vi "UNITEST MAIN v2.0.vi"() -> ()   [LabVIEW 2025]
uses:
  controls/LAB-IQ UI Data.ctl
  <vilib>/Platform/TimedLoop/XDataNode/timing_clust.ctl
  <vilib>/Platform/TimedLoop/XDataNode/nitl_modes.ctl
  <vilib>/Platform/TimedLoop/XDataNode/wakeup.ctl
  HEAVE vi's/Heave Write enum.ctl
  SWAY vi's/Sway Write enum.ctl
  d081153b-36ca-4bc4-8478-749476f82ba4.vi
  1202965f-721d-4349-8d61-5de826f379ef.vi
  785ec975-e53d-4ed4-be48-2cc128d7a91f.vi
  02c5850b-52e8-4ed5-91f8-6f0ad62f4994.vi
  1223eb78-e4c4-4b69-bf80-185c82055158.vi
  e5651a45-6a49-4a3f-b503-ff1eaf449b4a.vi
  <vilib>/Utility/error.llb/Trim Whitespace One-Sided.vi
  support/Message Queue/Enqueue Message (Single).vi
  <vilib>/Utility/error.llb/Error Cluster From Error Code.vi
  <vilib>/Utility/file.llb/Read Delimited Spreadsheet (string).vi
  <vilib>/Utility/file.llb/Write Delimited Spreadsheet (string).vi
  <vilib>/platform/TimedLoop/XDataNode/XDataNode.xnode
  <vilib>/ErrorRing/Error Ring.xnode
  support/Message Queue/LAB-IQ Message Queue.lvlib
  support/User Event - Stop/LAB-IQ User Event - Stop.lvlib
  <vilib>/Platform/TimedLoop/XDataNode/XDNodeRunTimeDep.lvlib
panel:
  in  "DEPTH TRIP   ENABLE":bool
  in  "DEPTH TRIP VALUE":dbl
  in  "LOAD TRIP  ENABLE":bool
  in  "LOAD TRIP VALUE":dbl
  in  "CYCLIC COF TRIP  ENABLE":bool
  in  "CYCLIC FF TRIP  ENABLE":bool
  in  "FF TRIP  ENABLE":bool
  in  "COF TRIP  ENABLE":bool
  in  "CYCLIC CoF TRIP VALUE":dbl
  in  "CYCLIC FF TRIP VALUE":dbl
  in  "FF TRIP VALUE":dbl
  in  "COF TRIP VALUE":dbl
  in  "Dummy Run":bool
  in  "AutoTune":bool
  in  "reinit 3":bool=TRUE
  in  "output range delay":cluster{"output high":dbl, "output low":dbl}={"output high"=100.0, "output low"=-100.0} {"output low" format="%.2f"; "output high" format="%.2f"}
  in  "PID gains out delay":T1={"proportional gain (Kc)"=30.0, "integral time (Ti, min)"=0.00101, "derivative time (Td, min)"=0.0} {"derivative time (Td, min)" format="%.3f"; "integral time (Ti, min)" min=1e-05 max=100.0 step=0.0001 format="%.4f"; "proportional gain (Kc)" format="%.3f"}
  in  "PID gains out delay (microForce)":T1={"proportional gain (Kc)"=300.0, "integral time (Ti, min)"=0.00011, "derivative time (Td, min)"=0.0} {"derivative time (Td, min)" format="%.3f"; "integral time (Ti, min)" min=1e-05 max=100.0 step=1e-06 format="%.6f"; "proportional gain (Kc)" format="%.3f"}
  in  "Gain 2":dbl=0.016
  in  "Offset  3":dbl=1.5
  in  "Ramp MulFac":dbl=2.0
  out "actpid":dbl
  in  "pulses LoadDiffRamp(2..10)":dbl=9.0
  in  "PulseControlRamp(diff<=3N)":dbl=5.0 min=1.0 max=1000.0 step=1.0 format="%#.1f"
  in  "SetLoadDeadband(%) Load(0-10N)":dbl=0.1 min=0.0001 max=100.0 step=0.0001 format="%#.6f"
  in  "pulses LoadDiff(2..10)":dbl=10.0
  in  "pulses LoadDiff(11..50)":dbl=40.0
  in  "PulseControl(diff<=3N)":dbl=1.0 min=1.0 max=1000.0 step=1.0 format="%#.1f"
  out "SetLoadDeadband(%)  2":dbl=1.0 min=0.001 max=100.0 step=0.001 format="%#.6f"
  in  "pulsesSent":dbl=200.0
  out "pulses":dbl
  in  "pulses LoadDiff(21..1000)":dbl=40.0
  in  "Delay":dbl=1.5 min=0.001 max=5.0 step=0.001 format="%#.6f"
  in  "deadband":dbl=0.2
  in  "Checkbox 2":bool
  in  "Checkbox":bool=TRUE
  out "Scratch Start Recording":bool
  in  "SwaySpeed Set":bool
  in  "Update":bool
  in  "Analysis Home":bool
  in  "Installation/Replacement completed":bool
  in  "Loahead":bool
  in  "Heave and Surge COM Port:":refnum<visa-resource-name>="COM9"
  in  "Sway COM Port:":refnum<visa-resource-name>="COM10"
  out "Test Trip":bool
  out "Hymidity":bool
  in  "Humidity Disable trip":bool=TRUE
  in  "CoF Trip  2":dbl=540.0 min=100.0 max=540.0 step=1.0
  in  "File Path :  2":path
  out "Wear Track Diameter":dbl
  in  "Stribeck table":bool
  in  "seq":bool=TRUE
  out "Drive Error":string
  out "mm/s  Surge":dbl=7.0 caption="Jog" min=0.001 max=50.0 step=0.0001 format="%.2f"
  in  "Update Surge Speed":bool
  out "mm/s  Sway":dbl=7.0 caption="Jog" min=0.001 max=50.0 step=0.0001 format="%.2f"
  in  "Update Sway Speed":bool
  in  "Update Heave Speed":bool
  out "mm/s Heave":dbl=7.0 caption="Jog" min=0.001 max=30.0 step=0.0001 format="%.2f"
  in  "mm/sec":dbl=1.0 caption="Jog" min=0.001 max=50.0 step=0.001 format="%.2f"
  out "Scratch Start Test":bool
  in  "HomeScratch":bool
  in  "TEST SELECTION":enum32{"Time", "Cycle"}(radio)
  out "HEAVE ENABLE":bool
  in  "SPARE  5":u8
  in  "Manual Write SWAY":bool
  out "SWAY WRITE":string
  in  "SPARE  4":u8
  in  "SPARE  3":u8
  in  "SPARE 2":u8
  in  "SPARE 1":u8
  out "Spare 15":u8
  out "Spare 14":u8
  out "Spare 13":u8
  out "Spare 12":u8
  out "Spare 11":u8
  out "Spare 10":u8
  out "Spare 9":u8
  out "Spare 8":u8
  out "Spare 7":u8
  out "Spare 6":u8
  out "Spare 5":u8
  out "Spare 4":u8
  out "Spare 3":u8
  out "Spare 2":u8
  out "Spare 1":u8
  out "Node Id":u8
  out "Read SWAY Temp":bool
  out "fwMinor":u8
  out "fwMajor":u8
  out "faultCode":u16
  out "Rotary POSE":sgl format="%#.6f"
  out "SWAY POSE":sgl format="%#.6f"
  out "Homed":u8
  out "State":u8
  out "Ack ID":u16
  in  "SPEED":sgl=10000.0
  in  "Distance":sgl=10000.0
  in  "Mode Command":u8=2
  out "Sequence ID":u16
  out "error out Read SWAY":errorcluster
  out "error out Write  SWAY":errorcluster
  out "SWAY READ":string
  out "Start Test Temp":bool
  in  "AppLoadSeq scratch":bool
  in  "PID Delay (sec)":dbl=1.0 format="%#_6p"
  in  "Manual Write Heave & Surge":bool
  out "Heave and Surge Write":string
  in  "SPARE 4":u8
  in  "SPARE 3":u8
  in  "SPARE 2":u8
  in  "SPARE 1":u8
  out "Spare 15":u8
  out "Spare 14":u8
  out "Spare 13":u8
  out "Spare 12":u8
  out "Spare 11":u8
  out "Spare 10":u8
  out "Spare 9":u8
  out "Spare 8":u8
  out "Spare 7":u8
  out "Spare 6":u8
  out "Spare 5":u8
  out "Spare 4":u8
  out "Spare 3":u8
  out "Spare 2":u8
  out "Spare 1":u8
  out "Node Id":u8
  out "Read Heave Temp":bool
  out "fwMinor":u8
  out "fwMajor":u8
  out "faultCode":u16
  out "SURGE POSE":sgl format="%#.6f"
  out "HEAVE POSE":sgl format="%#.6f"
  out "Homed":u8
  out "State":u8
  out "Ack ID":u16
  in  "SPEED":sgl=10000.0
  in  "Distance":sgl=10000.0
  in  "Mode Command":u8=2
  out "Sequence ID":u16
  out "error out Read":errorcluster
  out "error out Write":errorcluster
  out "Heave and Surge Read":string
  out "Load Cell Temp":bool
  in  "Stop Scratch":bool
  in  "Enter Fixed SRR 2":dbl min=0.0 max=0.0 format="%.3f"
  in  "E.Velocity 2":bool=TRUE caption="SRR"
  in  "Tab Control 3":T2(tab)
  in  "Tab Control 5":enum32{""}(tab)
  in  "Tab Control 14":T3(tab)=enum."Motor Load"
  in  "Ramp":bool
  in  "apply load":bool
  in  "Enter ByPass Load":dbl
  in  "Bypass Load":bool
  out "gFF Rot 7":cluster{dbl, dbl, dbl}(graph)
  in  "Current Load":dbl
  in  "Set Load":dbl
  out "Current Position":dbl
  in  "Kp":dbl=1.0
  in  "Ki":dbl
  in  "Kd":dbl
  in  "Deadband":dbl=0.1
  in  "pct_scale":dbl=100.0
  in  "Init Step":dbl=10.0
  in  "Max Step Linit":dbl=10.0
  in  "i_limit":dbl=10.0
  in  "Min_pos_limit":dbl
  in  "Max_pos_limit":dbl=50000000.0
  in  "Fine Tune Zone":dbl=10.0
  in  "fine_tune_pct":dbl=100.0
  in  "min_deadband_floor":dbl=0.05
  in  "min_finetune_floor":dbl=0.15
  out "Pulse delta":dbl
  out "Vertical load (N)":dbl format="%#.3f"
  in  "Tab Control 26":enum32{"Page 1", "Page 2"}(tab)
  in  "ClearAll":bool
  out "Mz(Nm)":dbl[](array[numeric])
  out "My(Nm)":dbl[](array[numeric])
  out "Mx(Nm)":dbl[](array[numeric])
  in  "Save Dwell":dbl=0.015 caption="Save Dwell (sec)" min=0.0 max=5.0 step=0.001 format="%.3f"
  out "Mx":dbl[](graph)
  out "My":dbl[](graph)
  out "Mz":dbl[](graph)
  out "Fy(N)":dbl[](graph)
  out "Fz(N)":dbl[](graph)
  in  "ZeroAll":bool
  in  "Acq Delay (ms)":dbl=10.0
  in  "Burst Delay (ms)":dbl=10.0
  out "model":string
  out "SN":i32
  out "FFx(N)":dbl[](array[numeric])
  in  "Sensor IP":string="192.168.1.100"
  in  "Port":i32=8080
  out "FFy(N)":dbl[](array[numeric])
  out "Load(N)":dbl[](array[numeric])
  out "Fx(N)":dbl[](graph)
  out "AE":bool
  in  "delete Handle":bool
  in  "Create Handle":bool=TRUE
  out "ft_data":dbl[](array[numeric])=[1.0, 1.0, 1.0, 1.0, 1.0, 1.0]
  out "ft_range":dbl[](array[numeric])=[1.0, 1.0, 1.0, 1.0, 1.0, 1.0]
  in  "stop 6":bool
  out "running_flag":bool
  out "ft_udp_handle":i32
  out "get-data-return":i32
  out "get-range-return":i32
  out "zero-return":i32
  out "filter-return":i32
  out "initial-return":i32
  out "deleteHandle-result":i32
  in  "Tab Control 19":enum32{"Platform COM", "Config ", "DevInfo"}(tab)=enum."Config "
  in  "SAMPLES":dbl=100.0
  in  "Re-initilaize":bool
  in  "Filter ON/OFF":bool=TRUE
  in  "TracHomeSurgeOffsetCounts 10MM":dbl=505100.0
  in  "TracHomeSwayOffsetCounts 10MM":dbl=1432.0
  in  "Acoustic Emission:":dbl=1.0 min=0.0001 max=200.0 step=0.0001 format="%.4f"
  in  "Apply Filter (FF)":bool
  in  "Filter% 2":dbl=50.0 min=50.0 max=100.0 step=0.1 format="%.1f"
  in  "Apply Filter (Load)":bool=TRUE
  in  "Filter%":dbl=80.0 min=50.0 max=100.0 step=0.1 format="%.1f"
  in  "Sway distance (mm)":dbl=245.0
  in  "Surge distance (mm)":dbl=370.0
  in  "DataSavingLoopDelay(ms)":dbl=15.0
  in  "SAVE  2":bool
  in  "Enter Distance":bool caption="Enter Counts"
  in  "Sway Counts:":dbl=100.0 min=0.0 max=100000000.0 step=1.0 format="%.2f"
  in  "Distance (mm): 3":dbl=100.0 caption="Distance (mm):" min=0.0 max=1500.0 step=0.001 format="%.5f"
  in  "Surge Counts:":dbl=100.0 min=0.0 max=100000000.0 step=1.0 format="%.1f"
  in  "Distance (mm): 2":dbl=100.0 caption="Distance (mm):" min=0.0 max=1500.0 step=0.0001 format="%.3f"
  in  "Distance (mm):":dbl=100.0 min=0.0 max=1500.0 step=0.001 format="%.5f"
  in  "Heave Counts:":dbl=100.0 min=0.0 max=100000000.0 step=1.0
  in  "LRMHomeSurgeOffsetCounts":dbl=307197.0
  in  "LRMHomeSwayOffsetCounts":dbl=26880.0
  in  "TracHomeSurgeOffsetCounts 20MM":dbl=505100.0
  in  "TracHomeSwayOffsetCounts 20MM":dbl=1432.0
  in  "RotHomeSwayOffsetCounts":dbl=14656.0
  in  "RotHomeSurgeOffsetCounts":dbl=311465.0
  in  "Heave distance":dbl=340.0
  out "Zmm":dbl=1600.0
  out "Heave Pulses/mm":dbl=1600.0
  out "Surge Pulses/mm":dbl=1600.0
  out "Sway Pulses/mm":dbl=320.0
  in  "Heave Pitch":dbl=4.0
  in  "Surge Pitch":dbl=3.0
  in  "Sway Pitch":dbl=2.0
  in  "Heave PPR":dbl=6400.0
  in  "Surge PPR":dbl=6400.0
  in  "Sway PPR":dbl=6400.0
  in  "Heave Jog Speed":dbl=15.0
  in  "Surge Jog Speed":dbl=1.0 format="%.4f"
  in  "Heave PID Speed":dbl=15.0
  in  "Heave Loop Delay":dbl
  in  "Sway Jog Speed":dbl=1.0 format="%.4f"
  in  "Sway PID Speed":dbl=1.0 format="%.4f"
  in  "Sway Loop Delay":dbl
  in  "GUI":T4(tab)
  in  "Platform Settings":bool caption="Password"
  in  "Configure":bool caption="Password"
  in  "Home":bool caption="Password"
  in  "EXIT":bool
  in  "Analysis":bool caption="Password"
  in  "service 2":bool caption="Password"
  in  "MainPage":T5(tab)=enum."HOME"
  in  "Select Load Head":bool
  in  "Notes :":string
  in  "FILE":string
  in  "Sample ID :":string
  in  "Operator ID :":string
  in  "Operator Name :":string
  in  "Auto":bool caption="Power Status"
  in  "Disable Axis Jog Soft Limits m":bool
  out "Sway and Surge COM Status":bool=TRUE caption="Load COM Status"
  out "Heave COM Status":bool=TRUE caption="Load COM Status"
  in  "Enable Platform":bool
  in  "Surge Forward Main":bool
  in  "Surge Backward Main":bool
  in  "Sway Right Main":bool
  in  "Sway Left Main":bool
  in  "Heave Down Main":bool
  in  "Heave Up main":bool
  in  "mm":dbl=0.001 caption="Jog" min=1.0 max=100.0 step=0.01 format="%#.3f"
  in  "Surface Analysis":bool
  in  "Imaging":bool
  in  "Image Analysis":bool
  in  "Post Analysis":bool
  in  "SSP 0.75":bool
  in  "SSP 0.5":bool
  in  "SSP 0.3":bool
  in  "Warning":enum32{"Page 2"}(tab)
  in  "gui GIF":enum32{"Check", "Deca", "kilo", "Micro"}(tab)
  out "Communication is established":bool=TRUE caption="Load COM Status"
  in  "Reference Sample":u16(ring) items=["None", "Brass", "Aluminium", "Mild Steel"]
  out "Load Cell Communication Slide":u8(slide)=1 min=1 max=10 step=1 scale=0.0..10.0
  in  "com 3":bool
  out "com":bool
  out "DecaForce COM Status":bool caption="Load COM Status"
  in  "Loading Mode":u16(ring) items=["Constant", "Ramp", "Steps", "Indentation"]
  in  "Enter the CoF Trip":dbl=1.0
  in  "Enter the Friction Force Trip":dbl=520.0 min=500.0 max=500.0 step=1.0 format="%#.1f"
  in  "Enter the Normal load Trip":dbl=520.0 min=500.0 max=500.0 step=0.001 format="%.3f"
  in  "KiloForce":bool
  in  "DecaForce":bool
  in  "MicroForce":bool
  in  "LHBack":bool
  in  "LHNext":bool
  in  "Load Selection":T6(tab)
  in  "Enter the Load  (N)":dbl=2.0 caption="Enter the Load (N)" min=2.0 max=200.0 step=0.1 format="%#.4f"
  in  "Enter the Final Load (N)":dbl=1.0 min=0.0 max=500.0 step=1.0 format="%#.0f"
  in  "Enter the Loading Rate (N/min)":dbl=60.0 min=1.0 max=1200.0 step=0.1 format="%.2f"
  out "Warning 2":bool
  in  "Stribeck Table  For loading":string[][](table)
  in  "Clear 3":bool
  out "Message":string="Load Entered is out of range!!!"
  in  "Indentation":string[][](table)=[["Detection", "5", "2"], ["Unload", "0", "5"], ["Load", "10", "2"], ["Unload", "0", "5"], ["Detection", "5", "2"], ["Unload", "0", "5"]]
  in  "Multipoint":bool caption="Singlepoint"
  in  "AppLoad 4":bool
  in  "zNL":bool
  out "NL disp":dbl caption="Normal Load ( N )" min=-2000.0 max=2000.0 step=0.0001 format="%.1f"
  in  "Traction":bool
  in  "Surge Forward MM":bool
  in  "Surge Backward MM":bool
  in  "M3 Image":enum32{"Page 1", "Page 2"}(tab)
  in  "String 39":string="Jog heave to bring the upper sample closer to the lower sample within 1mm."
  in  "Sway Left MM":bool
  in  "Sway Right MM":bool
  in  "Disable Axis Jog Soft Limits":bool
  in  "mm":dbl=0.001 caption="Jog" min=0.001 max=5.0 step=0.0001 format="%#.3f"
  in  "Heave Down MM":bool
  in  "Heave Up MM":bool
  in  "Wear Track Diameter (mm)":dbl=30.0 caption="Wear Track Diameter (mm):" min=1.0 max=30.0 step=1.0 format="%.2f"
  in  "Set WTD":bool
  in  "HomeScratch":bool
  in  "HomeRot":bool
  in  "PlaceModule":bool
  in  "Motion Mode:":u16(ring) items=["Uniform Rotation", "Angular Oscillation", "Stribeck ", "Steps"]
  in  "LR Sway":bool
  in  "Rot Hor":bool
  in  "Rot Ver":bool
  in  "Scratch":bool
  in  "LR Cam":bool
  in  "MMBack":bool
  in  "MMNext":bool
  in  "Rotary Module Selection":T7(tab)
  in  "SPEED SELECTION :":enum32{"Speed in RPM", "Speed in m/sec"}(radio)=enum."Speed in m/sec"
  in  "Enter the Speed(mm/sec)":dbl=0.1 min=0.1 max=10.0 step=0.1 format="%.3f"
  in  "Enter the Speed (RPM)":dbl=45.0 min=1.0 max=3000.0 step=1.0
  in  "Enter the Frequency (Hz)":dbl=1.0 min=0.1 max=10.0 step=0.1 format="%.1f"
  in  "Enter the Angle (Deg)":dbl=45.0 min=5.0 max=300.0 step=1.0
  in  "Angular Oscillation Set":bool
  in  "Rotary Tab":enum32{"Page 1", "Page 2"}(tab)
  out "e.v/ssr 2":enum32{"E.V", "SSR"}(tab)
  in  "Enter the Final E.Velocity (m/s) 2":dbl=1.0 min=0.001 max=4.0 step=0.001 format="%.3f"
  in  "Enter initial E.Velocity (m/s) 2":dbl=2.0 min=0.001 max=4.0 step=0.001 format="%.3f"
  in  "Enter Fixed E.Velocity 2":dbl=1.0 min=0.001 max=2.0 step=0.001 format="%.3f"
  in  "Enter Final SRR 2":dbl=1.0 min=0.001 max=1.0 step=0.001 format="%.2f"
  in  "Enter initial SRR 2":dbl=1.0 min=0.001 max=1.0 step=0.001 format="%.2f"
  out "Final Speed (RPM) 3":dbl=1.0 min=0.1 max=3000.0 step=0.1 format="%.1f"
  out "Initial Speed (RPM) 2":dbl=100.0 min=0.1 max=3000.0 step=0.1 format="%.1f"
  in  "Enter the Final Velocity (m/s) 3":dbl=1.0 min=0.001 max=2.0 step=0.001 format="%.3f"
  in  "Enter initial Velocity (m/s)  3":dbl=2.0 min=0.001 max=2.0 step=0.001 format="%.3f"
  out "Ramp Up 2":bool caption="Ramp Down"
  in  "Import 2":bool
  in  "Save 2":bool
  in  "SPEED SELECTION : rotary":enum32{"Speed in Rpm", "Speed in m/sec"}(radio)=enum."Speed in m/sec"
  in  "calculate rotary":bool
  in  "String 45":string="File Path Location : C:-->LAB-IQ 150 --> User Defined\n                                       Protocol-->File.txt"
  in  "Step Speed":enum32{"Step Speed", "Step (load-Speed)"}(tab)
  in  "StepTable For Speed":string[][](table)
  in  "StepTable For Load-Speed":string[][](table)=[["", "", ""], ["", "", ""], ["", "", ""], ["", "", ""]]
  in  "StepTable For Speed 3":string[][](table)=[["", "", ""], ["", "", ""], ["", "", ""], ["", "", ""]]
  in  "Motion Direction:  3":u16(ring) items=["Clockwise", "Counter Clockwise"]
  in  "Enter Scratch length (mm):":dbl=1.0 min=1.0 max=50.0 step=0.0001 format="%.4f"
  in  "Enter Scratch Speed (mm/s):":dbl=1.0 min=0.003 max=10.0 step=0.0031 format="%.5f"
  in  "Scartch Offset":dbl=1.0 caption="Scratch Offset: (mm)" min=0.1 max=5.0 step=0.1 format="%.1f"
  in  "Motion type:":u16(ring) items=["Unidirection", "Bidirection"]
  in  "Scratch Mode":u16(ring) items=["Scratch", "Pre-Post Scan", "Multi Scratch"]
  in  "Rotary Speed Exced":string="Motor Speed Out of Range"
  in  "No of Scratch":dbl=1.0 min=1.0 max=50.0 step=0.0001
  out "Humidity  Status  3":bool caption="Communication Status"
  out "Low Temp  Status  2":bool=TRUE caption="Communication Status"
  out "TK4 status 2":bool=TRUE caption="Communication Status"
  in  "String 40":string="Before selecting Acoustic make sure the sensor output pin is connected to A4."
  in  "Stage Temperature":dbl[](array[numeric])=[150.0, 230.0, 300.0, 350.0, 400.0, 450.0, 500.0]
  in  "Sample Temperature":dbl[](array[numeric])=[100.0, 150.0, 200.0, 250.0, 300.0, 350.0, 400.0]
  in  "Humidity (Amb)":bool
  in  "Clear List":bool
  out "Sensors Picked":string
  in  "Add to list":bool
  in  "Wear":bool
  in  "Vibration":bool
  in  "Humidity (Chamber)":bool
  in  "Temperature (Chamber)":bool
  in  "ECR":bool
  in  "Temperature (Amb)":bool
  in  "Microphone":bool
  in  "Acoustic Emission 3":bool
  in  "SNext":bool
  in  "APBack":bool
  in  "Enter the Temperature (°C):":dbl
  in  "Enter the Stage \nTemperature (°C):":dbl=20.0 min=20.0 max=150.0 step=1.0 format="%#.0f"
  in  "Enter the Humidity (%Rh):":dbl=30.0 min=30.0 max=85.0 step=1.0
  in  "Low Temp":bool
  in  "High Temp":bool
  in  "Humidity":bool
  in  "Main Screen Tab":T8(tab)
  in  "ClrLog":bool
  out "Trip Log":string
  in  "Start Test":bool
  out "Test status":bool caption="Test Status"
  out "AR Led":bool caption="AR"
  out "Data":bool=TRUE
  out "Health":bool=TRUE
  out "Sway COM Status":bool=TRUE caption="Load COM Status"
  out "Heave COM Status":bool=TRUE caption="Load COM Status"
  in  "BACK":bool
  out "Ambient \nTemperature":dbl min=0.0 max=5000.0 step=0.1 format="%.1f"
  out "Ambient\n Humidity":dbl min=0.0 max=5000.0 step=0.1 format="%.2f"
  out "NL disp 2":dbl caption="Normal Load ( N )" min=-2000.0 max=2000.0 step=0.0001 format="%.1f"
  out "Set Humidity":dbl caption="Set Humidity  (% Rh)" min=-2000.0 max=2000.0 step=1.0 format="%.1f"
  out "humidity disp":dbl caption="Humidity (% Rh)" min=-2000.0 max=2000.0 step=1.0 format="%.1f"
  in  "Humidity On":bool
  in  "zNL 2":bool
  out "NLt":bool
  in  "Load En":bool
  out "Freq (Hz)":dbl min=0.0 max=5000.0 step=0.1 format="%.4f"
  out "HumCOMStatus":bool caption="Communication Status"
  out "Load Communication":bool
  in  "Temp Tabs":enum32{"Low Temp", "High Temp"}(tab)=enum."High Temp"
  out "Controller  Status":bool
  out "ChamberTemp":dbl format="%#.1f"
  in  "SetTmp":dbl=-190.0 caption="Set Temperature (Deg C)" min=-190.0 max=100.0 step=1.0 format="%.1f"
  in  "Cooling":bool
  in  "Heater":bool
  out "TK4 status":bool caption="Controller  Status"
  out "ChamberTemp":dbl format="%#.1f"
  in  "SetTmp":dbl caption="Set Temperature (Deg C)" min=0.0 max=1000.0 step=1.0 format="%.1f"
  in  "Set Load (N)":dbl=100.0 min=0.01 max=1500.0 step=0.01 format="%.1f"
  in  "Time Tab":enum32{"cycles", "duration"}(tab)=enum."duration"
  out "Test Duration 4":dbl=600.0 caption="Test Duration\n(HH:MM:SS)" min=0.0083 max=180000.0 step=0.0001 format="%<%H:%M:%S>t"
  out "TEST CYCLE":dbl min=0.0 max=5000.0 step=0.01 format="%.2f"
  in  "TOTAL CYCLES":dbl min=0.0 max=5000.0 step=0.1 format="%.4f"
  out "Time ( HH:MM:SS ) 2":dbl min=0.0 max=144000.0 step=1.0 format="%<%H:%M:%S>t"
  in  "Test Duration":dbl=600.0 caption="Test Duration\n(HH:MM:SS)" min=0.0083 max=180000.0 step=0.0001 format="%<%H:%M:%S>t"
  in  "Main Speed Tab":enum32{"ROTARY", "TRACTION"}(tab)
  in  "SPEED TAB":enum32{"RPM", "m/sec"}(tab)
  out "Speed (RPM)":dbl min=0.0 max=5000.0 step=0.1 format="%.1f"
  out "Set Speed":dbl caption="Set Speed (RPM)" min=0.0 max=1500.0 step=0.1 format="%.1f"
  out "Speed (m/sec)":dbl min=0.0 max=5000.0 step=0.001 format="%.4f"
  out "Set Speed (m/sec)":dbl min=0.0 max=1500.0 step=0.001 format="%.4f"
  in  "MTM MOTOR DISPLAY":enum32{"MTM RPM", "MTM m/sec"}(tab)
  out "Disc Speed (RPM)":dbl min=0.0 max=1500.0 step=0.1 format="%.1f"
  out "Ball Speed (RPM)":dbl min=0.0 max=1500.0 step=0.1 format="%.1f"
  out "Disc Speed (m/sec)":dbl min=0.0 max=1500.0 step=0.1 format="%.1f"
  out "Ball Speed (m/sec)":dbl min=0.0 max=1500.0 step=0.1 format="%.1f"
  in  "Angle and Frequency":enum32{"angular", "lrm"}(tab)
  out "Angle (Deg)":dbl min=0.0 max=5000.0 step=0.01 format="%.2f"
  out "Stroke (mm)":dbl min=0.0 max=5000.0 step=0.01 format="%.2f"
  in  "STOP":bool
  out "Multi Scratch Pass":dbl min=0.0 max=5000.0 step=0.1
  in  "FF Tab":T9(tab)
  in  "COF Reset Graph":bool
  in  "COF Disable Trip":bool=TRUE
  out "COF TRIP":dbl=600.0
  out "Coefficient of Friction":dbl(graph)=0.13298760003255525
  in  "zFF":bool
  in  "FF Reset Graph":bool
  in  "FF Disable Trip":bool=TRUE
  out "FF TRIP":dbl=600.0
  out "Friction Force (N)":dbl min=-2000.0 max=2000.0 step=0.0001 format="%.3f"
  out "Friction Force (N) Graph":dbl(graph)=0.13298760003255525
  out "Cyclic FF TRIP":dbl=600.0
  in  "Cyclic FF Disable Trip":bool=TRUE
  in  "Cyclic FF Reset Graph":bool
  in  "CZ FF":bool
  out "Cyclic Friction Force (N) Graph":dbl(graph)=0.13298760003255525
  out "Cyclic Friction Force (N)":dbl min=-2000.0 max=2000.0 step=0.0001 format="%.3f"
  out "cyclic COF TRIP":dbl=600.0
  in  "cyclic COF Disable Trip":bool=TRUE
  in  "cyclic COF Reset Graph":bool
  out "Cyclic Coefficient of Friction":dbl(graph)=0.13298760003255525
  out "Main Chart 3":cluster{dbl, "NL disp":dbl, dbl}(graph)
  out "NL Display 4":dbl caption="Normal Load ( N )" min=-2000.0 max=2000.0 step=0.0001 format="%.1f"
  in  "Load Reset Graph":bool
  in  "Load Disable Trip":bool=TRUE
  out "Load pid":bool
  out "NL Trip 2":dbl=600.0
  out "WearGp":dbl(graph)=0.13298760003255525
  out "Depth (µm)":dbl min=-200.0 max=200.0 step=0.1 format="%.1f"
  in  "Depthz":bool
  out "Weart":bool
  in  "Depth Reset Graph":bool
  out "Weart Deapth":bool
  in  "Depth Trip 2":bool=TRUE
  out "Depth Trip":dbl=600.0
  in  "Sub Graph":T10(tab)
  in  "Speed Tab":enum32{" Rotary Disc", "MTM Ball", "MTM Disc"}(tab)
  out "speed mm/sec":dbl(graph)=0.13298760003255525
  in  "Speed Reset Graph":bool
  out "MTM BALL SPEED":dbl(graph)=0.13298760003255525
  out "MTM DISC  SPEED":dbl(graph)=0.13298760003255525
  in  "Temperature Reset":bool
  out "Temperature (deg c)":dbl(graph)=0.13298760003255525
  out "ECR 2":dbl(graph)=0.13298760003255525
  in  "ECR RESET":bool
  out "Acoustic Emission (mV)":dbl min=0.0 max=5000.0 step=0.1
  in  "Aqucostic Reset Graph":bool
  out "gACQUOS":dbl(graph)=0.13298760003255525
  in  "Humidity Reset Graph":bool
  out "HumrGp":dbl(graph)=0.13298760003255525
  out "SD (mm)":dbl caption="Sliding Distance ( mm )" min=-200.0 max=200.0 step=0.1 format="%.4f"
  in  "Siliding distance Reset Graph":bool
  out "SDGp":dbl(graph)=0.13298760003255525
  in  "X-AXIS":u16(ring) items=["None", "Time ( Sec )", "Normal Load ( N )", "Frictional Force ( N )", "Coefficient of Friction", "Depth ( Microns )", "Speed ( RPM )", "Frequency ( Hz )", "Angle ( Degree )", "Cyclic Friction Force ( N )", "Cyclic Co efficient Friction ", "Stage temperature ( Degree celcius )", "Sample temperature ( Degree celcius )", "Stroke Length ( mm )", "Scratch Speed ( mm/sec )", "Amb Humidity ( % Rh ) ", "Amb Temperature (Deg C)", "Acoustic (mV)", "Mx (Nm)", "My (Nm)", "Mz (Nm)", "Humidity ( % Rh )", "Sliding Distance (mm)", "Wear Track Diameter (mm)", "Fx(N)", "Fy(N)", "MTM BallSpeed (RPM)", "MTM DiscSpeed (RPM)", "Entrainment Speed", "Slide Role", "Slip(%)", "Rotary Speed (m/sec)", "MTM Ball Speed (m/sec)", "MTM Disc Speed (m/sec)", "ECR (ohms)"]
  in  "Y-AXIS":u16(ring) items=["None", "Time ( Sec )", "Normal Load ( N )", "Frictional Force ( N )", "Coefficient of Friction", "Depth ( Microns )", "Speed ( RPM )", "Frequency ( Hz )", "Angle ( Degree )", "Cyclic Friction Force ( N )", "Cyclic Co efficient Friction ", "Stage temperature ( Degree celcius )", "Sample temperature ( Degree celcius )", "Stroke Length ( mm )", "Scratch Speed ( mm/sec )", "Amb Humidity ( % Rh ) ", "Amb Temperature (Deg C)", "Acoustic (mV)", "Mx (Nm)", "My (Nm)", "Mz (Nm)", "Humidity ( % Rh )", "Sliding Distance (mm)", "Wear Track Diameter (mm)", "Fx(N)", "Fy(N)", "MTM BallSpeed (RPM)", "MTM DiscSpeed (RPM)", "Entrainment Speed", "Slide Role", "Slip(%)", "Rotary Speed (m/sec)", "MTM Ball Speed (m/sec)", "MTM Disc Speed (m/sec)", "ECR (ohms)"]
  out "XY Graph":cluster{"Array 2":dbl[], "Array 2":dbl[]}[](graph) caption="XY Graph 20"
  out "VARIANCE":dbl=-0.0 format="%0.2f"
  out "SD":dbl=-0.0 format="%.3f"
  out "MEAN":dbl format="%.3f"
  out "VARIANCE":dbl=-0.0 format="%0.2f"
  out "SD":dbl=-0.0 format="%.3f"
  out "MEAN":dbl format="%.3f"
  out "VARIANCE":dbl=-0.0 format="%0.2f"
  out "SD":dbl=-0.0 format="%.3f"
  out "MEAN":dbl format="%.3f"
  out "VARIANCE":dbl=-0.0 format="%0.2f"
  out "SD":dbl=-0.0 format="%.3f"
  out "MEAN":dbl format="%.3f"
  in  "Analysis Home new":bool
  out "File 2 Discription":string="\r"
  out "File 1 Discription":string="\r"
  in  "OPEN 1":bool
  in  "OPEN 2":bool
  out "File Name 1":string
  out "File Name 2":string
  in  "Refresh 2":bool
  in  "OPEN 3":bool
  out "File Name 3":string
  out "File Name 4":string
  in  "OPEN 4":bool
  out "File 4 Discription":string="\r"
  out "File 3 Discription":string="\r"
  in  "File Format":u16(ring) items=["csv", "txt", "duf"]
  in  "Export":bool
  in  "Report":bool
  in  "Password":string
  in  "Home Service":bool
  in  "Advanced Setting":bool
  in  "About Tab":enum32{"Primary"}(tab)
  in  "ECR Port:":refnum<visa-resource-name>="COM10"
  in  "Ramp Port:":refnum<visa-resource-name>="COM10"
  in  "Temp Modbus:":refnum<visa-resource-name>="COM14"
  in  "Humidity Port:":refnum<visa-resource-name>="COM10"
  in  "Edit Gain Constants":bool
  in  "Save Gain Constants":bool
  in  "Service About":bool
  # "SET JOG SPEED"
  # "Speed Exceed the limit of the Motor"
  # "Motor Speed Out of Range"
  # "NOTE: This operation needs to be done only when the machine is ON."
  # "ohms"
  # "load Aquisition off"
  # "load Aquisition On"
  # "Configuration"
  # "Limits for Heave Surge and Sway"
  # "Modules Offset Parameters"
  # "Counts-Distance Calculator"
  # "File Name :"
  # "Ensure the traction module is aligned\n horizontally with the stage before ENABLE."
  # "JOG MODE"
  # "Module Selection"
  # "Positioning Control"
  # "Connect the controller\ncable to M3"
  # "Environment"
  # "Sensors"
  # "Data Points"
  # "Data Points"
  # "Data Points"
  # "Data Points"
  # "Data Points"
  # "Data Points"
  # "Data Points"
  # "LAB-IQ 150 / UNITEST / WO2456 / UT150  v05 / AUGUST 2025"
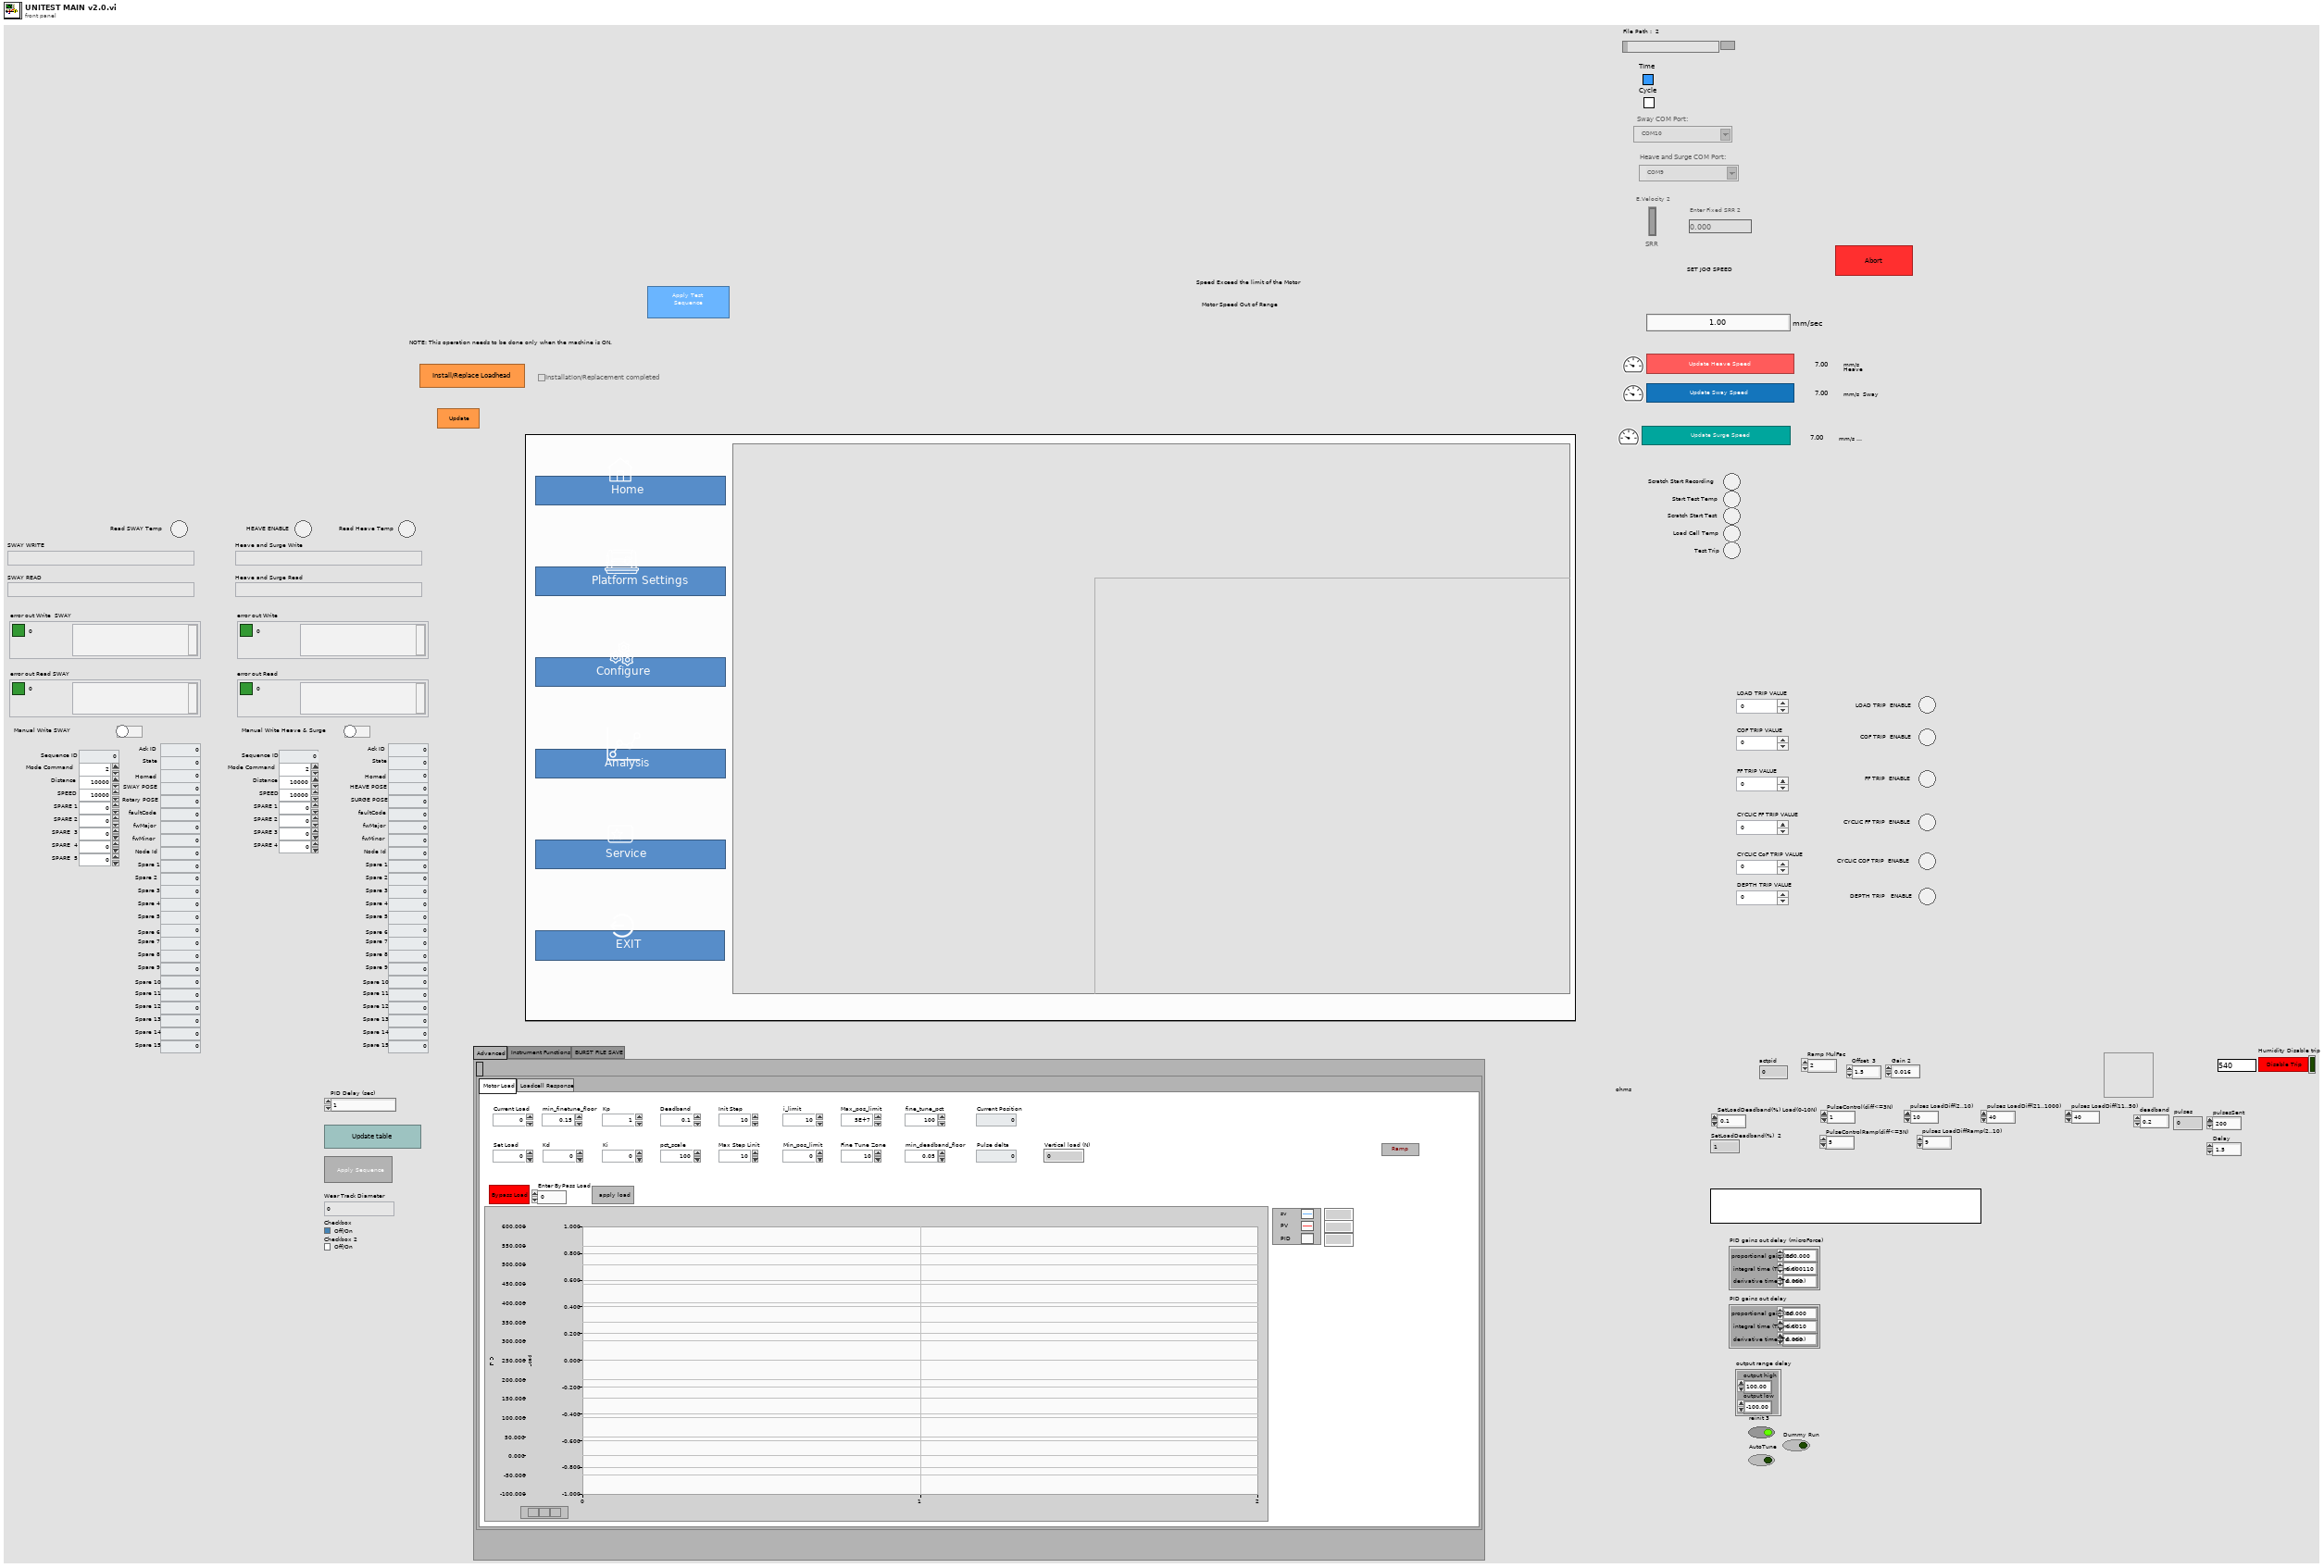
[diagram p1: front panel]
types:
  T1 = cluster{"proportional gain (Kc)":dbl, "integral time (Ti, min)":dbl, "derivative time (Td, min)":dbl}
  T2 = enum32{"Advanced", "Motor", "Depth_graph", "UIO Communicator", "Add to list parametrs", "Instrument Functions", "BURST FILE SAVE"}
  T3 = enum32{"LRM heating", "FBT_Heating", "Motor Load", "Loadcell Response", "Voice Load", "Step loading and speed ", "Depth"}
  T4 = enum32{"Setup", "Load Head", "Motion Module", "Environment", "Begin"}
  T5 = enum32{"Details", "PlatformSetting", "Analysis", "HOME"}
  T6 = enum32{"Constant", "Ramp", "Step", "Indentation"}
  T7 = enum32{"Uniform Rotation", "Angular Oscillation", "Speed Ramp", "Speed Step"}
  T8 = enum32{"  Acquire  ", "Compare Files Rot", "About", "Service"}
  T9 = enum32{"Coefficient of Friction ", "Friction Force (N)", "Cyclic Friction Force (N)", "Cyclic Coefficient of Friction "}
  T10 = enum32{"Speed", "Temperature", "ECR", "Acoustic Emission", "Humidity", "Sliding Distance"}
  T11 = typedef "LAB-IQ UI Data.ctl" = cluster{"Main Home Screen":cluster{"GUI":refnum<vi>, "Platform Settings":refnum<vi>, "Configure":refnum<vi>, "Home":refnum<vi>, "EXIT":refnum<vi>, "service 2":refnum<vi>, "MainPage":refnum<vi>, "Analysis":refnum<vi>}, "Platform Settings":cluster{"mm/s  Surge":refnum<vi>, "Update Surge Speed":refnum<vi>, "Drive Error":refnum<vi>, "Disable Axis Jog Soft Limits":refnum<vi>, "mm/s  Sway":refnum<vi>, "Sway and Surge COM Status":refnum<vi>, "Heave COM Status":refnum<vi>, "Enable Platform":refnum<vi>, "Surge Forward Main":refnum<vi>, "Sway Right Main":refnum<vi>, "Sway Left Main":refnum<vi>, "Heave Down Main":refnum<vi>, "Heave Up main":refnum<vi>, "Update Sway Speed":refnum<vi>, "Update Heave Speed":refnum<vi>, "mm/s Heave":refnum<vi>, "mm/sec":refnum<vi>, "mm":refnum<vi>, "Surge Backward Main":refnum<vi>}, "Analysis Screen":cluster{"Analysis Home":refnum<vi>, "Surface Analysis":refnum<vi>, "Imaging":refnum<vi>, "Image Analysis":refnum<vi>, "Post Analysis":refnum<vi>}, "Config Screen":cluster{"Select Load Head":refnum<vi>, "Notes :":refnum<vi>, "FILE":refnum<vi>, "Sample ID :":refnum<vi>, "Operator ID :":refnum<vi>, "Operator Name :":refnum<vi>, "Auto":refnum<vi>}, "Motion Module":cluster{"zNL":refnum<vi>, "NL disp":refnum<vi>, "Rotary Tab":refnum<vi>, "Motion Direction:  3":refnum<vi>, "E.Velocity 2":refnum<vi>, "e.v/ssr 2":refnum<vi>, "Enter Fixed E.Velocity 2":refnum<vi>, "Enter Final SRR 2":refnum<vi>, "Enter initial SRR 2":refnum<vi>, "Enter Fixed SRR 2":refnum<vi>, "Enter the Final E.Velocity (m/s) 2":refnum<vi>, "Enter initial E.Velocity (m/s) 2":refnum<vi>, "Final Speed (RPM) 3":refnum<vi>, "Initial Speed (RPM) 2":refnum<vi>, "Enter the Final Velocity (m/s) 3":refnum<vi>, "Enter initial Velocity (m/s)  3":refnum<vi>, "Ramp Up 2":refnum<vi>, "TEST SELECTION":refnum<vi>, "SPEED SELECTION : ":refnum<vi>, "Angular Oscillation Set":refnum<vi>, "Traction":refnum<vi>, "Step Speed":refnum<vi>, "StepTable For Load-Speed":refnum<vi>, "StepTable For Speed":refnum<vi>, "Surge Forward MM":refnum<vi>, "Surge Backward MM":refnum<vi>, "M3 Image":refnum<vi>, "String 39":refnum<vi>, "Sway Left MM":refnum<vi>, "Sway Right MM":refnum<vi>, "Disable Axis Jog Soft Limits":refnum<vi>, "mm":refnum<vi>, "Heave Down MM":refnum<vi>, "Heave Up MM":refnum<vi>, "Wear Track Diameter (mm)":refnum<vi>, "Set WTD":refnum<vi>, "HomeScratch":refnum<vi>, "HomeRot":refnum<vi>, "PlaceModule":refnum<vi>, "Enter the Angle (Deg)":refnum<vi>, "Enter the Frequency (Hz)":refnum<vi>, "Motion Mode:":refnum<vi>, "LR Sway":refnum<vi>, "Rot Hor":refnum<vi>, "Scratch":refnum<vi>, "LR Cam":refnum<vi>, "MMBack":refnum<vi>, "MMNext":refnum<vi>, "Rot Ver":refnum<vi>, "Rotary Module Selection":refnum<vi>, "calculate rotary":refnum<vi>, "SPEED SELECTION : rotary":refnum<vi>, "Import 2":refnum<vi>, "Save 2":refnum<vi>, "File Path :  2":refnum<vi>, "String 45":refnum<vi>, "StepTable For Speed 3":refnum<vi>, "Enter the Speed(mm/sec)":refnum<vi>, "Enter the Speed(RPM)":refnum<vi>, "Enter Scratch Speed (mm/s):":refnum<vi>, "SwaySpeed Set":refnum<vi>, "Scartch Offset":refnum<vi>, "Motion type:":refnum<vi>, "HomeScratch 2":refnum<vi>, "Enter Scratch length (mm):":refnum<vi>, "Wear Track Diameter":refnum<vi>, "Rotary Speed Exced":refnum<vi>, "Scratch Mode":refnum<vi>, "No of Scratch":refnum<vi>}, "Environmental control":cluster{"Humidity  Status  3":refnum<vi>, "Low Temp  Status  2":refnum<vi>, "TK4 status 2":refnum<vi>, "Stage Temperature":refnum<vi>, "Sample Temperature":refnum<vi>, "Humidity (Amb)":refnum<vi>, "Clear List":refnum<vi>, "Add to list":refnum<vi>, "Wear":refnum<vi>, "Vibration":refnum<vi>, "Humidity (Chamber)":refnum<vi>, "Temperature (Chamber)":refnum<vi>, "ECR ":refnum<vi>, "Temperature (Amb)":refnum<vi>, "Microphone":refnum<vi>, "Acoustic Emission 3":refnum<vi>, "SNext":refnum<vi>, "APBack":refnum<vi>, "Enter the Temperature (°C):":refnum<vi>, "Enter the Stage \nTemperature (°C):":refnum<vi>, "Enter the Humidity (%Rh):":refnum<vi>, "Low Temp":refnum<vi>, "High Temp":refnum<vi>, "Humidity":refnum<vi>, "Sensors Picked":refnum<vi>}, "About Screen":cluster{"Password":refnum<vi>, "Home Service":refnum<vi>, "Advanced Setting":refnum<vi>, "About Tab":refnum<vi>, "ECR Port:":refnum<vi>, "Ramp Port:":refnum<vi>, "Installation/Replacement completed":refnum<vi>, "Loahead":refnum<vi>, "Heave and Surge COM Port:":refnum<vi>, "Sway COM Port:":refnum<vi>, "Temp Modbus:":refnum<vi>, "Humidity Port:":refnum<vi>, "Edit Gain Constants":refnum<vi>, "Save Gain Constants":refnum<vi>}, "Main Screen":cluster{"Main Screen Tab":refnum<vi>, "Angle and Frequency":refnum<vi>, "Stroke (mm)":refnum<vi>, "Angle (Deg)":refnum<vi>, "Main Speed Tab":refnum<vi>, "MTM MOTOR DISPLAY":refnum<vi>, "Disc Speed (m/sec)":refnum<vi>, "Ball Speed (m/sec)":refnum<vi>, "Disc Speed (RPM)":refnum<vi>, "Ball Speed (RPM)":refnum<vi>, "SPEED TAB":refnum<vi>, "Speed (m/sec)":refnum<vi>, "Set Speed (m/sec)":refnum<vi>, "Speed (RPM)":refnum<vi>, "Set Speed":refnum<vi>, "Time Tab":refnum<vi>, "Time ( HH:MM:SS ) 2":refnum<vi>, "Test Duration":refnum<vi>, "Test Duration 4":refnum<vi>, "TEST CYCLE":refnum<vi>, "TOTAL CYCLES":refnum<vi>, "Set Load (N)":refnum<vi>, "Temp Tabs":refnum<vi>, "Heater":refnum<vi>, "TK4 status":refnum<vi>, "ChamberTemp":refnum<vi>, "SetTmp":refnum<vi>, "Controller  Status":refnum<vi>, "ChamberTemp 2":refnum<vi>, "SetTmp 2":refnum<vi>, "Controller  Status 2":refnum<vi>, "ChamberTemp 3":refnum<vi>, "SetTmp 3":refnum<vi>, "Cooling":refnum<vi>, "Load Communication":refnum<vi>, "Ambient \nTemperature":refnum<vi>, "HumCOMStatus":refnum<vi>, "Ambient\n Humidity":refnum<vi>, "Freq (Hz)":refnum<vi>, "Load En":refnum<vi>, "NLt":refnum<vi>, "zNL 2":refnum<vi>, "Humidity On":refnum<vi>, "humidity disp":refnum<vi>, "Set Humidity":refnum<vi>, "NL disp 2":refnum<vi>, "Humidity On 2":refnum<vi>, "humidity disp 2":refnum<vi>, "Set Humidity 2":refnum<vi>, "NL disp 3":refnum<vi>, "AppLoadSeq scratch":refnum<vi>, "Stop Scratch":refnum<vi>, "ClrLog":refnum<vi>, "Trip Log":refnum<vi>, "STOP":refnum<vi>, "Start Test":refnum<vi>, "Test status":refnum<vi>, "AR Led":refnum<vi>, "Data":refnum<vi>, "Health":refnum<vi>, "Sway COM Status":refnum<vi>, "Heave COM Status":refnum<vi>, "Grp Tab":refnum<vi>, "Sub Graph":refnum<vi>, "SD (mm)":refnum<vi>, "Siliding distance Reset Graph":refnum<vi>, "SDGp":refnum<vi>, "Humidity Reset Graph":refnum<vi>, "HumrGp":refnum<vi>, "Acoustic Emission (mV)":refnum<vi>, "Aqucostic Reset Graph":refnum<vi>, "gACQUOS":refnum<vi>, "ECR RESET":refnum<vi>, "ECR":refnum<vi>, "Temperature Reset":refnum<vi>, "Acoustic Emission (mV) 2":refnum<vi>, "Aqucostic Reset Graph 2":refnum<vi>, "gACQUOS 2":refnum<vi>, "ECR RESET 2":refnum<vi>, "ECR 2":refnum<vi>, "Temperature Reset 2":refnum<vi>, "Temperature (deg c)":refnum<vi>, "Speed Reset Graph":refnum<vi>, "Speed Tab":refnum<vi>, "MTM DISC  SPEED":refnum<vi>, "MTM BALL SPEED":refnum<vi>, "speed mm/sec":refnum<vi>, "Hymidity":refnum<vi>, "Humidity Disable trip":refnum<vi>, "CoF Trip  2":refnum<vi>, "Depth Trip":refnum<vi>, "Weart Deapth":refnum<vi>, "Depth Reset Graph":refnum<vi>, "Weart":refnum<vi>, "Depthz":refnum<vi>, "Depth (µm)":refnum<vi>, "WearGp":refnum<vi>, "NL Trip 2":refnum<vi>, "Load pid":refnum<vi>, "Load Disable Trip":refnum<vi>, "Load Reset Graph":refnum<vi>, "NL Display 4":refnum<vi>, "Main Chart 3":refnum<vi>, "BACK":refnum<vi>, "Depth Trip 2":refnum<vi>, "COF TRIP ":refnum<vi>, "Friction Force (N)":refnum<vi>, "FF Reset Graph":refnum<vi>, "FF Disable Trip":refnum<vi>, "FF TRIP":refnum<vi>, "COF Disable Trip":refnum<vi>, "COF Reset Graph":refnum<vi>, "Start Test Temp":refnum<vi>, "zFF":refnum<vi>, "Friction Force (N) Graph":refnum<vi>, "Coefficient of Friction":refnum<vi>, "Scratch Start Test":refnum<vi>, "FF Tab":refnum<vi>, "Cyclic Friction Force (N)":refnum<vi>, "CZ FF":refnum<vi>, "Cyclic Friction Force (N) Graph":refnum<vi>, "Cyclic Coefficient of Friction":refnum<vi>, "Cyclic FF TRIP":refnum<vi>, "Cyclic FF Disable Trip":refnum<vi>, "cyclic COF Disable Trip":refnum<vi>, "cyclic COF TRIP":refnum<vi>, "cyclic COF Reset Graph":refnum<vi>, "Cyclic FF Reset Graph":refnum<vi>, "Test Trip":refnum<vi>, "Multi Scratch Pass":refnum<vi>, "Scratch Start Recording":refnum<vi>}, "Loading":cluster{"Indentation":refnum<vi>, "Reference Sample":refnum<vi>, "Load Cell Communication Slide":refnum<vi>, "com 3":refnum<vi>, "com":refnum<vi>, "DecaForce COM Status":refnum<vi>, "Update":refnum<vi>, "Clear 3":refnum<vi>, "seq":refnum<vi>, "Stribeck table":refnum<vi>, "Stribeck Table  For loading":refnum<vi>, "Loading Mode":refnum<vi>, "Enter the Final Load (N)":refnum<vi>, "Enter the CoF Trip":refnum<vi>, "Enter the Friction Force Trip":refnum<vi>, "Enter the Normal load Trip":refnum<vi>, "Enter the Load  (N)":refnum<vi>, "KiloForce":refnum<vi>, "DecaForce ":refnum<vi>, "MicroForce":refnum<vi>, "LHBack":refnum<vi>, "LHNext":refnum<vi>, "Enter the Loading Rate (N/min)":refnum<vi>, "Message":refnum<vi>, "Warning 2":refnum<vi>, "SSP 0.75":refnum<vi>, "SSP 0.5":refnum<vi>, "SSP 0.3":refnum<vi>, "Warning":refnum<vi>, "gui GIF":refnum<vi>, "Communication is established":refnum<vi>, "AppLoad 4":refnum<vi>, "Multipoint":refnum<vi>, "Load Selection":refnum<vi>}, "PID":cluster{"Ramp MulFac":refnum<vi>, "pulses LoadDiffRamp(2..10)":refnum<vi>, "PulseControlRamp(diff<=3N)":refnum<vi>, "SetLoadDeadband(%) Load(0-10N)":refnum<vi>, "PID gains out delay (microForce)":refnum<vi>, "Ramp":refnum<vi>, "Gain 2":refnum<vi>, "pulses LoadDiff(2..10)":refnum<vi>, "pulses LoadDiff(11..50)":refnum<vi>, "PulseControl(diff<=3N)":refnum<vi>, "SetLoadDeadband(%)  2":refnum<vi>, "Dummy Run":refnum<vi>, "Vertical load (N)":refnum<vi>, "AutoTune":refnum<vi>, "Offset 3 ":refnum<vi>, "apply load":refnum<vi>, "Offset  3":refnum<vi>, "apply load 2":refnum<vi>, "Enter ByPass Load":refnum<vi>, "reinit 3":refnum<vi>, "output range delay":refnum<vi>, "PID gains out delay":refnum<vi>, "Bypass Load":refnum<vi>, "pulsesSent":refnum<vi>, "pulses ":refnum<vi>, "actpid":refnum<vi>, "gFF Rot":refnum<vi>, "pulses LoadDiff(21..1000)":refnum<vi>, "Delay":refnum<vi>, "deadband":refnum<vi>}, "Config Parameters":cluster{"Tab Control 3":refnum<vi>, "Tab Control 19":refnum<vi>, "SAMPLES":refnum<vi>, "Re-initilaize":refnum<vi>, "Filter ON/OFF":refnum<vi>, "TracHomeSurgeOffsetCounts 10MM":refnum<vi>, "TracHomeSwayOffsetCounts 10MM":refnum<vi>, "Acoustic Emission:":refnum<vi>, "Apply Filter (FF)":refnum<vi>, "Filter% 2":refnum<vi>, "Apply Filter (Load)":refnum<vi>, "Filter% ":refnum<vi>, "Sway distance (mm)":refnum<vi>, "Surge distance (mm)":refnum<vi>, "DataSavingLoopDelay(ms)":refnum<vi>, "SAVE 2":refnum<vi>, "Enter Distance":refnum<vi>, "Sway Counts:":refnum<vi>, "Distance (mm): 3":refnum<vi>, "Surge Counts:":refnum<vi>, "Distance (mm): 2":refnum<vi>, "Distance (mm):":refnum<vi>, "Heave Counts:":refnum<vi>, "LRMHomeSurgeOffsetCounts":refnum<vi>, "LRMHomeSwayOffsetCounts":refnum<vi>, "TracHomeSurgeOffsetCounts 20MM":refnum<vi>, "TracHomeSwayOffsetCounts 20MM":refnum<vi>, "RotHomeSwayOffsetCounts":refnum<vi>, "RotHomeSurgeOffsetCounts":refnum<vi>, "Heave distance":refnum<vi>, "Zmm":refnum<vi>, "Heave Pulses/mm":refnum<vi>, "Surge Pulses/mm":refnum<vi>, "Sway Pulses/mm":refnum<vi>, "Heave Pitch":refnum<vi>, "Surge Pitch":refnum<vi>, "Sway Pitch":refnum<vi>, "Heave PPR":refnum<vi>, "Surge PPR":refnum<vi>, "Sway PPR":refnum<vi>, "Tab Control 5":refnum<vi>, "Tab Control 14":refnum<vi>, "Tab Control 26":refnum<vi>, "AE":refnum<vi>, "Heave Loop Delay":refnum<vi>, "Heave PID Speed":refnum<vi>, "Surge Jog Speed":refnum<vi>, "Heave Jog Speed":refnum<vi>, "Sway Loop Delay":refnum<vi>, "Sway PID Speed":refnum<vi>, "Sway Jog Speed":refnum<vi>, "DEPTH TRIP VALUE":refnum<vi>, "LOAD TRIP VALUE":refnum<vi>, "DEPTH TRIP   ENABLE":refnum<vi>, "LOAD TRIP  ENABLE":refnum<vi>, "CYCLIC FF TRIP VALUE":refnum<vi>, "FF TRIP VALUE":refnum<vi>, "CYCLIC CoF TRIP VALUE":refnum<vi>, "COF TRIP VALUE":refnum<vi>, "CYCLIC COF TRIP  ENABLE":refnum<vi>, "CYCLIC FF TRIP  ENABLE":refnum<vi>, "FF TRIP  ENABLE":refnum<vi>, "COF TRIP  ENABLE":refnum<vi>}, "Loading Com Port":cluster{"ClearAll":refnum<vi>, "Mz(Nm)":refnum<vi>, "My(Nm)":refnum<vi>, "Mx(Nm)":refnum<vi>, "Save Dwell":refnum<vi>, "Mx ":refnum<vi>, "My ":refnum<vi>, "Mz":refnum<vi>, "Fx(N)":refnum<vi>, "Fy(N)":refnum<vi>, "Fz(N)":refnum<vi>, "ZeroAll":refnum<vi>, "Acq Delay (ms)":refnum<vi>, "Burst Delay (ms)":refnum<vi>, "model":refnum<vi>, "SN":refnum<vi>, "FFx(N)":refnum<vi>, "Sensor IP":refnum<vi>, "Port":refnum<vi>, "FFy(N)":refnum<vi>, "Load(N)":refnum<vi>, "delete Handle":refnum<vi>, "Create Handle":refnum<vi>, "ft_data":refnum<vi>, "ft_range":refnum<vi>, "ft_data 2":refnum<vi>, "stop 6":refnum<vi>, "running_flag":refnum<vi>, "ft_udp_handle":refnum<vi>, "get-data-return":refnum<vi>, "get-range-return":refnum<vi>, "zero-return":refnum<vi>, "filter-return":refnum<vi>, "initial-return":refnum<vi>, "deleteHandle-result":refnum<vi>, "Load Cell Temp":refnum<vi>}, "Heave AND Surge":cluster{"SURGE POSE":refnum<vi>, "error out Read":refnum<vi>, "HEAVE POSE":refnum<vi>, "State":refnum<vi>, "Homed":refnum<vi>, "Sequence ID":refnum<vi>, "error out Write":refnum<vi>, "faultCode":refnum<vi>, "Ack ID":refnum<vi>, "SPEED":refnum<vi>, "Distance":refnum<vi>, "Mode Command":refnum<vi>, "Heave and Surge Read":refnum<vi>, "Read Heave Temp":refnum<vi>, "Spare 15":refnum<vi>, "Spare 14":refnum<vi>, "Spare 13":refnum<vi>, "Spare 12":refnum<vi>, "Spare 11":refnum<vi>, "Spare 10":refnum<vi>, "Spare 9":refnum<vi>, "Spare 8":refnum<vi>, "Spare 7":refnum<vi>, "Spare 6":refnum<vi>, "Spare 5":refnum<vi>, "Spare 4":refnum<vi>, "Spare 2":refnum<vi>, "Spare 1":refnum<vi>, "Node Id":refnum<vi>, "Spare 3":refnum<vi>, "SPARE 4":refnum<vi>, "SPARE 3":refnum<vi>, "SPARE 2":refnum<vi>, "SPARE 1":refnum<vi>, "fwMajor":refnum<vi>, "fwMinor":refnum<vi>, "Manual Write":refnum<vi>, "Heave and Surge Write":refnum<vi>}, "New PID LOGIC":cluster{"Fine Tune Zone":refnum<vi>, "PID SDelay":refnum<vi>, "Max_pos_limit":refnum<vi>, "Min_pos_limit":refnum<vi>, "i_limit":refnum<vi>, "pct_scale":refnum<vi>, "Deadband":refnum<vi>, "Kd":refnum<vi>, "Ki":refnum<vi>, "Kp":refnum<vi>, "Current Position":refnum<vi>, "Set Load":refnum<vi>, "Current Load":refnum<vi>, "Pulse delta":refnum<vi>, "Init Step":refnum<vi>, "Max Step Linit":refnum<vi>}, "SWAY ":cluster{"fwMajor":refnum<vi>, "Homed":refnum<vi>, "Rotary POSE":refnum<vi>, "State":refnum<vi>, "SWAY POSE":refnum<vi>, "Ack ID":refnum<vi>, "faultCode":refnum<vi>, "Node Id":refnum<vi>, "fwMinor":refnum<vi>, "Spare 6":refnum<vi>, "Spare 5":refnum<vi>, "Spare 4":refnum<vi>, "Spare 3":refnum<vi>, "Spare 2":refnum<vi>, "Spare 1":refnum<vi>, "Spare 7":refnum<vi>, "SPARE  5":refnum<vi>, "error out Write  SWAY ":refnum<vi>, "error out Read SWAY ":refnum<vi>, "Manual Write SWAY ":refnum<vi>, "SWAY WRITE":refnum<vi>, "SPARE  4":refnum<vi>, "SPARE  3":refnum<vi>, "SPARE 2":refnum<vi>, "SPARE 1":refnum<vi>, "Spare 15":refnum<vi>, "Spare 14":refnum<vi>, "Spare 13":refnum<vi>, "Spare 12":refnum<vi>, "Spare 11":refnum<vi>, "Spare 9":refnum<vi>, "Spare 8":refnum<vi>, "SPEED":refnum<vi>, "Distance":refnum<vi>, "Mode Command":refnum<vi>, "Sequence ID":refnum<vi>, "SWAY READ":refnum<vi>, "Spare 10":refnum<vi>, "Read SWAY Temp":refnum<vi>}, "Analysis Screen":cluster{"Analysis Home":refnum<vi>, "Refresh 2":refnum<vi>, "MEAN 4":refnum<vi>, "SD 4":refnum<vi>, "VARIANCE 4":refnum<vi>, "MEAN  3":refnum<vi>, "SD  3":refnum<vi>, "VARIANCE  3":refnum<vi>, "MEAN 2":refnum<vi>, "SD  2":refnum<vi>, "VARIANCE 2":refnum<vi>, "MEAN":refnum<vi>, "SD":refnum<vi>, "VARIANCE":refnum<vi>, "File 4 Discription":refnum<vi>, "OPEN 4":refnum<vi>, "File Name 4":refnum<vi>, "OPEN 3":refnum<vi>, "File 3 Discription":refnum<vi>, "File Name 3":refnum<vi>, "Y-AXIS":refnum<vi>, "X-AXIS":refnum<vi>, "XY Graph":refnum<vi>, "File Name 2":refnum<vi>, "File Name 1":refnum<vi>, "OPEN 2":refnum<vi>, "OPEN 1":refnum<vi>, "File 1 Discription ":refnum<vi>, "File 2 Discription":refnum<vi>, "Export":refnum<vi>, "File Format":refnum<vi>}}
  T12 = typedef "init queue out loop.ctl" = cluster{"UI Loop":refnum<queue>, "LOAD COM LOOP ":refnum<queue>, "SWAY MOTOR COM LOOP":refnum<queue>, "HEAVE MOTOR COM LOOP":refnum<queue>, "TEMPERATURE COM LOOP":refnum<queue>, "RAMP MOTOR COM LOOP":refnum<queue>, "ECR PORT":refnum<queue>, "HUMIDITY COM PORT":refnum<queue>, "PROGRAM LOOP":refnum<queue>, "MONITOR LOOP":refnum<queue>, "REPORT":refnum<queue>, "LOAD PID":refnum<queue>}
  T13 = typedef "XDNodeRunTimeDep.lvlib/timing_clust.ctl" = cluster{"Expected End [f-1]":u64, "Actual End [f-1]":u64, "Finished Late? [f-1]":bool, "Expected End [i-1]":u64, "Actual End [i-1]":u64, "Finished Late? [i-1]":bool, "Expected Start [i]":u64, "Actual Start [i]":u64, "Expected Start [f]":u64, "Actual Start [f]":u64, "Source Name":string, "Structure Name":string, "Period":i64, "Deadline":i64, "Offset":i64, "Start":i64, "Priority":i32, "Timeout":i32, "Mode":T14, "Wakeup Reason":T15, "Error":errorcluster, "Source Type":string, "Secondary Source Type":string, "Global End Time":u64, "Global Start Time":u64, "Frame Duration":u64, "Iteration Duration":u64, "Assigned CPU":i32, "I/O Scan Engine Mode":u32}
  T14 = typedef "XDNodeRunTimeDep.lvlib/nitl_modes.ctl" = enum32{"No Change", "Process missed periods, maintain original phase", "Discard missed periods, maintain original phase", "Process missed periods, ignore original phase", "Discard missed periods, ignore original phase"}
  T15 = typedef "XDNodeRunTimeDep.lvlib/wakeup.ctl" = enum32{"Normal", "Aborted", "Asynchronous wakeup", "Timing source error", "Timed loop error", "Timeout"}
  T16 = enum8{"Enabled", "Disabled", "Disabled and Grayed Out"}
  T17 = enum16{"INIT", "SETLOWPASSFILTER", "SETZERO", "GETSENSORINFO", "GETRANGE", "ZEROALL", "READDATA", "UNINITIAL", "DELETEHANDLE"}
  T18 = typedef "Heave Write enum.ctl" = enum16{"INIT", "READ", "WRITE", "CLOSE", "REINIT"}
  T19 = typedef "Sway Write enum.ctl" = enum16{"INIT", "READ", "WRITE", "CLOSE", "REINIT"}
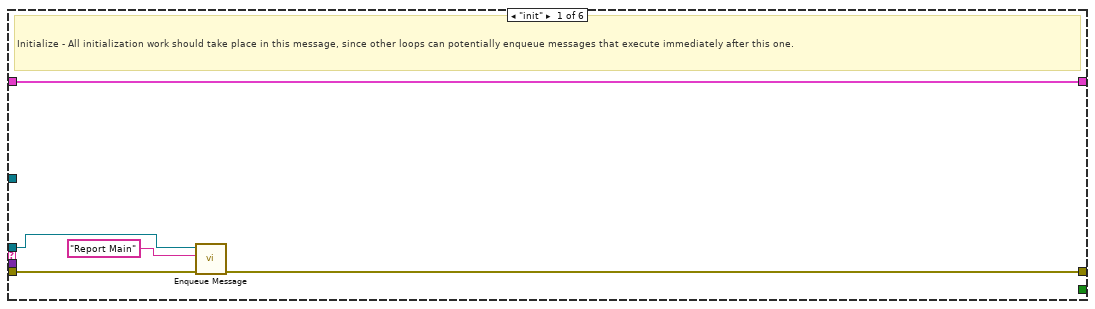
[diagram p2: hidden frame]
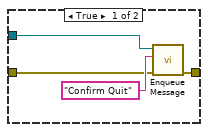
[diagram p3: hidden frame]
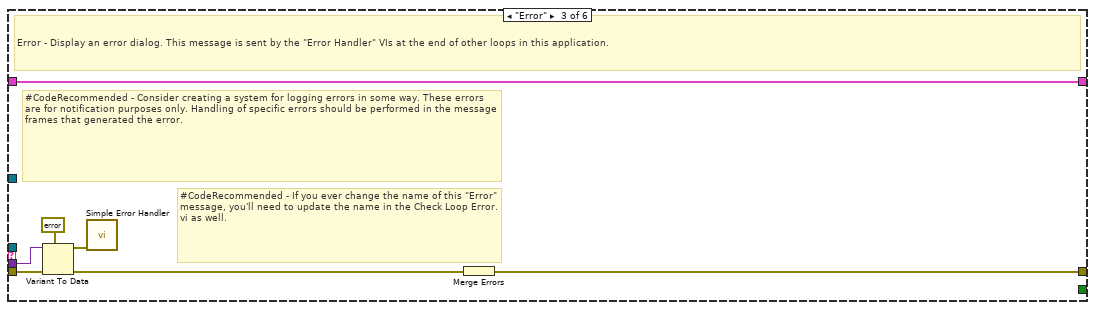
[diagram p4: hidden frame]
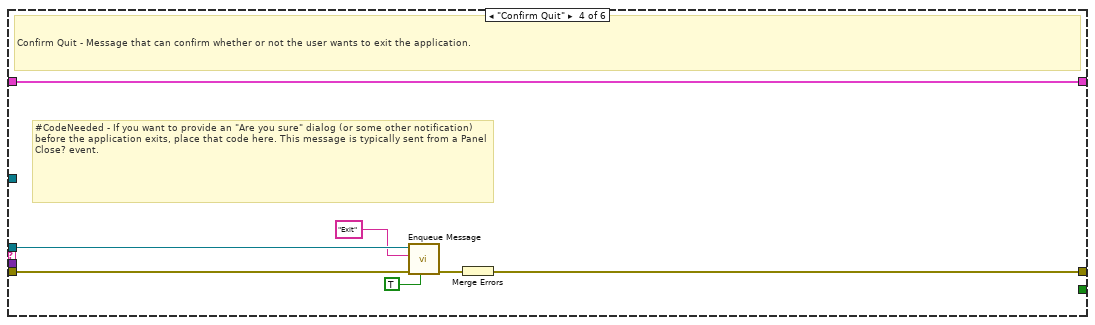
[diagram p5: hidden frame]
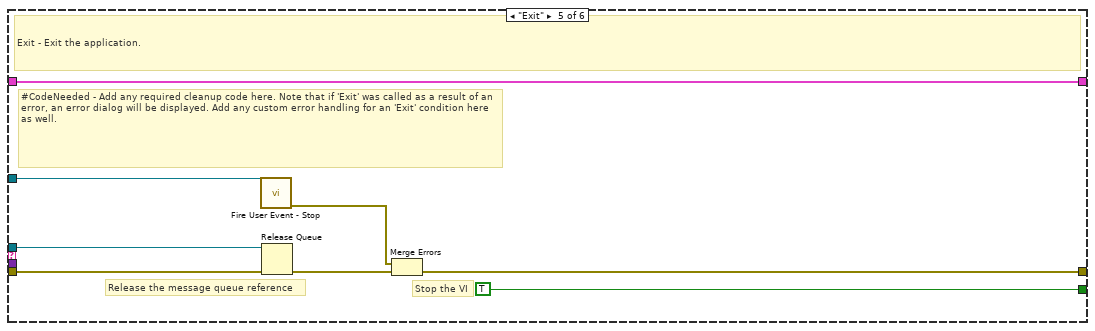
[diagram p6: hidden frame]
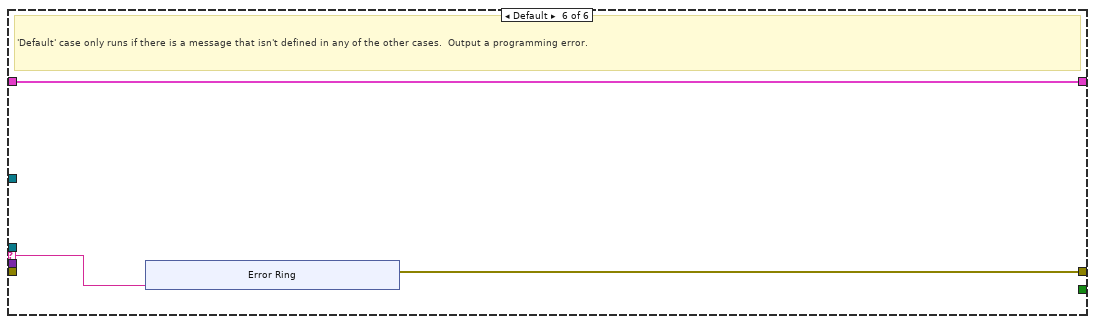
[diagram p7: hidden frame]
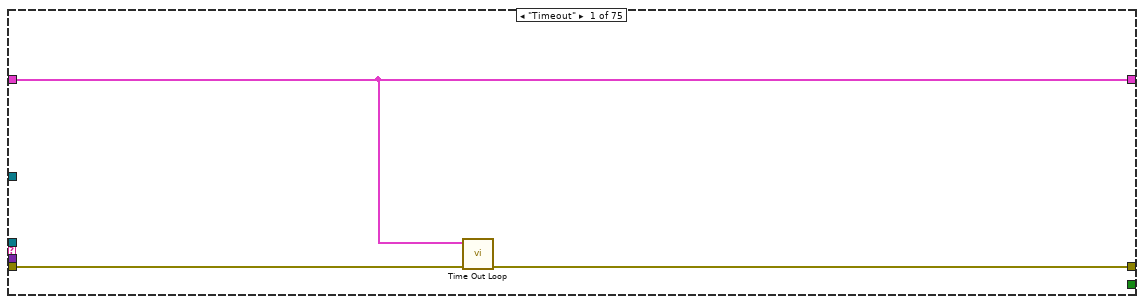
[diagram p9: hidden frame]
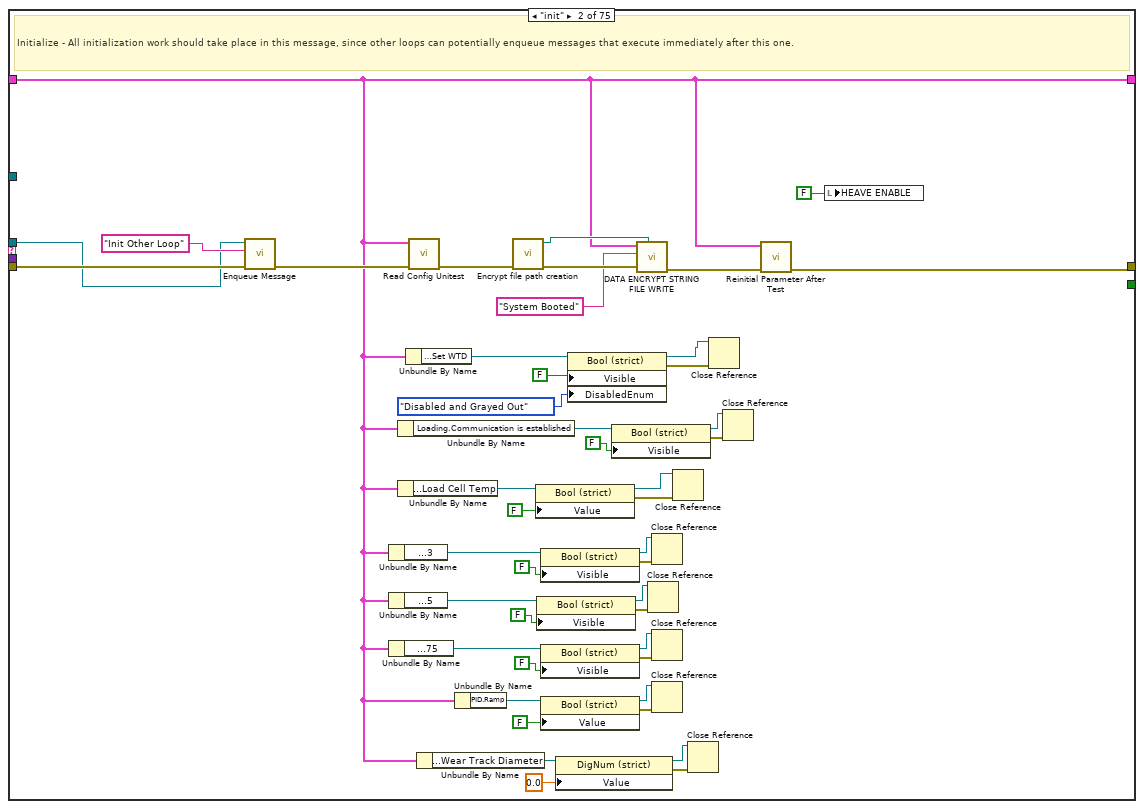
[diagram p10: hidden frame]
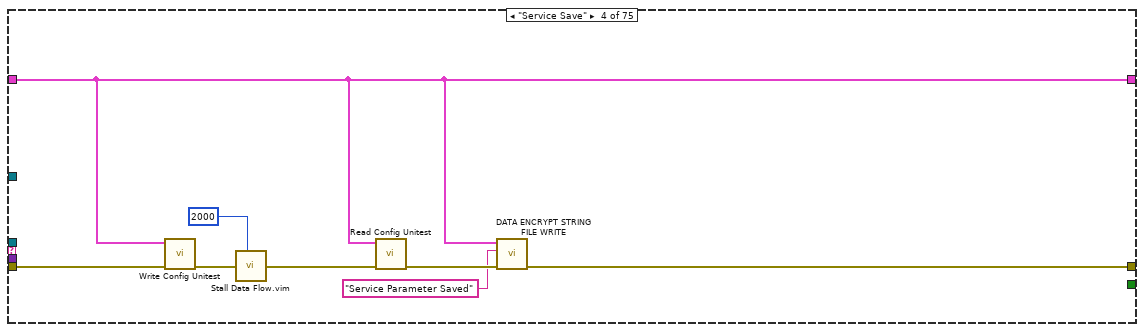
[diagram p12: hidden frame]
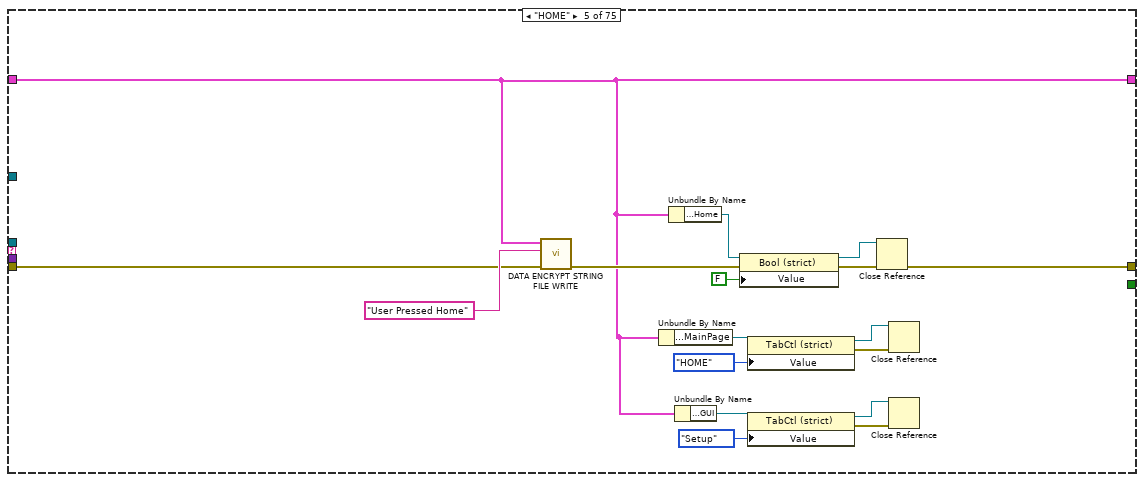
[diagram p13: hidden frame]
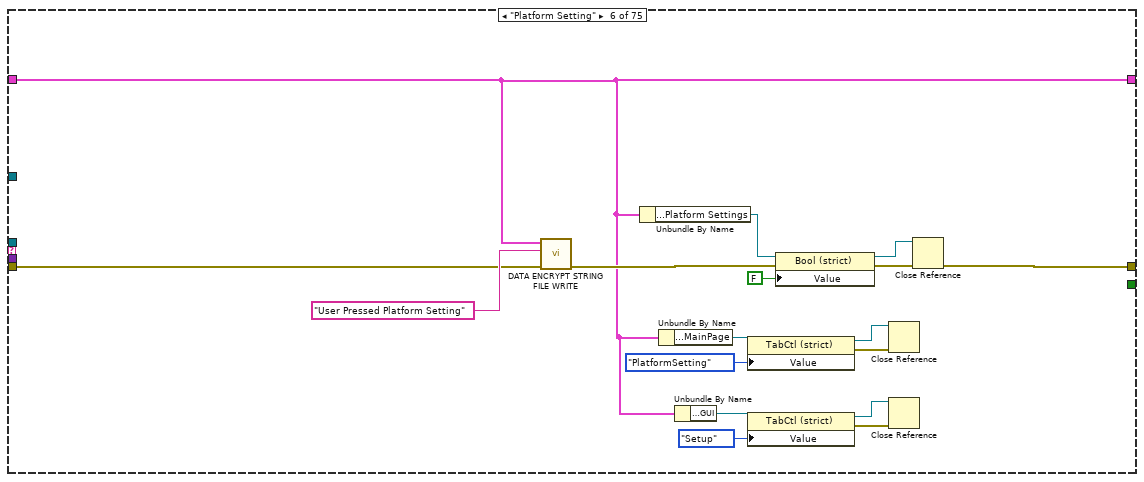
[diagram p14: hidden frame]
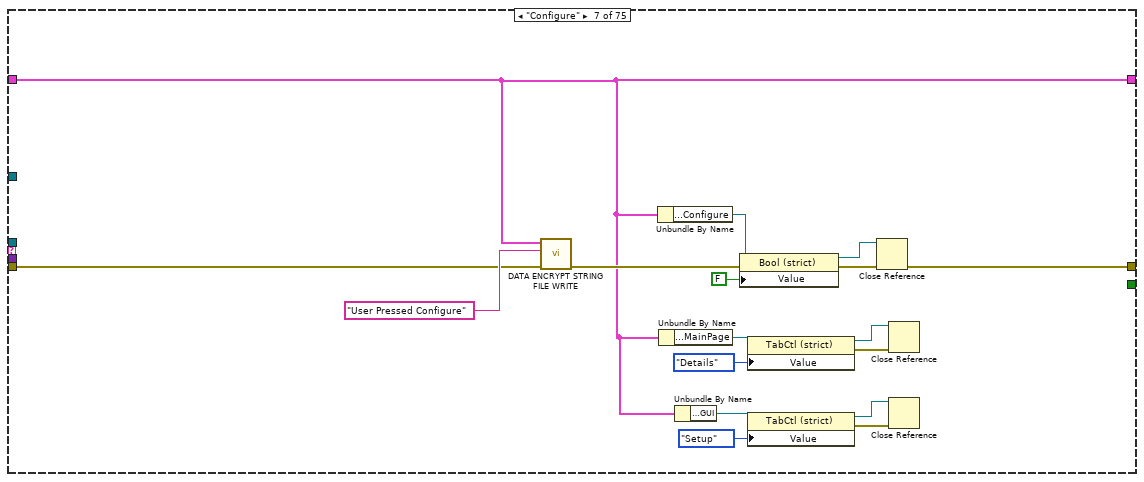
[diagram p15: hidden frame]
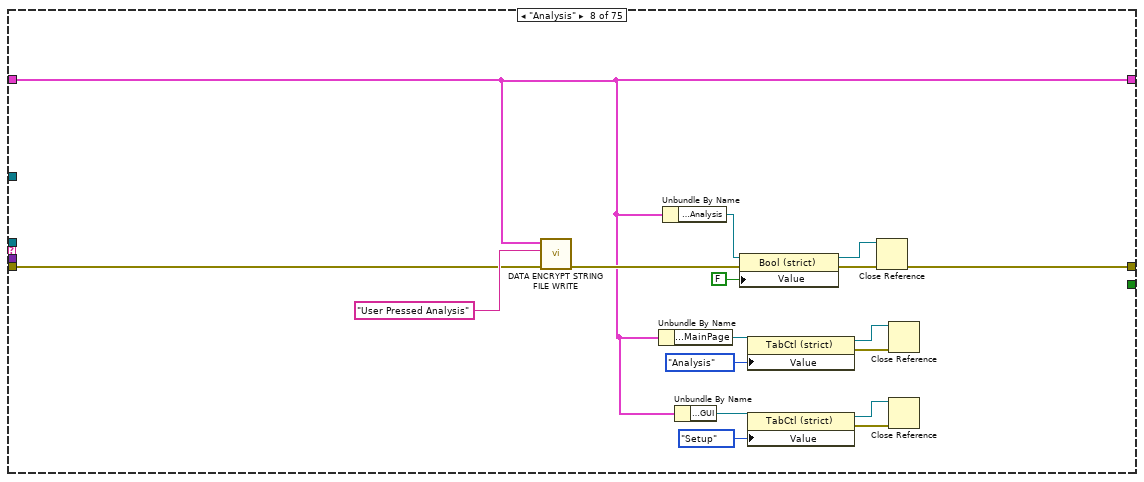
[diagram p16: hidden frame]
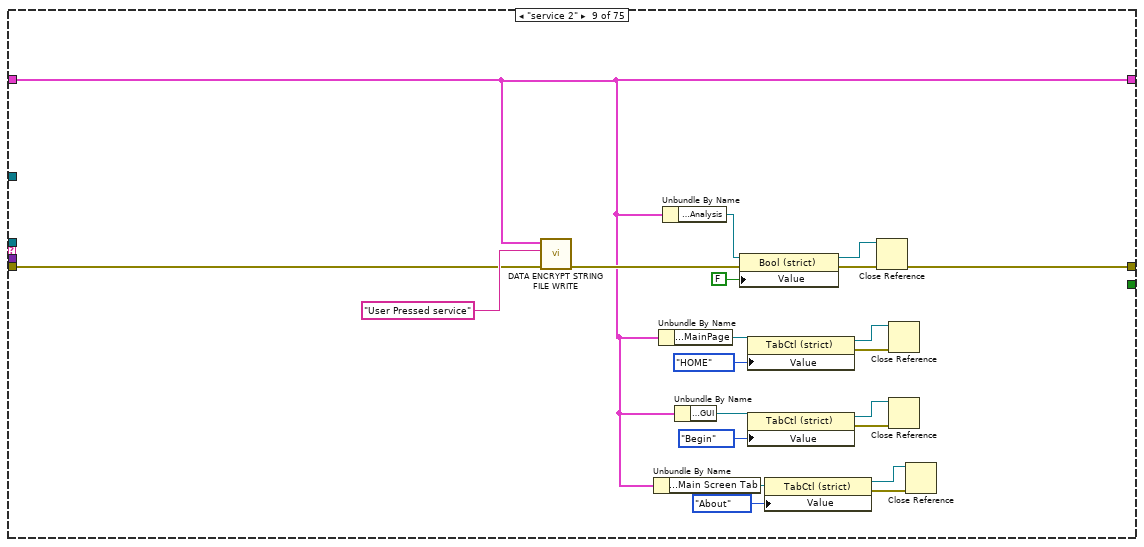
[diagram p17: hidden frame]
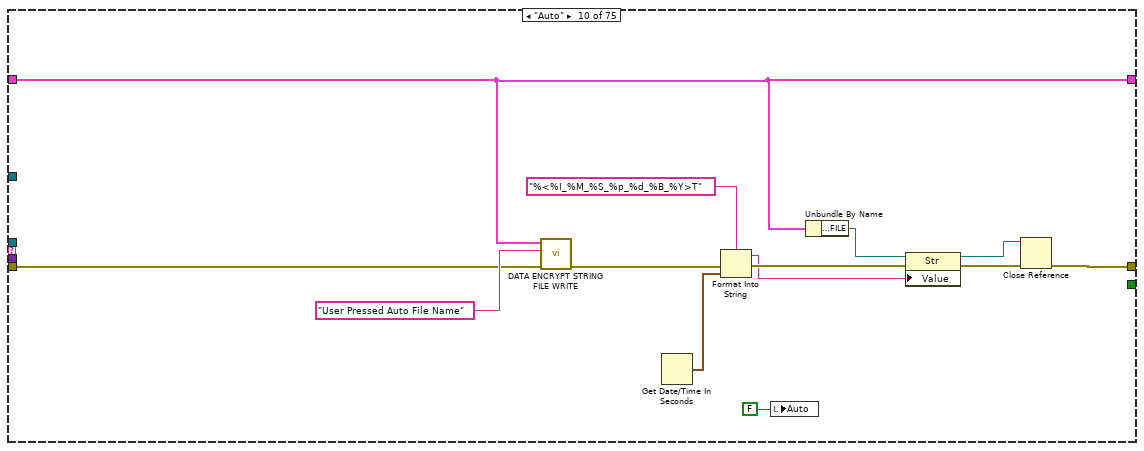
[diagram p18: hidden frame]
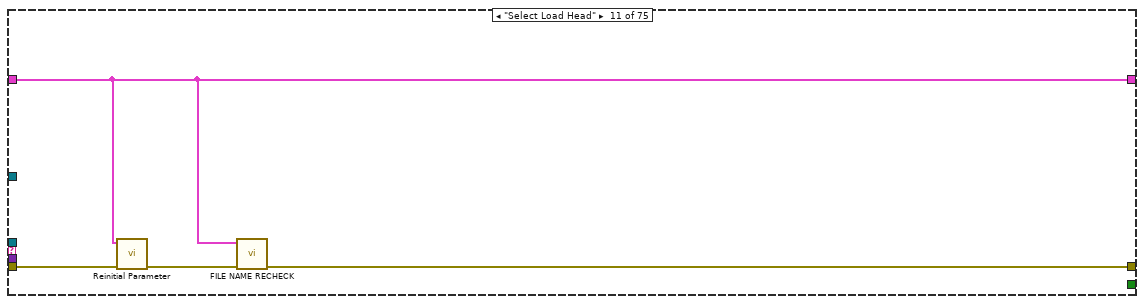
[diagram p19: hidden frame]
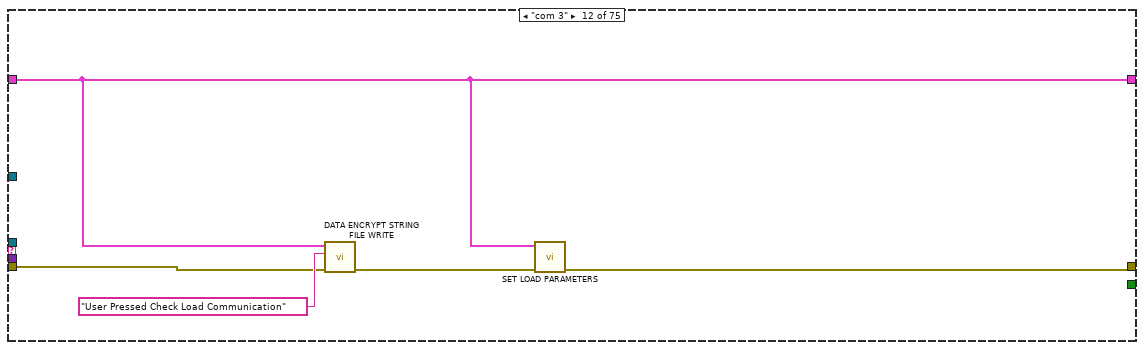
[diagram p20: hidden frame]
diagram:
  w1 = 0.0 ("prev_error_out")
  n1 = flat-sequence {
    tunnel: [w67] -> w54
    tunnel: T11 {"Main Home Screen"={"GUI"=refnum, "Platform Settings"=refnum, "Configure"=refnum, "Home"=refnum, "EXIT"=refnum, "service 2"=refnum, "MainPage"=refnum, "Analysis"=refnum}, "Platform Settings"={"mm/s  Surge"=refnum, "Update Surge Speed"=refnum, "Drive Error"=refnum, "Disable Axis Jog Soft Limits"=refnum, "mm/s  Sway"=refnum, "Sway and Surge COM Status"=refnum, "Heave COM Status"=refnum, "Enable Platform"=refnum, "Surge Forward Main"=refnum, "Sway Right Main"=refnum, "Sway Left Main"=refnum, "Heave Down Main"=refnum, "Heave Up main"=refnum, "Update Sway Speed"=refnum, "Update Heave Speed"=refnum, "mm/s Heave"=refnum, "mm/sec"=refnum, "mm"=refnum, "Surge Backward Main"=refnum}, "Analysis Screen"={"Analysis Home"=refnum, "Surface Analysis"=refnum, "Imaging"=refnum, "Image Analysis"=refnum, "Post Analysis"=refnum}, "Config Screen"={"Select Load Head"=refnum, "Notes :"=refnum, "FILE"=refnum, "Sample ID :"=refnum, "Operator ID :"=refnum, "Operator Name :"=refnum, "Auto"=refnum}, "Motion Module"={"zNL"=refnum, "NL disp"=refnum, "Rotary Tab"=refnum, "Motion Direction:  3"=refnum, "E.Velocity 2"=refnum, "e.v/ssr 2"=refnum, "Enter Fixed E.Velocity 2"=refnum, "Enter Final SRR 2"=refnum, "Enter initial SRR 2"=refnum, "Enter Fixed SRR 2"=refnum, "Enter the Final E.Velocity (m/s) 2"=refnum, "Enter initial E.Velocity (m/s) 2"=refnum, "Final Speed (RPM) 3"=refnum, "Initial Speed (RPM) 2"=refnum, "Enter the Final Velocity (m/s) 3"=refnum, "Enter initial Velocity (m/s)  3"=refnum, "Ramp Up 2"=refnum, "TEST SELECTION"=refnum, "SPEED SELECTION : "=refnum, "Angular Oscillation Set"=refnum, "Traction"=refnum, "Step Speed"=refnum, "StepTable For Load-Speed"=refnum, "StepTable For Speed"=refnum, "Surge Forward MM"=refnum, "Surge Backward MM"=refnum, "M3 Image"=refnum, "String 39"=refnum, "Sway Left MM"=refnum, "Sway Right MM"=refnum, "Disable Axis Jog Soft Limits"=refnum, "mm"=refnum, "Heave Down MM"=refnum, "Heave Up MM"=refnum, "Wear Track Diameter (mm)"=refnum, "Set WTD"=refnum, "HomeScratch"=refnum, "HomeRot"=refnum, "PlaceModule"=refnum, "Enter the Angle (Deg)"=refnum, "Enter the Frequency (Hz)"=refnum, "Motion Mode:"=refnum, "LR Sway"=refnum, "Rot Hor"=refnum, "Scratch"=refnum, "LR Cam"=refnum, "MMBack"=refnum, "MMNext"=refnum, "Rot Ver"=refnum, "Rotary Module Selection"=refnum, "calculate rotary"=refnum, "SPEED SELECTION : rotary"=refnum, "Import 2"=refnum, "Save 2"=refnum, "File Path :  2"=refnum, "String 45"=refnum, "StepTable For Speed 3"=refnum, "Enter the Speed(mm/sec)"=refnum, "Enter the Speed(RPM)"=refnum, "Enter Scratch Speed (mm/s):"=refnum, "SwaySpeed Set"=refnum, "Scartch Offset"=refnum, "Motion type:"=refnum, "HomeScratch 2"=refnum, "Enter Scratch length (mm):"=refnum, "Wear Track Diameter"=refnum, "Rotary Speed Exced"=refnum, "Scratch Mode"=refnum, "No of Scratch"=refnum}, "Environmental control"={"Humidity  Status  3"=refnum, "Low Temp  Status  2"=refnum, "TK4 status 2"=refnum, "Stage Temperature"=refnum, "Sample Temperature"=refnum, "Humidity (Amb)"=refnum, "Clear List"=refnum, "Add to list"=refnum, "Wear"=refnum, "Vibration"=refnum, "Humidity (Chamber)"=refnum, "Temperature (Chamber)"=refnum, "ECR "=refnum, "Temperature (Amb)"=refnum, "Microphone"=refnum, "Acoustic Emission 3"=refnum, "SNext"=refnum, "APBack"=refnum, "Enter the Temperature (°C):"=refnum, "Enter the Stage \nTemperature (°C):"=refnum, "Enter the Humidity (%Rh):"=refnum, "Low Temp"=refnum, "High Temp"=refnum, "Humidity"=refnum, "Sensors Picked"=refnum}, "About Screen"={"Password"=refnum, "Home Service"=refnum, "Advanced Setting"=refnum, "About Tab"=refnum, "ECR Port:"=refnum, "Ramp Port:"=refnum, "Installation/Replacement completed"=refnum, "Loahead"=refnum, "Heave and Surge COM Port:"=refnum, "Sway COM Port:"=refnum, "Temp Modbus:"=refnum, "Humidity Port:"=refnum, "Edit Gain Constants"=refnum, "Save Gain Constants"=refnum}, "Main Screen"={"Main Screen Tab"=refnum, "Angle and Frequency"=refnum, "Stroke (mm)"=refnum, "Angle (Deg)"=refnum, "Main Speed Tab"=refnum, "MTM MOTOR DISPLAY"=refnum, "Disc Speed (m/sec)"=refnum, "Ball Speed (m/sec)"=refnum, "Disc Speed (RPM)"=refnum, "Ball Speed (RPM)"=refnum, "SPEED TAB"=refnum, "Speed (m/sec)"=refnum, "Set Speed (m/sec)"=refnum, "Speed (RPM)"=refnum, "Set Speed"=refnum, "Time Tab"=refnum, "Time ( HH:MM:SS ) 2"=refnum, "Test Duration"=refnum, "Test Duration 4"=refnum, "TEST CYCLE"=refnum, "TOTAL CYCLES"=refnum, "Set Load (N)"=refnum, "Temp Tabs"=refnum, "Heater"=refnum, "TK4 status"=refnum, "ChamberTemp"=refnum, "SetTmp"=refnum, "Controller  Status"=refnum, "ChamberTemp 2"=refnum, "SetTmp 2"=refnum, "Controller  Status 2"=refnum, "ChamberTemp 3"=refnum, "SetTmp 3"=refnum, "Cooling"=refnum, "Load Communication"=refnum, "Ambient \nTemperature"=refnum, "HumCOMStatus"=refnum, "Ambient\n Humidity"=refnum, "Freq (Hz)"=refnum, "Load En"=refnum, "NLt"=refnum, "zNL 2"=refnum, "Humidity On"=refnum, "humidity disp"=refnum, "Set Humidity"=refnum, "NL disp 2"=refnum, "Humidity On 2"=refnum, "humidity disp 2"=refnum, "Set Humidity 2"=refnum, "NL disp 3"=refnum, "AppLoadSeq scratch"=refnum, "Stop Scratch"=refnum, "ClrLog"=refnum, "Trip Log"=refnum, "STOP"=refnum, "Start Test"=refnum, "Test status"=refnum, "AR Led"=refnum, "Data"=refnum, "Health"=refnum, "Sway COM Status"=refnum, "Heave COM Status"=refnum, "Grp Tab"=refnum, "Sub Graph"=refnum, "SD (mm)"=refnum, "Siliding distance Reset Graph"=refnum, "SDGp"=refnum, "Humidity Reset Graph"=refnum, "HumrGp"=refnum, "Acoustic Emission (mV)"=refnum, "Aqucostic Reset Graph"=refnum, "gACQUOS"=refnum, "ECR RESET"=refnum, "ECR"=refnum, "Temperature Reset"=refnum, "Acoustic Emission (mV) 2"=refnum, "Aqucostic Reset Graph 2"=refnum, "gACQUOS 2"=refnum, "ECR RESET 2"=refnum, "ECR 2"=refnum, "Temperature Reset 2"=refnum, "Temperature (deg c)"=refnum, "Speed Reset Graph"=refnum, "Speed Tab"=refnum, "MTM DISC  SPEED"=refnum, "MTM BALL SPEED"=refnum, "speed mm/sec"=refnum, "Hymidity"=refnum, "Humidity Disable trip"=refnum, "CoF Trip  2"=refnum, "Depth Trip"=refnum, "Weart Deapth"=refnum, "Depth Reset Graph"=refnum, "Weart"=refnum, "Depthz"=refnum, "Depth (µm)"=refnum, "WearGp"=refnum, "NL Trip 2"=refnum, "Load pid"=refnum, "Load Disable Trip"=refnum, "Load Reset Graph"=refnum, "NL Display 4"=refnum, "Main Chart 3"=refnum, "BACK"=refnum, "Depth Trip 2"=refnum, "COF TRIP "=refnum, "Friction Force (N)"=refnum, "FF Reset Graph"=refnum, "FF Disable Trip"=refnum, "FF TRIP"=refnum, "COF Disable Trip"=refnum, "COF Reset Graph"=refnum, "Start Test Temp"=refnum, "zFF"=refnum, "Friction Force (N) Graph"=refnum, "Coefficient of Friction"=refnum, "Scratch Start Test"=refnum, "FF Tab"=refnum, "Cyclic Friction Force (N)"=refnum, "CZ FF"=refnum, "Cyclic Friction Force (N) Graph"=refnum, "Cyclic Coefficient of Friction"=refnum, "Cyclic FF TRIP"=refnum, "Cyclic FF Disable Trip"=refnum, "cyclic COF Disable Trip"=refnum, "cyclic COF TRIP"=refnum, "cyclic COF Reset Graph"=refnum, "Cyclic FF Reset Graph"=refnum, "Test Trip"=refnum, "Multi Scratch Pass"=refnum, "Scratch Start Recording"=refnum}, "Loading"={"Indentation"=refnum, "Reference Sample"=refnum, "Load Cell Communication Slide"=refnum, "com 3"=refnum, "com"=refnum, "DecaForce COM Status"=refnum, "Update"=refnum, "Clear 3"=refnum, "seq"=refnum, "Stribeck table"=refnum, "Stribeck Table  For loading"=refnum, "Loading Mode"=refnum, "Enter the Final Load (N)"=refnum, "Enter the CoF Trip"=refnum, "Enter the Friction Force Trip"=refnum, "Enter the Normal load Trip"=refnum, "Enter the Load  (N)"=refnum, "KiloForce"=refnum, "DecaForce "=refnum, "MicroForce"=refnum, "LHBack"=refnum, "LHNext"=refnum, "Enter the Loading Rate (N/min)"=refnum, "Message"=refnum, "Warning 2"=refnum, "SSP 0.75"=refnum, "SSP 0.5"=refnum, "SSP 0.3"=refnum, "Warning"=refnum, "gui GIF"=refnum, "Communication is established"=refnum, "AppLoad 4"=refnum, "Multipoint"=refnum, "Load Selection"=refnum}, "PID"={"Ramp MulFac"=refnum, "pulses LoadDiffRamp(2..10)"=refnum, "PulseControlRamp(diff<=3N)"=refnum, "SetLoadDeadband(%) Load(0-10N)"=refnum, "PID gains out delay (microForce)"=refnum, "Ramp"=refnum, "Gain 2"=refnum, "pulses LoadDiff(2..10)"=refnum, "pulses LoadDiff(11..50)"=refnum, "PulseControl(diff<=3N)"=refnum, "SetLoadDeadband(%)  2"=refnum, "Dummy Run"=refnum, "Vertical load (N)"=refnum, "AutoTune"=refnum, "Offset 3 "=refnum, "apply load"=refnum, "Offset  3"=refnum, "apply load 2"=refnum, "Enter ByPass Load"=refnum, "reinit 3"=refnum, "output range delay"=refnum, "PID gains out delay"=refnum, "Bypass Load"=refnum, "pulsesSent"=refnum, "pulses "=refnum, "actpid"=refnum, "gFF Rot"=refnum, "pulses LoadDiff(21..1000)"=refnum, "Delay"=refnum, "deadband"=refnum}, "Config Parameters"={"Tab Control 3"=refnum, "Tab Control 19"=refnum, "SAMPLES"=refnum, "Re-initilaize"=refnum, "Filter ON/OFF"=refnum, "TracHomeSurgeOffsetCounts 10MM"=refnum, "TracHomeSwayOffsetCounts 10MM"=refnum, "Acoustic Emission:"=refnum, "Apply Filter (FF)"=refnum, "Filter% 2"=refnum, "Apply Filter (Load)"=refnum, "Filter% "=refnum, "Sway distance (mm)"=refnum, "Surge distance (mm)"=refnum, "DataSavingLoopDelay(ms)"=refnum, "SAVE 2"=refnum, "Enter Distance"=refnum, "Sway Counts:"=refnum, "Distance (mm): 3"=refnum, "Surge Counts:"=refnum, "Distance (mm): 2"=refnum, "Distance (mm):"=refnum, "Heave Counts:"=refnum, "LRMHomeSurgeOffsetCounts"=refnum, "LRMHomeSwayOffsetCounts"=refnum, "TracHomeSurgeOffsetCounts 20MM"=refnum, "TracHomeSwayOffsetCounts 20MM"=refnum, "RotHomeSwayOffsetCounts"=refnum, "RotHomeSurgeOffsetCounts"=refnum, "Heave distance"=refnum, "Zmm"=refnum, "Heave Pulses/mm"=refnum, "Surge Pulses/mm"=refnum, "Sway Pulses/mm"=refnum, "Heave Pitch"=refnum, "Surge Pitch"=refnum, "Sway Pitch"=refnum, "Heave PPR"=refnum, "Surge PPR"=refnum, "Sway PPR"=refnum, "Tab Control 5"=refnum, "Tab Control 14"=refnum, "Tab Control 26"=refnum, "AE"=refnum, "Heave Loop Delay"=refnum, "Heave PID Speed"=refnum, "Surge Jog Speed"=refnum, "Heave Jog Speed"=refnum, "Sway Loop Delay"=refnum, "Sway PID Speed"=refnum, "Sway Jog Speed"=refnum, "DEPTH TRIP VALUE"=refnum, "LOAD TRIP VALUE"=refnum, "DEPTH TRIP   ENABLE"=refnum, "LOAD TRIP  ENABLE"=refnum, "CYCLIC FF TRIP VALUE"=refnum, "FF TRIP VALUE"=refnum, "CYCLIC CoF TRIP VALUE"=refnum, "COF TRIP VALUE"=refnum, "CYCLIC COF TRIP  ENABLE"=refnum, "CYCLIC FF TRIP  ENABLE"=refnum, "FF TRIP  ENABLE"=refnum, "COF TRIP  ENABLE"=refnum}, "Loading Com Port"={"ClearAll"=refnum, "Mz(Nm)"=refnum, "My(Nm)"=refnum, "Mx(Nm)"=refnum, "Save Dwell"=refnum, "Mx "=refnum, "My "=refnum, "Mz"=refnum, "Fx(N)"=refnum, "Fy(N)"=refnum, "Fz(N)"=refnum, "ZeroAll"=refnum, "Acq Delay (ms)"=refnum, "Burst Delay (ms)"=refnum, "model"=refnum, "SN"=refnum, "FFx(N)"=refnum, "Sensor IP"=refnum, "Port"=refnum, "FFy(N)"=refnum, "Load(N)"=refnum, "delete Handle"=refnum, "Create Handle"=refnum, "ft_data"=refnum, "ft_range"=refnum, "ft_data 2"=refnum, "stop 6"=refnum, "running_flag"=refnum, "ft_udp_handle"=refnum, "get-data-return"=refnum, "get-range-return"=refnum, "zero-return"=refnum, "filter-return"=refnum, "initial-return"=refnum, "deleteHandle-result"=refnum, "Load Cell Temp"=refnum}, "Heave AND Surge"={"SURGE POSE"=refnum, "error out Read"=refnum, "HEAVE POSE"=refnum, "State"=refnum, "Homed"=refnum, "Sequence ID"=refnum, "error out Write"=refnum, "faultCode"=refnum, "Ack ID"=refnum, "SPEED"=refnum, "Distance"=refnum, "Mode Command"=refnum, "Heave and Surge Read"=refnum, "Read Heave Temp"=refnum, "Spare 15"=refnum, "Spare 14"=refnum, "Spare 13"=refnum, "Spare 12"=refnum, "Spare 11"=refnum, "Spare 10"=refnum, "Spare 9"=refnum, "Spare 8"=refnum, "Spare 7"=refnum, "Spare 6"=refnum, "Spare 5"=refnum, "Spare 4"=refnum, "Spare 2"=refnum, "Spare 1"=refnum, "Node Id"=refnum, "Spare 3"=refnum, "SPARE 4"=refnum, "SPARE 3"=refnum, "SPARE 2"=refnum, "SPARE 1"=refnum, "fwMajor"=refnum, "fwMinor"=refnum, "Manual Write"=refnum, "Heave and Surge Write"=refnum}, "New PID LOGIC"={"Fine Tune Zone"=refnum, "PID SDelay"=refnum, "Max_pos_limit"=refnum, "Min_pos_limit"=refnum, "i_limit"=refnum, "pct_scale"=refnum, "Deadband"=refnum, "Kd"=refnum, "Ki"=refnum, "Kp"=refnum, "Current Position"=refnum, "Set Load"=refnum, "Current Load"=refnum, "Pulse delta"=refnum, "Init Step"=refnum, "Max Step Linit"=refnum}, "SWAY "={"fwMajor"=refnum, "Homed"=refnum, "Rotary POSE"=refnum, "State"=refnum, "SWAY POSE"=refnum, "Ack ID"=refnum, "faultCode"=refnum, "Node Id"=refnum, "fwMinor"=refnum, "Spare 6"=refnum, "Spare 5"=refnum, "Spare 4"=refnum, "Spare 3"=refnum, "Spare 2"=refnum, "Spare 1"=refnum, "Spare 7"=refnum, "SPARE  5"=refnum, "error out Write  SWAY "=refnum, "error out Read SWAY "=refnum, "Manual Write SWAY "=refnum, "SWAY WRITE"=refnum, "SPARE  4"=refnum, "SPARE  3"=refnum, "SPARE 2"=refnum, "SPARE 1"=refnum, "Spare 15"=refnum, "Spare 14"=refnum, "Spare 13"=refnum, "Spare 12"=refnum, "Spare 11"=refnum, "Spare 9"=refnum, "Spare 8"=refnum, "SPEED"=refnum, "Distance"=refnum, "Mode Command"=refnum, "Sequence ID"=refnum, "SWAY READ"=refnum, "Spare 10"=refnum, "Read SWAY Temp"=refnum}, "Analysis Screen"={"Analysis Home"=refnum, "Refresh 2"=refnum, "MEAN 4"=refnum, "SD 4"=refnum, "VARIANCE 4"=refnum, "MEAN  3"=refnum, "SD  3"=refnum, "VARIANCE  3"=refnum, "MEAN 2"=refnum, "SD  2"=refnum, "VARIANCE 2"=refnum, "MEAN"=refnum, "SD"=refnum, "VARIANCE"=refnum, "File 4 Discription"=refnum, "OPEN 4"=refnum, "File Name 4"=refnum, "OPEN 3"=refnum, "File 3 Discription"=refnum, "File Name 3"=refnum, "Y-AXIS"=refnum, "X-AXIS"=refnum, "XY Graph"=refnum, "File Name 2"=refnum, "File Name 1"=refnum, "OPEN 2"=refnum, "OPEN 1"=refnum, "File 1 Discription "=refnum, "File 2 Discription"=refnum, "Export"=refnum, "File Format"=refnum}} ("Data Cluster") -> [w66]
    tunnel: w54 -> [w96]
    tunnel: [w76] -> w53
    tunnel: w53 -> [w103]
    tunnel: [w97] -> w52
    tunnel: w52 -> [w112]
    tunnel: [w111] -> w51
    tunnel: w51 -> [w148]
    tunnel: [w147] -> w49
    tunnel: w49 -> [w219]
    tunnel: [w218] -> w48
    tunnel: w48 -> [w246]
    tunnel: [w245] -> w47
    tunnel: w47 -> [w262]
    tunnel: [w261] -> w46
    tunnel: w46 -> [w381]
    tunnel: [w380] -> w21
    tunnel: w21 -> [w411]
    tunnel: [w410] -> w20
    tunnel: w20 -> [w476]
    tunnel: [w475] -> w19
    tunnel: w19 -> [w513]
    tunnel: [w512] -> w18
    tunnel: w18 -> [w553]
    tunnel: [w552] -> w15
    tunnel: w15 -> [w571]
    tunnel: [w570] -> w14
    tunnel: w14 -> [w612]
    tunnel: [w611] -> w12
    tunnel: [w644] -> w26
    tunnel: w12 -> [w645]
    frame #0 {
      n2 = control-ref of="GUI"() -> (w75:refnum<vi>)
      n3 = control-ref of="MainPage"() -> (w69:refnum<vi>)
      n4 = control-ref of="Platform Settings"() -> (w74:refnum<vi>)
      n5 = control-ref of="Configure"() -> (w73:refnum<vi>)
      n6 = control-ref of="Home"() -> (w72:refnum<vi>)
      n7 = control-ref of="EXIT"() -> (w71:refnum<vi>)
      n8 = control-ref of="service 2"() -> (w70:refnum<vi>)
      n9 = control-ref of="Analysis"() -> (w68:refnum<vi>)
      n10 = Bundle By Name(cluster=w66, "Main Home Screen.GUI"=w75, "Main Home Screen.Platform Settings"=w74, "Main Home Screen.Configure"=w73, "Main Home Screen.Home"=w72, "Main Home Screen.EXIT"=w71, "Main Home Screen.service 2"=w70, "Main Home Screen.MainPage"=w69, "Main Home Screen.Analysis"=w68) -> (w67:T11)
    }
    frame #1 {
      n11 = control-ref of="Sway Right Main"() -> (w86:refnum<vi>)
      n12 = control-ref of="Sway Left Main"() -> (w85:refnum<vi>)
      n13 = control-ref of="Heave Down Main"() -> (w84:refnum<vi>)
      n14 = control-ref of="Heave Up main"() -> (w83:refnum<vi>)
      n15 = control-ref of="Update Sway Speed"() -> (w82:refnum<vi>)
      n16 = control-ref of="Update Heave Speed"() -> (w81:refnum<vi>)
      n17 = control-ref of="Surge Backward Main"() -> (w77:refnum<vi>)
      n18 = control-ref of="Update Surge Speed"() -> (w94:refnum<vi>)
      n19 = control-ref of="Disable Axis Jog Soft Limits m"() -> (w92:refnum<vi>)
      n20 = control-ref of="Sway and Surge COM Status"() -> (w90:refnum<vi>)
      n21 = control-ref of="Heave COM Status"() -> (w89:refnum<vi>)
      n22 = control-ref of="Enable Platform"() -> (w88:refnum<vi>)
      n23 = control-ref of="Surge Forward Main"() -> (w87:refnum<vi>)
      n24 = control-ref of="mm/s Heave"() -> (w80:refnum<vi>)
      n25 = control-ref of="mm/sec"() -> (w79:refnum<vi>)
      n26 = control-ref of="mm"() -> (w78:refnum<vi>)
      n27 = control-ref of="mm/s  Surge"() -> (w95:refnum<vi>)
      n28 = control-ref of="mm/s  Sway"() -> (w91:refnum<vi>)
      n29 = control-ref of="Drive Error"() -> (w93:refnum<vi>)
      n30 = Bundle By Name(cluster=w96, "Platform Settings.mm/s  Surge"=w95, "Platform Settings.Update Surge Speed"=w94, "Platform Settings.Drive Error"=w93, "Platform Settings.Disable Axis Jog Soft Limits"=w92, "Platform Settings.mm/s  Sway"=w91, "Platform Settings.Sway and Surge COM Status"=w90, "Platform Settings.Heave COM Status"=w89, "Platform Settings.Enable Platform"=w88, "Platform Settings.Surge Forward Main"=w87, "Platform Settings.Sway Right Main"=w86, "Platform Settings.Sway Left Main"=w85, "Platform Settings.Heave Down Main"=w84, "Platform Settings.Heave Up main"=w83, "Platform Settings.Update Sway Speed"=w82, "Platform Settings.Update Heave Speed"=w81, "Platform Settings.mm/s Heave"=w80, "Platform Settings.mm/sec"=w79, "Platform Settings.mm"=w78, "Platform Settings.Surge Backward Main"=w77) -> (w76:T11)
    }
    frame #2 {
      n31 = control-ref of="Analysis Home"() -> (w102:refnum<vi>)
      n32 = control-ref of="Surface Analysis"() -> (w101:refnum<vi>)
      n33 = control-ref of="Imaging"() -> (w100:refnum<vi>)
      n34 = control-ref of="Image Analysis"() -> (w99:refnum<vi>)
      n35 = control-ref of="Post Analysis"() -> (w98:refnum<vi>)
      n36 = Bundle By Name(cluster=w103, "Analysis Screen.Analysis Home"=w102, "Analysis Screen.Surface Analysis"=w101, "Analysis Screen.Imaging"=w100, "Analysis Screen.Image Analysis"=w99, "Analysis Screen.Post Analysis"=w98) -> (w97:T11)
    }
    frame #3 {
      n37 = control-ref of="Select Load Head"() -> (w110:refnum<vi>)
      n38 = control-ref of="Auto"() -> (w104:refnum<vi>)
      n39 = control-ref of="Notes :"() -> (w109:refnum<vi>)
      n40 = control-ref of="FILE"() -> (w108:refnum<vi>)
      n41 = control-ref of="Sample ID :"() -> (w107:refnum<vi>)
      n42 = control-ref of="Operator ID :"() -> (w106:refnum<vi>)
      n43 = control-ref of="Operator Name :"() -> (w105:refnum<vi>)
      n44 = Bundle By Name(cluster=w112, "Config Screen.Select Load Head"=w110, "Config Screen.Notes :"=w109, "Config Screen.FILE"=w108, "Config Screen.Sample ID :"=w107, "Config Screen.Operator ID :"=w106, "Config Screen.Operator Name :"=w105, "Config Screen.Auto"=w104) -> (w111:T11)
    }
    frame #4 {
      n45 = control-ref of="Warning"() -> (w140:refnum<vi>)
      n46 = control-ref of="gui GIF"() -> (w139:refnum<vi>)
      n47 = control-ref of="Load Selection"() -> (w113:refnum<vi>)
      n48 = control-ref of="Warning 2"() -> (w144:refnum<vi>)
      n49 = control-ref of="SSP 0.75"() -> (w143:refnum<vi>)
      n50 = control-ref of="SSP 0.5"() -> (w142:refnum<vi>)
      n51 = control-ref of="SSP 0.3"() -> (w141:refnum<vi>)
      n52 = control-ref of="Communication is established"() -> (w138:refnum<vi>)
      n53 = control-ref of="AppLoad 4"() -> (w137:refnum<vi>)
      n54 = control-ref of="Multipoint"() -> (w136:refnum<vi>)
      n55 = control-ref of="com 3"() -> (w132:refnum<vi>)
      n56 = control-ref of="com"() -> (w131:refnum<vi>)
      n57 = control-ref of="DecaForce COM Status"() -> (w130:refnum<vi>)
      n58 = control-ref of="Update"() -> (w129:refnum<vi>)
      n59 = control-ref of="Clear 3"() -> (w128:refnum<vi>)
      n60 = control-ref of="seq"() -> (w127:refnum<vi>)
      n61 = control-ref of="Stribeck table"() -> (w126:refnum<vi>)
      n62 = control-ref of="KiloForce"() -> (w118:refnum<vi>)
      n63 = control-ref of="DecaForce"() -> (w117:refnum<vi>)
      n64 = control-ref of="MicroForce"() -> (w116:refnum<vi>)
      n65 = control-ref of="LHBack"() -> (w115:refnum<vi>)
      n66 = control-ref of="LHNext"() -> (w114:refnum<vi>)
      n67 = control-ref of="Enter the Loading Rate (N/min)"() -> (w146:refnum<vi>)
      n68 = control-ref of="Enter the Final Load (N)"() -> (w123:refnum<vi>)
      n69 = control-ref of="Enter the CoF Trip"() -> (w122:refnum<vi>)
      n70 = control-ref of="Enter the Friction Force Trip"() -> (w121:refnum<vi>)
      n71 = control-ref of="Enter the Normal load Trip"() -> (w120:refnum<vi>)
      n72 = control-ref of="Enter the Load  (N)"() -> (w119:refnum<vi>)
      n73 = control-ref of="Message"() -> (w145:refnum<vi>)
      n74 = control-ref of="Indentation"() -> (w135:refnum<vi>)
      n75 = control-ref of="Stribeck Table  For loading"() -> (w125:refnum<vi>)
      n76 = control-ref of="Reference Sample"() -> (w134:refnum<vi>)
      n77 = control-ref of="Load Cell Communication Slide"() -> (w133:refnum<vi>)
      n78 = control-ref of="Loading Mode"() -> (w124:refnum<vi>)
      n79 = Bundle By Name(cluster=w148, "Loading.Enter the Loading Rate (N/min)"=w146, "Loading.Message"=w145, "Loading.Warning 2"=w144, "Loading.SSP 0.75"=w143, "Loading.SSP 0.5"=w142, "Loading.SSP 0.3"=w141, "Loading.Warning"=w140, "Loading.gui GIF"=w139, "Loading.Communication is established"=w138, "Loading.AppLoad 4"=w137, "Loading.Multipoint"=w136, "Loading.Indentation"=w135, "Loading.Reference Sample"=w134, "Loading.Load Cell Communication Slide"=w133, "Loading.com 3"=w132, "Loading.com"=w131, "Loading.DecaForce COM Status"=w130, "Loading.Update"=w129, "Loading.Clear 3"=w128, "Loading.seq"=w127, "Loading.Stribeck table"=w126, "Loading.Stribeck Table  For loading"=w125, "Loading.Loading Mode"=w124, "Loading.Enter the Final Load (N)"=w123, "Loading.Enter the CoF Trip"=w122, "Loading.Enter the Friction Force Trip"=w121, "Loading.Enter the Normal load Trip"=w120, "Loading.Enter the Load  (N)"=w119, "Loading.KiloForce"=w118, "Loading.DecaForce"=w117, "Loading.MicroForce"=w116, "Loading.LHBack"=w115, "Loading.LHNext"=w114, "Loading.Load Selection"=w113) -> (w147:T11)
    }
    frame #5 {
      n80 = control-ref of="TEST SELECTION"() -> (w200:refnum<vi>)
      n81 = control-ref of="SPEED SELECTION :"() -> (w199:refnum<vi>)
      n82 = control-ref of="SPEED SELECTION : rotary"() -> (w166:refnum<vi>)
      n83 = control-ref of="Rotary Tab"() -> (w215:refnum<vi>)
      n84 = control-ref of="e.v/ssr 2"() -> (w212:refnum<vi>)
      n85 = control-ref of="Step Speed"() -> (w196:refnum<vi>)
      n86 = control-ref of="M3 Image"() -> (w191:refnum<vi>)
      n87 = control-ref of="Rotary Module Selection"() -> (w168:refnum<vi>)
      n88 = control-ref of="zNL"() -> (w217:refnum<vi>)
      n89 = control-ref of="E.Velocity 2"() -> (w213:refnum<vi>)
      n90 = control-ref of="Ramp Up 2"() -> (w201:refnum<vi>)
      n91 = control-ref of="Angular Oscillation Set"() -> (w198:refnum<vi>)
      n92 = control-ref of="Traction"() -> (w197:refnum<vi>)
      n93 = control-ref of="Surge Forward MM"() -> (w193:refnum<vi>)
      n94 = control-ref of="Surge Backward MM"() -> (w192:refnum<vi>)
      n95 = control-ref of="Sway Left MM"() -> (w189:refnum<vi>)
      n96 = control-ref of="Sway Right MM"() -> (w188:refnum<vi>)
      n97 = control-ref of="Disable Axis Jog Soft Limits"() -> (w187:refnum<vi>)
      n98 = control-ref of="Heave Down MM"() -> (w185:refnum<vi>)
      n99 = control-ref of="Heave Up MM"() -> (w184:refnum<vi>)
      n100 = control-ref of="Set WTD"() -> (w182:refnum<vi>)
      n101 = control-ref of="HomeScratch"() -> (w181:refnum<vi>)
      n102 = control-ref of="HomeRot"() -> (w180:refnum<vi>)
      n103 = control-ref of="PlaceModule"() -> (w179:refnum<vi>)
      n104 = control-ref of="LR Sway"() -> (w175:refnum<vi>)
      n105 = control-ref of="Rot Hor"() -> (w174:refnum<vi>)
      n106 = control-ref of="Scratch"() -> (w173:refnum<vi>)
      n107 = control-ref of="LR Cam"() -> (w172:refnum<vi>)
      n108 = control-ref of="MMBack"() -> (w171:refnum<vi>)
      n109 = control-ref of="MMNext"() -> (w170:refnum<vi>)
      n110 = control-ref of="Rot Ver"() -> (w169:refnum<vi>)
      n111 = control-ref of="calculate rotary"() -> (w167:refnum<vi>)
      n112 = control-ref of="Import 2"() -> (w165:refnum<vi>)
      n113 = control-ref of="Save 2"() -> (w164:refnum<vi>)
      n114 = control-ref of="SwaySpeed Set"() -> (w157:refnum<vi>)
      n115 = control-ref of="HomeScratch"() -> (w153:refnum<vi>)
      n116 = control-ref of="NL disp"() -> (w216:refnum<vi>)
      n117 = control-ref of="Enter Fixed E.Velocity 2"() -> (w211:refnum<vi>)
      n118 = control-ref of="Enter Final SRR 2"() -> (w210:refnum<vi>)
      n119 = control-ref of="Enter initial SRR 2"() -> (w209:refnum<vi>)
      n120 = control-ref of="Enter Fixed SRR 2"() -> (w208:refnum<vi>)
      n121 = control-ref of="Enter the Final E.Velocity (m/s) 2"() -> (w207:refnum<vi>)
      n122 = control-ref of="Enter initial E.Velocity (m/s) 2"() -> (w206:refnum<vi>)
      n123 = control-ref of="Final Speed (RPM) 3"() -> (w205:refnum<vi>)
      n124 = control-ref of="Initial Speed (RPM) 2"() -> (w204:refnum<vi>)
      n125 = control-ref of="Enter the Final Velocity (m/s) 3"() -> (w203:refnum<vi>)
      n126 = control-ref of="Enter initial Velocity (m/s)  3"() -> (w202:refnum<vi>)
      n127 = control-ref of="mm"() -> (w186:refnum<vi>)
      n128 = control-ref of="Wear Track Diameter (mm)"() -> (w183:refnum<vi>)
      n129 = control-ref of="Enter the Angle (Deg)"() -> (w178:refnum<vi>)
      n130 = control-ref of="Enter the Frequency (Hz)"() -> (w177:refnum<vi>)
      n131 = control-ref of="Enter the Speed(mm/sec)"() -> (w160:refnum<vi>)
      n132 = control-ref of="Enter the Speed (RPM)"() -> (w159:refnum<vi>)
      n133 = control-ref of="Enter Scratch Speed (mm/s):"() -> (w158:refnum<vi>)
      n134 = control-ref of="Scartch Offset"() -> (w156:refnum<vi>)
      n135 = control-ref of="Enter Scratch length (mm):"() -> (w152:refnum<vi>)
      n136 = control-ref of="Wear Track Diameter"() -> (w151:refnum<vi>)
      n137 = control-ref of="No of Scratch"() -> (w149:refnum<vi>)
      n138 = control-ref of="String 39"() -> (w190:refnum<vi>)
      n139 = control-ref of="String 45"() -> (w162:refnum<vi>)
      n140 = control-ref of="Rotary Speed Exced"() -> (w150:refnum<vi>)
      n141 = control-ref of="StepTable For Load-Speed"() -> (w195:refnum<vi>)
      n142 = control-ref of="StepTable For Speed"() -> (w194:refnum<vi>)
      n143 = control-ref of="StepTable For Speed 3"() -> (w161:refnum<vi>)
      n144 = control-ref of="Motion Direction:  3"() -> (w214:refnum<vi>)
      n145 = control-ref of="Motion Mode:"() -> (w176:refnum<vi>)
      n146 = control-ref of="Scratch Mode"() -> (w155:refnum<vi>)
      n147 = control-ref of="Motion type:"() -> (w154:refnum<vi>)
      n148 = control-ref of="File Path :  2"() -> (w163:refnum<vi>)
      n149 = Bundle By Name(cluster=w219, "Motion Module.zNL"=w217, "Motion Module.NL disp"=w216, "Motion Module.Rotary Tab"=w215, "Motion Module.Motion Direction:  3"=w214, "Motion Module.E.Velocity 2"=w213, "Motion Module.e.v/ssr 2"=w212, "Motion Module.Enter Fixed E.Velocity 2"=w211, "Motion Module.Enter Final SRR 2"=w210, "Motion Module.Enter initial SRR 2"=w209, "Motion Module.Enter Fixed SRR 2"=w208, "Motion Module.Enter the Final E.Velocity (m/s) 2"=w207, "Motion Module.Enter initial E.Velocity (m/s) 2"=w206, "Motion Module.Final Speed (RPM) 3"=w205, "Motion Module.Initial Speed (RPM) 2"=w204, "Motion Module.Enter the Final Velocity (m/s) 3"=w203, "Motion Module.Enter initial Velocity (m/s)  3"=w202, "Motion Module.Ramp Up 2"=w201, "Motion Module.TEST SELECTION"=w200, "Motion Module.SPEED SELECTION :"=w199, "Motion Module.Angular Oscillation Set"=w198, "Motion Module.Traction"=w197, "Motion Module.Step Speed"=w196, "Motion Module.StepTable For Load-Speed"=w195, "Motion Module.StepTable For Speed"=w194, "Motion Module.Surge Forward MM"=w193, "Motion Module.Surge Backward MM"=w192, "Motion Module.M3 Image"=w191, "Motion Module.String 39"=w190, "Motion Module.Sway Left MM"=w189, "Motion Module.Sway Right MM"=w188, "Motion Module.Disable Axis Jog Soft Limits"=w187, "Motion Module.mm"=w186, "Motion Module.Heave Down MM"=w185, "Motion Module.Heave Up MM"=w184, "Motion Module.Wear Track Diameter (mm)"=w183, "Motion Module.Set WTD"=w182, "Motion Module.HomeScratch"=w181, "Motion Module.HomeRot"=w180, "Motion Module.PlaceModule"=w179, "Motion Module.Enter the Angle (Deg)"=w178, "Motion Module.Enter the Frequency (Hz)"=w177, "Motion Module.Motion Mode:"=w176, "Motion Module.LR Sway"=w175, "Motion Module.Rot Hor"=w174, "Motion Module.Scratch"=w173, "Motion Module.LR Cam"=w172, "Motion Module.MMBack"=w171, "Motion Module.MMNext"=w170, "Motion Module.Rot Ver"=w169, "Motion Module.Rotary Module Selection"=w168, "Motion Module.calculate rotary"=w167, "Motion Module.SPEED SELECTION : rotary"=w166, "Motion Module.Import 2"=w165, "Motion Module.Save 2"=w164, "Motion Module.File Path :  2"=w163, "Motion Module.String 45"=w162, "Motion Module.StepTable For Speed 3"=w161, "Motion Module.Enter the Speed(mm/sec)"=w160, "Motion Module.Enter the Speed(RPM)"=w159, "Motion Module.Enter Scratch Speed (mm/s):"=w158, "Motion Module.SwaySpeed Set"=w157, "Motion Module.Scartch Offset"=w156, "Motion Module.Scratch Mode"=w155, "Motion Module.Motion type:"=w154, "Motion Module.HomeScratch 2"=w153, "Motion Module.Enter Scratch length (mm):"=w152, "Motion Module.Wear Track Diameter"=w151, "Motion Module.Rotary Speed Exced"=w150, "Motion Module.No of Scratch"=w149) -> (w218:T11)
    }
    frame #6 {
      n150 = control-ref of="Add to list"() -> (w237:refnum<vi>)
      n151 = control-ref of="Wear"() -> (w236:refnum<vi>)
      n152 = control-ref of="Vibration"() -> (w235:refnum<vi>)
      n153 = control-ref of="Humidity (Chamber)"() -> (w234:refnum<vi>)
      n154 = control-ref of="Temperature (Chamber)"() -> (w233:refnum<vi>)
      n155 = control-ref of="ECR"() -> (w232:refnum<vi>)
      n156 = control-ref of="Temperature (Amb)"() -> (w231:refnum<vi>)
      n157 = control-ref of="Microphone"() -> (w230:refnum<vi>)
      n158 = control-ref of="Acoustic Emission 3"() -> (w229:refnum<vi>)
      n159 = control-ref of="SNext"() -> (w228:refnum<vi>)
      n160 = control-ref of="APBack"() -> (w227:refnum<vi>)
      n161 = control-ref of="Low Temp"() -> (w223:refnum<vi>)
      n162 = control-ref of="High Temp"() -> (w222:refnum<vi>)
      n163 = control-ref of="Humidity"() -> (w221:refnum<vi>)
      n164 = control-ref of="Humidity  Status  3"() -> (w244:refnum<vi>)
      n165 = control-ref of="Low Temp  Status  2"() -> (w243:refnum<vi>)
      n166 = control-ref of="TK4 status 2"() -> (w242:refnum<vi>)
      n167 = control-ref of="Humidity (Amb)"() -> (w239:refnum<vi>)
      n168 = control-ref of="Clear List"() -> (w238:refnum<vi>)
      n169 = control-ref of="Enter the Temperature (°C):"() -> (w226:refnum<vi>)
      n170 = control-ref of="Enter the Stage \nTemperature (°C):"() -> (w225:refnum<vi>)
      n171 = control-ref of="Enter the Humidity (%Rh):"() -> (w224:refnum<vi>)
      n172 = control-ref of="Sensors Picked"() -> (w220:refnum<vi>)
      n173 = control-ref of="Stage Temperature"() -> (w241:refnum<vi>)
      n174 = control-ref of="Sample Temperature"() -> (w240:refnum<vi>)
      n175 = Bundle By Name(cluster=w246, "Environmental control.Humidity  Status  3"=w244, "Environmental control.Low Temp  Status  2"=w243, "Environmental control.TK4 status 2"=w242, "Environmental control.Stage Temperature"=w241, "Environmental control.Sample Temperature"=w240, "Environmental control.Humidity (Amb)"=w239, "Environmental control.Clear List"=w238, "Environmental control.Add to list"=w237, "Environmental control.Wear"=w236, "Environmental control.Vibration"=w235, "Environmental control.Humidity (Chamber)"=w234, "Environmental control.Temperature (Chamber)"=w233, "Environmental control.ECR"=w232, "Environmental control.Temperature (Amb)"=w231, "Environmental control.Microphone"=w230, "Environmental control.Acoustic Emission 3"=w229, "Environmental control.SNext"=w228, "Environmental control.APBack"=w227, "Environmental control.Enter the Temperature (°C):"=w226, "Environmental control.Enter the Stage \nTemperature (°C):"=w225, "Environmental control.Enter the Humidity (%Rh):"=w224, "Environmental control.Low Temp"=w223, "Environmental control.High Temp"=w222, "Environmental control.Humidity"=w221, "Environmental control.Sensors Picked"=w220) -> (w245:T11)
    }
    frame #7 {
      n176 = control-ref of="ECR Port:"() -> (w256:refnum<vi>)
      n177 = control-ref of="Ramp Port:"() -> (w255:refnum<vi>)
      n178 = control-ref of="Heave and Surge COM Port:"() -> (w252:refnum<vi>)
      n179 = control-ref of="Sway COM Port:"() -> (w251:refnum<vi>)
      n180 = control-ref of="Temp Modbus:"() -> (w250:refnum<vi>)
      n181 = control-ref of="Humidity Port:"() -> (w249:refnum<vi>)
      n182 = control-ref of="About Tab"() -> (w257:refnum<vi>)
      n183 = control-ref of="Home Service"() -> (w259:refnum<vi>)
      n184 = control-ref of="Advanced Setting"() -> (w258:refnum<vi>)
      n185 = control-ref of="Installation/Replacement completed"() -> (w254:refnum<vi>)
      n186 = control-ref of="Loahead"() -> (w253:refnum<vi>)
      n187 = control-ref of="Edit Gain Constants"() -> (w248:refnum<vi>)
      n188 = control-ref of="Save Gain Constants"() -> (w247:refnum<vi>)
      n189 = control-ref of="Password"() -> (w260:refnum<vi>)
      n190 = Bundle By Name(cluster=w262, "About Screen.Password"=w260, "About Screen.Home Service"=w259, "About Screen.Advanced Setting"=w258, "About Screen.About Tab"=w257, "About Screen.ECR Port:"=w256, "About Screen.Ramp Port:"=w255, "About Screen.Installation/Replacement completed"=w254, "About Screen.Loahead"=w253, "About Screen.Heave and Surge COM Port:"=w252, "About Screen.Sway COM Port:"=w251, "About Screen.Temp Modbus:"=w250, "About Screen.Humidity Port:"=w249, "About Screen.Edit Gain Constants"=w248, "About Screen.Save Gain Constants"=w247) -> (w261:T11)
    }
    frame #8 {
      n191 = control-ref of="Cyclic Friction Force (N) Graph"() -> (w273:refnum<vi>)
      n192 = control-ref of="Cyclic Coefficient of Friction"() -> (w272:refnum<vi>)
      n193 = control-ref of="SDGp"() -> (w321:refnum<vi>)
      n194 = control-ref of="HumrGp"() -> (w319:refnum<vi>)
      n195 = control-ref of="gACQUOS"() -> (w316:refnum<vi>)
      n196 = control-ref of="ECR 2"() -> (w314:refnum<vi>)
      n197 = control-ref of="Temperature (deg c)"() -> (w312:refnum<vi>)
      n198 = control-ref of="MTM DISC  SPEED"() -> (w309:refnum<vi>)
      n199 = control-ref of="MTM BALL SPEED"() -> (w308:refnum<vi>)
      n200 = control-ref of="speed mm/sec"() -> (w307:refnum<vi>)
      n201 = control-ref of="WearGp"() -> (w297:refnum<vi>)
      n202 = control-ref of="Main Chart 3"() -> (w291:refnum<vi>)
      n203 = control-ref of="Friction Force (N) Graph"() -> (w279:refnum<vi>)
      n204 = control-ref of="Coefficient of Friction"() -> (w278:refnum<vi>)
      n205 = control-ref of="Main Screen Tab"() -> (w379:refnum<vi>)
      n206 = control-ref of="Angle and Frequency"() -> (w378:refnum<vi>)
      n207 = control-ref of="Main Speed Tab"() -> (w375:refnum<vi>)
      n208 = control-ref of="MTM MOTOR DISPLAY"() -> (w374:refnum<vi>)
      n209 = control-ref of="SPEED TAB"() -> (w369:refnum<vi>)
      n210 = control-ref of="Time Tab"() -> (w364:refnum<vi>)
      n211 = control-ref of="Temp Tabs"() -> (w357:refnum<vi>)
      n212 = control-ref of="Sub Graph"() -> (w324:refnum<vi>)
      n213 = control-ref of="Speed Tab"() -> (w310:refnum<vi>)
      n214 = control-ref of="FF Tab"() -> (w276:refnum<vi>)
      n215 = control-ref of="CZ FF"() -> (w274:refnum<vi>)
      n216 = control-ref of="Cyclic FF Disable Trip"() -> (w270:refnum<vi>)
      n217 = control-ref of="cyclic COF Disable Trip"() -> (w269:refnum<vi>)
      n218 = control-ref of="cyclic COF Reset Graph"() -> (w267:refnum<vi>)
      n219 = control-ref of="Cyclic FF Reset Graph"() -> (w266:refnum<vi>)
      n220 = control-ref of="Test Trip"() -> (w265:refnum<vi>)
      n221 = control-ref of="Scratch Start Test"() -> (w277:refnum<vi>)
      n222 = control-ref of="Scratch Start Recording"() -> (w263:refnum<vi>)
      n223 = control-ref of="Heater"() -> (w356:refnum<vi>)
      n224 = control-ref of="TK4 status"() -> (w355:refnum<vi>)
      n225 = control-ref of="Controller  Status"() -> (w352:refnum<vi>)
      n226 = control-ref of="Cooling"() -> (w349:refnum<vi>)
      n227 = control-ref of="Load Communication"() -> (w348:refnum<vi>)
      n228 = control-ref of="HumCOMStatus"() -> (w346:refnum<vi>)
      n229 = control-ref of="Load En"() -> (w343:refnum<vi>)
      n230 = control-ref of="NLt"() -> (w342:refnum<vi>)
      n231 = control-ref of="zNL 2"() -> (w341:refnum<vi>)
      n232 = control-ref of="Humidity On"() -> (w340:refnum<vi>)
      n233 = control-ref of="AppLoadSeq scratch"() -> (w336:refnum<vi>)
      n234 = control-ref of="Stop Scratch"() -> (w335:refnum<vi>)
      n235 = control-ref of="ClrLog"() -> (w334:refnum<vi>)
      n236 = control-ref of="STOP"() -> (w332:refnum<vi>)
      n237 = control-ref of="Start Test"() -> (w331:refnum<vi>)
      n238 = control-ref of="Test status"() -> (w330:refnum<vi>)
      n239 = control-ref of="AR Led"() -> (w329:refnum<vi>)
      n240 = control-ref of="Data"() -> (w328:refnum<vi>)
      n241 = control-ref of="Health"() -> (w327:refnum<vi>)
      n242 = control-ref of="Sway COM Status"() -> (w326:refnum<vi>)
      n243 = control-ref of="Heave COM Status"() -> (w325:refnum<vi>)
      n244 = control-ref of="Siliding distance Reset Graph"() -> (w322:refnum<vi>)
      n245 = control-ref of="Humidity Reset Graph"() -> (w320:refnum<vi>)
      n246 = control-ref of="Aqucostic Reset Graph"() -> (w317:refnum<vi>)
      n247 = control-ref of="ECR RESET"() -> (w315:refnum<vi>)
      n248 = control-ref of="Temperature Reset"() -> (w313:refnum<vi>)
      n249 = control-ref of="Speed Reset Graph"() -> (w311:refnum<vi>)
      n250 = control-ref of="Hymidity"() -> (w306:refnum<vi>)
      n251 = control-ref of="Humidity Disable trip"() -> (w305:refnum<vi>)
      n252 = control-ref of="Weart Deapth"() -> (w302:refnum<vi>)
      n253 = control-ref of="Depth Reset Graph"() -> (w301:refnum<vi>)
      n254 = control-ref of="Weart"() -> (w300:refnum<vi>)
      n255 = control-ref of="Depthz"() -> (w299:refnum<vi>)
      n256 = control-ref of="Load pid"() -> (w295:refnum<vi>)
      n257 = control-ref of="Load Disable Trip"() -> (w294:refnum<vi>)
      n258 = control-ref of="Load Reset Graph"() -> (w293:refnum<vi>)
      n259 = control-ref of="BACK"() -> (w290:refnum<vi>)
      n260 = control-ref of="zFF"() -> (w280:refnum<vi>)
      n261 = control-ref of="FF Reset Graph"() -> (w286:refnum<vi>)
      n262 = control-ref of="FF Disable Trip"() -> (w285:refnum<vi>)
      n263 = control-ref of="COF Disable Trip"() -> (w283:refnum<vi>)
      n264 = control-ref of="COF Reset Graph"() -> (w282:refnum<vi>)
      n265 = control-ref of="Start Test Temp"() -> (w281:refnum<vi>)
      n266 = control-ref of="Depth Trip 2"() -> (w289:refnum<vi>)
      n267 = control-ref of="Multi Scratch Pass"() -> (w264:refnum<vi>)
      n268 = control-ref of="Cyclic Friction Force (N)"() -> (w275:refnum<vi>)
      n269 = control-ref of="Cyclic FF TRIP"() -> (w271:refnum<vi>)
      n270 = control-ref of="cyclic COF TRIP"() -> (w268:refnum<vi>)
      n271 = control-ref of="Stroke (mm)"() -> (w377:refnum<vi>)
      n272 = control-ref of="Angle (Deg)"() -> (w376:refnum<vi>)
      n273 = control-ref of="Disc Speed (m/sec)"() -> (w373:refnum<vi>)
      n274 = control-ref of="Ball Speed (m/sec)"() -> (w372:refnum<vi>)
      n275 = control-ref of="Disc Speed (RPM)"() -> (w371:refnum<vi>)
      n276 = control-ref of="Ball Speed (RPM)"() -> (w370:refnum<vi>)
      n277 = control-ref of="Speed (m/sec)"() -> (w368:refnum<vi>)
      n278 = control-ref of="Set Speed (m/sec)"() -> (w367:refnum<vi>)
      n279 = control-ref of="Speed (RPM)"() -> (w366:refnum<vi>)
      n280 = control-ref of="Set Speed"() -> (w365:refnum<vi>)
      n281 = control-ref of="Time ( HH:MM:SS ) 2"() -> (w363:refnum<vi>)
      n282 = control-ref of="Test Duration"() -> (w362:refnum<vi>)
      n283 = control-ref of="Test Duration 4"() -> (w361:refnum<vi>)
      n284 = control-ref of="TEST CYCLE"() -> (w360:refnum<vi>)
      n285 = control-ref of="TOTAL CYCLES"() -> (w359:refnum<vi>)
      n286 = control-ref of="Set Load (N)"() -> (w358:refnum<vi>)
      n287 = control-ref of="ChamberTemp"() -> (w354:refnum<vi>)
      n288 = control-ref of="SetTmp"() -> (w353:refnum<vi>)
      n289 = control-ref of="ChamberTemp"() -> (w351:refnum<vi>)
      n290 = control-ref of="SetTmp"() -> (w350:refnum<vi>)
      n291 = control-ref of="Ambient \nTemperature"() -> (w347:refnum<vi>)
      n292 = control-ref of="Ambient\n Humidity"() -> (w345:refnum<vi>)
      n293 = control-ref of="Freq (Hz)"() -> (w344:refnum<vi>)
      n294 = control-ref of="humidity disp"() -> (w339:refnum<vi>)
      n295 = control-ref of="Set Humidity"() -> (w338:refnum<vi>)
      n296 = control-ref of="NL disp 2"() -> (w337:refnum<vi>)
      n297 = control-ref of="SD (mm)"() -> (w323:refnum<vi>)
      n298 = control-ref of="Acoustic Emission (mV)"() -> (w318:refnum<vi>)
      n299 = control-ref of="CoF Trip  2"() -> (w304:refnum<vi>)
      n300 = control-ref of="Depth Trip"() -> (w303:refnum<vi>)
      n301 = control-ref of="Depth (µm)"() -> (w298:refnum<vi>)
      n302 = control-ref of="NL Trip 2"() -> (w296:refnum<vi>)
      n303 = control-ref of="NL Display 4"() -> (w292:refnum<vi>)
      n304 = control-ref of="COF TRIP"() -> (w288:refnum<vi>)
      n305 = control-ref of="Friction Force (N)"() -> (w287:refnum<vi>)
      n306 = control-ref of="FF TRIP"() -> (w284:refnum<vi>)
      n307 = control-ref of="Trip Log"() -> (w333:refnum<vi>)
      n308 = Bundle By Name(cluster=w381, "Main Screen.Test Trip"=w265, "Main Screen.Main Screen Tab"=w379, "Main Screen.Angle and Frequency"=w378, "Main Screen.Stroke (mm)"=w377, "Main Screen.Angle (Deg)"=w376, "Main Screen.Main Speed Tab"=w375, "Main Screen.MTM MOTOR DISPLAY"=w374, "Main Screen.Disc Speed (m/sec)"=w373, "Main Screen.Ball Speed (m/sec)"=w372, "Main Screen.Disc Speed (RPM)"=w371, "Main Screen.Ball Speed (RPM)"=w370, "Main Screen.SPEED TAB"=w369, "Main Screen.Speed (m/sec)"=w368, "Main Screen.Set Speed (m/sec)"=w367, "Main Screen.Speed (RPM)"=w366, "Main Screen.Set Speed"=w365, "Main Screen.Time Tab"=w364, "Main Screen.Time ( HH:MM:SS ) 2"=w363, "Main Screen.Test Duration"=w362, "Main Screen.Test Duration 4"=w361, "Main Screen.TEST CYCLE"=w360, "Main Screen.TOTAL CYCLES"=w359, "Main Screen.Set Load (N)"=w358, "Main Screen.Temp Tabs"=w357, "Main Screen.Heater"=w356, "Main Screen.TK4 status"=w355, "Main Screen.ChamberTemp"=w354, "Main Screen.SetTmp"=w353, "Main Screen.Controller  Status"=w352, "Main Screen.ChamberTemp 2"=w351, "Main Screen.SetTmp 2"=w350, "Main Screen.Cooling"=w349, "Main Screen.Load Communication"=w348, "Main Screen.Ambient \nTemperature"=w347, "Main Screen.HumCOMStatus"=w346, "Main Screen.Ambient\n Humidity"=w345, "Main Screen.Freq (Hz)"=w344, "Main Screen.Load En"=w343, "Main Screen.NLt"=w342, "Main Screen.zNL 2"=w341, "Main Screen.Humidity On"=w340, "Main Screen.humidity disp"=w339, "Main Screen.Set Humidity"=w338, "Main Screen.NL disp 2"=w337, "Main Screen.AppLoadSeq scratch"=w336, "Main Screen.Stop Scratch"=w335, "Main Screen.ClrLog"=w334, "Main Screen.Trip Log"=w333, "Main Screen.STOP"=w332, "Main Screen.Start Test"=w331, "Main Screen.Test status"=w330, "Main Screen.AR Led"=w329, "Main Screen.Data"=w328, "Main Screen.Health"=w327, "Main Screen.Sway COM Status"=w326, "Main Screen.Heave COM Status"=w325, "Main Screen.Sub Graph"=w324, "Main Screen.SD (mm)"=w323, "Main Screen.Siliding distance Reset Graph"=w322, "Main Screen.SDGp"=w321, "Main Screen.Humidity Reset Graph"=w320, "Main Screen.HumrGp"=w319, "Main Screen.Acoustic Emission (mV)"=w318, "Main Screen.Aqucostic Reset Graph"=w317, "Main Screen.gACQUOS"=w316, "Main Screen.ECR RESET"=w315, "Main Screen.ECR"=w314, "Main Screen.Temperature Reset"=w313, "Main Screen.Temperature (deg c)"=w312, "Main Screen.Speed Reset Graph"=w311, "Main Screen.Speed Tab"=w310, "Main Screen.MTM DISC  SPEED"=w309, "Main Screen.MTM BALL SPEED"=w308, "Main Screen.speed mm/sec"=w307, "Main Screen.Hymidity"=w306, "Main Screen.Humidity Disable trip"=w305, "Main Screen.CoF Trip  2"=w304, "Main Screen.Depth Trip"=w303, "Main Screen.Weart Deapth"=w302, "Main Screen.Depth Reset Graph"=w301, "Main Screen.Weart"=w300, "Main Screen.Depthz"=w299, "Main Screen.Depth (µm)"=w298, "Main Screen.WearGp"=w297, "Main Screen.NL Trip 2"=w296, "Main Screen.Load pid"=w295, "Main Screen.Load Disable Trip"=w294, "Main Screen.Load Reset Graph"=w293, "Main Screen.NL Display 4"=w292, "Main Screen.Main Chart 3"=w291, "Main Screen.BACK"=w290, "Main Screen.Depth Trip 2"=w289, "Main Screen.COF TRIP"=w288, "Main Screen.Friction Force (N)"=w287, "Main Screen.FF Reset Graph"=w286, "Main Screen.FF Disable Trip"=w285, "Main Screen.FF TRIP"=w284, "Main Screen.COF Disable Trip"=w283, "Main Screen.COF Reset Graph"=w282, "Main Screen.FF Tab"=w276, "Main Screen.Start Test Temp"=w281, "Main Screen.zFF"=w280, "Main Screen.Friction Force (N) Graph"=w279, "Main Screen.Coefficient of Friction"=w278, "Main Screen.Scratch Start Test"=w277, "Main Screen.Cyclic Friction Force (N)"=w275, "Main Screen.CZ FF"=w274, "Main Screen.Cyclic Friction Force (N) Graph"=w273, "Main Screen.Cyclic Coefficient of Friction"=w272, "Main Screen.Cyclic FF TRIP"=w271, "Main Screen.Cyclic FF Disable Trip"=w270, "Main Screen.cyclic COF Disable Trip"=w269, "Main Screen.cyclic COF TRIP"=w268, "Main Screen.cyclic COF Reset Graph"=w267, "Main Screen.Cyclic FF Reset Graph"=w266, "Main Screen.Multi Scratch Pass"=w264, "Main Screen.Scratch Start Recording"=w263) -> (w380:T11)
    }
    frame #9 {
      n309 = control-ref of="gFF Rot 7"() -> (w385:refnum<vi>)
      n310 = control-ref of="Ramp"() -> (w404:refnum<vi>)
      n311 = control-ref of="Dummy Run"() -> (w398:refnum<vi>)
      n312 = control-ref of="AutoTune"() -> (w396:refnum<vi>)
      n313 = control-ref of="apply load"() -> (w394:refnum<vi>)
      n314 = control-ref of="reinit 3"() -> (w392:refnum<vi>)
      n315 = control-ref of="Bypass Load"() -> (w389:refnum<vi>)
      n316 = control-ref of="PID gains out delay (microForce)"() -> (w405:refnum<vi>)
      n317 = control-ref of="output range delay"() -> (w391:refnum<vi>)
      n318 = control-ref of="PID gains out delay"() -> (w390:refnum<vi>)
      n319 = control-ref of="Ramp MulFac"() -> (w409:refnum<vi>)
      n320 = control-ref of="pulses LoadDiffRamp(2..10)"() -> (w408:refnum<vi>)
      n321 = control-ref of="PulseControlRamp(diff<=3N)"() -> (w407:refnum<vi>)
      n322 = control-ref of="SetLoadDeadband(%) Load(0-10N)"() -> (w406:refnum<vi>)
      n323 = control-ref of="Gain 2"() -> (w403:refnum<vi>)
      n324 = control-ref of="pulses LoadDiff(2..10)"() -> (w402:refnum<vi>)
      n325 = control-ref of="pulses LoadDiff(11..50)"() -> (w401:refnum<vi>)
      n326 = control-ref of="PulseControl(diff<=3N)"() -> (w400:refnum<vi>)
      n327 = control-ref of="SetLoadDeadband(%)  2"() -> (w399:refnum<vi>)
      n328 = control-ref of="Vertical load (N)"() -> (w397:refnum<vi>)
      n329 = control-ref of="Offset  3"() -> (w395:refnum<vi>)
      n330 = control-ref of="Enter ByPass Load"() -> (w393:refnum<vi>)
      n331 = control-ref of="pulsesSent"() -> (w388:refnum<vi>)
      n332 = control-ref of="pulses"() -> (w387:refnum<vi>)
      n333 = control-ref of="actpid"() -> (w386:refnum<vi>)
      n334 = control-ref of="pulses LoadDiff(21..1000)"() -> (w384:refnum<vi>)
      n335 = control-ref of="Delay"() -> (w383:refnum<vi>)
      n336 = control-ref of="deadband"() -> (w382:refnum<vi>)
      n337 = Bundle By Name(cluster=w411, "PID.Ramp MulFac"=w409, "PID.pulses LoadDiffRamp(2..10)"=w408, "PID.PulseControlRamp(diff<=3N)"=w407, "PID.SetLoadDeadband(%) Load(0-10N)"=w406, "PID.PID gains out delay (microForce)"=w405, "PID.Ramp"=w404, "PID.Gain 2"=w403, "PID.pulses LoadDiff(2..10)"=w402, "PID.pulses LoadDiff(11..50)"=w401, "PID.PulseControl(diff<=3N)"=w400, "PID.SetLoadDeadband(%)  2"=w399, "PID.Dummy Run"=w398, "PID.Vertical load (N)"=w397, "PID.AutoTune"=w396, "PID.Offset 3"=w395, "PID.apply load"=w394, "PID.Enter ByPass Load"=w393, "PID.reinit 3"=w392, "PID.output range delay"=w391, "PID.PID gains out delay"=w390, "PID.Bypass Load"=w389, "PID.pulsesSent"=w388, "PID.pulses"=w387, "PID.actpid"=w386, "PID.gFF Rot"=w385, "PID.pulses LoadDiff(21..1000)"=w384, "PID.Delay"=w383, "PID.deadband"=w382) -> (w410:T11)
    }
    frame #10 {
      n338 = control-ref of="Tab Control 3"() -> (w474:refnum<vi>)
      n339 = control-ref of="Tab Control 19"() -> (w473:refnum<vi>)
      n340 = control-ref of="Tab Control 5"() -> (w434:refnum<vi>)
      n341 = control-ref of="Tab Control 14"() -> (w433:refnum<vi>)
      n342 = control-ref of="Tab Control 26"() -> (w432:refnum<vi>)
      n343 = control-ref of="DEPTH TRIP   ENABLE"() -> (w421:refnum<vi>)
      n344 = control-ref of="LOAD TRIP  ENABLE"() -> (w420:refnum<vi>)
      n345 = control-ref of="CYCLIC COF TRIP  ENABLE"() -> (w415:refnum<vi>)
      n346 = control-ref of="CYCLIC FF TRIP  ENABLE"() -> (w414:refnum<vi>)
      n347 = control-ref of="FF TRIP  ENABLE"() -> (w413:refnum<vi>)
      n348 = control-ref of="COF TRIP  ENABLE"() -> (w412:refnum<vi>)
      n349 = control-ref of="Re-initilaize"() -> (w471:refnum<vi>)
      n350 = control-ref of="Filter ON/OFF"() -> (w470:refnum<vi>)
      n351 = control-ref of="Apply Filter (FF)"() -> (w466:refnum<vi>)
      n352 = control-ref of="Apply Filter (Load)"() -> (w464:refnum<vi>)
      n353 = control-ref of="SAVE  2"() -> (w459:refnum<vi>)
      n354 = control-ref of="Enter Distance"() -> (w458:refnum<vi>)
      n355 = control-ref of="AE"() -> (w431:refnum<vi>)
      n356 = control-ref of="Heave Loop Delay"() -> (w430:refnum<vi>)
      n357 = control-ref of="Heave PID Speed"() -> (w429:refnum<vi>)
      n358 = control-ref of="Surge Jog Speed"() -> (w428:refnum<vi>)
      n359 = control-ref of="Heave Jog Speed"() -> (w427:refnum<vi>)
      n360 = control-ref of="Sway Loop Delay"() -> (w426:refnum<vi>)
      n361 = control-ref of="Sway PID Speed"() -> (w425:refnum<vi>)
      n362 = control-ref of="Sway Jog Speed"() -> (w424:refnum<vi>)
      n363 = control-ref of="DEPTH TRIP VALUE"() -> (w423:refnum<vi>)
      n364 = control-ref of="LOAD TRIP VALUE"() -> (w422:refnum<vi>)
      n365 = control-ref of="CYCLIC FF TRIP VALUE"() -> (w419:refnum<vi>)
      n366 = control-ref of="FF TRIP VALUE"() -> (w418:refnum<vi>)
      n367 = control-ref of="CYCLIC CoF TRIP VALUE"() -> (w417:refnum<vi>)
      n368 = control-ref of="COF TRIP VALUE"() -> (w416:refnum<vi>)
      n369 = control-ref of="SAMPLES"() -> (w472:refnum<vi>)
      n370 = control-ref of="TracHomeSurgeOffsetCounts 10MM"() -> (w469:refnum<vi>)
      n371 = control-ref of="TracHomeSwayOffsetCounts 10MM"() -> (w468:refnum<vi>)
      n372 = control-ref of="Acoustic Emission:"() -> (w467:refnum<vi>)
      n373 = control-ref of="Filter% 2"() -> (w465:refnum<vi>)
      n374 = control-ref of="Filter%"() -> (w463:refnum<vi>)
      n375 = control-ref of="Sway distance (mm)"() -> (w462:refnum<vi>)
      n376 = control-ref of="Surge distance (mm)"() -> (w461:refnum<vi>)
      n377 = control-ref of="DataSavingLoopDelay(ms)"() -> (w460:refnum<vi>)
      n378 = control-ref of="Sway Counts:"() -> (w457:refnum<vi>)
      n379 = control-ref of="Distance (mm): 3"() -> (w456:refnum<vi>)
      n380 = control-ref of="Surge Counts:"() -> (w455:refnum<vi>)
      n381 = control-ref of="Distance (mm): 2"() -> (w454:refnum<vi>)
      n382 = control-ref of="Distance (mm):"() -> (w453:refnum<vi>)
      n383 = control-ref of="Heave Counts:"() -> (w452:refnum<vi>)
      n384 = control-ref of="LRMHomeSurgeOffsetCounts"() -> (w451:refnum<vi>)
      n385 = control-ref of="LRMHomeSwayOffsetCounts"() -> (w450:refnum<vi>)
      n386 = control-ref of="TracHomeSurgeOffsetCounts 20MM"() -> (w449:refnum<vi>)
      n387 = control-ref of="TracHomeSwayOffsetCounts 20MM"() -> (w448:refnum<vi>)
      n388 = control-ref of="RotHomeSwayOffsetCounts"() -> (w447:refnum<vi>)
      n389 = control-ref of="RotHomeSurgeOffsetCounts"() -> (w446:refnum<vi>)
      n390 = control-ref of="Heave distance"() -> (w445:refnum<vi>)
      n391 = control-ref of="Zmm"() -> (w444:refnum<vi>)
      n392 = control-ref of="Heave Pulses/mm"() -> (w443:refnum<vi>)
      n393 = control-ref of="Surge Pulses/mm"() -> (w442:refnum<vi>)
      n394 = control-ref of="Sway Pulses/mm"() -> (w441:refnum<vi>)
      n395 = control-ref of="Heave Pitch"() -> (w440:refnum<vi>)
      n396 = control-ref of="Surge Pitch"() -> (w439:refnum<vi>)
      n397 = control-ref of="Sway Pitch"() -> (w438:refnum<vi>)
      n398 = control-ref of="Heave PPR"() -> (w437:refnum<vi>)
      n399 = control-ref of="Surge PPR"() -> (w436:refnum<vi>)
      n400 = control-ref of="Sway PPR"() -> (w435:refnum<vi>)
      n401 = Bundle By Name(cluster=w476, "Config Parameters.Tab Control 3"=w474, "Config Parameters.Tab Control 19"=w473, "Config Parameters.SAMPLES"=w472, "Config Parameters.Re-initilaize"=w471, "Config Parameters.Filter ON/OFF"=w470, "Config Parameters.TracHomeSurgeOffsetCounts 10MM"=w469, "Config Parameters.TracHomeSwayOffsetCounts 10MM"=w468, "Config Parameters.Acoustic Emission:"=w467, "Config Parameters.Apply Filter (FF)"=w466, "Config Parameters.Filter% 2"=w465, "Config Parameters.Apply Filter (Load)"=w464, "Config Parameters.Filter%"=w463, "Config Parameters.Sway distance (mm)"=w462, "Config Parameters.Surge distance (mm)"=w461, "Config Parameters.DataSavingLoopDelay(ms)"=w460, "Config Parameters.SAVE 2"=w459, "Config Parameters.Enter Distance"=w458, "Config Parameters.Sway Counts:"=w457, "Config Parameters.Distance (mm): 3"=w456, "Config Parameters.Surge Counts:"=w455, "Config Parameters.Distance (mm): 2"=w454, "Config Parameters.Distance (mm):"=w453, "Config Parameters.Heave Counts:"=w452, "Config Parameters.LRMHomeSurgeOffsetCounts"=w451, "Config Parameters.LRMHomeSwayOffsetCounts"=w450, "Config Parameters.TracHomeSurgeOffsetCounts 20MM"=w449, "Config Parameters.TracHomeSwayOffsetCounts 20MM"=w448, "Config Parameters.RotHomeSwayOffsetCounts"=w447, "Config Parameters.RotHomeSurgeOffsetCounts"=w446, "Config Parameters.Heave distance"=w445, "Config Parameters.Zmm"=w444, "Config Parameters.Heave Pulses/mm"=w443, "Config Parameters.Surge Pulses/mm"=w442, "Config Parameters.Sway Pulses/mm"=w441, "Config Parameters.Heave Pitch"=w440, "Config Parameters.Surge Pitch"=w439, "Config Parameters.Sway Pitch"=w438, "Config Parameters.Heave PPR"=w437, "Config Parameters.Surge PPR"=w436, "Config Parameters.Sway PPR"=w435, "Config Parameters.Tab Control 5"=w434, "Config Parameters.Tab Control 14"=w433, "Config Parameters.Tab Control 26"=w432, "Config Parameters.AE"=w431, "Config Parameters.Heave Loop Delay"=w430, "Config Parameters.Heave PID Speed"=w429, "Config Parameters.Surge Jog Speed"=w428, "Config Parameters.Heave Jog Speed"=w427, "Config Parameters.Sway Loop Delay"=w426, "Config Parameters.Sway PID Speed"=w425, "Config Parameters.Sway Jog Speed"=w424, "Config Parameters.DEPTH TRIP VALUE"=w423, "Config Parameters.LOAD TRIP VALUE"=w422, "Config Parameters.DEPTH TRIP   ENABLE"=w421, "Config Parameters.LOAD TRIP  ENABLE"=w420, "Config Parameters.CYCLIC FF TRIP VALUE"=w419, "Config Parameters.FF TRIP VALUE"=w418, "Config Parameters.CYCLIC CoF TRIP VALUE"=w417, "Config Parameters.COF TRIP VALUE"=w416, "Config Parameters.CYCLIC COF TRIP  ENABLE"=w415, "Config Parameters.CYCLIC FF TRIP  ENABLE"=w414, "Config Parameters.FF TRIP  ENABLE"=w413, "Config Parameters.COF TRIP  ENABLE"=w412) -> (w475:T11)
    }
    frame #11 {
      n402 = control-ref of="Mx"() -> (w506:refnum<vi>)
      n403 = control-ref of="My"() -> (w505:refnum<vi>)
      n404 = control-ref of="Mz"() -> (w504:refnum<vi>)
      n405 = control-ref of="Fx(N)"() -> (w503:refnum<vi>)
      n406 = control-ref of="Fy(N)"() -> (w502:refnum<vi>)
      n407 = control-ref of="Fz(N)"() -> (w501:refnum<vi>)
      n408 = control-ref of="Load Cell Temp"() -> (w477:refnum<vi>)
      n409 = control-ref of="ClearAll"() -> (w511:refnum<vi>)
      n410 = control-ref of="ZeroAll"() -> (w500:refnum<vi>)
      n411 = control-ref of="delete Handle"() -> (w490:refnum<vi>)
      n412 = control-ref of="Create Handle"() -> (w489:refnum<vi>)
      n413 = control-ref of="stop 6"() -> (w486:refnum<vi>)
      n414 = control-ref of="running_flag"() -> (w485:refnum<vi>)
      n415 = control-ref of="Save Dwell"() -> (w507:refnum<vi>)
      n416 = control-ref of="Acq Delay (ms)"() -> (w499:refnum<vi>)
      n417 = control-ref of="Burst Delay (ms)"() -> (w498:refnum<vi>)
      n418 = control-ref of="SN"() -> (w496:refnum<vi>)
      n419 = control-ref of="Port"() -> (w493:refnum<vi>)
      n420 = control-ref of="ft_udp_handle"() -> (w484:refnum<vi>)
      n421 = control-ref of="get-data-return"() -> (w483:refnum<vi>)
      n422 = control-ref of="get-range-return"() -> (w482:refnum<vi>)
      n423 = control-ref of="zero-return"() -> (w481:refnum<vi>)
      n424 = control-ref of="filter-return"() -> (w480:refnum<vi>)
      n425 = control-ref of="initial-return"() -> (w479:refnum<vi>)
      n426 = control-ref of="deleteHandle-result"() -> (w478:refnum<vi>)
      n427 = control-ref of="model"() -> (w497:refnum<vi>)
      n428 = control-ref of="Sensor IP"() -> (w494:refnum<vi>)
      n429 = control-ref of="Mz(Nm)"() -> (w510:refnum<vi>)
      n430 = control-ref of="My(Nm)"() -> (w509:refnum<vi>)
      n431 = control-ref of="Mx(Nm)"() -> (w508:refnum<vi>)
      n432 = control-ref of="FFx(N)"() -> (w495:refnum<vi>)
      n433 = control-ref of="FFy(N)"() -> (w492:refnum<vi>)
      n434 = control-ref of="Load(N)"() -> (w491:refnum<vi>)
      n435 = control-ref of="ft_data"() -> (w488:refnum<vi>)
      n436 = control-ref of="ft_range"() -> (w487:refnum<vi>)
      n437 = Bundle By Name(cluster=w513, "Loading Com Port.ClearAll"=w511, "Loading Com Port.Mz(Nm)"=w510, "Loading Com Port.My(Nm)"=w509, "Loading Com Port.Mx(Nm)"=w508, "Loading Com Port.Save Dwell"=w507, "Loading Com Port.Mx"=w506, "Loading Com Port.My"=w505, "Loading Com Port.Mz"=w504, "Loading Com Port.Fx(N)"=w503, "Loading Com Port.Fy(N)"=w502, "Loading Com Port.Fz(N)"=w501, "Loading Com Port.ZeroAll"=w500, "Loading Com Port.Acq Delay (ms)"=w499, "Loading Com Port.Burst Delay (ms)"=w498, "Loading Com Port.model"=w497, "Loading Com Port.SN"=w496, "Loading Com Port.FFx(N)"=w495, "Loading Com Port.Sensor IP"=w494, "Loading Com Port.Port"=w493, "Loading Com Port.FFy(N)"=w492, "Loading Com Port.Load(N)"=w491, "Loading Com Port.delete Handle"=w490, "Loading Com Port.Create Handle"=w489, "Loading Com Port.ft_data"=w488, "Loading Com Port.ft_range"=w487, "Loading Com Port.stop 6"=w486, "Loading Com Port.running_flag"=w485, "Loading Com Port.ft_udp_handle"=w484, "Loading Com Port.get-data-return"=w483, "Loading Com Port.get-range-return"=w482, "Loading Com Port.zero-return"=w481, "Loading Com Port.filter-return"=w480, "Loading Com Port.initial-return"=w479, "Loading Com Port.deleteHandle-result"=w478, "Loading Com Port.Load Cell Temp"=w477) -> (w512:T11)
    }
    frame #12 {
      n438 = control-ref of="Manual Write Heave & Surge"() -> (w515:refnum<vi>)
      n439 = control-ref of="Read Heave Temp"() -> (w538:refnum<vi>)
      n440 = control-ref of="error out Read"() -> (w550:refnum<vi>)
      n441 = control-ref of="error out Write"() -> (w545:refnum<vi>)
      n442 = control-ref of="SURGE POSE"() -> (w551:refnum<vi>)
      n443 = control-ref of="HEAVE POSE"() -> (w549:refnum<vi>)
      n444 = control-ref of="State"() -> (w548:refnum<vi>)
      n445 = control-ref of="Homed"() -> (w547:refnum<vi>)
      n446 = control-ref of="Sequence ID"() -> (w546:refnum<vi>)
      n447 = control-ref of="faultCode"() -> (w544:refnum<vi>)
      n448 = control-ref of="Ack ID"() -> (w543:refnum<vi>)
      n449 = control-ref of="SPEED"() -> (w542:refnum<vi>)
      n450 = control-ref of="Distance"() -> (w541:refnum<vi>)
      n451 = control-ref of="Mode Command"() -> (w540:refnum<vi>)
      n452 = control-ref of="SPARE 2"() -> (w537:refnum<vi>)
      n453 = control-ref of="SPARE 1"() -> (w536:refnum<vi>)
      n454 = control-ref of="Spare 15"() -> (w535:refnum<vi>)
      n455 = control-ref of="Spare 14"() -> (w534:refnum<vi>)
      n456 = control-ref of="Spare 13"() -> (w533:refnum<vi>)
      n457 = control-ref of="Spare 12"() -> (w532:refnum<vi>)
      n458 = control-ref of="Spare 11"() -> (w531:refnum<vi>)
      n459 = control-ref of="Spare 10"() -> (w530:refnum<vi>)
      n460 = control-ref of="Spare 9"() -> (w529:refnum<vi>)
      n461 = control-ref of="Spare 8"() -> (w528:refnum<vi>)
      n462 = control-ref of="Spare 7"() -> (w527:refnum<vi>)
      n463 = control-ref of="Spare 6"() -> (w526:refnum<vi>)
      n464 = control-ref of="Spare 5"() -> (w525:refnum<vi>)
      n465 = control-ref of="Spare 4"() -> (w524:refnum<vi>)
      n466 = control-ref of="Spare 3"() -> (w523:refnum<vi>)
      n467 = control-ref of="Spare 2"() -> (w522:refnum<vi>)
      n468 = control-ref of="Spare 1"() -> (w521:refnum<vi>)
      n469 = control-ref of="Node Id"() -> (w520:refnum<vi>)
      n470 = control-ref of="SPARE 3"() -> (w519:refnum<vi>)
      n471 = control-ref of="SPARE 4"() -> (w518:refnum<vi>)
      n472 = control-ref of="fwMajor"() -> (w517:refnum<vi>)
      n473 = control-ref of="fwMinor"() -> (w516:refnum<vi>)
      n474 = control-ref of="Heave and Surge Write"() -> (w514:refnum<vi>)
      n475 = control-ref of="Heave and Surge Read"() -> (w539:refnum<vi>)
      n476 = Bundle By Name(cluster=w553, "Heave AND Surge.SURGE POSE"=w551, "Heave AND Surge.error out Read"=w550, "Heave AND Surge.HEAVE POSE"=w549, "Heave AND Surge.State"=w548, "Heave AND Surge.Homed"=w547, "Heave AND Surge.Sequence ID"=w546, "Heave AND Surge.error out Write"=w545, "Heave AND Surge.faultCode"=w544, "Heave AND Surge.Ack ID"=w543, "Heave AND Surge.SPEED"=w542, "Heave AND Surge.Distance"=w541, "Heave AND Surge.Mode Command"=w540, "Heave AND Surge.Heave and Surge Read"=w539, "Heave AND Surge.Read Heave Temp"=w538, "Heave AND Surge.SPARE 2"=w537, "Heave AND Surge.SPARE 1"=w536, "Heave AND Surge.Spare 15"=w535, "Heave AND Surge.Spare 14"=w534, "Heave AND Surge.Spare 13"=w533, "Heave AND Surge.Spare 12"=w532, "Heave AND Surge.Spare 11"=w531, "Heave AND Surge.Spare 10"=w530, "Heave AND Surge.Spare 9"=w529, "Heave AND Surge.Spare 8"=w528, "Heave AND Surge.Spare 7"=w527, "Heave AND Surge.Spare 6"=w526, "Heave AND Surge.Spare 5"=w525, "Heave AND Surge.Spare 4"=w524, "Heave AND Surge.Spare 3"=w523, "Heave AND Surge.Spare 2"=w522, "Heave AND Surge.Spare 1"=w521, "Heave AND Surge.Node Id"=w520, "Heave AND Surge.SPARE 3"=w519, "Heave AND Surge.SPARE 4"=w518, "Heave AND Surge.fwMajor"=w517, "Heave AND Surge.fwMinor"=w516, "Heave AND Surge.Manual Write"=w515, "Heave AND Surge.Heave and Surge Write"=w514) -> (w552:T11)
    }
    frame #13 {
      n477 = control-ref of="Fine Tune Zone"() -> (w569:refnum<vi>)
      n478 = control-ref of="PID Delay (sec)"() -> (w568:refnum<vi>)
      n479 = control-ref of="Max_pos_limit"() -> (w567:refnum<vi>)
      n480 = control-ref of="Min_pos_limit"() -> (w566:refnum<vi>)
      n481 = control-ref of="i_limit"() -> (w565:refnum<vi>)
      n482 = control-ref of="pct_scale"() -> (w556:refnum<vi>)
      n483 = control-ref of="Deadband"() -> (w564:refnum<vi>)
      n484 = control-ref of="Kd"() -> (w563:refnum<vi>)
      n485 = control-ref of="Ki"() -> (w562:refnum<vi>)
      n486 = control-ref of="Kp"() -> (w561:refnum<vi>)
      n487 = control-ref of="Current Position"() -> (w560:refnum<vi>)
      n488 = control-ref of="Set Load"() -> (w559:refnum<vi>)
      n489 = control-ref of="Current Load"() -> (w558:refnum<vi>)
      n490 = control-ref of="Pulse delta"() -> (w557:refnum<vi>)
      n491 = control-ref of="Init Step"() -> (w555:refnum<vi>)
      n492 = control-ref of="Max Step Linit"() -> (w554:refnum<vi>)
      n493 = Bundle By Name(cluster=w571, "New PID LOGIC.Fine Tune Zone"=w569, "New PID LOGIC.PID SDelay"=w568, "New PID LOGIC.Max_pos_limit"=w567, "New PID LOGIC.Min_pos_limit"=w566, "New PID LOGIC.i_limit"=w565, "New PID LOGIC.pct_scale"=w556, "New PID LOGIC.Deadband"=w564, "New PID LOGIC.Kd"=w563, "New PID LOGIC.Ki"=w562, "New PID LOGIC.Kp"=w561, "New PID LOGIC.Current Position"=w560, "New PID LOGIC.Set Load"=w559, "New PID LOGIC.Current Load"=w558, "New PID LOGIC.Pulse delta"=w557, "New PID LOGIC.Init Step"=w555, "New PID LOGIC.Max Step Linit"=w554) -> (w570:T11)
    }
    frame #14 {
      n494 = control-ref of="Manual Write SWAY"() -> (w591:refnum<vi>)
      n495 = control-ref of="Read SWAY Temp"() -> (w572:refnum<vi>)
      n496 = control-ref of="error out Write  SWAY"() -> (w593:refnum<vi>)
      n497 = control-ref of="error out Read SWAY"() -> (w592:refnum<vi>)
      n498 = control-ref of="fwMajor"() -> (w610:refnum<vi>)
      n499 = control-ref of="Homed"() -> (w609:refnum<vi>)
      n500 = control-ref of="Rotary POSE"() -> (w608:refnum<vi>)
      n501 = control-ref of="State"() -> (w607:refnum<vi>)
      n502 = control-ref of="SWAY POSE"() -> (w606:refnum<vi>)
      n503 = control-ref of="Ack ID"() -> (w605:refnum<vi>)
      n504 = control-ref of="faultCode"() -> (w604:refnum<vi>)
      n505 = control-ref of="Node Id"() -> (w603:refnum<vi>)
      n506 = control-ref of="fwMinor"() -> (w602:refnum<vi>)
      n507 = control-ref of="Spare 6"() -> (w601:refnum<vi>)
      n508 = control-ref of="Spare 5"() -> (w600:refnum<vi>)
      n509 = control-ref of="Spare 4"() -> (w599:refnum<vi>)
      n510 = control-ref of="Spare 3"() -> (w598:refnum<vi>)
      n511 = control-ref of="Spare 2"() -> (w597:refnum<vi>)
      n512 = control-ref of="Spare 1"() -> (w596:refnum<vi>)
      n513 = control-ref of="Spare 7"() -> (w595:refnum<vi>)
      n514 = control-ref of="SPARE  5"() -> (w594:refnum<vi>)
      n515 = control-ref of="SPARE  4"() -> (w589:refnum<vi>)
      n516 = control-ref of="SPARE  3"() -> (w588:refnum<vi>)
      n517 = control-ref of="SPARE 2"() -> (w587:refnum<vi>)
      n518 = control-ref of="SPARE 1"() -> (w586:refnum<vi>)
      n519 = control-ref of="Spare 15"() -> (w585:refnum<vi>)
      n520 = control-ref of="Spare 14"() -> (w584:refnum<vi>)
      n521 = control-ref of="Spare 13"() -> (w583:refnum<vi>)
      n522 = control-ref of="Spare 12"() -> (w582:refnum<vi>)
      n523 = control-ref of="Spare 11"() -> (w581:refnum<vi>)
      n524 = control-ref of="Spare 9"() -> (w580:refnum<vi>)
      n525 = control-ref of="Spare 8"() -> (w579:refnum<vi>)
      n526 = control-ref of="SPEED"() -> (w578:refnum<vi>)
      n527 = control-ref of="Distance"() -> (w577:refnum<vi>)
      n528 = control-ref of="Mode Command"() -> (w576:refnum<vi>)
      n529 = control-ref of="Sequence ID"() -> (w575:refnum<vi>)
      n530 = control-ref of="Spare 10"() -> (w573:refnum<vi>)
      n531 = control-ref of="SWAY WRITE"() -> (w590:refnum<vi>)
      n532 = control-ref of="SWAY READ"() -> (w574:refnum<vi>)
      n533 = Bundle By Name(cluster=w612, "SWAY.fwMajor"=w610, "SWAY.Homed"=w609, "SWAY.Rotary POSE"=w608, "SWAY.State"=w607, "SWAY.SWAY POSE"=w606, "SWAY.Ack ID"=w605, "SWAY.faultCode"=w604, "SWAY.Node Id"=w603, "SWAY.fwMinor"=w602, "SWAY.Spare 6"=w601, "SWAY.Spare 5"=w600, "SWAY.Spare 4"=w599, "SWAY.Spare 3"=w598, "SWAY.Spare 2"=w597, "SWAY.Spare 1"=w596, "SWAY.Spare 7"=w595, "SWAY.SPARE  5"=w594, "SWAY.error out Write  SWAY"=w593, "SWAY.error out Read SWAY"=w592, "SWAY.Manual Write SWAY"=w591, "SWAY.SWAY WRITE"=w590, "SWAY.SPARE  4"=w589, "SWAY.SPARE  3"=w588, "SWAY.SPARE 2"=w587, "SWAY.SPARE 1"=w586, "SWAY.Spare 15"=w585, "SWAY.Spare 14"=w584, "SWAY.Spare 13"=w583, "SWAY.Spare 12"=w582, "SWAY.Spare 11"=w581, "SWAY.Spare 9"=w580, "SWAY.Spare 8"=w579, "SWAY.SPEED"=w578, "SWAY.Distance"=w577, "SWAY.Mode Command"=w576, "SWAY.Sequence ID"=w575, "SWAY.SWAY READ"=w574, "SWAY.Spare 10"=w573, "SWAY.Read SWAY Temp"=w572) -> (w611:T11)
    }
    frame #15 {
      n534 = control-ref of="Analysis Home new"() -> (w643:refnum<vi>)
      n535 = control-ref of="Refresh 2"() -> (w642:refnum<vi>)
      n536 = control-ref of="OPEN 4"() -> (w628:refnum<vi>)
      n537 = control-ref of="OPEN 3"() -> (w626:refnum<vi>)
      n538 = control-ref of="XY Graph"() -> (w621:refnum<vi>)
      n539 = control-ref of="OPEN 2"() -> (w618:refnum<vi>)
      n540 = control-ref of="OPEN 1"() -> (w617:refnum<vi>)
      n541 = control-ref of="Export"() -> (w614:refnum<vi>)
      n542 = control-ref of="MEAN"() -> (w641:refnum<vi>)
      n543 = control-ref of="SD"() -> (w640:refnum<vi>)
      n544 = control-ref of="VARIANCE"() -> (w639:refnum<vi>)
      n545 = control-ref of="MEAN"() -> (w638:refnum<vi>)
      n546 = control-ref of="SD"() -> (w637:refnum<vi>)
      n547 = control-ref of="VARIANCE"() -> (w636:refnum<vi>)
      n548 = control-ref of="MEAN"() -> (w635:refnum<vi>)
      n549 = control-ref of="SD"() -> (w634:refnum<vi>)
      n550 = control-ref of="VARIANCE"() -> (w633:refnum<vi>)
      n551 = control-ref of="MEAN"() -> (w632:refnum<vi>)
      n552 = control-ref of="SD"() -> (w631:refnum<vi>)
      n553 = control-ref of="VARIANCE"() -> (w630:refnum<vi>)
      n554 = control-ref of="File 4 Discription"() -> (w629:refnum<vi>)
      n555 = control-ref of="File Name 4"() -> (w627:refnum<vi>)
      n556 = control-ref of="File 3 Discription"() -> (w625:refnum<vi>)
      n557 = control-ref of="File Name 3"() -> (w624:refnum<vi>)
      n558 = control-ref of="File Name 2"() -> (w620:refnum<vi>)
      n559 = control-ref of="File Name 1"() -> (w619:refnum<vi>)
      n560 = control-ref of="File 1 Discription"() -> (w616:refnum<vi>)
      n561 = control-ref of="File 2 Discription"() -> (w615:refnum<vi>)
      n562 = control-ref of="Y-AXIS"() -> (w623:refnum<vi>)
      n563 = control-ref of="X-AXIS"() -> (w622:refnum<vi>)
      n564 = control-ref of="File Format"() -> (w613:refnum<vi>)
      n565 = Bundle By Name(cluster=w645, "Analysis Screen.Analysis Home"=w643, "Analysis Screen.Refresh 2"=w642, "Analysis Screen.MEAN 4"=w641, "Analysis Screen.SD 4"=w640, "Analysis Screen.VARIANCE 4"=w639, "Analysis Screen.MEAN  3"=w638, "Analysis Screen.SD  3"=w637, "Analysis Screen.VARIANCE  3"=w636, "Analysis Screen.MEAN 2"=w635, "Analysis Screen.SD  2"=w634, "Analysis Screen.VARIANCE 2"=w633, "Analysis Screen.MEAN"=w632, "Analysis Screen.SD"=w631, "Analysis Screen.VARIANCE"=w630, "Analysis Screen.File 4 Discription"=w629, "Analysis Screen.OPEN 4"=w628, "Analysis Screen.File Name 4"=w627, "Analysis Screen.OPEN 3"=w626, "Analysis Screen.File 3 Discription"=w625, "Analysis Screen.File Name 3"=w624, "Analysis Screen.Y-AXIS"=w623, "Analysis Screen.X-AXIS"=w622, "Analysis Screen.XY Graph"=w621, "Analysis Screen.File Name 2"=w620, "Analysis Screen.File Name 1"=w619, "Analysis Screen.OPEN 2"=w618, "Analysis Screen.OPEN 1"=w617, "Analysis Screen.File 1 Discription"=w616, "Analysis Screen.File 2 Discription"=w615, "Analysis Screen.Export"=w614, "Analysis Screen.File Format"=w613) -> (w644:T11)
    }
  }
  n566 = call <userlib>:"Fit VI window to Largest Dec.vi"() -> ("error out"=w42:errorcluster, "dup VI Ref"=w39:refnum<vi>)  [unwired: 6 in]
  n567 = invoke on="Invoke Node" class="VI" method="FP.Run-Time Position.Maximized"(reference=w39, error in=w42) -> (error out=w41:errorcluster)  [unwired: 2 in, 3 out]
  n568 = call <vilib>:"Clear Errors.vi"("error in (no error)"=w41) -> ("error out"=w40:errorcluster)  [unwired: 5 in, 1 out]
  n569 = control-ref of="This VI"() -> (w45:refnum<vi>)
  n570 = invoke on="Invoke Node" class="VI" method="Default Vals.Reinit All"(reference=w45, error in=w40) -> (reference out=w43:refnum<vi>, error out=w44:errorcluster)  [unwired: 1 in, 1 out]
  n571 = Close Reference(reference=w43, error in (no error)=w44) -> (error out=w38:errorcluster)
  n572 = call "Create User Event - Stop.vi"("error in (no error)"=w38) -> ("error out"=w16:errorcluster, "User Event - Stop"=w25:refnum<user-event>)  [unwired: 9 in]
  n573 = call "main screen queue out Unitest.vi"("error in (no error)"=w16) -> ("error out"=w65:errorcluster, "output Queue"=w37:T12)  [unwired: 9 in]
  n574 = Unbundle By Name(w37) -> ("RAMP MOTOR COM LOOP"=w30:refnum<queue>)
  n575 = Unbundle By Name(w37) -> ("TEMPERATURE COM LOOP"=w32:refnum<queue>)
  n576 = Unbundle By Name(w37) -> ("ECR PORT"=w29:refnum<queue>)
  n577 = Unbundle By Name(w37) -> ("SWAY MOTOR COM LOOP"=w34:refnum<queue>)
  n578 = Unbundle By Name(w37) -> ("UI Loop"=w63:refnum<queue>)
  n579 = Unbundle By Name(w37) -> ("LOAD COM LOOP"=w35:refnum<queue>)
  n580 = Unbundle By Name(w37) -> ("HEAVE MOTOR COM LOOP"=w17:refnum<queue>)
  n581 = Unbundle By Name(w37) -> ("HUMIDITY COM PORT"=w28:refnum<queue>)
  n582 = Unbundle By Name(w37) -> ("PROGRAM LOOP"=w27:refnum<queue>)
  n583 = Unbundle By Name(w37) -> ("MONITOR LOOP"=w24:refnum<queue>)
  n584 = Unbundle By Name(w37) -> ("LOAD PID"=w23:refnum<queue>)
  n585 = Unbundle By Name(w37) -> ("REPORT"=w22:refnum<queue>)
  n586 = register-events(w25) -> (reference out=w57:refnum<event-registration>, error out=w55:errorcluster)  [unwired: 2 in]
  n587 = Merge Errors(w55, w65) -> (w56:errorcluster)
  n588 = disable-structure shown="Enabled" {
    disable-tunnel: w26 -> [w649 _]
    disable-tunnel: w25 -> [w648 _]
    disable-tunnel: w22 -> [w647 _]
    disable-tunnel: w16 -> [w646 _]
    frame Enabled {
      n589 = node-c288() -> (w651:T13)  [unwired: 4 in]
      n590 = timed-loop {
        shift-right: [w662] -> _
        shift-left: w649 -> [w663]
        tunnel: [w656] -> _
        tunnel: w647 -> [w654]
        tunnel: w646 -> [w653]
        tunnel: w648 -> [w652]
        timing: w651 -> [_]
        timing-out: [_] -> w650
        stop <- w661 stop-if-true
        # "Report  Handling Loop"
        n591 = node-c288() -> ()  [unwired: 1 in, 1 out]
        n592 = call "Dequeue Message.vi"("error in (no error)"=w653, "Message Queue"=w654) -> ("error out"=w660:errorcluster, "Message Data"=w658:variant, "Message"=w659:string, "dup Message Queue"=w657:refnum<queue>)  [unwired: 6 in]
        n593 = case "Message Cases" shown="\"Report Main\"" w659 {
          selector: w659 -> [_ _ _ _ _ w710]
          tunnel: w657 -> [w666 w678 _ w697 w709 _]
          tunnel: w660 -> [w669 w676 w694 w701 w703 _]
          tunnel: [w670 w679 w688 w699 w705 w711] -> w655
          tunnel: w663 -> [w668 w671 w693 w700 w708 w712]
          tunnel: [w668 w671 w693 w700 w708 w712] -> w662
          tunnel: [_ _ _ _ TRUE _] -> w661
          tunnel: w658 -> [_ _ w692 _ _ _]
          tunnel: w652 -> [_ _ _ _ w702 _]
          frame "init" {
            # "Initialize - All initialization work should take place in this message, since other loops can potentially enqueue messages that execute immediately after this one."
            n594 = call-poly "Enqueue Message.vi"("error in (no error)"=w669, "Message"="Report Main", "Message Queue"=w666) -> ("error out"=w670:errorcluster)  [unwired: 7 in, 1 out]
          }
          frame "Report Main" {
            n595 = call "Main Data Log.vi"("error in (no error)"=w676, "main ref"=w671) -> ("error out"=w672:errorcluster)  [unwired: 9 in]
            n596 = Unbundle By Name(w671) -> ("Main Home Screen.EXIT"=w677:refnum<vi>)
            n597 = property class="Bool (strict)"(reference=w677) -> (reference out=w674:refnum<vi>, error out=w675:errorcluster, "Value"=w673:bool)  [unwired: 1 in]
            n598 = case shown="False" w673 {
              tunnel: [w682 w686] -> w679
              tunnel: w678 -> [w681 w685]
              tunnel: w672 -> [w680 w684]
              frame True {
                n599 = call-poly "Enqueue Message.vi"("error in (no error)"=w680, "Message"="Confirm Quit", "Message Queue"=w681) -> ("error out"=w682:errorcluster)  [unwired: 7 in, 1 out]
              }
              frame False {
                n600 = call-poly "Enqueue Message.vi"("error in (no error)"=w684, "Message"="Report Main", "Message Queue"=w685) -> ("error out"=w686:errorcluster)  [unwired: 7 in, 1 out]
              }
            }
            n601 = Close Reference(reference=w674, error in (no error)=w675) -> ()  [unwired: 1 out]
          }
          frame "Error" {
            # "#CodeRecommended - If you ever change the name of this \"Error\" message, you'll need to update the name in the Check Loop Error.vi as well."
            # "#CodeRecommended - Consider creating a system for logging errors in some way. These errors are for notification purposes only. Handling of specific errors should be performed in the message frames that generated the error."
            # "Error - Display an error dialog. This message is sent by the \"Error Handler\" VIs at the end of other loops in this application."
            n602 = Variant To Data(error in=w694, type=errorcluster {"status"=FALSE, "code"=0, "source"=""} ("error constant"), Variant=w692) -> (data=w690:errorcluster, error out=w689:errorcluster)
            n603 = call <vilib>:"Simple Error Handler.vi"("error in (no error)"=w690) -> ()  [unwired: 4 in, 5 out]
            n604 = Merge Errors(w689) -> (w688:errorcluster)
          }
          frame "Confirm Quit" {
            # "#CodeNeeded - If you want to provide an \"Are you sure\" dialog (or some other notification) before the application exits, place that code here. This message is typically sent from a Panel Close? event."
            # "Confirm Quit - Message that can confirm whether or not the user wants to exit the application."
            n605 = call-poly "Enqueue Message.vi"("Priority Message? (F)"=TRUE, "error in (no error)"=w701, "Message"="Exit", "Message Queue"=w697) -> ("error out"=w698:errorcluster)  [unwired: 6 in, 1 out]
            n606 = Merge Errors(w698) -> (w699:errorcluster)
          }
          frame "Exit" {
            # "Stop the VI"
            # "Release the message queue reference"
            # "#CodeNeeded - Add any required cleanup code here. Note that if 'Exit' was called as a result of an error, an error dialog will be displayed. Add any custom error handling for an 'Exit' condition here as well."
            # "Exit - Exit the application."
            n607 = call "Fire User Event - Stop.vi"("User Event - Stop"=w702) -> ("error out"=w704:errorcluster)  [unwired: 10 in]
            n608 = Release Queue(queue=w709, error in (no error)=w703) -> (error out=w706:errorcluster)  [unwired: 1 in, 2 out]
            n609 = Merge Errors(w704, w706) -> (w705:errorcluster)
          }
          frame Default {
            # "'Default' case only runs if there is a message that isn't defined in any of the other cases.  Output a programming error."
            n610 = xnode "Error Ring"("parameter 0"=w710) -> ("error out"=w711:errorcluster)
          }
        }
        n611 = node-c288() -> ()  [unwired: 1 in, 1 out]
        n612 = call "LAB-IQ Error Handler - Message Handling Loop.vi"("error in (no error)"=w655, "Message Queue"=w657) -> ("dup error in"=w656:errorcluster)  [unwired: 8 in, 1 out]
      }
      n613 = node-c288(w650) -> ()  [unwired: 1 out]
    }
    frame Disabled {
    }
  }
  n614 = node-c288() -> (w3:T13)  [unwired: 4 in]
  n615 = node-c288() -> (w9:T13)  [unwired: 4 in]
  n616 = node-c288() -> (w5:T13)  [unwired: 4 in]
  n617 = node-c288() -> (w7:T13)  [unwired: 4 in]
  n618 = node-c288() -> (w11:T13)  [unwired: 4 in]
  n619 = disable-structure shown="Disabled" {
    disable-tunnel: w28 -> [w725 _]
    disable-tunnel: w26 -> [w724 _]
    disable-tunnel: w25 -> [w723 _]
    disable-tunnel: w16 -> [w722 _]
    frame Disabled {
      n620 = while {
        shift-right: [w736] -> _
        shift-left: w724 -> [w737]
        tunnel: [w730] -> _
        tunnel: w725 -> [w728]
        tunnel: w722 -> [w727]
        tunnel: w723 -> [w726]
        stop <- w735 stop-if-true
        # "Humidity  Handling Loop"
        n621 = call "Dequeue Message.vi"("error in (no error)"=w727, "Message Queue"=w728) -> ("error out"=w734:errorcluster, "Message Data"=w732:variant, "Message"=w733:string, "dup Message Queue"=w731:refnum<queue>)  [unwired: 6 in]
        n622 = case "Message Cases" shown="\"Humidity Main\"" w733 {
          selector: w733 -> [_ _ _ _ _ w781]
          tunnel: w731 -> [w738 w749 _ w768 w780 _]
          tunnel: w734 -> [w741 w746 w765 w772 w774 _]
          tunnel: [w742 w750 w759 w770 w776 w782] -> w729
          tunnel: w737 -> [w740 w748 w764 w771 w779 w783]
          tunnel: [w740 w748 w764 w771 w779 w783] -> w736
          tunnel: [_ _ _ _ TRUE _] -> w735
          tunnel: w732 -> [_ _ w763 _ _ _]
          tunnel: w726 -> [_ _ _ _ w773 _]
          frame "init" {
            # "Initialize - All initialization work should take place in this message, since other loops can potentially enqueue messages that execute immediately after this one."
            n623 = call-poly "Enqueue Message.vi"("error in (no error)"=w741, "Message"="Humidity Main", "Message Queue"=w738) -> ("error out"=w742:errorcluster)  [unwired: 7 in, 1 out]
          }
          frame "Humidity Main" {
            n624 = Unbundle By Name(w748) -> ("Main Home Screen.EXIT"=w747:refnum<vi>)
            n625 = property class="Bool (strict)"(reference=w747) -> (reference out=w744:refnum<vi>, error out=w745:errorcluster, "Value"=w743:bool)  [unwired: 1 in]
            n626 = case shown="False" w743 {
              tunnel: [w753 w757] -> w750
              tunnel: w749 -> [w752 w756]
              tunnel: w746 -> [w751 w755]
              frame True {
                n627 = call-poly "Enqueue Message.vi"("error in (no error)"=w751, "Message"="Confirm Quit", "Message Queue"=w752) -> ("error out"=w753:errorcluster)  [unwired: 7 in, 1 out]
              }
              frame False {
                n628 = call-poly "Enqueue Message.vi"("error in (no error)"=w755, "Message"="Humidity Main", "Message Queue"=w756) -> ("error out"=w757:errorcluster)  [unwired: 7 in, 1 out]
              }
            }
            n629 = Close Reference(reference=w744, error in (no error)=w745) -> ()  [unwired: 1 out]
          }
          frame "Error" {
            # "#CodeRecommended - If you ever change the name of this \"Error\" message, you'll need to update the name in the Check Loop Error.vi as well."
            # "#CodeRecommended - Consider creating a system for logging errors in some way. These errors are for notification purposes only. Handling of specific errors should be performed in the message frames that generated the error."
            # "Error - Display an error dialog. This message is sent by the \"Error Handler\" VIs at the end of other loops in this application."
            n630 = Variant To Data(error in=w765, type=errorcluster {"status"=FALSE, "code"=0, "source"=""} ("error constant"), Variant=w763) -> (data=w761:errorcluster, error out=w760:errorcluster)
            n631 = call <vilib>:"Simple Error Handler.vi"("error in (no error)"=w761) -> ()  [unwired: 4 in, 5 out]
            n632 = Merge Errors(w760) -> (w759:errorcluster)
          }
          frame "Confirm Quit" {
            # "#CodeNeeded - If you want to provide an \"Are you sure\" dialog (or some other notification) before the application exits, place that code here. This message is typically sent from a Panel Close? event."
            # "Confirm Quit - Message that can confirm whether or not the user wants to exit the application."
            n633 = call-poly "Enqueue Message.vi"("Priority Message? (F)"=TRUE, "error in (no error)"=w772, "Message"="Exit", "Message Queue"=w768) -> ("error out"=w769:errorcluster)  [unwired: 6 in, 1 out]
            n634 = Merge Errors(w769) -> (w770:errorcluster)
          }
          frame "Exit" {
            # "Stop the VI"
            # "Release the message queue reference"
            # "#CodeNeeded - Add any required cleanup code here. Note that if 'Exit' was called as a result of an error, an error dialog will be displayed. Add any custom error handling for an 'Exit' condition here as well."
            # "Exit - Exit the application."
            n635 = call "Fire User Event - Stop.vi"("User Event - Stop"=w773) -> ("error out"=w775:errorcluster)  [unwired: 10 in]
            n636 = Release Queue(queue=w780, error in (no error)=w774) -> (error out=w777:errorcluster)  [unwired: 1 in, 2 out]
            n637 = Merge Errors(w775, w777) -> (w776:errorcluster)
          }
          frame Default {
            # "'Default' case only runs if there is a message that isn't defined in any of the other cases.  Output a programming error."
            n638 = xnode "Error Ring"("parameter 0"=w781) -> ("error out"=w782:errorcluster)
          }
        }
        n639 = call "LAB-IQ Error Handler - Message Handling Loop.vi"("error in (no error)"=w729, "Message Queue"=w731) -> ("dup error in"=w730:errorcluster)  [unwired: 8 in, 1 out]
      }
    }
    frame Enabled {
    }
  }
  n640 = disable-structure shown="Enabled" {
    disable-tunnel: w29 -> [w794 _]
    disable-tunnel: w26 -> [w793 _]
    disable-tunnel: w25 -> [w792 _]
    disable-tunnel: w16 -> [w791 w860]
    disable-tunnel: [_ w860] -> _
    frame Disabled {
      n641 = while {
        shift-right: [w805] -> _
        shift-left: w793 -> [w806]
        tunnel: [w799] -> _
        tunnel: w794 -> [w797]
        tunnel: w791 -> [w796]
        tunnel: w792 -> [w795]
        stop <- w804 stop-if-true
        # "ECR  Handling Loop"
        n642 = call "Dequeue Message.vi"("error in (no error)"=w796, "Message Queue"=w797) -> ("error out"=w803:errorcluster, "Message Data"=w801:variant, "Message"=w802:string, "dup Message Queue"=w800:refnum<queue>)  [unwired: 6 in]
        n643 = case "Message Cases" shown="\"ECR Main\"" w802 {
          selector: w802 -> [_ _ _ _ _ w850]
          tunnel: w800 -> [w807 w818 _ w837 w849 _]
          tunnel: w803 -> [w810 w815 w834 w841 w843 _]
          tunnel: [w811 w819 w828 w839 w845 w851] -> w798
          tunnel: w806 -> [w809 w817 w833 w840 w848 w852]
          tunnel: [w809 w817 w833 w840 w848 w852] -> w805
          tunnel: [_ _ _ _ TRUE _] -> w804
          tunnel: w801 -> [_ _ w832 _ _ _]
          tunnel: w795 -> [_ _ _ _ w842 _]
          frame "init" {
            # "Initialize - All initialization work should take place in this message, since other loops can potentially enqueue messages that execute immediately after this one."
            n644 = call-poly "Enqueue Message.vi"("error in (no error)"=w810, "Message"="ECR Main", "Message Queue"=w807) -> ("error out"=w811:errorcluster)  [unwired: 7 in, 1 out]
          }
          frame "ECR Main" {
            n645 = Unbundle By Name(w817) -> ("Main Home Screen.EXIT"=w816:refnum<vi>)
            n646 = property class="Bool (strict)"(reference=w816) -> (reference out=w813:refnum<vi>, error out=w814:errorcluster, "Value"=w812:bool)  [unwired: 1 in]
            n647 = case shown="False" w812 {
              tunnel: [w822 w826] -> w819
              tunnel: w818 -> [w821 w825]
              tunnel: w815 -> [w820 w824]
              frame True {
                n648 = call-poly "Enqueue Message.vi"("error in (no error)"=w820, "Message"="Confirm Quit", "Message Queue"=w821) -> ("error out"=w822:errorcluster)  [unwired: 7 in, 1 out]
              }
              frame False {
                n649 = call-poly "Enqueue Message.vi"("error in (no error)"=w824, "Message"="ECR Main", "Message Queue"=w825) -> ("error out"=w826:errorcluster)  [unwired: 7 in, 1 out]
              }
            }
            n650 = Close Reference(reference=w813, error in (no error)=w814) -> ()  [unwired: 1 out]
          }
          frame "Error" {
            # "#CodeRecommended - If you ever change the name of this \"Error\" message, you'll need to update the name in the Check Loop Error.vi as well."
            # "#CodeRecommended - Consider creating a system for logging errors in some way. These errors are for notification purposes only. Handling of specific errors should be performed in the message frames that generated the error."
            # "Error - Display an error dialog. This message is sent by the \"Error Handler\" VIs at the end of other loops in this application."
            n651 = Variant To Data(error in=w834, type=errorcluster {"status"=FALSE, "code"=0, "source"=""} ("error constant"), Variant=w832) -> (data=w830:errorcluster, error out=w829:errorcluster)
            n652 = call <vilib>:"Simple Error Handler.vi"("error in (no error)"=w830) -> ()  [unwired: 4 in, 5 out]
            n653 = Merge Errors(w829) -> (w828:errorcluster)
          }
          frame "Confirm Quit" {
            # "#CodeNeeded - If you want to provide an \"Are you sure\" dialog (or some other notification) before the application exits, place that code here. This message is typically sent from a Panel Close? event."
            # "Confirm Quit - Message that can confirm whether or not the user wants to exit the application."
            n654 = call-poly "Enqueue Message.vi"("Priority Message? (F)"=TRUE, "error in (no error)"=w841, "Message"="Exit", "Message Queue"=w837) -> ("error out"=w838:errorcluster)  [unwired: 6 in, 1 out]
            n655 = Merge Errors(w838) -> (w839:errorcluster)
          }
          frame "Exit" {
            # "Stop the VI"
            # "Release the message queue reference"
            # "#CodeNeeded - Add any required cleanup code here. Note that if 'Exit' was called as a result of an error, an error dialog will be displayed. Add any custom error handling for an 'Exit' condition here as well."
            # "Exit - Exit the application."
            n656 = call "Fire User Event - Stop.vi"("User Event - Stop"=w842) -> ("error out"=w844:errorcluster)  [unwired: 10 in]
            n657 = Release Queue(queue=w849, error in (no error)=w843) -> (error out=w846:errorcluster)  [unwired: 1 in, 2 out]
            n658 = Merge Errors(w844, w846) -> (w845:errorcluster)
          }
          frame Default {
            # "'Default' case only runs if there is a message that isn't defined in any of the other cases.  Output a programming error."
            n659 = xnode "Error Ring"("parameter 0"=w850) -> ("error out"=w851:errorcluster)
          }
        }
        n660 = call "LAB-IQ Error Handler - Message Handling Loop.vi"("error in (no error)"=w798, "Message Queue"=w800) -> ("dup error in"=w799:errorcluster)  [unwired: 8 in, 1 out]
      }
    }
    frame Enabled {
    }
  }
  n661 = disable-structure shown="Disabled" {
    disable-tunnel: w30 -> [w864 _]
    disable-tunnel: w26 -> [w863 _]
    disable-tunnel: w25 -> [w862 _]
    disable-tunnel: w16 -> [w861 _]
    frame Disabled {
      n662 = while {
        shift-right: [w875] -> _
        shift-left: w863 -> [w876]
        tunnel: [w869] -> _
        tunnel: w864 -> [w867]
        tunnel: w861 -> [w866]
        tunnel: w862 -> [w865]
        stop <- w874 stop-if-true
        # "Ramp Motor  Handling Loop"
        n663 = call "Dequeue Message.vi"("error in (no error)"=w866, "Message Queue"=w867) -> ("error out"=w873:errorcluster, "Message Data"=w871:variant, "Message"=w872:string, "dup Message Queue"=w870:refnum<queue>)  [unwired: 6 in]
        n664 = case "Message Cases" shown="\"Ramp Main\"" w872 {
          selector: w872 -> [_ _ _ _ _ w920]
          tunnel: w870 -> [w877 w888 _ w907 w919 _]
          tunnel: w873 -> [w880 w885 w904 w911 w913 _]
          tunnel: [w881 w889 w898 w909 w915 w921] -> w868
          tunnel: w876 -> [w879 w887 w903 w910 w918 w922]
          tunnel: [w879 w887 w903 w910 w918 w922] -> w875
          tunnel: [_ _ _ _ TRUE _] -> w874
          tunnel: w871 -> [_ _ w902 _ _ _]
          tunnel: w865 -> [_ _ _ _ w912 _]
          frame "init" {
            # "Initialize - All initialization work should take place in this message, since other loops can potentially enqueue messages that execute immediately after this one."
            n665 = call-poly "Enqueue Message.vi"("error in (no error)"=w880, "Message"="Ramp Main", "Message Queue"=w877) -> ("error out"=w881:errorcluster)  [unwired: 7 in, 1 out]
          }
          frame "Ramp Main" {
            n666 = Unbundle By Name(w887) -> ("Main Home Screen.EXIT"=w886:refnum<vi>)
            n667 = property class="Bool (strict)"(reference=w886) -> (reference out=w883:refnum<vi>, error out=w884:errorcluster, "Value"=w882:bool)  [unwired: 1 in]
            n668 = case shown="False" w882 {
              tunnel: [w892 w896] -> w889
              tunnel: w888 -> [w891 w895]
              tunnel: w885 -> [w890 w894]
              frame True {
                n669 = call-poly "Enqueue Message.vi"("error in (no error)"=w890, "Message"="Confirm Quit", "Message Queue"=w891) -> ("error out"=w892:errorcluster)  [unwired: 7 in, 1 out]
              }
              frame False {
                n670 = call-poly "Enqueue Message.vi"("error in (no error)"=w894, "Message"="Ramp Main", "Message Queue"=w895) -> ("error out"=w896:errorcluster)  [unwired: 7 in, 1 out]
              }
            }
            n671 = Close Reference(reference=w883, error in (no error)=w884) -> ()  [unwired: 1 out]
          }
          frame "Error" {
            # "#CodeRecommended - If you ever change the name of this \"Error\" message, you'll need to update the name in the Check Loop Error.vi as well."
            # "#CodeRecommended - Consider creating a system for logging errors in some way. These errors are for notification purposes only. Handling of specific errors should be performed in the message frames that generated the error."
            # "Error - Display an error dialog. This message is sent by the \"Error Handler\" VIs at the end of other loops in this application."
            n672 = Variant To Data(error in=w904, type=errorcluster {"status"=FALSE, "code"=0, "source"=""} ("error constant"), Variant=w902) -> (data=w900:errorcluster, error out=w899:errorcluster)
            n673 = call <vilib>:"Simple Error Handler.vi"("error in (no error)"=w900) -> ()  [unwired: 4 in, 5 out]
            n674 = Merge Errors(w899) -> (w898:errorcluster)
          }
          frame "Confirm Quit" {
            # "#CodeNeeded - If you want to provide an \"Are you sure\" dialog (or some other notification) before the application exits, place that code here. This message is typically sent from a Panel Close? event."
            # "Confirm Quit - Message that can confirm whether or not the user wants to exit the application."
            n675 = call-poly "Enqueue Message.vi"("Priority Message? (F)"=TRUE, "error in (no error)"=w911, "Message"="Exit", "Message Queue"=w907) -> ("error out"=w908:errorcluster)  [unwired: 6 in, 1 out]
            n676 = Merge Errors(w908) -> (w909:errorcluster)
          }
          frame "Exit" {
            # "Stop the VI"
            # "Release the message queue reference"
            # "#CodeNeeded - Add any required cleanup code here. Note that if 'Exit' was called as a result of an error, an error dialog will be displayed. Add any custom error handling for an 'Exit' condition here as well."
            # "Exit - Exit the application."
            n677 = call "Fire User Event - Stop.vi"("User Event - Stop"=w912) -> ("error out"=w914:errorcluster)  [unwired: 10 in]
            n678 = Release Queue(queue=w919, error in (no error)=w913) -> (error out=w916:errorcluster)  [unwired: 1 in, 2 out]
            n679 = Merge Errors(w914, w916) -> (w915:errorcluster)
          }
          frame Default {
            # "'Default' case only runs if there is a message that isn't defined in any of the other cases.  Output a programming error."
            n680 = xnode "Error Ring"("parameter 0"=w920) -> ("error out"=w921:errorcluster)
          }
        }
        n681 = call "LAB-IQ Error Handler - Message Handling Loop.vi"("error in (no error)"=w868, "Message Queue"=w870) -> ("dup error in"=w869:errorcluster)  [unwired: 8 in, 1 out]
      }
    }
    frame Enabled {
    }
  }
  n682 = timed-loop {
    shift-right: [w948] -> _
    shift-left: w26 -> [w949]
    tunnel: [w942] -> _
    tunnel: w23 -> [w940]
    tunnel: w16 -> [w939]
    tunnel: w25 -> [w938]
    timing: w3 -> [_]
    timing-out: [_] -> w2
    shift-right: [w936] -> _
    shift-left: w1 -> [w937]
    shift-right: [w934] -> _
    shift-left: w1 -> [w935]
    shift-right: [w932] -> _
    shift-left: w1 -> [w933]
    shift-right: [w931] -> _
    shift-left: w1 -> [w930]
    stop <- w947 stop-if-true
    # "Load Pid  Handling Loop"
    n683 = node-c288() -> ()  [unwired: 1 in, 1 out]
    n684 = call "Dequeue Message.vi"("error in (no error)"=w939, "Message Queue"=w940) -> ("error out"=w946:errorcluster, "Message Data"=w944:variant, "Message"=w945:string, "dup Message Queue"=w943:refnum<queue>)  [unwired: 6 in]
    n685 = case "Message Cases" shown="\"init\"" w945 {
      selector: w945 -> [_ _ _ _ _ w1057]
      tunnel: w943 -> [w956 w985 _ w1036 w1052 _]
      tunnel: w946 -> [w959 w983 w1029 w1040 w1046 _]
      tunnel: [w960 w986 w1023 w1038 w1048 w1058] -> w941
      tunnel: w949 -> [w958 w972 w1028 w1039 w1051 w1059]
      tunnel: [w958 w972 w1028 w1039 w1051 w1059] -> w948
      tunnel: [_ _ _ _ TRUE _] -> w947
      tunnel: w944 -> [_ _ w1027 _ _ _]
      tunnel: w938 -> [_ _ _ _ w1045 _]
      tunnel: w937 -> [w954 w968 w1022 w1033 w1044 w1055]
      tunnel: [w954 w967 w1022 w1033 w1044 w1055] -> w936
      tunnel: w935 -> [w955 w966 w1021 w1032 w1043 w1056]
      tunnel: [w955 w965 w1021 w1032 w1043 w1056] -> w934
      tunnel: w933 -> [w953 w964 w1020 w1031 w1042 w1054]
      tunnel: [w953 w963 w1020 w1031 w1042 w1054] -> w932
      tunnel: w930 -> [_ w962 _ _ _ _]
      tunnel: [w952 w961 w1019 w1030 w1041 w1053] -> w931
      tunnel: w930 -> [w952 _ w1019 w1030 w1041 w1053]
      frame "init" {
        # "Initialize - All initialization work should take place in this message, since other loops can potentially enqueue messages that execute immediately after this one."
        n686 = call-poly "Enqueue Message.vi"("error in (no error)"=w959, "Message"="Load Pid Main", "Message Queue"=w956) -> ("error out"=w960:errorcluster)  [unwired: 7 in, 1 out]
      }
      frame "Load Pid Main" {
        n687 = Unbundle By Name(w972) -> ("Main Screen.Load En"=w978:refnum<vi>)
        n688 = Unbundle By Name(w972) -> ("PID.apply load"=w973:refnum<vi>)
        n689 = property class="Bool (strict)"(reference=w978) -> (reference out=w976:refnum<vi>, error out=w977:errorcluster, "Value"=w971:bool)  [unwired: 1 in]
        n690 = property class="Bool (strict)"(reference=w973) -> (reference out=w975:refnum<vi>, error out=w974:errorcluster, "Value"=w970:bool)  [unwired: 1 in]
        n691 = Close Reference(reference=w976, error in (no error)=w977) -> ()  [unwired: 1 out]
        n692 = Close Reference(reference=w975, error in (no error)=w974) -> ()  [unwired: 1 out]
        n693 = Or(x=w971, y=w970) -> (x .or. y?=w969:bool)
        n694 = case shown="False" w969 {
          tunnel: w983 -> [w993 w1006]
          tunnel: [w993 w1005] -> w979
          tunnel: w972 -> [_ w1004]
          tunnel: w968 -> [w992 w1003]
          tunnel: [w992 w1002] -> w967
          tunnel: w966 -> [w991 w1001]
          tunnel: [w991 w1000] -> w965
          tunnel: w964 -> [w988 w997]
          tunnel: [w988 w996] -> w963
          tunnel: w962 -> [w987 w995]
          tunnel: [w987 w994] -> w961
          frame False {
            n695 = local write "Checkbox 2"(TRUE ("Checkbox 2")) -> ()
            n696 = local write "Checkbox"(TRUE ("Checkbox")) -> ()
          }
          frame True {
            n697 = case shown="True" "Checkbox 2" {
              selector: "Checkbox 2" -> [_ w1009]
              tunnel: [FALSE ("Checkbox") "Checkbox"] -> w999
              frame False {
              }
              frame True {
                n698 = Not(x=w1009) -> (.not. x?=w1008:bool)
                n699 = local write "Checkbox 2"(w1008) -> ()
              }
            }
            n700 = call "NEW LOAD CELL PID.vi"("filtered_load_in"=w997, "filtered_deriv_in"=w995, "integral_out"=w1001, "error in (no error)"=w1006, "prev_error_out"=w1003, "Checkbox"=w999, "main ref"=w1004) -> ("error out"=w1005:errorcluster, "prev_error_out"=w1002:dbl, "integral_out"=w1000:dbl, "filtered_load_out"=w996:dbl, "filtered_deriv_out"=w994:dbl)
          }
        }
        n701 = Unbundle By Name(w972) -> ("Main Home Screen.EXIT"=w984:refnum<vi>)
        n702 = property class="Bool (strict)"(reference=w984) -> (reference out=w981:refnum<vi>, error out=w982:errorcluster, "Value"=w980:bool)  [unwired: 1 in]
        n703 = case shown="False" w980 {
          tunnel: [w1013 w1017] -> w986
          tunnel: w985 -> [w1012 w1016]
          tunnel: w979 -> [w1011 w1015]
          frame True {
            n704 = call-poly "Enqueue Message.vi"("error in (no error)"=w1011, "Message"="Confirm Quit", "Message Queue"=w1012) -> ("error out"=w1013:errorcluster)  [unwired: 7 in, 1 out]
          }
          frame False {
            n705 = call-poly "Enqueue Message.vi"("error in (no error)"=w1015, "Message"="Load Pid Main", "Message Queue"=w1016) -> ("error out"=w1017:errorcluster)  [unwired: 7 in, 1 out]
          }
        }
        n706 = Close Reference(reference=w981, error in (no error)=w982) -> ()  [unwired: 1 out]
      }
      frame "Error" {
        # "#CodeRecommended - If you ever change the name of this \"Error\" message, you'll need to update the name in the Check Loop Error.vi as well."
        # "#CodeRecommended - Consider creating a system for logging errors in some way. These errors are for notification purposes only. Handling of specific errors should be performed in the message frames that generated the error."
        # "Error - Display an error dialog. This message is sent by the \"Error Handler\" VIs at the end of other loops in this application."
        n707 = Variant To Data(error in=w1029, type=errorcluster {"status"=FALSE, "code"=0, "source"=""} ("error constant"), Variant=w1027) -> (data=w1025:errorcluster, error out=w1024:errorcluster)
        n708 = call <vilib>:"Simple Error Handler.vi"("error in (no error)"=w1025) -> ()  [unwired: 4 in, 5 out]
        n709 = Merge Errors(w1024) -> (w1023:errorcluster)
      }
      frame "Confirm Quit" {
        # "#CodeNeeded - If you want to provide an \"Are you sure\" dialog (or some other notification) before the application exits, place that code here. This message is typically sent from a Panel Close? event."
        # "Confirm Quit - Message that can confirm whether or not the user wants to exit the application."
        n710 = call-poly "Enqueue Message.vi"("Priority Message? (F)"=TRUE, "error in (no error)"=w1040, "Message"="Exit", "Message Queue"=w1036) -> ("error out"=w1037:errorcluster)  [unwired: 6 in, 1 out]
        n711 = Merge Errors(w1037) -> (w1038:errorcluster)
      }
      frame "Exit" {
        # "Stop the VI"
        # "Release the message queue reference"
        # "#CodeNeeded - Add any required cleanup code here. Note that if 'Exit' was called as a result of an error, an error dialog will be displayed. Add any custom error handling for an 'Exit' condition here as well."
        # "Exit - Exit the application."
        n712 = call "Fire User Event - Stop.vi"("User Event - Stop"=w1045) -> ("error out"=w1047:errorcluster)  [unwired: 10 in]
        n713 = Release Queue(queue=w1052, error in (no error)=w1046) -> (error out=w1049:errorcluster)  [unwired: 1 in, 2 out]
        n714 = Merge Errors(w1047, w1049) -> (w1048:errorcluster)
      }
      frame Default {
        # "'Default' case only runs if there is a message that isn't defined in any of the other cases.  Output a programming error."
        n715 = xnode "Error Ring"("parameter 0"=w1057) -> ("error out"=w1058:errorcluster)
      }
    }
    n716 = call "LAB-IQ Error Handler - Message Handling Loop.vi"("error in (no error)"=w941, "Message Queue"=w943) -> ("dup error in"=w942:errorcluster)  [unwired: 8 in, 1 out]
    n717 = node-c288() -> ()  [unwired: 1 in, 1 out]
  }
  n718 = disable-structure shown="Disabled" {
    disable-tunnel: w32 -> [w1071 _]
    disable-tunnel: w26 -> [w1070 _]
    disable-tunnel: w25 -> [w1069 _]
    disable-tunnel: w16 -> [w1068 w1137]
    disable-tunnel: [w1067 w1137] -> w13
    frame Disabled {
      n719 = while {
        shift-right: [w1082] -> _
        shift-left: w1070 -> [w1083]
        tunnel: [w1076] -> w1067
        tunnel: w1071 -> [w1074]
        tunnel: w1068 -> [w1073]
        tunnel: w1069 -> [w1072]
        stop <- w1081 stop-if-true
        # "Temperature  Handling Loop"
        n720 = call "Dequeue Message.vi"("error in (no error)"=w1073, "Message Queue"=w1074) -> ("error out"=w1080:errorcluster, "Message Data"=w1078:variant, "Message"=w1079:string, "dup Message Queue"=w1077:refnum<queue>)  [unwired: 6 in]
        n721 = case "Message Cases" shown="\"Temperature Main\"" w1079 {
          selector: w1079 -> [_ _ _ _ _ w1127]
          tunnel: w1077 -> [w1084 w1095 _ w1114 w1126 _]
          tunnel: w1080 -> [w1087 w1092 w1111 w1118 w1120 _]
          tunnel: [w1088 w1096 w1105 w1116 w1122 w1128] -> w1075
          tunnel: w1083 -> [w1086 w1094 w1110 w1117 w1125 w1129]
          tunnel: [w1086 w1094 w1110 w1117 w1125 w1129] -> w1082
          tunnel: [_ _ _ _ TRUE _] -> w1081
          tunnel: w1078 -> [_ _ w1109 _ _ _]
          tunnel: w1072 -> [_ _ _ _ w1119 _]
          frame "init" {
            # "Initialize - All initialization work should take place in this message, since other loops can potentially enqueue messages that execute immediately after this one."
            n722 = call-poly "Enqueue Message.vi"("error in (no error)"=w1087, "Message"="Temperature Main", "Message Queue"=w1084) -> ("error out"=w1088:errorcluster)  [unwired: 7 in, 1 out]
          }
          frame "Temperature Main" {
            n723 = Unbundle By Name(w1094) -> ("Main Home Screen.EXIT"=w1093:refnum<vi>)
            n724 = property class="Bool (strict)"(reference=w1093) -> (reference out=w1090:refnum<vi>, error out=w1091:errorcluster, "Value"=w1089:bool)  [unwired: 1 in]
            n725 = case shown="False" w1089 {
              tunnel: [w1099 w1103] -> w1096
              tunnel: w1095 -> [w1098 w1102]
              tunnel: w1092 -> [w1097 w1101]
              frame True {
                n726 = call-poly "Enqueue Message.vi"("error in (no error)"=w1097, "Message"="Confirm Quit", "Message Queue"=w1098) -> ("error out"=w1099:errorcluster)  [unwired: 7 in, 1 out]
              }
              frame False {
                n727 = call-poly "Enqueue Message.vi"("error in (no error)"=w1101, "Message"="Temperature Main", "Message Queue"=w1102) -> ("error out"=w1103:errorcluster)  [unwired: 7 in, 1 out]
              }
            }
            n728 = Close Reference(reference=w1090, error in (no error)=w1091) -> ()  [unwired: 1 out]
          }
          frame "Error" {
            # "#CodeRecommended - If you ever change the name of this \"Error\" message, you'll need to update the name in the Check Loop Error.vi as well."
            # "#CodeRecommended - Consider creating a system for logging errors in some way. These errors are for notification purposes only. Handling of specific errors should be performed in the message frames that generated the error."
            # "Error - Display an error dialog. This message is sent by the \"Error Handler\" VIs at the end of other loops in this application."
            n729 = Variant To Data(error in=w1111, type=errorcluster {"status"=FALSE, "code"=0, "source"=""} ("error constant"), Variant=w1109) -> (data=w1107:errorcluster, error out=w1106:errorcluster)
            n730 = call <vilib>:"Simple Error Handler.vi"("error in (no error)"=w1107) -> ()  [unwired: 4 in, 5 out]
            n731 = Merge Errors(w1106) -> (w1105:errorcluster)
          }
          frame "Confirm Quit" {
            # "#CodeNeeded - If you want to provide an \"Are you sure\" dialog (or some other notification) before the application exits, place that code here. This message is typically sent from a Panel Close? event."
            # "Confirm Quit - Message that can confirm whether or not the user wants to exit the application."
            n732 = call-poly "Enqueue Message.vi"("Priority Message? (F)"=TRUE, "error in (no error)"=w1118, "Message"="Exit", "Message Queue"=w1114) -> ("error out"=w1115:errorcluster)  [unwired: 6 in, 1 out]
            n733 = Merge Errors(w1115) -> (w1116:errorcluster)
          }
          frame "Exit" {
            # "Stop the VI"
            # "Release the message queue reference"
            # "#CodeNeeded - Add any required cleanup code here. Note that if 'Exit' was called as a result of an error, an error dialog will be displayed. Add any custom error handling for an 'Exit' condition here as well."
            # "Exit - Exit the application."
            n734 = call "Fire User Event - Stop.vi"("User Event - Stop"=w1119) -> ("error out"=w1121:errorcluster)  [unwired: 10 in]
            n735 = Release Queue(queue=w1126, error in (no error)=w1120) -> (error out=w1123:errorcluster)  [unwired: 1 in, 2 out]
            n736 = Merge Errors(w1121, w1123) -> (w1122:errorcluster)
          }
          frame Default {
            # "'Default' case only runs if there is a message that isn't defined in any of the other cases.  Output a programming error."
            n737 = xnode "Error Ring"("parameter 0"=w1127) -> ("error out"=w1128:errorcluster)
          }
        }
        n738 = call "LAB-IQ Error Handler - Message Handling Loop.vi"("error in (no error)"=w1075, "Message Queue"=w1077) -> ("dup error in"=w1076:errorcluster)  [unwired: 8 in, 1 out]
      }
    }
    frame Enabled {
    }
  }
  n739 = while {
    tunnel: w63 -> [w1145]
    shift-right: [w1143] -> w60
    shift-left: w57 -> [w1144]
    tunnel: [w1139] -> w58
    stop <- w1141 stop-if-true
    # "Event Handling Loop"
    n740 = event shown="[1] Timeout" {
      selector: w1144 -> [_ _ _ _ _ _ _ _ _ _ _ _ _ _ _ _ _ _ _ _ _ _ _ _ _ _ _ _ _ _ _ _ _ _ _ _ _ _ _ _ _ _ _ _ _ _ _ _ _ _ _ _ _ _ _ _ _ _ _ _ _ _ _ _ _ _ _ _ _ _ _ _ _]
      dyn-events: [_ _ _ _ _ _ _ _ _ _ _ _ _ _ _ _ _ _ _ _ _ _ _ _ _ _ _ _ _ _ _ _ _ _ _ _ _ _ _ _ _ _ _ _ _ _ _ _ _ _ _ _ _ _ _ _ _ _ _ _ _ _ _ _ _ _ _ _ _ _ _ _ _] -> w1143
      timeout: 100 -> [_ _ _ _ _ _ _ _ _ _ _ _ _ _ _ _ _ _ _ _ _ _ _ _ _ _ _ _ _ _ _ _ _ _ _ _ _ _ _ _ _ _ _ _ _ _ _ _ _ _ _ _ _ _ _ _ _ _ _ _ _ _ _ _ _ _ _ _ _ _ _ _ _]
      tunnel: [_ _ _ _ _ _ _ _ _ _ _ _ _ _ _ _ _ _ _ _ _ _ _ _ _ _ _ _ _ _ _ _ _ _ _ _ _ _ _ _ _ _ _ _ _ _ _ _ _ _ _ _ _ _ _ _ _ _ _ _ _ _ _ _ _ _ _ _ _ _ _ _ TRUE ("Discard?")] -> w1141
      tunnel: w1145 -> [w1150 w1156 w1159 w1164 w1169 w1174 w1179 w1184 w1189 w1194 w1199 w1204 w1209 w1214 w1219 w1224 w1229 w1234 w1239 w1244 w1249 w1254 w1259 w1264 w1269 w1274 w1279 w1284 w1289 w1294 w1299 w1304 w1309 w1314 w1319 w1324 w1329 w1334 w1339 w1344 w1349 w1354 w1359 w1364 w1369 w1374 w1379 w1384 w1389 w1394 w1399 w1404 w1409 w1414 w1419 w1424 w1429 w1434 w1439 w1444 w1449 w1454 w1459 w1464 w1469 w1474 w1479 w1484 w1489 w1494 w1497 w1502 w1504]
      tunnel: [w1149 w1155 w1157 w1162 w1167 w1172 w1177 w1182 w1187 w1192 w1197 w1202 w1207 w1212 w1217 w1222 w1227 w1232 w1237 w1242 w1247 w1252 w1257 w1262 w1267 w1272 w1277 w1282 w1287 w1292 w1297 w1302 w1307 w1312 w1317 w1322 w1327 w1332 w1337 w1342 w1347 w1352 w1357 w1362 w1367 w1372 w1377 w1382 w1387 w1392 w1397 w1402 w1407 w1412 w1417 w1422 w1427 w1432 w1437 w1442 w1447 w1452 w1457 w1462 w1467 w1472 w1477 w1482 w1487 w1492 _ w1501 _] -> w1142
      tunnel: [w1148 w1154 w1158 w1163 w1168 w1173 w1178 w1183 w1188 w1193 w1198 w1203 w1208 w1213 w1218 w1223 w1228 w1233 w1238 w1243 w1248 w1253 w1258 w1263 w1268 w1273 w1278 w1283 w1288 w1293 w1298 w1303 w1308 w1313 w1318 w1323 w1328 w1333 w1338 w1343 w1348 w1353 w1358 w1363 w1368 w1373 w1378 w1383 w1388 w1393 w1398 w1403 w1408 w1413 w1418 w1423 w1428 w1433 w1438 w1443 w1448 w1453 w1458 w1463 w1468 w1473 w1478 w1483 w1488 w1493 w1497 w1500 w1504] -> w1140
      event Panel Close? {
        n741 = event-data() -> ()  [unwired: 1 in, 1 out]
        n742 = call-poly "Enqueue Message.vi"("Priority Message? (F)"=TRUE, "Message"="Confirm Quit", "Message Queue"=w1150) -> ("error out"=w1149:errorcluster, "dup Message Queue"=w1148:refnum<queue>)  [unwired: 7 in]
        n743 = event-data("Discard?"=TRUE) -> ()  [unwired: 1 in, 1 out]
      }
      event Timeout {
        n744 = event-data() -> ()  [unwired: 1 in, 1 out]
        n745 = call-poly "Enqueue Message.vi"("Priority Message? (F)"=TRUE, "Message"="Timeout", "Message Queue"=w1156) -> ("error out"=w1155:errorcluster, "dup Message Queue"=w1154:refnum<queue>)  [unwired: 7 in]
      }
      event "SAVE  2": Value Change {
        n746 = event-data() -> ()  [unwired: 1 in, 1 out]
        n747 = call-poly "Enqueue Message.vi"("Priority Message? (F)"=TRUE, "Message"="Service Save", "Message Queue"=w1159) -> ("error out"=w1157:errorcluster, "dup Message Queue"=w1158:refnum<queue>)  [unwired: 7 in]
      }
      event "Home": Value Change {
        n748 = event-data() -> ()  [unwired: 1 in, 1 out]
        n749 = call-poly "Enqueue Message.vi"("Priority Message? (F)"=TRUE, "Message"="HOME", "Message Queue"=w1164) -> ("error out"=w1162:errorcluster, "dup Message Queue"=w1163:refnum<queue>)  [unwired: 7 in]
      }
      event "Platform Settings": Value Change {
        n750 = event-data() -> ()  [unwired: 1 in, 1 out]
        n751 = call-poly "Enqueue Message.vi"("Priority Message? (F)"=TRUE, "Message"="Platform Setting", "Message Queue"=w1169) -> ("error out"=w1167:errorcluster, "dup Message Queue"=w1168:refnum<queue>)  [unwired: 7 in]
      }
      event "Configure": Value Change {
        n752 = event-data() -> ()  [unwired: 1 in, 1 out]
        n753 = call-poly "Enqueue Message.vi"("Priority Message? (F)"=TRUE, "Message"="Configure", "Message Queue"=w1174) -> ("error out"=w1172:errorcluster, "dup Message Queue"=w1173:refnum<queue>)  [unwired: 7 in]
      }
      event "Analysis": Value Change {
        n754 = event-data() -> ()  [unwired: 1 in, 1 out]
        n755 = call-poly "Enqueue Message.vi"("Priority Message? (F)"=TRUE, "Message"="Analysis", "Message Queue"=w1179) -> ("error out"=w1177:errorcluster, "dup Message Queue"=w1178:refnum<queue>)  [unwired: 7 in]
      }
      event "service 2": Value Change {
        n756 = event-data() -> ()  [unwired: 1 in, 1 out]
        n757 = call-poly "Enqueue Message.vi"("Priority Message? (F)"=TRUE, "Message"="service 2", "Message Queue"=w1184) -> ("error out"=w1182:errorcluster, "dup Message Queue"=w1183:refnum<queue>)  [unwired: 7 in]
      }
      event "Auto": Value Change {
        n758 = event-data() -> ()  [unwired: 1 in, 1 out]
        n759 = call-poly "Enqueue Message.vi"("Priority Message? (F)"=TRUE, "Message"="Auto", "Message Queue"=w1189) -> ("error out"=w1187:errorcluster, "dup Message Queue"=w1188:refnum<queue>)  [unwired: 7 in]
      }
      event "Select Load Head": Value Change {
        n760 = event-data() -> ()  [unwired: 1 in, 1 out]
        n761 = call-poly "Enqueue Message.vi"("Priority Message? (F)"=TRUE, "Message"="Select Load Head", "Message Queue"=w1194) -> ("error out"=w1192:errorcluster, "dup Message Queue"=w1193:refnum<queue>)  [unwired: 7 in]
      }
      event "com 3": Value Change {
        n762 = event-data() -> ()  [unwired: 1 in, 1 out]
        n763 = call-poly "Enqueue Message.vi"("Priority Message? (F)"=TRUE, "Message"="com 3", "Message Queue"=w1199) -> ("error out"=w1197:errorcluster, "dup Message Queue"=w1198:refnum<queue>)  [unwired: 7 in]
      }
      event "Loading Mode": Value Change {
        n764 = event-data() -> ()  [unwired: 1 in, 1 out]
        n765 = call-poly "Enqueue Message.vi"("Priority Message? (F)"=TRUE, "Message"="Loading Mode", "Message Queue"=w1204) -> ("error out"=w1202:errorcluster, "dup Message Queue"=w1203:refnum<queue>)  [unwired: 7 in]
      }
      event "SSP 0.3": Value Change {
        n766 = event-data() -> ()  [unwired: 1 in, 1 out]
        n767 = call-poly "Enqueue Message.vi"("Priority Message? (F)"=TRUE, "Message"="SSP 0.3", "Message Queue"=w1209) -> ("error out"=w1207:errorcluster, "dup Message Queue"=w1208:refnum<queue>)  [unwired: 7 in]
      }
      event "SSP 0.5": Value Change {
        n768 = event-data() -> ()  [unwired: 1 in, 1 out]
        n769 = call-poly "Enqueue Message.vi"("Priority Message? (F)"=TRUE, "Message"="SSP 0.5", "Message Queue"=w1214) -> ("error out"=w1212:errorcluster, "dup Message Queue"=w1213:refnum<queue>)  [unwired: 7 in]
      }
      event "SSP 0.75": Value Change {
        n770 = event-data() -> ()  [unwired: 1 in, 1 out]
        n771 = call-poly "Enqueue Message.vi"("Priority Message? (F)"=TRUE, "Message"="SSP 0.75", "Message Queue"=w1219) -> ("error out"=w1217:errorcluster, "dup Message Queue"=w1218:refnum<queue>)  [unwired: 7 in]
      }
      event "LHBack": Value Change {
        n772 = event-data() -> ()  [unwired: 1 in, 1 out]
        n773 = call-poly "Enqueue Message.vi"("Priority Message? (F)"=TRUE, "Message"="LHBack", "Message Queue"=w1224) -> ("error out"=w1222:errorcluster, "dup Message Queue"=w1223:refnum<queue>)  [unwired: 7 in]
      }
      event "LHNext": Value Change {
        n774 = event-data() -> ()  [unwired: 1 in, 1 out]
        n775 = call-poly "Enqueue Message.vi"("Priority Message? (F)"=TRUE, "Message"="LHNext", "Message Queue"=w1229) -> ("error out"=w1227:errorcluster, "dup Message Queue"=w1228:refnum<queue>)  [unwired: 7 in]
      }
      event "Rot Ver": Value Change {
        n776 = event-data() -> ()  [unwired: 1 in, 1 out]
        n777 = call-poly "Enqueue Message.vi"("Priority Message? (F)"=TRUE, "Message"="Rot Ver", "Message Queue"=w1234) -> ("error out"=w1232:errorcluster, "dup Message Queue"=w1233:refnum<queue>)  [unwired: 7 in]
      }
      event "Scratch": Value Change {
        n778 = event-data() -> ()  [unwired: 1 in, 1 out]
        n779 = call-poly "Enqueue Message.vi"("Priority Message? (F)"=TRUE, "Message"="Scratch", "Message Queue"=w1239) -> ("error out"=w1237:errorcluster, "dup Message Queue"=w1238:refnum<queue>)  [unwired: 7 in]
      }
      event "Motion Mode:": Value Change {
        n780 = event-data() -> ()  [unwired: 1 in, 1 out]
        n781 = call-poly "Enqueue Message.vi"("Priority Message? (F)"=TRUE, "Message"="Motion Mode:", "Message Queue"=w1244) -> ("error out"=w1242:errorcluster, "dup Message Queue"=w1243:refnum<queue>)  [unwired: 7 in]
      }
      event "MMBack": Value Change {
        n782 = event-data() -> ()  [unwired: 1 in, 1 out]
        n783 = call-poly "Enqueue Message.vi"("Priority Message? (F)"=TRUE, "Message"="MMBack", "Message Queue"=w1249) -> ("error out"=w1247:errorcluster, "dup Message Queue"=w1248:refnum<queue>)  [unwired: 7 in]
      }
      event "MMNext": Value Change {
        n784 = event-data() -> ()  [unwired: 1 in, 1 out]
        n785 = call-poly "Enqueue Message.vi"("Priority Message? (F)"=TRUE, "Message"="MMNext", "Message Queue"=w1254) -> ("error out"=w1252:errorcluster, "dup Message Queue"=w1253:refnum<queue>)  [unwired: 7 in]
      }
      event "APBack": Value Change {
        n786 = event-data() -> ()  [unwired: 1 in, 1 out]
        n787 = call-poly "Enqueue Message.vi"("Priority Message? (F)"=TRUE, "Message"="APBack", "Message Queue"=w1259) -> ("error out"=w1257:errorcluster, "dup Message Queue"=w1258:refnum<queue>)  [unwired: 7 in]
      }
      event "SNext": Value Change {
        n788 = event-data() -> ()  [unwired: 1 in, 1 out]
        n789 = call-poly "Enqueue Message.vi"("Priority Message? (F)"=TRUE, "Message"="SNext", "Message Queue"=w1264) -> ("error out"=w1262:errorcluster, "dup Message Queue"=w1263:refnum<queue>)  [unwired: 7 in]
      }
      event "ZeroAll": Value Change {
        n790 = event-data() -> ()  [unwired: 1 in, 1 out]
        n791 = call-poly "Enqueue Message.vi"("Priority Message? (F)"=TRUE, "Message"="ZeroAll", "Message Queue"=w1269) -> ("error out"=w1267:errorcluster, "dup Message Queue"=w1268:refnum<queue>)  [unwired: 7 in]
      }
      event "Enable Platform": Value Change {
        n792 = event-data() -> ()  [unwired: 1 in, 1 out]
        n793 = call-poly "Enqueue Message.vi"("Priority Message? (F)"=TRUE, "Message"="Enable Platform", "Message Queue"=w1274) -> ("error out"=w1272:errorcluster, "dup Message Queue"=w1273:refnum<queue>)  [unwired: 7 in]
      }
      event "Heave Up main": Value Change {
        n794 = event-data() -> ()  [unwired: 1 in, 1 out]
        n795 = call-poly "Enqueue Message.vi"("Priority Message? (F)"=TRUE, "Message"="Heave Up main", "Message Queue"=w1279) -> ("error out"=w1277:errorcluster, "dup Message Queue"=w1278:refnum<queue>)  [unwired: 7 in]
      }
      event "Heave Up MM": Value Change {
        n796 = event-data() -> ()  [unwired: 1 in, 1 out]
        n797 = call-poly "Enqueue Message.vi"("Priority Message? (F)"=TRUE, "Message"="Heave Up MM", "Message Queue"=w1284) -> ("error out"=w1282:errorcluster, "dup Message Queue"=w1283:refnum<queue>)  [unwired: 7 in]
      }
      event "Heave Down Main": Value Change {
        n798 = event-data() -> ()  [unwired: 1 in, 1 out]
        n799 = call-poly "Enqueue Message.vi"("Priority Message? (F)"=TRUE, "Message"="Heave Down Main", "Message Queue"=w1289) -> ("error out"=w1287:errorcluster, "dup Message Queue"=w1288:refnum<queue>)  [unwired: 7 in]
      }
      event "Heave Down MM": Value Change {
        n800 = event-data() -> ()  [unwired: 1 in, 1 out]
        n801 = call-poly "Enqueue Message.vi"("Priority Message? (F)"=TRUE, "Message"="Heave Down MM", "Message Queue"=w1294) -> ("error out"=w1292:errorcluster, "dup Message Queue"=w1293:refnum<queue>)  [unwired: 7 in]
      }
      event "Manual Write Heave & Surge": Value Change {
        n802 = event-data() -> ()  [unwired: 1 in, 1 out]
        n803 = call-poly "Enqueue Message.vi"("Priority Message? (F)"=TRUE, "Message"="Manual Write Heave & Surge", "Message Queue"=w1299) -> ("error out"=w1297:errorcluster, "dup Message Queue"=w1298:refnum<queue>)  [unwired: 7 in]
      }
      event "Manual Write SWAY": Value Change {
        n804 = event-data() -> ()  [unwired: 1 in, 1 out]
        n805 = call-poly "Enqueue Message.vi"("Priority Message? (F)"=TRUE, "Message"="Manual Write SWAY", "Message Queue"=w1304) -> ("error out"=w1302:errorcluster, "dup Message Queue"=w1303:refnum<queue>)  [unwired: 7 in]
      }
      event "Surge Backward Main": Value Change {
        n806 = event-data() -> ()  [unwired: 1 in, 1 out]
        n807 = call-poly "Enqueue Message.vi"("Priority Message? (F)"=TRUE, "Message"="Surge Backward Main", "Message Queue"=w1309) -> ("error out"=w1307:errorcluster, "dup Message Queue"=w1308:refnum<queue>)  [unwired: 7 in]
      }
      event "Surge Backward MM": Value Change {
        n808 = event-data() -> ()  [unwired: 1 in, 1 out]
        n809 = call-poly "Enqueue Message.vi"("Priority Message? (F)"=TRUE, "Message"="Surge Backward MM", "Message Queue"=w1314) -> ("error out"=w1312:errorcluster, "dup Message Queue"=w1313:refnum<queue>)  [unwired: 7 in]
      }
      event "Surge Forward Main": Value Change {
        n810 = event-data() -> ()  [unwired: 1 in, 1 out]
        n811 = call-poly "Enqueue Message.vi"("Priority Message? (F)"=TRUE, "Message"="Surge Forward Main", "Message Queue"=w1319) -> ("error out"=w1317:errorcluster, "dup Message Queue"=w1318:refnum<queue>)  [unwired: 7 in]
      }
      event "Surge Forward MM": Value Change {
        n812 = event-data() -> ()  [unwired: 1 in, 1 out]
        n813 = call-poly "Enqueue Message.vi"("Priority Message? (F)"=TRUE, "Message"="Surge Forward MM", "Message Queue"=w1324) -> ("error out"=w1322:errorcluster, "dup Message Queue"=w1323:refnum<queue>)  [unwired: 7 in]
      }
      event "Sway Left Main": Value Change {
        n814 = event-data() -> ()  [unwired: 1 in, 1 out]
        n815 = call-poly "Enqueue Message.vi"("Priority Message? (F)"=TRUE, "Message"="Sway Left Main", "Message Queue"=w1329) -> ("error out"=w1327:errorcluster, "dup Message Queue"=w1328:refnum<queue>)  [unwired: 7 in]
      }
      event "Sway Left MM": Value Change {
        n816 = event-data() -> ()  [unwired: 1 in, 1 out]
        n817 = call-poly "Enqueue Message.vi"("Priority Message? (F)"=TRUE, "Message"="Sway Left MM", "Message Queue"=w1334) -> ("error out"=w1332:errorcluster, "dup Message Queue"=w1333:refnum<queue>)  [unwired: 7 in]
      }
      event "Sway Right MM": Value Change {
        n818 = event-data() -> ()  [unwired: 1 in, 1 out]
        n819 = call-poly "Enqueue Message.vi"("Priority Message? (F)"=TRUE, "Message"="Sway Right MM", "Message Queue"=w1339) -> ("error out"=w1337:errorcluster, "dup Message Queue"=w1338:refnum<queue>)  [unwired: 7 in]
      }
      event "Sway Right Main": Value Change {
        n820 = event-data() -> ()  [unwired: 1 in, 1 out]
        n821 = call-poly "Enqueue Message.vi"("Priority Message? (F)"=TRUE, "Message"="Sway Right Main", "Message Queue"=w1344) -> ("error out"=w1342:errorcluster, "dup Message Queue"=w1343:refnum<queue>)  [unwired: 7 in]
      }
      event "Load En": Value Change {
        n822 = event-data() -> ()  [unwired: 1 in, 1 out]
        n823 = call-poly "Enqueue Message.vi"("Priority Message? (F)"=TRUE, "Message"="Load En", "Message Queue"=w1349) -> ("error out"=w1347:errorcluster, "dup Message Queue"=w1348:refnum<queue>)  [unwired: 7 in]
      }
      event "apply load": Value Change {
        n824 = event-data() -> ()  [unwired: 1 in, 1 out]
        n825 = call-poly "Enqueue Message.vi"("Priority Message? (F)"=TRUE, "Message"="apply load", "Message Queue"=w1354) -> ("error out"=w1352:errorcluster, "dup Message Queue"=w1353:refnum<queue>)  [unwired: 7 in]
      }
      event "BACK": Value Change {
        n826 = event-data() -> ()  [unwired: 1 in, 1 out]
        n827 = call-poly "Enqueue Message.vi"("Priority Message? (F)"=TRUE, "Message"="BACK", "Message Queue"=w1359) -> ("error out"=w1357:errorcluster, "dup Message Queue"=w1358:refnum<queue>)  [unwired: 7 in]
      }
      event "Start Test": Value Change {
        n828 = event-data() -> ()  [unwired: 1 in, 1 out]
        n829 = call-poly "Enqueue Message.vi"("Priority Message? (F)"=TRUE, "Message"="Start Test", "Message Queue"=w1364) -> ("error out"=w1362:errorcluster, "dup Message Queue"=w1363:refnum<queue>)  [unwired: 7 in]
      }
      event "STOP": Value Change {
        n830 = event-data() -> ()  [unwired: 1 in, 1 out]
        n831 = call-poly "Enqueue Message.vi"("Priority Message? (F)"=TRUE, "Message"="STOP", "Message Queue"=w1369) -> ("error out"=w1367:errorcluster, "dup Message Queue"=w1368:refnum<queue>)  [unwired: 7 in]
      }
      event "PlaceModule": Value Change {
        n832 = event-data() -> ()  [unwired: 1 in, 1 out]
        n833 = call-poly "Enqueue Message.vi"("Priority Message? (F)"=TRUE, "Message"="PlaceModule", "Message Queue"=w1374) -> ("error out"=w1372:errorcluster, "dup Message Queue"=w1373:refnum<queue>)  [unwired: 7 in]
      }
      event "HomeRot", "HomeScratch", "HomeScratch": Value Change {
        n834 = event-data() -> ()  [unwired: 1 in, 1 out]
        n835 = call-poly "Enqueue Message.vi"("Priority Message? (F)"=TRUE, "Message"="Stage Homing", "Message Queue"=w1379) -> ("error out"=w1377:errorcluster, "dup Message Queue"=w1378:refnum<queue>)  [unwired: 7 in]
      }
      event "Clear 3": Value Change {
        n836 = event-data() -> ()  [unwired: 1 in, 1 out]
        n837 = call-poly "Enqueue Message.vi"("Priority Message? (F)"=TRUE, "Message"="Clear 3", "Message Queue"=w1384) -> ("error out"=w1382:errorcluster, "dup Message Queue"=w1383:refnum<queue>)  [unwired: 7 in]
      }
      event "Set WTD": Value Change {
        n838 = event-data() -> ()  [unwired: 1 in, 1 out]
        n839 = call-poly "Enqueue Message.vi"("Priority Message? (F)"=TRUE, "Message"="Set WTD", "Message Queue"=w1389) -> ("error out"=w1387:errorcluster, "dup Message Queue"=w1388:refnum<queue>)  [unwired: 7 in]
      }
      event "Import 2": Value Change {
        n840 = event-data() -> ()  [unwired: 1 in, 1 out]
        n841 = call-poly "Enqueue Message.vi"("Priority Message? (F)"=TRUE, "Message"="Import 2", "Message Queue"=w1394) -> ("error out"=w1392:errorcluster, "dup Message Queue"=w1393:refnum<queue>)  [unwired: 7 in]
      }
      event "Save 2": Value Change {
        n842 = event-data() -> ()  [unwired: 1 in, 1 out]
        n843 = call-poly "Enqueue Message.vi"("Priority Message? (F)"=TRUE, "Message"="Save 2", "Message Queue"=w1399) -> ("error out"=w1397:errorcluster, "dup Message Queue"=w1398:refnum<queue>)  [unwired: 7 in]
      }
      event "calculate rotary": Value Change {
        n844 = event-data() -> ()  [unwired: 1 in, 1 out]
        n845 = call-poly "Enqueue Message.vi"("Priority Message? (F)"=TRUE, "Message"="Calculate Rotary", "Message Queue"=w1404) -> ("error out"=w1402:errorcluster, "dup Message Queue"=w1403:refnum<queue>)  [unwired: 7 in]
      }
      event "Clear List": Value Change {
        n846 = event-data() -> ()  [unwired: 1 in, 1 out]
        n847 = call-poly "Enqueue Message.vi"("Priority Message? (F)"=TRUE, "Message"="Clear List", "Message Queue"=w1409) -> ("error out"=w1407:errorcluster, "dup Message Queue"=w1408:refnum<queue>)  [unwired: 7 in]
      }
      event "Add to list": Value Change {
        n848 = event-data() -> ()  [unwired: 1 in, 1 out]
        n849 = call-poly "Enqueue Message.vi"("Priority Message? (F)"=TRUE, "Message"="Add to list", "Message Queue"=w1414) -> ("error out"=w1412:errorcluster, "dup Message Queue"=w1413:refnum<queue>)  [unwired: 7 in]
      }
      event "ClrLog": Value Change {
        n850 = event-data() -> ()  [unwired: 1 in, 1 out]
        n851 = call-poly "Enqueue Message.vi"("Priority Message? (F)"=TRUE, "Message"="ClrLog", "Message Queue"=w1419) -> ("error out"=w1417:errorcluster, "dup Message Queue"=w1418:refnum<queue>)  [unwired: 7 in]
      }
      event "Disable Axis Jog Soft Limits m": Value Change {
        n852 = event-data() -> ()  [unwired: 1 in, 1 out]
        n853 = call-poly "Enqueue Message.vi"("Priority Message? (F)"=TRUE, "Message"="Disable Axis Jog Soft Limits", "Message Queue"=w1424) -> ("error out"=w1422:errorcluster, "dup Message Queue"=w1423:refnum<queue>)  [unwired: 7 in]
      }
      event "Home Service": Value Change {
        n854 = event-data() -> ()  [unwired: 1 in, 1 out]
        n855 = call-poly "Enqueue Message.vi"("Priority Message? (F)"=TRUE, "Message"="Home Service", "Message Queue"=w1429) -> ("error out"=w1427:errorcluster, "dup Message Queue"=w1428:refnum<queue>)  [unwired: 7 in]
      }
      event "Edit Gain Constants": Value Change {
        n856 = event-data() -> ()  [unwired: 1 in, 1 out]
        n857 = call-poly "Enqueue Message.vi"("Priority Message? (F)"=TRUE, "Message"="Edit Gain Constants", "Message Queue"=w1434) -> ("error out"=w1432:errorcluster, "dup Message Queue"=w1433:refnum<queue>)  [unwired: 7 in]
      }
      event "Advanced Setting": Value Change {
        n858 = event-data() -> ()  [unwired: 1 in, 1 out]
        n859 = call-poly "Enqueue Message.vi"("Priority Message? (F)"=TRUE, "Message"="Advanced Setting", "Message Queue"=w1439) -> ("error out"=w1437:errorcluster, "dup Message Queue"=w1438:refnum<queue>)  [unwired: 7 in]
      }
      event "Password": Value Change {
        n860 = event-data() -> ()  [unwired: 1 in, 1 out]
        n861 = call-poly "Enqueue Message.vi"("Priority Message? (F)"=TRUE, "Message"="Password", "Message Queue"=w1444) -> ("error out"=w1442:errorcluster, "dup Message Queue"=w1443:refnum<queue>)  [unwired: 7 in]
      }
      event "Service About": Value Change {
        n862 = event-data() -> ()  [unwired: 1 in, 1 out]
        n863 = call-poly "Enqueue Message.vi"("Priority Message? (F)"=TRUE, "Message"="Service About", "Message Queue"=w1449) -> ("error out"=w1447:errorcluster, "dup Message Queue"=w1448:refnum<queue>)  [unwired: 7 in]
      }
      event "OPEN 1": Value Change {
        n864 = event-data() -> ()  [unwired: 1 in, 1 out]
        n865 = call-poly "Enqueue Message.vi"("Priority Message? (F)"=TRUE, "Message"="OPEN 1", "Message Queue"=w1454) -> ("error out"=w1452:errorcluster, "dup Message Queue"=w1453:refnum<queue>)  [unwired: 7 in]
      }
      event "OPEN 2": Value Change {
        n866 = event-data() -> ()  [unwired: 1 in, 1 out]
        n867 = call-poly "Enqueue Message.vi"("Priority Message? (F)"=TRUE, "Message"="OPEN 2", "Message Queue"=w1459) -> ("error out"=w1457:errorcluster, "dup Message Queue"=w1458:refnum<queue>)  [unwired: 7 in]
      }
      event "OPEN 3": Value Change {
        n868 = event-data() -> ()  [unwired: 1 in, 1 out]
        n869 = call-poly "Enqueue Message.vi"("Priority Message? (F)"=TRUE, "Message"="OPEN 3", "Message Queue"=w1464) -> ("error out"=w1462:errorcluster, "dup Message Queue"=w1463:refnum<queue>)  [unwired: 7 in]
      }
      event "OPEN 4": Value Change {
        n870 = event-data() -> ()  [unwired: 1 in, 1 out]
        n871 = call-poly "Enqueue Message.vi"("Priority Message? (F)"=TRUE, "Message"="OPEN 4", "Message Queue"=w1469) -> ("error out"=w1467:errorcluster, "dup Message Queue"=w1468:refnum<queue>)  [unwired: 7 in]
      }
      event "Refresh 2": Value Change {
        n872 = event-data() -> ()  [unwired: 1 in, 1 out]
        n873 = call-poly "Enqueue Message.vi"("Priority Message? (F)"=TRUE, "Message"="Refresh 2", "Message Queue"=w1474) -> ("error out"=w1472:errorcluster, "dup Message Queue"=w1473:refnum<queue>)  [unwired: 7 in]
      }
      event "Analysis Home new": Value Change {
        n874 = event-data() -> ()  [unwired: 1 in, 1 out]
        n875 = call-poly "Enqueue Message.vi"("Priority Message? (F)"=TRUE, "Message"="Analysis Home", "Message Queue"=w1479) -> ("error out"=w1477:errorcluster, "dup Message Queue"=w1478:refnum<queue>)  [unwired: 7 in]
      }
      event "Post Analysis": Value Change {
        n876 = event-data() -> ()  [unwired: 1 in, 1 out]
        n877 = call-poly "Enqueue Message.vi"("Priority Message? (F)"=TRUE, "Message"="Post Analysis", "Message Queue"=w1484) -> ("error out"=w1482:errorcluster, "dup Message Queue"=w1483:refnum<queue>)  [unwired: 7 in]
      }
      event "Scratch Mode": Value Change {
        n878 = event-data() -> ()  [unwired: 1 in, 1 out]
        n879 = call-poly "Enqueue Message.vi"("Priority Message? (F)"=TRUE, "Message"="Scratch Mode", "Message Queue"=w1489) -> ("error out"=w1487:errorcluster, "dup Message Queue"=w1488:refnum<queue>)  [unwired: 7 in]
      }
      event "Export": Value Change {
        n880 = event-data() -> ()  [unwired: 1 in, 1 out]
        n881 = call-poly "Enqueue Message.vi"("Priority Message? (F)"=TRUE, "Message"="Export", "Message Queue"=w1494) -> ("error out"=w1492:errorcluster, "dup Message Queue"=w1493:refnum<queue>)  [unwired: 7 in]
      }
      event Application Instance Close {
        # "#CodeRecommended - When a project closes, all VIs within that project are aborted and leave memory. However, any code placed in this event frame is guaranteed to run to completion, so add any cleanup code that absolutely must happen here."
        n882 = event-data() -> ()  [unwired: 1 in, 1 out]
      }
      event "EXIT": Value Change {
        n883 = event-data() -> ()  [unwired: 1 in, 1 out]
        n884 = call-poly "Enqueue Message.vi"("Priority Message? (F)"=TRUE, "Message"="Exit", "Message Queue"=w1502) -> ("error out"=w1501:errorcluster, "dup Message Queue"=w1500:refnum<queue>)  [unwired: 7 in]
      }
      event User Event {
        # "The Message Handling Loop processed an \"Exit\" message, which fired this event to stop the Event Handling Loop."
        n885 = event-data() -> ()  [unwired: 1 in, 1 out]
      }
    }
    n886 = call "LAB-IQ Error Handler - Event Handling Loop.vi"("error in (no error)"=w1142, "Message Queue"=w1140) -> ("dup error in"=w1139:errorcluster)  [unwired: 8 in, 1 out]
  }
  n887 = while {
    tunnel: w63 -> [w1508]
    shift-right: [w1515] -> _
    shift-left: w26 -> [w1516]
    tunnel: w25 -> [w1513]
    tunnel: w56 -> [w1512]
    tunnel: [w1506] -> w64
    stop <- w1514 stop-if-true
    # "Message Handling Loop"
    n888 = call "Dequeue Message.vi"("error in (no error)"=w1512, "Message Queue"=w1508) -> ("error out"=w1511:errorcluster, "Message Data"=w1509:variant, "Message"=w1510:string, "dup Message Queue"=w1507:refnum<queue>)  [unwired: 6 in]
    n889 = case "Message Cases" shown="\"Surge Forward MM\"" w1510 {
      selector: w1510 -> [_ _ _ _ _ _ _ _ _ _ _ _ _ _ _ _ _ _ _ _ _ _ _ _ _ _ _ _ _ _ _ _ _ _ _ _ _ _ _ _ _ _ _ _ _ _ _ _ _ _ _ _ _ _ _ _ _ _ _ _ _ _ _ _ _ _ _ _ _ _ _ _ _ _ w2812]
      tunnel: w1507 -> [_ w1561 _ _ _ _ _ _ _ _ _ _ _ _ _ _ _ _ _ _ _ _ _ _ _ _ _ _ _ _ _ _ _ _ _ _ _ _ _ _ _ _ _ _ _ _ _ _ _ _ _ _ _ _ _ _ _ _ _ _ _ _ _ _ _ _ _ _ _ _ _ _ w2800 w2811 _]
      tunnel: w1511 -> [w1519 w1563 w1565 w1569 w1590 w1607 w1624 w1641 w1662 w1675 w1680 w1684 w1691 w1696 w1761 w1787 w1813 w1848 w1864 w1916 w1920 w1923 w1930 w1973 w1985 w2014 w2044 w2063 w2074 w2085 w2096 w2107 w2118 w2129 w2140 w2152 w2163 w2174 w2185 w2194 w2205 w2216 w2246 w2287 w2293 w2309 w2313 w2316 w2324 w2336 w2345 w2365 w2379 w2389 w2399 w2401 w2416 w2429 w2446 w2463 w2499 w2507 w2566 w2590 w2600 w2641 w2684 w2727 w2763 w2770 w2789 w2796 w2803 w2804 _]
      tunnel: [w1518 w1530 w1565 w1570 w1585 w1602 w1619 w1636 w1657 w1667 w1678 w1682 w1689 w1700 w1757 w1783 w1809 w1849 w1865 w1880 w1919 w1922 w1929 w1972 w1984 w2013 w2031 w2065 w2076 w2087 w2098 w2109 w2120 w2131 w2142 w2153 w2164 w2175 w2186 w2196 w2206 w2215 w2245 w2266 w2292 w2310 w2312 w2315 w2323 w2330 w2340 w2358 w2378 w2389 w2399 w2407 w2415 w2428 w2445 w2462 w2498 w2506 w2566 w2590 w2597 w2638 w2681 w2724 w2764 w2770 w2783 w2790 w2802 w2807 w2813] -> w1505
      tunnel: w1516 -> [w1517 w1521 w1566 w1568 w1576 w1593 w1610 w1627 w1645 w1665 w1677 w1681 w1687 w1695 w1759 w1785 w1811 w1836 w1851 w1867 w1918 w1921 w1924 w1967 w1983 w1996 w2026 w2061 w2072 w2083 w2094 w2105 w2116 w2127 w2138 w2150 w2161 w2172 w2183 w2193 w2204 w2214 w2244 w2265 w2291 w2295 w2311 w2314 w2318 w2329 w2338 w2360 w2377 w2381 w2391 w2400 w2414 w2418 w2431 w2449 w2465 w2501 w2558 w2581 w2593 w2634 w2677 w2720 w2762 w2765 w2782 w2795 w2797 w2810 w2814]
      tunnel: [w1517 w1521 w1566 w1568 w1576 w1593 w1610 w1627 w1645 w1665 w1677 w1681 w1687 w1695 w1759 w1785 w1811 w1836 w1851 w1867 w1918 w1921 w1924 w1967 w1983 w1996 w2026 w2061 w2072 w2083 w2094 w2105 w2116 w2127 w2138 w2150 w2161 w2172 w2183 w2193 w2204 w2214 w2244 w2265 w2291 w2295 w2311 w2314 w2318 w2329 w2338 w2360 w2377 w2381 w2391 w2400 w2414 w2418 w2431 w2449 w2465 w2501 w2558 w2581 w2593 w2634 w2677 w2720 w2762 w2765 w2782 w2795 w2797 w2810 w2814] -> w1515
      tunnel: [_ _ _ _ _ _ _ _ _ _ _ _ _ _ _ _ _ _ _ _ _ _ _ _ _ _ _ _ _ _ _ _ _ _ _ _ _ _ _ _ _ _ _ _ _ _ _ _ _ _ _ _ _ _ _ _ _ _ _ _ _ _ _ _ _ _ _ _ _ _ _ _ _ TRUE _] -> w1514
      tunnel: w1509 -> [_ _ _ _ _ _ _ _ _ _ _ _ _ _ _ _ _ _ _ _ _ _ _ _ _ _ _ _ _ _ _ _ _ _ _ _ _ _ _ _ _ _ _ _ _ _ _ _ _ _ _ _ _ _ _ _ _ _ _ _ _ _ _ _ _ _ _ _ _ _ _ w2794 _ _ _]
      tunnel: w1513 -> [_ _ _ _ _ _ _ _ _ _ _ _ _ _ _ _ _ _ _ _ _ _ _ _ _ _ _ _ _ _ _ _ _ _ _ _ _ _ _ _ _ _ _ _ _ _ _ _ _ _ _ _ _ _ _ _ _ _ _ _ _ _ _ _ _ _ _ _ _ _ _ _ _ w2806 _]
      frame "Timeout" {
        n890 = call "Time Out Loop.vi"("error in (no error)"=w1519, "Data Cluster"=w1517) -> ("error out"=w1518:errorcluster)  [unwired: 9 in]
      }
      frame "init" {
        # "Initialize - All initialization work should take place in this message, since other loops can potentially enqueue messages that execute immediately after this one."
        n891 = call-poly "Enqueue Message.vi"("error in (no error)"=w1563, "Message"="Init Other Loop", "Message Queue"=w1561) -> ("error out"=w1564:errorcluster)  [unwired: 7 in, 1 out]
        n892 = Unbundle By Name(w1521) -> ("Loading.SSP 0.3"=w1549:refnum<vi>)
        n893 = Unbundle By Name(w1521) -> ("Loading.SSP 0.5"=w1546:refnum<vi>)
        n894 = Unbundle By Name(w1521) -> ("Loading.SSP 0.75"=w1541:refnum<vi>)
        n895 = Unbundle By Name(w1521) -> ("Loading.Communication is established"=w1536:refnum<vi>)
        n896 = Unbundle By Name(w1521) -> ("Loading Com Port.Load Cell Temp"=w1555:refnum<vi>)
        n897 = Unbundle By Name(w1521) -> ("Motion Module.Set WTD"=w1529:refnum<vi>)
        n898 = call "Read Config Unitest.vi"("error in (no error)"=w1564, "main ref"=w1521) -> ("error out"=w1559:errorcluster)  [unwired: 9 in]
        n899 = Unbundle By Name(w1521) -> ("Motion Module.Wear Track Diameter"=w1523:refnum<vi>)
        n900 = Unbundle By Name(w1521) -> ("PID.Ramp"=w1533:refnum<vi>)
        n901 = call "Encrypt file path creation.vi"("error in (no error)"=w1559) -> ("error out"=w1558:errorcluster, "File Path"=w1557:path)  [unwired: 9 in]
        n902 = property class="Bool (strict)"(reference=w1555, "Value"=FALSE) -> (reference out=w1553:refnum<vi>, error out=w1554:errorcluster)  [unwired: 1 in]
        n903 = property class="Bool (strict)"(reference=w1546, "Visible"=FALSE) -> (reference out=w1544:refnum<vi>, error out=w1545:errorcluster)  [unwired: 1 in]
        n904 = property class="Bool (strict)"(reference=w1549, "Visible"=FALSE) -> (reference out=w1551:refnum<vi>, error out=w1550:errorcluster)  [unwired: 1 in]
        n905 = property class="Bool (strict)"(reference=w1541, "Visible"=FALSE) -> (reference out=w1543:refnum<vi>, error out=w1542:errorcluster)  [unwired: 1 in]
        n906 = property class="Bool (strict)"(reference=w1533, "Value"=FALSE) -> (reference out=w1535:refnum<vi>, error out=w1534:errorcluster)  [unwired: 1 in]
        n907 = property class="DigNum (strict)"(reference=w1523, "Value"=0.0) -> (reference out=w1522:refnum<vi>, error out=w1524:errorcluster)  [unwired: 1 in]
        n908 = property class="Bool (strict)"(reference=w1529, "Visible"=FALSE, "DisabledEnum"=T16."Disabled and Grayed Out" ("Disabled")) -> (reference out=w1526:refnum<vi>, error out=w1528:errorcluster)  [unwired: 1 in]
        n909 = property class="Bool (strict)"(reference=w1536, "Visible"=FALSE ("Value")) -> (reference out=w1538:refnum<vi>, error out=w1537:errorcluster)  [unwired: 1 in]
        n910 = call "DATA ENCRYPT STRING FILE WRITE.vi"("file path (dialog if empty)"=w1557, "error in (no error)"=w1558, "User Action"="System Booted", "main ref"=w1521) -> ("error out"=w1560:errorcluster)  [unwired: 5 in, 1 out]
        n911 = Close Reference(reference=w1544, error in (no error)=w1545) -> ()  [unwired: 1 out]
        n912 = Close Reference(reference=w1551, error in (no error)=w1550) -> ()  [unwired: 1 out]
        n913 = Close Reference(reference=w1543, error in (no error)=w1542) -> ()  [unwired: 1 out]
        n914 = Close Reference(reference=w1535, error in (no error)=w1534) -> ()  [unwired: 1 out]
        n915 = Close Reference(reference=w1553, error in (no error)=w1554) -> ()  [unwired: 1 out]
        n916 = Close Reference(reference=w1522, error in (no error)=w1524) -> ()  [unwired: 1 out]
        n917 = Close Reference(reference=w1526, error in (no error)=w1528) -> ()  [unwired: 1 out]
        n918 = Close Reference(reference=w1538, error in (no error)=w1537) -> ()  [unwired: 1 out]
        n919 = call "Reinitial Parameter After Test.vi"("error in (no error)"=w1560, "main ref"=w1521) -> ("error out"=w1530:errorcluster)  [unwired: 9 in]
        n920 = local write "HEAVE ENABLE"(FALSE ("HEAVE ENABLE")) -> ()
      }
      frame "Init Other Loop" {
      }
      frame "Service Save" {
        n921 = call "Write Config Unitest.vi"("error in (no error)"=w1569, "main ref"=w1568) -> ("error out"=w1574:errorcluster)  [unwired: 9 in]
        n922 = call "Stall Data Flow.vim"("value in"=w1574, "milliseconds to wait"=u32 2000) -> ("value out"=w1573:errorcluster)  [unwired: 1 out]
        n923 = call "Read Config Unitest.vi"("error in (no error)"=w1573, "main ref"=w1568) -> ("error out"=w1571:errorcluster)  [unwired: 9 in]
        n924 = call "DATA ENCRYPT STRING FILE WRITE.vi"("error in (no error)"=w1571, "User Action"="Service Parameter Saved", "main ref"=w1568) -> ("error out"=w1570:errorcluster)  [unwired: 6 in, 1 out]
      }
      frame "HOME" {
        n925 = call "DATA ENCRYPT STRING FILE WRITE.vi"("error in (no error)"=w1590, "User Action"="User Pressed Home", "main ref"=w1576) -> ("error out"=w1586:errorcluster)  [unwired: 6 in, 1 out]
        n926 = Unbundle By Name(w1576) -> ("Main Home Screen.MainPage"=w1581:refnum<vi>)
        n927 = Unbundle By Name(w1576) -> ("Main Home Screen.Home"=w1589:refnum<vi>)
        n928 = Unbundle By Name(w1576) -> ("Main Home Screen.GUI"=w1579:refnum<vi>)
        n929 = property class="Bool (strict)"(reference=w1589, error in=w1586, "Value"=FALSE) -> (reference out=w1587:refnum<vi>, error out=w1588:errorcluster)
        n930 = property class="TabCtl (strict)"(reference=w1581, "Value"=T5."HOME") -> (reference out=w1583:refnum<vi>, error out=w1582:errorcluster)  [unwired: 1 in]
        n931 = property class="TabCtl (strict)"(reference=w1579, "Value"=T4."Setup") -> (reference out=w1577:refnum<vi>, error out=w1578:errorcluster)  [unwired: 1 in]
        n932 = Close Reference(reference=w1587, error in (no error)=w1588) -> (error out=w1585:errorcluster)
        n933 = Close Reference(reference=w1583, error in (no error)=w1582) -> ()  [unwired: 1 out]
        n934 = Close Reference(reference=w1577, error in (no error)=w1578) -> ()  [unwired: 1 out]
      }
      frame "Platform Setting" {
        n935 = call "DATA ENCRYPT STRING FILE WRITE.vi"("error in (no error)"=w1607, "User Action"="User Pressed Platform Setting", "main ref"=w1593) -> ("error out"=w1603:errorcluster)  [unwired: 6 in, 1 out]
        n936 = Unbundle By Name(w1593) -> ("Main Home Screen.Platform Settings"=w1606:refnum<vi>)
        n937 = Unbundle By Name(w1593) -> ("Main Home Screen.MainPage"=w1598:refnum<vi>)
        n938 = Unbundle By Name(w1593) -> ("Main Home Screen.GUI"=w1596:refnum<vi>)
        n939 = property class="TabCtl (strict)"(reference=w1598, "Value"=T5."PlatformSetting") -> (reference out=w1600:refnum<vi>, error out=w1599:errorcluster)  [unwired: 1 in]
        n940 = property class="TabCtl (strict)"(reference=w1596, "Value"=T4."Setup") -> (reference out=w1594:refnum<vi>, error out=w1595:errorcluster)  [unwired: 1 in]
        n941 = property class="Bool (strict)"(reference=w1606, error in=w1603, "Value"=FALSE) -> (reference out=w1604:refnum<vi>, error out=w1605:errorcluster)
        n942 = Close Reference(reference=w1600, error in (no error)=w1599) -> ()  [unwired: 1 out]
        n943 = Close Reference(reference=w1594, error in (no error)=w1595) -> ()  [unwired: 1 out]
        n944 = Close Reference(reference=w1604, error in (no error)=w1605) -> (error out=w1602:errorcluster)
      }
      frame "Configure" {
        n945 = call "DATA ENCRYPT STRING FILE WRITE.vi"("error in (no error)"=w1624, "User Action"="User Pressed Configure", "main ref"=w1610) -> ("error out"=w1620:errorcluster)  [unwired: 6 in, 1 out]
        n946 = Unbundle By Name(w1610) -> ("Main Home Screen.Configure"=w1623:refnum<vi>)
        n947 = Unbundle By Name(w1610) -> ("Main Home Screen.MainPage"=w1615:refnum<vi>)
        n948 = Unbundle By Name(w1610) -> ("Main Home Screen.GUI"=w1613:refnum<vi>)
        n949 = property class="Bool (strict)"(reference=w1623, error in=w1620, "Value"=FALSE) -> (reference out=w1621:refnum<vi>, error out=w1622:errorcluster)
        n950 = property class="TabCtl (strict)"(reference=w1615, "Value"=T5."Details") -> (reference out=w1617:refnum<vi>, error out=w1616:errorcluster)  [unwired: 1 in]
        n951 = property class="TabCtl (strict)"(reference=w1613, "Value"=T4."Setup") -> (reference out=w1611:refnum<vi>, error out=w1612:errorcluster)  [unwired: 1 in]
        n952 = Close Reference(reference=w1621, error in (no error)=w1622) -> (error out=w1619:errorcluster)
        n953 = Close Reference(reference=w1617, error in (no error)=w1616) -> ()  [unwired: 1 out]
        n954 = Close Reference(reference=w1611, error in (no error)=w1612) -> ()  [unwired: 1 out]
      }
      frame "Analysis" {
        n955 = call "DATA ENCRYPT STRING FILE WRITE.vi"("error in (no error)"=w1641, "User Action"="User Pressed Analysis", "main ref"=w1627) -> ("error out"=w1637:errorcluster)  [unwired: 6 in, 1 out]
        n956 = Unbundle By Name(w1627) -> ("Main Home Screen.MainPage"=w1632:refnum<vi>)
        n957 = Unbundle By Name(w1627) -> ("Main Home Screen.Analysis"=w1640:refnum<vi>)
        n958 = Unbundle By Name(w1627) -> ("Main Home Screen.GUI"=w1630:refnum<vi>)
        n959 = property class="Bool (strict)"(reference=w1640, error in=w1637, "Value"=FALSE) -> (reference out=w1638:refnum<vi>, error out=w1639:errorcluster)
        n960 = property class="TabCtl (strict)"(reference=w1632, "Value"=T5."Analysis") -> (reference out=w1634:refnum<vi>, error out=w1633:errorcluster)  [unwired: 1 in]
        n961 = property class="TabCtl (strict)"(reference=w1630, "Value"=T4."Setup") -> (reference out=w1628:refnum<vi>, error out=w1629:errorcluster)  [unwired: 1 in]
        n962 = Close Reference(reference=w1638, error in (no error)=w1639) -> (error out=w1636:errorcluster)
        n963 = Close Reference(reference=w1634, error in (no error)=w1633) -> ()  [unwired: 1 out]
        n964 = Close Reference(reference=w1628, error in (no error)=w1629) -> ()  [unwired: 1 out]
      }
      frame "service 2" {
        n965 = call "DATA ENCRYPT STRING FILE WRITE.vi"("error in (no error)"=w1662, "User Action"="User Pressed service", "main ref"=w1645) -> ("error out"=w1658:errorcluster)  [unwired: 6 in, 1 out]
        n966 = Unbundle By Name(w1645) -> ("Main Screen.Main Screen Tab"=w1646:refnum<vi>)
        n967 = Unbundle By Name(w1645) -> ("Main Home Screen.MainPage"=w1653:refnum<vi>)
        n968 = Unbundle By Name(w1645) -> ("Main Home Screen.Analysis"=w1661:refnum<vi>)
        n969 = Unbundle By Name(w1645) -> ("Main Home Screen.GUI"=w1651:refnum<vi>)
        n970 = property class="Bool (strict)"(reference=w1661, error in=w1658, "Value"=FALSE) -> (reference out=w1659:refnum<vi>, error out=w1660:errorcluster)
        n971 = property class="TabCtl (strict)"(reference=w1653, "Value"=T5."HOME") -> (reference out=w1655:refnum<vi>, error out=w1654:errorcluster)  [unwired: 1 in]
        n972 = property class="TabCtl (strict)"(reference=w1651, "Value"=T4."Begin") -> (reference out=w1649:refnum<vi>, error out=w1650:errorcluster)  [unwired: 1 in]
        n973 = property class="TabCtl (strict)"(reference=w1646, "Value"=T8."About") -> (reference out=w1643:refnum<vi>, error out=w1647:errorcluster)  [unwired: 1 in]
        n974 = Close Reference(reference=w1659, error in (no error)=w1660) -> (error out=w1657:errorcluster)
        n975 = Close Reference(reference=w1655, error in (no error)=w1654) -> ()  [unwired: 1 out]
        n976 = Close Reference(reference=w1649, error in (no error)=w1650) -> ()  [unwired: 1 out]
        n977 = Close Reference(reference=w1643, error in (no error)=w1647) -> ()  [unwired: 1 out]
      }
      frame "Auto" {
        n978 = call "DATA ENCRYPT STRING FILE WRITE.vi"("error in (no error)"=w1675, "User Action"="User Pressed Auto File Name", "main ref"=w1665) -> ("error out"=w1672:errorcluster)  [unwired: 6 in, 1 out]
        n979 = Get Date/Time In Seconds() -> (seconds since 1Jan1904=w1673:timestamp)
        n980 = Format Into String(format string="%<%I_%M_%S_%p_%d_%B_%Y>T", error in=w1672, w1673) -> (resulting string=w1666:string, error out=w1668:errorcluster)  [unwired: 1 in]
        n981 = local write "Auto"(FALSE ("Auto")) -> ()
        n982 = Unbundle By Name(w1665) -> ("Config Screen.FILE"=w1671:refnum<vi>)
        n983 = property class="Str"(reference=w1671, error in=w1668, "Value"=w1666) -> (reference out=w1669:refnum<vi>, error out=w1670:errorcluster)
        n984 = Close Reference(reference=w1669, error in (no error)=w1670) -> (error out=w1667:errorcluster)
      }
      frame "Select Load Head" {
        n985 = call "Reinitial Parameter.vi"("error in (no error)"=w1680, "Data Cluster"=w1677) -> ("error out"=w1679:errorcluster)  [unwired: 9 in]
        n986 = call "FILE NAME RECHECK.vi"("error in (no error)"=w1679, "main ref"=w1677) -> ("error out"=w1678:errorcluster)  [unwired: 9 in]
      }
      frame "com 3" {
        n987 = call "DATA ENCRYPT STRING FILE WRITE.vi"("error in (no error)"=w1684, "User Action"="User Pressed Check Load Communication", "main ref"=w1681) -> ("error out"=w1683:errorcluster)  [unwired: 6 in, 1 out]
        n988 = call "SET LOAD PARAMETERS.vi"("error in (no error)"=w1683, "main ref"=w1681) -> ("error out"=w1682:errorcluster)  [unwired: 9 in]
      }
      frame "ZeroAll" {
        n989 = call "DATA ENCRYPT STRING FILE WRITE.vi"("error in (no error)"=w1691, "User Action"="User Pressed Zero All", "main ref"=w1687) -> ("error out"=w1690:errorcluster)  [unwired: 6 in, 1 out]
        n990 = local write "ZeroAll"(FALSE ("ZeroAll")) -> ()
        n991 = call "LOAD CELL FGV MAIN.vi"("Enum"=T17."ZEROALL", "error in (no error)"=w1690, "main ref"=w1687) -> ("error IO"=w1689:errorcluster)  [unwired: 8 in]
      }
      frame "Loading Mode" {
        n992 = Unbundle By Name(w1695) -> ("Loading.Loading Mode"=w1697:refnum<vi>)
        n993 = property class="Ring (strict)"(reference=w1697, error in=w1696) -> (reference out=w1699:refnum<vi>, error out=w1698:errorcluster, "Value"=w1693:u16)
        n994 = Close Reference(reference=w1699, error in (no error)=w1698) -> (error out=w1694:errorcluster)
        n995 = case shown="1" w1693 {
          tunnel: [w1714 w1731 w1743 w1755] -> w1700
          tunnel: w1695 -> [w1701 w1717 w1735 w1747]
          tunnel: w1694 -> [w1715 w1730 w1742 w1754]
          frame 0, Default {
            n996 = Unbundle By Name(w1701) -> ("Loading.Enter the Loading Rate (N/min)"=w1708:refnum<vi>)
            n997 = Unbundle By Name(w1701) -> ("Loading.Load Selection"=w1711:refnum<vi>)
            n998 = Unbundle By Name(w1701) -> ("Loading.Enter the Final Load (N)"=w1703:refnum<vi>)
            n999 = property class="TabCtl (strict)"(reference=w1711, "Value"=T6."Constant") -> (reference out=w1713:refnum<vi>, error out=w1712:errorcluster)  [unwired: 1 in]
            n1000 = property class="DigNum (strict)"(reference=w1708, "DisabledEnum"=T16."Disabled and Grayed Out" ("Disabled")) -> (reference out=w1707:refnum<vi>, error out=w1709:errorcluster)  [unwired: 1 in]
            n1001 = property class="DigNum (strict)"(reference=w1703, "DisabledEnum"=T16."Disabled and Grayed Out" ("Disabled")) -> (reference out=w1704:refnum<vi>, error out=w1702:errorcluster)  [unwired: 1 in]
            n1002 = call "DATA ENCRYPT STRING FILE WRITE.vi"("error in (no error)"=w1715, "User Action"="User selected Constant Mode", "main ref"=w1701) -> ("error out"=w1714:errorcluster)  [unwired: 6 in, 1 out]
            n1003 = Close Reference(reference=w1713, error in (no error)=w1712) -> ()  [unwired: 1 out]
            n1004 = Close Reference(reference=w1707, error in (no error)=w1709) -> ()  [unwired: 1 out]
            n1005 = Close Reference(reference=w1704, error in (no error)=w1702) -> ()  [unwired: 1 out]
          }
          frame 1 {
            n1006 = Unbundle By Name(w1717) -> ("Loading.Enter the Loading Rate (N/min)"=w1728:refnum<vi>)
            n1007 = Unbundle By Name(w1717) -> ("Loading.Enter the Final Load (N)"=w1723:refnum<vi>)
            n1008 = Unbundle By Name(w1717) -> ("Loading.Load Selection"=w1719:refnum<vi>)
            n1009 = property class="TabCtl (strict)"(reference=w1719, "Value"=T6."Constant") -> (reference out=w1721:refnum<vi>, error out=w1720:errorcluster)  [unwired: 1 in]
            n1010 = property class="DigNum (strict)"(reference=w1728, "DisabledEnum"=T16."Enabled" ("Disabled")) -> (reference out=w1727:refnum<vi>, error out=w1729:errorcluster)  [unwired: 1 in]
            n1011 = property class="DigNum (strict)"(reference=w1723, "DisabledEnum"=T16."Enabled" ("Disabled")) -> (reference out=w1724:refnum<vi>, error out=w1722:errorcluster)  [unwired: 1 in]
            n1012 = call "DATA ENCRYPT STRING FILE WRITE.vi"("error in (no error)"=w1730, "User Action"="User selected Ramp Mode", "main ref"=w1717) -> ("error out"=w1731:errorcluster)  [unwired: 6 in, 1 out]
            n1013 = Close Reference(reference=w1721, error in (no error)=w1720) -> ()  [unwired: 1 out]
            n1014 = Close Reference(reference=w1727, error in (no error)=w1729) -> ()  [unwired: 1 out]
            n1015 = Close Reference(reference=w1724, error in (no error)=w1722) -> ()  [unwired: 1 out]
          }
          frame 2 {
            n1016 = Unbundle By Name(w1735) -> ("Loading.Load Selection"=w1739:refnum<vi>)
            n1017 = Unbundle By Name(w1735) -> ("Loading.Warning 2"=w1737:refnum<vi>)
            n1018 = property class="TabCtl (strict)"(reference=w1739, "Value"=T6."Step") -> (reference out=w1741:refnum<vi>, error out=w1740:errorcluster)  [unwired: 1 in]
            n1019 = property class="Bool (strict)"(reference=w1737, "Visible"=FALSE) -> (reference out=w1733:refnum<vi>, error out=w1736:errorcluster)  [unwired: 1 in]
            n1020 = call "DATA ENCRYPT STRING FILE WRITE.vi"("error in (no error)"=w1742, "User Action"="User selected Step Mode", "main ref"=w1735) -> ("error out"=w1743:errorcluster)  [unwired: 6 in, 1 out]
            n1021 = Close Reference(reference=w1741, error in (no error)=w1740) -> ()  [unwired: 1 out]
            n1022 = Close Reference(reference=w1733, error in (no error)=w1736) -> ()  [unwired: 1 out]
          }
          frame 3 {
            n1023 = Unbundle By Name(w1747) -> ("Loading.Load Selection"=w1751:refnum<vi>)
            n1024 = Unbundle By Name(w1747) -> ("Loading.Warning 2"=w1749:refnum<vi>)
            n1025 = property class="TabCtl (strict)"(reference=w1751, "Value"=T6."Indentation") -> (reference out=w1753:refnum<vi>, error out=w1752:errorcluster)  [unwired: 1 in]
            n1026 = property class="Bool (strict)"(reference=w1749, "Visible"=FALSE) -> (reference out=w1745:refnum<vi>, error out=w1748:errorcluster)  [unwired: 1 in]
            n1027 = call "DATA ENCRYPT STRING FILE WRITE.vi"("error in (no error)"=w1754, "User Action"="User selected Indentation Mode", "main ref"=w1747) -> ("error out"=w1755:errorcluster)  [unwired: 6 in, 1 out]
            n1028 = Close Reference(reference=w1753, error in (no error)=w1752) -> ()  [unwired: 1 out]
            n1029 = Close Reference(reference=w1745, error in (no error)=w1748) -> ()  [unwired: 1 out]
          }
        }
      }
      frame "SSP 0.3" {
        n1030 = Unbundle By Name(w1759) -> ("Loading.SSP 0.3"=w1762:refnum<vi>)
        n1031 = property class="Bool (strict)"(reference=w1762, error in=w1761) -> (reference out=w1764:refnum<vi>, error out=w1763:errorcluster, "Value"=w1760:bool)
        n1032 = Close Reference(reference=w1764, error in (no error)=w1763) -> (error out=w1758:errorcluster)
        n1033 = case shown="True" w1760 {
          tunnel: w1759 -> [_ w1766]
          tunnel: w1758 -> [w1765 w1774]
          tunnel: [w1765 w1773] -> w1757
          frame False {
          }
          frame True {
            w1776 = FALSE ("Value")
            n1034 = Unbundle By Name(w1766) -> ("Loading.Enter the Load  (N)"=w1772:refnum<vi>)
            n1035 = Unbundle By Name(w1766) -> ("Loading.SSP 0.75"=w1777:refnum<vi>)
            n1036 = Unbundle By Name(w1766) -> ("Loading.SSP 0.5"=w1782:refnum<vi>)
            n1037 = property class="Bool (strict)"(reference=w1777, "Value"=w1776) -> (reference out=w1779:refnum<vi>, error out=w1778:errorcluster)  [unwired: 1 in]
            n1038 = property class="Bool (strict)"(reference=w1782, "Value"=w1776) -> (reference out=w1780:refnum<vi>, error out=w1781:errorcluster)  [unwired: 1 in]
            n1039 = property class="DigNum (strict)"(reference=w1772, "Minimum"=2.0 ("Data Entry Limits:Minimum"), "Maximum"=50.0 ("Data Entry Limits:Maximum"), "Increment"=0.1 ("Data Entry Limits:Increment")) -> (reference out=w1770:refnum<vi>, error out=w1771:errorcluster)  [unwired: 1 in]
            n1040 = call "DATA ENCRYPT STRING FILE WRITE.vi"("error in (no error)"=w1774, "User Action"="User selected 0.3 SSP", "main ref"=w1766) -> ("error out"=w1773:errorcluster)  [unwired: 6 in, 1 out]
            n1041 = Close Reference(reference=w1779, error in (no error)=w1778) -> ()  [unwired: 1 out]
            n1042 = Close Reference(reference=w1780, error in (no error)=w1781) -> ()  [unwired: 1 out]
            n1043 = Close Reference(reference=w1770, error in (no error)=w1771) -> ()  [unwired: 1 out]
          }
        }
      }
      frame "SSP 0.5" {
        n1044 = Unbundle By Name(w1785) -> ("Loading.SSP 0.5"=w1788:refnum<vi>)
        n1045 = property class="Bool (strict)"(reference=w1788, error in=w1787) -> (reference out=w1790:refnum<vi>, error out=w1789:errorcluster, "Value"=w1786:bool)
        n1046 = Close Reference(reference=w1790, error in (no error)=w1789) -> (error out=w1784:errorcluster)
        n1047 = case shown="True" w1786 {
          tunnel: w1785 -> [_ w1792]
          tunnel: w1784 -> [w1791 w1800]
          tunnel: [w1791 w1799] -> w1783
          frame False {
          }
          frame True {
            w1802 = FALSE ("Value")
            n1048 = Unbundle By Name(w1792) -> ("Loading.Enter the Load  (N)"=w1798:refnum<vi>)
            n1049 = Unbundle By Name(w1792) -> ("Loading.SSP 0.75"=w1808:refnum<vi>)
            n1050 = Unbundle By Name(w1792) -> ("Loading.SSP 0.3"=w1803:refnum<vi>)
            n1051 = property class="Bool (strict)"(reference=w1803, "Value"=w1802) -> (reference out=w1805:refnum<vi>, error out=w1804:errorcluster)  [unwired: 1 in]
            n1052 = property class="Bool (strict)"(reference=w1808, "Value"=w1802) -> (reference out=w1806:refnum<vi>, error out=w1807:errorcluster)  [unwired: 1 in]
            n1053 = property class="DigNum (strict)"(reference=w1798, "Minimum"=2.0 ("Data Entry Limits:Minimum"), "Maximum"=200.0 ("Data Entry Limits:Maximum"), "Increment"=0.1 ("Data Entry Limits:Increment")) -> (reference out=w1796:refnum<vi>, error out=w1797:errorcluster)  [unwired: 1 in]
            n1054 = call "DATA ENCRYPT STRING FILE WRITE.vi"("error in (no error)"=w1800, "User Action"="User selected 0.5 SSP", "main ref"=w1792) -> ("error out"=w1799:errorcluster)  [unwired: 6 in, 1 out]
            n1055 = Close Reference(reference=w1805, error in (no error)=w1804) -> ()  [unwired: 1 out]
            n1056 = Close Reference(reference=w1806, error in (no error)=w1807) -> ()  [unwired: 1 out]
            n1057 = Close Reference(reference=w1796, error in (no error)=w1797) -> ()  [unwired: 1 out]
          }
        }
      }
      frame "SSP 0.75" {
        n1058 = Unbundle By Name(w1811) -> ("Loading.SSP 0.75"=w1814:refnum<vi>)
        n1059 = property class="Bool (strict)"(reference=w1814, error in=w1813) -> (reference out=w1816:refnum<vi>, error out=w1815:errorcluster, "Value"=w1812:bool)
        n1060 = Close Reference(reference=w1816, error in (no error)=w1815) -> (error out=w1810:errorcluster)
        n1061 = case shown="True" w1812 {
          tunnel: w1811 -> [_ w1818]
          tunnel: w1810 -> [w1817 w1826]
          tunnel: [w1817 w1825] -> w1809
          frame False {
          }
          frame True {
            w1828 = FALSE ("Value")
            n1062 = Unbundle By Name(w1818) -> ("Loading.SSP 0.3"=w1829:refnum<vi>)
            n1063 = Unbundle By Name(w1818) -> ("Loading.SSP 0.5"=w1834:refnum<vi>)
            n1064 = Unbundle By Name(w1818) -> ("Loading.Enter the Load  (N)"=w1824:refnum<vi>)
            n1065 = property class="Bool (strict)"(reference=w1829, "Value"=w1828) -> (reference out=w1831:refnum<vi>, error out=w1830:errorcluster)  [unwired: 1 in]
            n1066 = property class="Bool (strict)"(reference=w1834, "Value"=w1828) -> (reference out=w1832:refnum<vi>, error out=w1833:errorcluster)  [unwired: 1 in]
            n1067 = property class="DigNum (strict)"(reference=w1824, "Minimum"=200.0 ("Data Entry Limits:Minimum"), "Maximum"=500.0 ("Data Entry Limits:Maximum"), "Increment"=0.1 ("Data Entry Limits:Increment")) -> (reference out=w1822:refnum<vi>, error out=w1823:errorcluster)  [unwired: 1 in]
            n1068 = call "DATA ENCRYPT STRING FILE WRITE.vi"("error in (no error)"=w1826, "User Action"="User selected 0.75 SSP", "main ref"=w1818) -> ("error out"=w1825:errorcluster)  [unwired: 6 in, 1 out]
            n1069 = Close Reference(reference=w1831, error in (no error)=w1830) -> ()  [unwired: 1 out]
            n1070 = Close Reference(reference=w1832, error in (no error)=w1833) -> ()  [unwired: 1 out]
            n1071 = Close Reference(reference=w1822, error in (no error)=w1823) -> ()  [unwired: 1 out]
          }
        }
      }
      frame "LHBack" {
        # "Back to Configure"
        n1072 = Unbundle By Name(w1836) -> ("Main Home Screen.GUI"=w1845:refnum<vi>)
        n1073 = Unbundle By Name(w1836) -> ("Main Home Screen.MainPage"=w1841:refnum<vi>)
        n1074 = Unbundle By Name(w1836) -> ("Loading.LHBack"=w1839:refnum<vi>)
        n1075 = property class="TabCtl (strict)"(reference=w1841, "Value"=T5."HOME") -> (reference out=w1843:refnum<vi>, error out=w1842:errorcluster)  [unwired: 1 in]
        n1076 = property class="Bool (strict)"(reference=w1839, "Value"=FALSE) -> (reference out=w1837:refnum<vi>, error out=w1838:errorcluster)  [unwired: 1 in]
        n1077 = property class="TabCtl (strict)"(reference=w1845, "Value"=T4."Setup") -> (reference out=w1847:refnum<vi>, error out=w1846:errorcluster)  [unwired: 1 in]
        n1078 = Close Reference(reference=w1843, error in (no error)=w1842) -> ()  [unwired: 1 out]
        n1079 = Close Reference(reference=w1837, error in (no error)=w1838) -> ()  [unwired: 1 out]
        n1080 = Close Reference(reference=w1847, error in (no error)=w1846) -> ()  [unwired: 1 out]
        n1081 = call "DATA ENCRYPT STRING FILE WRITE.vi"("error in (no error)"=w1848, "User Action"="User selected Back to Configure", "main ref"=w1836) -> ("error out"=w1849:errorcluster)  [unwired: 6 in, 1 out]
      }
      frame "MMBack" {
        # "Back to Configure"
        n1082 = Unbundle By Name(w1851) -> ("Motion Module.MMBack"=w1855:refnum<vi>)
        n1083 = Unbundle By Name(w1851) -> ("Main Home Screen.GUI"=w1861:refnum<vi>)
        n1084 = Unbundle By Name(w1851) -> ("Main Home Screen.MainPage"=w1857:refnum<vi>)
        n1085 = property class="Bool (strict)"(reference=w1855, "Value"=FALSE) -> (reference out=w1853:refnum<vi>, error out=w1854:errorcluster)  [unwired: 1 in]
        n1086 = property class="TabCtl (strict)"(reference=w1857, "Value"=T5."HOME") -> (reference out=w1859:refnum<vi>, error out=w1858:errorcluster)  [unwired: 1 in]
        n1087 = property class="TabCtl (strict)"(reference=w1861, "Value"=T4."Load Head") -> (reference out=w1863:refnum<vi>, error out=w1862:errorcluster)  [unwired: 1 in]
        n1088 = Close Reference(reference=w1853, error in (no error)=w1854) -> ()  [unwired: 1 out]
        n1089 = Close Reference(reference=w1859, error in (no error)=w1858) -> ()  [unwired: 1 out]
        n1090 = Close Reference(reference=w1863, error in (no error)=w1862) -> ()  [unwired: 1 out]
        n1091 = call "DATA ENCRYPT STRING FILE WRITE.vi"("error in (no error)"=w1864, "User Action"="User selected Back to Load Selection", "main ref"=w1851) -> ("error out"=w1865:errorcluster)  [unwired: 6 in, 1 out]
      }
      frame "LHNext" {
        w1901 = FALSE ("Visible")
        n1092 = Unbundle By Name(w1867) -> ("Motion Module.HomeRot"=w1907:refnum<vi>)
        n1093 = Unbundle By Name(w1867) -> ("Motion Module.HomeScratch"=w1902:refnum<vi>)
        n1094 = Unbundle By Name(w1867) -> ("Motion Module.PlaceModule"=w1900:refnum<vi>)
        n1095 = Unbundle By Name(w1867) -> ("Motion Module.Motion Mode:"=w1893:refnum<vi>)
        n1096 = Unbundle By Name(w1867) -> ("Motion Module.Motion Direction:  3"=w1892:refnum<vi>)
        n1097 = Unbundle By Name(w1867) -> ("Motion Module.Wear Track Diameter (mm)"=w1886:refnum<vi>)
        n1098 = Unbundle By Name(w1867) -> ("Motion Module.Set WTD"=w1883:refnum<vi>)
        n1099 = Unbundle By Name(w1867) -> ("Motion Module.Rotary Module Selection"=w1877:refnum<vi>)
        n1100 = call "DATA ENCRYPT STRING FILE WRITE.vi"("error in (no error)"=w1916, "User Action"="User selected Select Module", "main ref"=w1867) -> ("error out"=w1880:errorcluster)  [unwired: 6 in, 1 out]
        n1101 = property class="TabCtl (strict)"(reference=w1877, "Visible"=FALSE) -> (reference out=w1876:refnum<vi>, error out=w1878:errorcluster)  [unwired: 1 in]
        n1102 = property class="Bool (strict)"(reference=w1907, error in=w1880, "Visible"=w1901) -> (reference out=w1905:refnum<vi>, error out=w1906:errorcluster)
        n1103 = property class="Bool (strict)"(reference=w1902, error in=w1880, "Visible"=w1901) -> (reference out=w1904:refnum<vi>, error out=w1903:errorcluster)
        n1104 = property class="Bool (strict)"(reference=w1900, error in=w1880, "Visible"=TRUE) -> (reference out=w1898:refnum<vi>, error out=w1899:errorcluster)
        n1105 = property class="Ring (strict)"(reference=w1893, error in=w1880, "Visible"=FALSE) -> (reference out=w1895:refnum<vi>, error out=w1894:errorcluster)
        n1106 = property class="Ring (strict)"(reference=w1892, error in=w1880, "Visible"=FALSE) -> (reference out=w1889:refnum<vi>, error out=w1891:errorcluster)
        n1107 = property class="DigNum (strict)"(reference=w1886, "Visible"=FALSE) -> (reference out=w1885:refnum<vi>, error out=w1887:errorcluster)  [unwired: 1 in]
        n1108 = property class="Bool (strict)"(reference=w1883, "Visible"=FALSE) -> (reference out=w1884:refnum<vi>, error out=w1882:errorcluster)  [unwired: 1 in]
        n1109 = Close Reference(reference=w1905, error in (no error)=w1906) -> ()  [unwired: 1 out]
        n1110 = Close Reference(reference=w1904, error in (no error)=w1903) -> ()  [unwired: 1 out]
        n1111 = Close Reference(reference=w1898, error in (no error)=w1899) -> ()  [unwired: 1 out]
        n1112 = Close Reference(reference=w1895, error in (no error)=w1894) -> ()  [unwired: 1 out]
        n1113 = Close Reference(reference=w1889, error in (no error)=w1891) -> ()  [unwired: 1 out]
        n1114 = Close Reference(reference=w1885, error in (no error)=w1887) -> ()  [unwired: 1 out]
        n1115 = Close Reference(reference=w1876, error in (no error)=w1878) -> ()  [unwired: 1 out]
        n1116 = Close Reference(reference=w1884, error in (no error)=w1882) -> ()  [unwired: 1 out]
        n1117 = Unbundle By Name(w1867) -> ("Motion Module.M3 Image"=w1875:refnum<vi>)
        n1118 = Unbundle By Name(w1867) -> ("Main Home Screen.GUI"=w1913:refnum<vi>)
        n1119 = Unbundle By Name(w1867) -> ("Main Home Screen.MainPage"=w1909:refnum<vi>)
        n1120 = Unbundle By Name(w1867) -> ("Loading.LHNext"=w1871:refnum<vi>)
        n1121 = property class="TabCtl (strict)"(reference=w1875, "Value"=enum32{"Page 1", "Page 2"}."Page 2") -> (reference out=w1873:refnum<vi>, error out=w1874:errorcluster)  [unwired: 1 in]
        n1122 = property class="TabCtl (strict)"(reference=w1909, "Value"=T5."HOME") -> (reference out=w1911:refnum<vi>, error out=w1910:errorcluster)  [unwired: 1 in]
        n1123 = property class="TabCtl (strict)"(reference=w1913, "Value"=T4."Motion Module") -> (reference out=w1915:refnum<vi>, error out=w1914:errorcluster)  [unwired: 1 in]
        n1124 = property class="Bool (strict)"(reference=w1871, "Value"=FALSE ("Visible")) -> (reference out=w1868:refnum<vi>, error out=w1870:errorcluster)  [unwired: 1 in]
        n1125 = Close Reference(reference=w1873, error in (no error)=w1874) -> ()  [unwired: 1 out]
        n1126 = Close Reference(reference=w1868, error in (no error)=w1870) -> ()  [unwired: 1 out]
        n1127 = Close Reference(reference=w1911, error in (no error)=w1910) -> ()  [unwired: 1 out]
        n1128 = Close Reference(reference=w1915, error in (no error)=w1914) -> ()  [unwired: 1 out]
      }
      frame "Rot Ver" {
        n1129 = call "Rotory Module Selection.vi"("error in (no error)"=w1920, "Data Cluster"=w1918) -> ("error out"=w1919:errorcluster)  [unwired: 9 in]
      }
      frame "Scratch" {
        n1130 = call "Scratch Module Selection.vi"("error in (no error)"=w1923, "Data Cluster"=w1921) -> ("error out"=w1922:errorcluster)  [unwired: 9 in]
      }
      frame "Motion Mode:" {
        n1131 = Unbundle By Name(w1924) -> ("Motion Module.Motion Mode:"=w1926:refnum<vi>)
        n1132 = property class="Ring (strict)"(reference=w1926) -> (reference out=w1928:refnum<vi>, error out=w1927:errorcluster, "Value"=w1925:u16)  [unwired: 1 in]
        n1133 = Close Reference(reference=w1928, error in (no error)=w1927) -> ()  [unwired: 1 out]
        n1134 = case shown="3" w1925 {
          tunnel: w1930 -> [w1939 w1948 w1957 w1966]
          tunnel: [w1938 w1947 w1956 w1965] -> w1929
          tunnel: w1924 -> [w1937 w1946 w1955 w1964]
          tunnel: w1924 -> [w1932 w1941 w1950 w1959]
          frame 0, Default {
            n1135 = Unbundle By Name(w1932) -> ("Motion Module.Rotary Module Selection"=w1933:refnum<vi>)
            n1136 = property class="TabCtl (strict)"(reference=w1933, "Value"=T7."Uniform Rotation") -> (reference out=w1935:refnum<vi>, error out=w1934:errorcluster)  [unwired: 1 in]
            n1137 = Close Reference(reference=w1935, error in (no error)=w1934) -> ()  [unwired: 1 out]
            n1138 = call "DATA ENCRYPT STRING FILE WRITE.vi"("error in (no error)"=w1939, "User Action"="User Selected Uniform Rotation", "main ref"=w1937) -> ("error out"=w1938:errorcluster)  [unwired: 6 in, 1 out]
          }
          frame 1 {
            n1139 = Unbundle By Name(w1941) -> ("Motion Module.Rotary Module Selection"=w1942:refnum<vi>)
            n1140 = property class="TabCtl (strict)"(reference=w1942, "Value"=T7."Angular Oscillation") -> (reference out=w1944:refnum<vi>, error out=w1943:errorcluster)  [unwired: 1 in]
            n1141 = Close Reference(reference=w1944, error in (no error)=w1943) -> ()  [unwired: 1 out]
            n1142 = call "DATA ENCRYPT STRING FILE WRITE.vi"("error in (no error)"=w1948, "User Action"="User Selected Angular Oscillation", "main ref"=w1946) -> ("error out"=w1947:errorcluster)  [unwired: 6 in, 1 out]
          }
          frame 2 {
            n1143 = Unbundle By Name(w1950) -> ("Motion Module.Rotary Module Selection"=w1951:refnum<vi>)
            n1144 = property class="TabCtl (strict)"(reference=w1951, "Value"=T7."Speed Ramp") -> (reference out=w1953:refnum<vi>, error out=w1952:errorcluster)  [unwired: 1 in]
            n1145 = Close Reference(reference=w1953, error in (no error)=w1952) -> ()  [unwired: 1 out]
            n1146 = call "DATA ENCRYPT STRING FILE WRITE.vi"("error in (no error)"=w1957, "User Action"="User Selected Ramp Mode", "main ref"=w1955) -> ("error out"=w1956:errorcluster)  [unwired: 6 in, 1 out]
          }
          frame 3 {
            n1147 = Unbundle By Name(w1959) -> ("Motion Module.Rotary Module Selection"=w1960:refnum<vi>)
            n1148 = property class="TabCtl (strict)"(reference=w1960, "Value"=T7."Speed Step") -> (reference out=w1962:refnum<vi>, error out=w1961:errorcluster)  [unwired: 1 in]
            n1149 = Close Reference(reference=w1962, error in (no error)=w1961) -> ()  [unwired: 1 out]
            n1150 = call "DATA ENCRYPT STRING FILE WRITE.vi"("error in (no error)"=w1966, "User Action"="User Selected Step Mode", "main ref"=w1964) -> ("error out"=w1965:errorcluster)  [unwired: 6 in, 1 out]
          }
        }
      }
      frame "MMNext" {
        n1151 = Unbundle By Name(w1967) -> ("Motion Module.MMNext"=w1971:refnum<vi>)
        n1152 = Unbundle By Name(w1967) -> ("Motion Module.MMNext"=w1978:refnum<vi>)
        n1153 = Unbundle By Name(w1967) -> ("Main Home Screen.GUI"=w1980:refnum<vi>)
        n1154 = property class="Bool (strict)"(reference=w1971, "Value"=FALSE ("Visible")) -> (reference out=w1968:refnum<vi>, error out=w1970:errorcluster)  [unwired: 1 in]
        n1155 = property class="TabCtl (strict)"(reference=w1980, "Value"=T4."Environment") -> (reference out=w1982:refnum<vi>, error out=w1981:errorcluster)  [unwired: 1 in]
        n1156 = property class="Bool (strict)"(reference=w1978, "Value"=FALSE) -> (reference out=w1976:refnum<vi>, error out=w1977:errorcluster)  [unwired: 1 in]
        n1157 = Close Reference(reference=w1968, error in (no error)=w1970) -> ()  [unwired: 1 out]
        n1158 = Close Reference(reference=w1976, error in (no error)=w1977) -> ()  [unwired: 1 out]
        n1159 = Close Reference(reference=w1982, error in (no error)=w1981) -> ()  [unwired: 1 out]
        n1160 = call "DATA ENCRYPT STRING FILE WRITE.vi"("error in (no error)"=w1973, "User Action"="User Selected SetUp Module", "main ref"=w1967) -> ("error out"=w1972:errorcluster)  [unwired: 6 in, 1 out]
      }
      frame "APBack" {
        n1161 = Unbundle By Name(w1983) -> ("Environmental control.APBack"=w1990:refnum<vi>)
        n1162 = Unbundle By Name(w1983) -> ("Main Home Screen.GUI"=w1992:refnum<vi>)
        n1163 = property class="TabCtl (strict)"(reference=w1992, "Value"=T4."Motion Module") -> (reference out=w1994:refnum<vi>, error out=w1993:errorcluster)  [unwired: 1 in]
        n1164 = property class="Bool (strict)"(reference=w1990, "Value"=FALSE) -> (reference out=w1988:refnum<vi>, error out=w1989:errorcluster)  [unwired: 1 in]
        n1165 = Close Reference(reference=w1988, error in (no error)=w1989) -> ()  [unwired: 1 out]
        n1166 = Close Reference(reference=w1994, error in (no error)=w1993) -> ()  [unwired: 1 out]
        n1167 = call "DATA ENCRYPT STRING FILE WRITE.vi"("error in (no error)"=w1985, "User Action"="User Selected Back to Module", "main ref"=w1983) -> ("error out"=w1984:errorcluster)  [unwired: 6 in, 1 out]
      }
      frame "SNext" {
        w2007 = FALSE ("Value")
        n1168 = Unbundle By Name(w1996) -> ("Main Screen.zNL 2"=w1999:refnum<vi>)
        n1169 = Unbundle By Name(w1996) -> ("Main Screen.Start Test"=w2010:refnum<vi>)
        n1170 = Unbundle By Name(w1996) -> ("Main Screen.STOP"=w2009:refnum<vi>)
        n1171 = Unbundle By Name(w1996) -> ("Environmental control.SNext"=w2019:refnum<vi>)
        n1172 = Unbundle By Name(w1996) -> ("Main Home Screen.GUI"=w2021:refnum<vi>)
        n1173 = Unbundle By Name(w1996) -> ("PID.Ramp"=w2002:refnum<vi>)
        n1174 = property class="Bool (strict)"(reference=w1999, "DisabledEnum"=T16."Enabled" ("Disabled")) -> (reference out=w1997:refnum<vi>, error out=w1998:errorcluster)  [unwired: 1 in]
        n1175 = property class="Bool (strict)"(reference=w2002, "Value"=FALSE) -> (reference out=w2000:refnum<vi>, error out=w2003:errorcluster)  [unwired: 1 in]
        n1176 = property class="Bool (strict)"(reference=w2010, "Visible"=TRUE ("Value"), "Value"=FALSE) -> (reference out=w2005:refnum<vi>, error out=w2011:errorcluster)  [unwired: 1 in]
        n1177 = property class="Bool (strict)"(reference=w2009, "Value"=w2007, "Visible"=w2007) -> (reference out=w2004:refnum<vi>, error out=w2008:errorcluster)  [unwired: 1 in]
        n1178 = property class="TabCtl (strict)"(reference=w2021, "Value"=T4."Begin") -> (reference out=w2023:refnum<vi>, error out=w2022:errorcluster)  [unwired: 1 in]
        n1179 = property class="Bool (strict)"(reference=w2019, "Value"=FALSE) -> (reference out=w2017:refnum<vi>, error out=w2018:errorcluster)  [unwired: 1 in]
        n1180 = Close Reference(reference=w1997, error in (no error)=w1998) -> ()  [unwired: 1 out]
        n1181 = Close Reference(reference=w2000, error in (no error)=w2003) -> ()  [unwired: 1 out]
        n1182 = Close Reference(reference=w2005, error in (no error)=w2011) -> ()  [unwired: 1 out]
        n1183 = Close Reference(reference=w2004, error in (no error)=w2008) -> ()  [unwired: 1 out]
        n1184 = Close Reference(reference=w2017, error in (no error)=w2018) -> ()  [unwired: 1 out]
        n1185 = Close Reference(reference=w2023, error in (no error)=w2022) -> ()  [unwired: 1 out]
        n1186 = call "DATA ENCRYPT STRING FILE WRITE.vi"("error in (no error)"=w2014, "User Action"="User Pressed Setup", "main ref"=w1996) -> ("error out"=w2013:errorcluster)  [unwired: 6 in, 1 out]
      }
      frame "Enable Platform" {
        n1187 = Unbundle By Name(w2026) -> ("Heave AND Surge.Sequence ID"=w2028:refnum<vi>)
        n1188 = Unbundle By Name(w2026) -> ("Heave AND Surge.Mode Command"=w2052:refnum<vi>)
        n1189 = Unbundle By Name(w2026) -> ("Heave AND Surge.Distance"=w2049:refnum<vi>)
        n1190 = Unbundle By Name(w2026) -> ("Heave AND Surge.SPEED"=w2046:refnum<vi>)
        n1191 = Unbundle By Name(w2026) -> ("Platform Settings.Enable Platform"=w2060:refnum<vi>)
        n1192 = property class="DigNum (strict)"(reference=w2028, "Value"=u16 0) -> (reference out=w2027:refnum<vi>, error out=w2029:errorcluster)  [unwired: 1 in]
        n1193 = property class="DigNum (strict)"(reference=w2049, error in=w2044, "Value"=sgl 0.0) -> (reference out=w2050:refnum<vi>, error out=w2048:errorcluster)
        n1194 = property class="DigNum (strict)"(reference=w2046, error in=w2044, "Value"=sgl 0.0) -> (reference out=w2047:refnum<vi>, error out=w2045:errorcluster)
        n1195 = property class="DigNum (strict)"(reference=w2052, error in=w2044, "Value"=u8 1) -> (reference out=w2051:refnum<vi>, error out=w2053:errorcluster)
        n1196 = property class="Bool (strict)"(reference=w2060, "Value"=FALSE) -> (reference out=w2058:refnum<vi>, error out=w2059:errorcluster)  [unwired: 1 in]
        n1197 = Close Reference(reference=w2027, error in (no error)=w2029) -> (error out=w2025:errorcluster)
        n1198 = Close Reference(reference=w2050, error in (no error)=w2048) -> (error out=w2041:errorcluster)
        n1199 = Close Reference(reference=w2047, error in (no error)=w2045) -> (error out=w2040:errorcluster)
        n1200 = Close Reference(reference=w2051, error in (no error)=w2053) -> (error out=w2042:errorcluster)
        n1201 = Close Reference(reference=w2058, error in (no error)=w2059) -> ()  [unwired: 1 out]
        n1202 = Merge Errors(w2044, w2042, w2041, w2040, w2025) -> (w2043:errorcluster)
        n1203 = call "DATA ENCRYPT STRING FILE WRITE.vi"("error in (no error)"=w2043, "User Action"="User Pressed Enable Platform", "main ref"=w2026) -> ("error out"=w2055:errorcluster)  [unwired: 6 in, 1 out]
        n1204 = call "HEAVE WRITE FGV.vi"("Enum - Menu"=Heave_Write_enum."WRITE", "error in (no error)"=w2055, "main ref"=w2026) -> ("error out"=w2032:errorcluster)  [unwired: 7 in, 1 out]
        n1205 = Unbundle By Name(w2026) -> ("Heave AND Surge.Read Heave Temp"=w2036:refnum<vi>)
        n1206 = property class="Bool (strict)"(reference=w2036, error in=w2032, "Value"=TRUE) -> (reference out=w2034:refnum<vi>, error out=w2035:errorcluster)
        n1207 = Close Reference(reference=w2034, error in (no error)=w2035) -> (error out=w2031:errorcluster)
        "HEAVE ENABLE" <- TRUE ("HEAVE ENABLE")
      }
      frame "Heave Up main" {
        n1208 = Unbundle By Name(w2061) -> ("Platform Settings.Heave Up main"=w2071:refnum<vi>)
        n1209 = call "Heave Up Main.vi"("error in (no error)"=w2063, "main ref"=w2061) -> ("error out"=w2062:errorcluster)  [unwired: 9 in]
        n1210 = property class="Bool (strict)"(reference=w2071, "Value"=FALSE) -> (reference out=w2069:refnum<vi>, error out=w2070:errorcluster)  [unwired: 1 in]
        n1211 = Close Reference(reference=w2069, error in (no error)=w2070) -> ()  [unwired: 1 out]
        n1212 = call "DATA ENCRYPT STRING FILE WRITE.vi"("error in (no error)"=w2062, "User Action"="User Pressed Heave UP", "main ref"=w2061) -> ("error out"=w2066:errorcluster)  [unwired: 6 in, 1 out]
        n1213 = call "HEAVE WRITE FGV.vi"("Enum - Menu"=Heave_Write_enum."WRITE", "error in (no error)"=w2066, "main ref"=w2061) -> ("error out"=w2065:errorcluster)  [unwired: 7 in, 1 out]
      }
      frame "Heave Up MM" {
        n1214 = Unbundle By Name(w2072) -> ("Motion Module.Heave Up MM"=w2082:refnum<vi>)
        n1215 = call "Heave Up Motion Module.vi"("error in (no error)"=w2074, "main ref"=w2072) -> ("error out"=w2073:errorcluster)  [unwired: 9 in]
        n1216 = property class="Bool (strict)"(reference=w2082, "Value"=FALSE) -> (reference out=w2080:refnum<vi>, error out=w2081:errorcluster)  [unwired: 1 in]
        n1217 = Close Reference(reference=w2080, error in (no error)=w2081) -> ()  [unwired: 1 out]
        n1218 = call "DATA ENCRYPT STRING FILE WRITE.vi"("error in (no error)"=w2073, "User Action"="User Pressed Heave UP in Motion Module", "main ref"=w2072) -> ("error out"=w2077:errorcluster)  [unwired: 6 in, 1 out]
        n1219 = call "HEAVE WRITE FGV.vi"("Enum - Menu"=Heave_Write_enum."WRITE", "error in (no error)"=w2077, "main ref"=w2072) -> ("error out"=w2076:errorcluster)  [unwired: 7 in, 1 out]
      }
      frame "Heave Down Main" {
        n1220 = call "Heave Down Main.vi"("error in (no error)"=w2085, "main ref"=w2083) -> ("error out"=w2084:errorcluster)  [unwired: 9 in]
        n1221 = Unbundle By Name(w2083) -> ("Platform Settings.Heave Down Main"=w2093:refnum<vi>)
        n1222 = property class="Bool (strict)"(reference=w2093, "Value"=FALSE) -> (reference out=w2091:refnum<vi>, error out=w2092:errorcluster)  [unwired: 1 in]
        n1223 = Close Reference(reference=w2091, error in (no error)=w2092) -> ()  [unwired: 1 out]
        n1224 = call "DATA ENCRYPT STRING FILE WRITE.vi"("error in (no error)"=w2084, "User Action"="User Pressed Heave DOWN", "main ref"=w2083) -> ("error out"=w2088:errorcluster)  [unwired: 6 in, 1 out]
        n1225 = call "HEAVE WRITE FGV.vi"("Enum - Menu"=Heave_Write_enum."WRITE", "error in (no error)"=w2088, "main ref"=w2083) -> ("error out"=w2087:errorcluster)  [unwired: 7 in, 1 out]
      }
      frame "Heave Down MM" {
        n1226 = call "Heave Down Motion Module.vi"("error in (no error)"=w2096, "main ref"=w2094) -> ("error out"=w2095:errorcluster)  [unwired: 9 in]
        n1227 = Unbundle By Name(w2094) -> ("Motion Module.Heave Down MM"=w2104:refnum<vi>)
        n1228 = property class="Bool (strict)"(reference=w2104, "Value"=FALSE) -> (reference out=w2102:refnum<vi>, error out=w2103:errorcluster)  [unwired: 1 in]
        n1229 = Close Reference(reference=w2102, error in (no error)=w2103) -> ()  [unwired: 1 out]
        n1230 = call "DATA ENCRYPT STRING FILE WRITE.vi"("error in (no error)"=w2095, "User Action"="User Pressed Heave DOWN in Motion Module", "main ref"=w2094) -> ("error out"=w2099:errorcluster)  [unwired: 6 in, 1 out]
        n1231 = call "HEAVE WRITE FGV.vi"("Enum - Menu"=Heave_Write_enum."WRITE", "error in (no error)"=w2099, "main ref"=w2094) -> ("error out"=w2098:errorcluster)  [unwired: 7 in, 1 out]
      }
      frame "Surge Backward Main" {
        n1232 = Unbundle By Name(w2105) -> ("Platform Settings.Surge Backward Main"=w2115:refnum<vi>)
        n1233 = call "Surge Backward Main.vi"("error in (no error)"=w2107, "main ref"=w2105) -> ("error out"=w2106:errorcluster)  [unwired: 9 in]
        n1234 = property class="Bool (strict)"(reference=w2115, "Value"=FALSE) -> (reference out=w2113:refnum<vi>, error out=w2114:errorcluster)  [unwired: 1 in]
        n1235 = Close Reference(reference=w2113, error in (no error)=w2114) -> ()  [unwired: 1 out]
        n1236 = call "DATA ENCRYPT STRING FILE WRITE.vi"("error in (no error)"=w2106, "User Action"="User Pressed Surge Backward", "main ref"=w2105) -> ("error out"=w2110:errorcluster)  [unwired: 6 in, 1 out]
        n1237 = call "HEAVE WRITE FGV.vi"("Enum - Menu"=Heave_Write_enum."WRITE", "error in (no error)"=w2110, "main ref"=w2105) -> ("error out"=w2109:errorcluster)  [unwired: 7 in, 1 out]
      }
      frame "Surge Backward MM" {
        n1238 = Unbundle By Name(w2116) -> ("Motion Module.Surge Backward MM"=w2126:refnum<vi>)
        n1239 = call "Surge Backward MM.vi"("error in (no error)"=w2118, "main ref"=w2116) -> ("error out"=w2117:errorcluster)  [unwired: 9 in]
        n1240 = property class="Bool (strict)"(reference=w2126, "Value"=FALSE) -> (reference out=w2124:refnum<vi>, error out=w2125:errorcluster)  [unwired: 1 in]
        n1241 = Close Reference(reference=w2124, error in (no error)=w2125) -> ()  [unwired: 1 out]
        n1242 = call "DATA ENCRYPT STRING FILE WRITE.vi"("error in (no error)"=w2117, "User Action"="User Pressed Surge Backward in Motion Module", "main ref"=w2116) -> ("error out"=w2121:errorcluster)  [unwired: 6 in, 1 out]
        n1243 = call "HEAVE WRITE FGV.vi"("Enum - Menu"=Heave_Write_enum."WRITE", "error in (no error)"=w2121, "main ref"=w2116) -> ("error out"=w2120:errorcluster)  [unwired: 7 in, 1 out]
      }
      frame "Surge Forward Main" {
        n1244 = Unbundle By Name(w2127) -> ("Platform Settings.Surge Forward Main"=w2137:refnum<vi>)
        n1245 = call "Surge Forward Main.vi"("error in (no error)"=w2129, "main ref"=w2127) -> ("error out"=w2128:errorcluster)  [unwired: 9 in]
        n1246 = property class="Bool (strict)"(reference=w2137, "Value"=FALSE) -> (reference out=w2135:refnum<vi>, error out=w2136:errorcluster)  [unwired: 1 in]
        n1247 = Close Reference(reference=w2135, error in (no error)=w2136) -> ()  [unwired: 1 out]
        n1248 = call "DATA ENCRYPT STRING FILE WRITE.vi"("error in (no error)"=w2128, "User Action"="User Pressed Surge Forward", "main ref"=w2127) -> ("error out"=w2132:errorcluster)  [unwired: 6 in, 1 out]
        n1249 = call "HEAVE WRITE FGV.vi"("Enum - Menu"=Heave_Write_enum."WRITE", "error in (no error)"=w2132, "main ref"=w2127) -> ("error out"=w2131:errorcluster)  [unwired: 7 in, 1 out]
      }
      frame "Surge Forward MM" {
        n1250 = Unbundle By Name(w2138) -> ("Motion Module.Surge Forward MM"=w2148:refnum<vi>)
        n1251 = call "Surge Forward MM.vi"("error in (no error)"=w2140, "main ref"=w2138) -> ("error out"=w2139:errorcluster)  [unwired: 9 in]
        n1252 = property class="Bool (strict)"(reference=w2148, "Value"=FALSE) -> (reference out=w2146:refnum<vi>, error out=w2147:errorcluster)  [unwired: 1 in]
        n1253 = Close Reference(reference=w2146, error in (no error)=w2147) -> ()  [unwired: 1 out]
        n1254 = call "DATA ENCRYPT STRING FILE WRITE.vi"("error in (no error)"=w2139, "User Action"="User Pressed Surge Forward in Motion Module", "main ref"=w2138) -> ("error out"=w2143:errorcluster)  [unwired: 6 in, 1 out]
        n1255 = call "HEAVE WRITE FGV.vi"("Enum - Menu"=Heave_Write_enum."WRITE", "error in (no error)"=w2143, "main ref"=w2138) -> ("error out"=w2142:errorcluster)  [unwired: 7 in, 1 out]
      }
      frame "Sway Left Main" {
        n1256 = call "Sway Left Main.vi"("error in (no error)"=w2152, "main ref"=w2150) -> ("error out"=w2151:errorcluster)  [unwired: 9 in]
        n1257 = Unbundle By Name(w2150) -> ("Platform Settings.Sway Left Main"=w2159:refnum<vi>)
        n1258 = property class="Bool (strict)"(reference=w2159, "Value"=FALSE) -> (reference out=w2157:refnum<vi>, error out=w2158:errorcluster)  [unwired: 1 in]
        n1259 = Close Reference(reference=w2157, error in (no error)=w2158) -> ()  [unwired: 1 out]
        n1260 = call "DATA ENCRYPT STRING FILE WRITE.vi"("error in (no error)"=w2151, "User Action"="User Pressed Sway Left ", "main ref"=w2150) -> ("error out"=w2154:errorcluster)  [unwired: 6 in, 1 out]
        n1261 = call "SWAY WRITE FGV.vi"("Enum - Menu"=Sway_Write_enum."WRITE", "error in (no error)"=w2154, "main ref"=w2150) -> ("error out"=w2153:errorcluster)  [unwired: 8 in]
      }
      frame "Sway Left MM" {
        n1262 = call "Sway Left MM.vi"("error in (no error)"=w2163, "main ref"=w2161) -> ("error out"=w2162:errorcluster)  [unwired: 9 in]
        n1263 = Unbundle By Name(w2161) -> ("Motion Module.Sway Left MM"=w2170:refnum<vi>)
        n1264 = property class="Bool (strict)"(reference=w2170, "Value"=FALSE) -> (reference out=w2168:refnum<vi>, error out=w2169:errorcluster)  [unwired: 1 in]
        n1265 = Close Reference(reference=w2168, error in (no error)=w2169) -> ()  [unwired: 1 out]
        n1266 = call "DATA ENCRYPT STRING FILE WRITE.vi"("error in (no error)"=w2162, "User Action"="User Pressed Sway Left in MM", "main ref"=w2161) -> ("error out"=w2165:errorcluster)  [unwired: 6 in, 1 out]
        n1267 = call "SWAY WRITE FGV.vi"("Enum - Menu"=Sway_Write_enum."WRITE", "error in (no error)"=w2165, "main ref"=w2161) -> ("error out"=w2164:errorcluster)  [unwired: 8 in]
      }
      frame "Sway Right MM" {
        n1268 = call "Sway Right MM.vi"("error in (no error)"=w2174, "main ref"=w2172) -> ("error out"=w2173:errorcluster)  [unwired: 9 in]
        n1269 = Unbundle By Name(w2172) -> ("Motion Module.Sway Right MM"=w2181:refnum<vi>)
        n1270 = property class="Bool (strict)"(reference=w2181, "Value"=FALSE) -> (reference out=w2179:refnum<vi>, error out=w2180:errorcluster)  [unwired: 1 in]
        n1271 = Close Reference(reference=w2179, error in (no error)=w2180) -> ()  [unwired: 1 out]
        n1272 = call "DATA ENCRYPT STRING FILE WRITE.vi"("error in (no error)"=w2173, "User Action"="User Pressed Sway Right in MM", "main ref"=w2172) -> ("error out"=w2176:errorcluster)  [unwired: 6 in, 1 out]
        n1273 = call "SWAY WRITE FGV.vi"("Enum - Menu"=Sway_Write_enum."WRITE", "error in (no error)"=w2176, "main ref"=w2172) -> ("error out"=w2175:errorcluster)  [unwired: 8 in]
      }
      frame "Sway Right Main" {
        n1274 = call "Sway Right Main.vi"("error in (no error)"=w2185, "main ref"=w2183) -> ("error out"=w2184:errorcluster)  [unwired: 9 in]
        n1275 = Unbundle By Name(w2183) -> ("Platform Settings.Sway Right Main"=w2192:refnum<vi>)
        n1276 = property class="Bool (strict)"(reference=w2192, "Value"=FALSE) -> (reference out=w2190:refnum<vi>, error out=w2191:errorcluster)  [unwired: 1 in]
        n1277 = Close Reference(reference=w2190, error in (no error)=w2191) -> ()  [unwired: 1 out]
        n1278 = call "DATA ENCRYPT STRING FILE WRITE.vi"("error in (no error)"=w2184, "User Action"="User Pressed Sway Right", "main ref"=w2183) -> ("error out"=w2187:errorcluster)  [unwired: 6 in, 1 out]
        n1279 = call "SWAY WRITE FGV.vi"("Enum - Menu"=Sway_Write_enum."WRITE", "error in (no error)"=w2187, "main ref"=w2183) -> ("error out"=w2186:errorcluster)  [unwired: 8 in]
      }
      frame "Manual Write Heave & Surge" {
        n1280 = Unbundle By Name(w2193) -> ("Heave AND Surge.Manual Write"=w2202:refnum<vi>)
        n1281 = property class="Bool (strict)"(reference=w2202, "Value"=FALSE) -> (reference out=w2200:refnum<vi>, error out=w2201:errorcluster)  [unwired: 1 in]
        n1282 = Close Reference(reference=w2200, error in (no error)=w2201) -> ()  [unwired: 1 out]
        n1283 = call "DATA ENCRYPT STRING FILE WRITE.vi"("error in (no error)"=w2194, "User Action"="User Pressed Manual Write Heave and Surge", "main ref"=w2193) -> ("error out"=w2197:errorcluster)  [unwired: 6 in, 1 out]
        n1284 = call "HEAVE WRITE FGV.vi"("Enum - Menu"=Heave_Write_enum."WRITE", "error in (no error)"=w2197, "main ref"=w2193) -> ("error out"=w2196:errorcluster)  [unwired: 7 in, 1 out]
      }
      frame "Manual Write SWAY" {
        n1285 = Unbundle By Name(w2204) -> ("SWAY.Manual Write SWAY"=w2212:refnum<vi>)
        n1286 = property class="Bool (strict)"(reference=w2212, "Value"=FALSE) -> (reference out=w2210:refnum<vi>, error out=w2211:errorcluster)  [unwired: 1 in]
        n1287 = Close Reference(reference=w2210, error in (no error)=w2211) -> ()  [unwired: 1 out]
        n1288 = call "DATA ENCRYPT STRING FILE WRITE.vi"("error in (no error)"=w2205, "User Action"="User Pressed Manual Write Sway", "main ref"=w2204) -> ("error out"=w2207:errorcluster)  [unwired: 6 in, 1 out]
        n1289 = call "SWAY WRITE FGV.vi"("Enum - Menu"=Sway_Write_enum."WRITE", "error in (no error)"=w2207, "main ref"=w2204) -> ("error out"=w2206:errorcluster)  [unwired: 8 in]
      }
      frame "Load En" {
        # "zNL 2"
        n1290 = Unbundle By Name(w2214) -> ("Main Screen.Load En"=w2219:refnum<vi>)
        n1291 = property class="Bool (strict)"(reference=w2219) -> (reference out=w2217:refnum<vi>, error out=w2218:errorcluster, "Value"=w2213:bool)  [unwired: 1 in]
        n1292 = Close Reference(reference=w2217, error in (no error)=w2218) -> ()  [unwired: 1 out]
        n1293 = case shown="False" w2213 {
          tunnel: [w2231 w2241] -> w2215
          tunnel: w2216 -> [w2233 w2240]
          tunnel: w2214 -> [w2221 w2235]
          tunnel: w2214 -> [w2229 _]
          tunnel: w2214 -> [w2228 _]
          frame False {
            n1294 = call "DATA ENCRYPT STRING FILE WRITE.vi"("error in (no error)"=w2233, "User Action"="User Pressed UnLoad on Main Screen", "main ref"=w2221) -> ("error out"=w2222:errorcluster)  [unwired: 6 in, 1 out]
            n1295 = call "Stall Data Flow.vim"("value in"=w2222, "milliseconds to wait"=u32 2000) -> ("value out"=w2227:errorcluster)  [unwired: 1 out]
            n1296 = Unbundle By Name(w2221) -> ("Main Screen.zNL 2"=w2225:refnum<vi>)
            n1297 = property class="Bool (strict)"(reference=w2225, "DisabledEnum"=T16."Enabled" ("Disabled")) -> (reference out=w2223:refnum<vi>, error out=w2224:errorcluster)  [unwired: 1 in]
            n1298 = call "PID UNLOAD.vi"("error in (no error)"=w2227, "main ref"=w2228) -> ("error out"=w2230:errorcluster)  [unwired: 9 in]
            n1299 = Close Reference(reference=w2223, error in (no error)=w2224) -> ()  [unwired: 1 out]
            n1300 = call "HEAVE WRITE FGV.vi"("Enum - Menu"=Heave_Write_enum."WRITE", "error in (no error)"=w2230, "main ref"=w2229) -> ("error out"=w2231:errorcluster)  [unwired: 7 in, 1 out]
          }
          frame True {
            n1301 = call "DATA ENCRYPT STRING FILE WRITE.vi"("error in (no error)"=w2240, "User Action"="User Pressed Load on Main Screen", "main ref"=w2235) -> ("error out"=w2241:errorcluster)  [unwired: 6 in, 1 out]
            n1302 = Unbundle By Name(w2235) -> ("Main Screen.zNL 2"=w2239:refnum<vi>)
            n1303 = property class="Bool (strict)"(reference=w2239, "DisabledEnum"=T16."Disabled and Grayed Out" ("Disabled")) -> (reference out=w2237:refnum<vi>, error out=w2238:errorcluster)  [unwired: 1 in]
            n1304 = Close Reference(reference=w2237, error in (no error)=w2238) -> ()  [unwired: 1 out]
          }
        }
      }
      frame "apply load" {
        n1305 = Unbundle By Name(w2244) -> ("Main Screen.Load En"=w2249:refnum<vi>)
        n1306 = property class="Bool (strict)"(reference=w2249) -> (reference out=w2247:refnum<vi>, error out=w2248:errorcluster, "Value"=w2243:bool)  [unwired: 1 in]
        n1307 = Close Reference(reference=w2247, error in (no error)=w2248) -> ()  [unwired: 1 out]
        n1308 = case shown="False" w2243 {
          tunnel: [w2256 w2263] -> w2245
          tunnel: w2246 -> [w2259 w2262]
          tunnel: w2244 -> [w2258 w2261]
          tunnel: w2244 -> [w2253 _]
          tunnel: w2244 -> [w2252 _]
          frame False {
            n1309 = call "DATA ENCRYPT STRING FILE WRITE.vi"("error in (no error)"=w2259, "User Action"="User Pressed UnLoad on Service Screen", "main ref"=w2258) -> ("error out"=w2255:errorcluster)  [unwired: 6 in, 1 out]
            n1310 = call "Stall Data Flow.vim"("value in"=w2255, "milliseconds to wait"=u32 2000) -> ("value out"=w2251:errorcluster)  [unwired: 1 out]
            n1311 = call "PID UNLOAD.vi"("error in (no error)"=w2251, "main ref"=w2252) -> ("error out"=w2254:errorcluster)  [unwired: 9 in]
            n1312 = call "HEAVE WRITE FGV.vi"("Enum - Menu"=Heave_Write_enum."WRITE", "error in (no error)"=w2254, "main ref"=w2253) -> ("error out"=w2256:errorcluster)  [unwired: 7 in, 1 out]
          }
          frame True {
            n1313 = call "DATA ENCRYPT STRING FILE WRITE.vi"("error in (no error)"=w2262, "User Action"="User Pressed Load on Service Screen", "main ref"=w2261) -> ("error out"=w2263:errorcluster)  [unwired: 6 in, 1 out]
          }
        }
      }
      frame "BACK" {
        w2270 = FALSE ("Value")
        n1314 = Unbundle By Name(w2265) -> ("Main Screen.BACK"=w2290:refnum<vi>)
        n1315 = property class="Bool (strict)"(reference=w2290, "Value"=FALSE) -> (reference out=w2288:refnum<vi>, error out=w2289:errorcluster)  [unwired: 1 in]
        n1316 = Close Reference(reference=w2288, error in (no error)=w2289) -> ()  [unwired: 1 out]
        n1317 = call "DATA ENCRYPT STRING FILE WRITE.vi"("error in (no error)"=w2287, "User Action"="User Pressed Back on Main Screen", "main ref"=w2265) -> ("error out"=w2285:errorcluster)  [unwired: 6 in, 1 out]
        n1318 = Unbundle By Name(w2265) -> ("Main Home Screen.MainPage"=w2277:refnum<vi>)
        n1319 = Unbundle By Name(w2265) -> ("Main Screen.Start Test"=w2273:refnum<vi>)
        n1320 = Unbundle By Name(w2265) -> ("Main Screen.STOP"=w2272:refnum<vi>)
        n1321 = Unbundle By Name(w2265) -> ("Main Home Screen.GUI"=w2281:refnum<vi>)
        n1322 = property class="TabCtl (strict)"(reference=w2277, "Value"=T5."HOME") -> (reference out=w2279:refnum<vi>, error out=w2278:errorcluster)  [unwired: 1 in]
        n1323 = property class="TabCtl (strict)"(reference=w2281, "Value"=T4."Setup") -> (reference out=w2283:refnum<vi>, error out=w2282:errorcluster)  [unwired: 1 in]
        n1324 = property class="Bool (strict)"(reference=w2273, "Visible"=TRUE ("Value"), "Value"=FALSE) -> (reference out=w2268:refnum<vi>, error out=w2274:errorcluster)  [unwired: 1 in]
        n1325 = property class="Bool (strict)"(reference=w2272, "Value"=w2270, "Visible"=w2270) -> (reference out=w2267:refnum<vi>, error out=w2271:errorcluster)  [unwired: 1 in]
        n1326 = Close Reference(reference=w2283, error in (no error)=w2282) -> ()  [unwired: 1 out]
        n1327 = Close Reference(reference=w2279, error in (no error)=w2278) -> ()  [unwired: 1 out]
        n1328 = Close Reference(reference=w2268, error in (no error)=w2274) -> ()  [unwired: 1 out]
        n1329 = Close Reference(reference=w2267, error in (no error)=w2271) -> ()  [unwired: 1 out]
        n1330 = call "Reinitial Parameter After Test.vi"("error in (no error)"=w2285, "main ref"=w2265) -> ("error out"=w2266:errorcluster)  [unwired: 9 in]
      }
      frame "Start Test" {
        n1331 = call "Test Start Sequence.vi"("error in (no error)"=w2293, "Data Cluster"=w2291) -> ("error out"=w2292:errorcluster)  [unwired: 9 in]
      }
      frame "STOP" {
        n1332 = Unbundle By Name(w2295) -> ("Main Screen.Load En"=w2308:refnum<vi>)
        n1333 = Unbundle By Name(w2295) -> ("Main Screen.CZ FF"=w2303:refnum<vi>)
        n1334 = Unbundle By Name(w2295) -> ("Main Screen.zFF"=w2300:refnum<vi>)
        n1335 = property class="Bool (strict)"(reference=w2308, "DisabledEnum"=T16."Disabled and Grayed Out" ("Disabled")) -> (reference out=w2296:refnum<vi>, error out=w2307:errorcluster)  [unwired: 1 in]
        n1336 = property class="Bool (strict)"(reference=w2303, "DisabledEnum"=T16."Disabled and Grayed Out" ("Disabled"), "Value"=FALSE ("Visible")) -> (reference out=w2302:refnum<vi>, error out=w2304:errorcluster)  [unwired: 1 in]
        n1337 = property class="Bool (strict)"(reference=w2300, "DisabledEnum"=T16."Disabled and Grayed Out" ("Disabled"), "Value"=FALSE ("Visible")) -> (reference out=w2301:refnum<vi>, error out=w2299:errorcluster)  [unwired: 1 in]
        n1338 = Close Reference(reference=w2296, error in (no error)=w2307) -> ()  [unwired: 1 out]
        n1339 = Close Reference(reference=w2302, error in (no error)=w2304) -> ()  [unwired: 1 out]
        n1340 = Close Reference(reference=w2301, error in (no error)=w2299) -> ()  [unwired: 1 out]
        n1341 = call "Test Stop.vi"("error in (no error)"=w2309, "Data Cluster"=w2295) -> ("error out"=w2310:errorcluster)  [unwired: 9 in]
      }
      frame "PlaceModule" {
        n1342 = call "Place Module.vi"("error in (no error)"=w2313, "main ref"=w2311) -> ("error out"=w2312:errorcluster)  [unwired: 9 in]
      }
      frame "Stage Homing" {
        n1343 = call "HOMINING.vi"("error in (no error)"=w2316, "main ref"=w2314) -> ("error out"=w2315:errorcluster)  [unwired: 9 in]
      }
      frame "Clear 3" {
        n1344 = Unbundle By Name(w2318) -> ("Loading.Stribeck Table  For loading"=w2328:refnum<vi>)
        n1345 = Unbundle By Name(w2318) -> ("Loading.Clear 3"=w2319:refnum<vi>)
        n1346 = property class="Bool (strict)"(reference=w2319, "Value"=FALSE) -> (reference out=w2321:refnum<vi>, error out=w2320:errorcluster)  [unwired: 1 in]
        n1347 = call "DATA ENCRYPT STRING FILE WRITE.vi"("error in (no error)"=w2324, "User Action"="User Pressed Clear  on Step Load Sequence", "main ref"=w2318) -> ("error out"=w2323:errorcluster)  [unwired: 6 in, 1 out]
        n1348 = property class="Tbl (strict)"(reference=w2328, "Value"=string[][] []) -> (reference out=w2326:refnum<vi>, error out=w2327:errorcluster)  [unwired: 1 in]
        n1349 = Close Reference(reference=w2321, error in (no error)=w2320) -> ()  [unwired: 1 out]
        n1350 = Close Reference(reference=w2326, error in (no error)=w2327) -> ()  [unwired: 1 out]
      }
      frame "Set WTD" {
        n1351 = Unbundle By Name(w2329) -> ("Motion Module.Set WTD"=w2332:refnum<vi>)
        n1352 = property class="Bool (strict)"(reference=w2332, "Value"=FALSE) -> (reference out=w2334:refnum<vi>, error out=w2333:errorcluster)  [unwired: 1 in]
        n1353 = call "DATA ENCRYPT STRING FILE WRITE.vi"("error in (no error)"=w2336, "User Action"="User Pressed  on Set Wear Track", "main ref"=w2329) -> ("error out"=w2335:errorcluster)  [unwired: 6 in, 1 out]
        n1354 = call "Sway wear trac set.vi"("error in (no error)"=w2335, "main ref"=w2329) -> ("error out"=w2330:errorcluster)  [unwired: 9 in]
        n1355 = Close Reference(reference=w2334, error in (no error)=w2333) -> ()  [unwired: 1 out]
      }
      frame "Import 2" {
        n1356 = call "File Dialog"("start path"=path "C:/LAB-IQ 150/User Defined Protocol", "error in"=w2345) -> ("selected path"=w2339:path, "cancelled"=w2342:bool, "error out"=w2344:errorcluster)  [unwired: 10 in, 1 out]
        n1357 = call <vilib>:"Clear Errors.vi"("error in (no error)"=w2344) -> ("error out"=w2341:errorcluster)  [unwired: 5 in, 1 out]
        n1358 = case shown="False" w2342 {
          tunnel: w2341 -> [w2355 w2356]
          tunnel: [w2347 w2356] -> w2340
          tunnel: w2339 -> [w2354 _]
          tunnel: w2338 -> [w2349 _]
          frame False {
            n1359 = call-poly <vilib>:"Read Delimited Spreadsheet.vi"("file path (dialog if empty)"=w2354, "error in (no error)"=w2355, "delimiter (\\t)"=":" ("delimiter (\\t)")) -> ("all rows"=w2346:string[][], "error out"=w2348:errorcluster)  [unwired: 7 in, 4 out]
            n1360 = Unbundle By Name(w2349) -> ("Motion Module.StepTable For Speed"=w2352:refnum<vi>)
            n1361 = property class="Tbl (strict)"(reference=w2352, error in=w2348, "Value"=w2346) -> (reference out=w2350:refnum<vi>, error out=w2351:errorcluster)
            n1362 = Close Reference(reference=w2350, error in (no error)=w2351) -> (error out=w2347:errorcluster)
          }
          frame True {
          }
        }
      }
      frame "Save 2" {
        n1363 = Unbundle By Name(w2360) -> ("Motion Module.StepTable For Speed"=w2375:refnum<vi>)
        n1364 = property class="Tbl (strict)"(reference=w2375) -> (reference out=w2373:refnum<vi>, error out=w2374:errorcluster, "Value"=w2371:string[][])  [unwired: 1 in]
        n1365 = call "File Dialog2"("start path"=path "C:/LAB-IQ 150/User Defined Protocol", "error in"=w2365) -> ("selected path"=w2368:path, "error out"=w2367:errorcluster)  [unwired: 10 in, 2 out]
        n1366 = call <vilib>:"Clear Errors.vi"("error in (no error)"=w2367) -> ("error out"=w2366:errorcluster)  [unwired: 5 in, 1 out]
        n1367 = Close Reference(reference=w2373, error in (no error)=w2374) -> ()  [unwired: 1 out]
        n1368 = call-poly <vilib>:"Write Delimited Spreadsheet.vi"("file path (dialog if empty)"=w2368, "2D data"=w2371, "append to file? (new file:F)"=TRUE, "error in (no error)"=w2366, "delimiter (\\t)"=":" ("delimiter (\\t)")) -> ("error out"=w2364:errorcluster)  [unwired: 9 in, 1 out]
        n1369 = call <vilib>:"Clear Errors.vi"("error in (no error)"=w2364) -> ("error out"=w2359:errorcluster)  [unwired: 5 in, 1 out]
        n1370 = Unbundle By Name(w2360) -> ("Motion Module.Save 2"=w2361:refnum<vi>)
        n1371 = property class="Bool (strict)"(reference=w2361, error in=w2359, "Value"=FALSE) -> (reference out=w2363:refnum<vi>, error out=w2362:errorcluster)
        n1372 = Close Reference(reference=w2363, error in (no error)=w2362) -> (error out=w2358:errorcluster)
      }
      frame "Calculate Rotary" {
        n1373 = call "STEP LOAD MM_SEC AND RPM CONVERSION.vi"("error in (no error)"=w2379, "Data Cluster"=w2377) -> ("error out"=w2378:errorcluster)  [unwired: 9 in]
        n1374 = local write "calculate rotary"(FALSE) -> ()
      }
      frame "Clear List" {
        n1375 = Unbundle By Name(w2381) -> ("Environmental control.Sensors Picked"=w2388:refnum<vi>)
        n1376 = Unbundle By Name(w2381) -> ("Environmental control.Clear List"=w2382:refnum<vi>)
        n1377 = property class="Bool (strict)"(reference=w2382, "Value"=FALSE) -> (reference out=w2384:refnum<vi>, error out=w2383:errorcluster)  [unwired: 1 in]
        n1378 = property class="Str"(reference=w2388, "Value"="") -> (reference out=w2386:refnum<vi>, error out=w2387:errorcluster)  [unwired: 1 in]
        n1379 = Close Reference(reference=w2384, error in (no error)=w2383) -> ()  [unwired: 1 out]
        n1380 = Close Reference(reference=w2386, error in (no error)=w2387) -> ()  [unwired: 1 out]
      }
      frame "ClrLog" {
        n1381 = Unbundle By Name(w2391) -> ("Main Screen.ClrLog"=w2392:refnum<vi>)
        n1382 = Unbundle By Name(w2391) -> ("Main Screen.Trip Log"=w2398:refnum<vi>)
        n1383 = property class="Bool (strict)"(reference=w2392, "Value"=FALSE) -> (reference out=w2394:refnum<vi>, error out=w2393:errorcluster)  [unwired: 1 in]
        n1384 = property class="Str"(reference=w2398, "Value"="") -> (reference out=w2396:refnum<vi>, error out=w2397:errorcluster)  [unwired: 1 in]
        n1385 = Close Reference(reference=w2394, error in (no error)=w2393) -> ()  [unwired: 1 out]
        n1386 = Close Reference(reference=w2396, error in (no error)=w2397) -> ()  [unwired: 1 out]
      }
      frame "Add to list" {
        n1387 = Unbundle By Name(w2400) -> ("Environmental control.Sensors Picked"=w2406:refnum<vi>)
        n1388 = property class="Str"(reference=w2406, error in=w2401, "Value"="") -> (reference out=w2404:refnum<vi>, error out=w2405:errorcluster)
        n1389 = Close Reference(reference=w2404, error in (no error)=w2405) -> (error out=w2402:errorcluster)
        n1390 = call "Add  to List Loop.vi"("error in (no error)"=w2402, "Data Cluster"=w2400) -> ("error out"=w2408:errorcluster)  [unwired: 9 in]
        n1391 = Unbundle By Name(w2400) -> ("Environmental control.Add to list"=w2410:refnum<vi>)
        n1392 = property class="Bool (strict)"(reference=w2410, error in=w2408, "Value"=FALSE) -> (reference out=w2412:refnum<vi>, error out=w2411:errorcluster)
        n1393 = Close Reference(reference=w2412, error in (no error)=w2411) -> (error out=w2407:errorcluster)
      }
      frame "Disable Axis Jog Soft Limits" {
        n1394 = call "DATA ENCRYPT STRING FILE WRITE.vi"("error in (no error)"=w2416, "User Action"="User Pressed Disable Axis Jog Soft Limits in Main Screen", "main ref"=w2414) -> ("error out"=w2415:errorcluster)  [unwired: 6 in, 1 out]
      }
      frame "Home Service" {
        n1395 = Unbundle By Name(w2418) -> ("Main Home Screen.MainPage"=w2424:refnum<vi>)
        n1396 = Unbundle By Name(w2418) -> ("Main Home Screen.GUI"=w2422:refnum<vi>)
        n1397 = local write "Home Service"(FALSE ("Home Service")) -> ()
        n1398 = property class="TabCtl (strict)"(reference=w2424, "Value"=T5."HOME") -> (reference out=w2426:refnum<vi>, error out=w2425:errorcluster)  [unwired: 1 in]
        n1399 = property class="TabCtl (strict)"(reference=w2422, "Value"=T4."Setup") -> (reference out=w2420:refnum<vi>, error out=w2421:errorcluster)  [unwired: 1 in]
        n1400 = Close Reference(reference=w2426, error in (no error)=w2425) -> ()  [unwired: 1 out]
        n1401 = Close Reference(reference=w2420, error in (no error)=w2421) -> ()  [unwired: 1 out]
        n1402 = call "DATA ENCRYPT STRING FILE WRITE.vi"("error in (no error)"=w2429, "User Action"="User Pressed Home Service from Service Screen", "main ref"=w2418) -> ("error out"=w2428:errorcluster)  [unwired: 6 in, 1 out]
      }
      frame "Analysis Home" {
        n1403 = Unbundle By Name(w2431) -> ("Main Screen.Main Screen Tab"=w2434:refnum<vi>)
        n1404 = Unbundle By Name(w2431) -> ("Main Home Screen.MainPage"=w2441:refnum<vi>)
        n1405 = Unbundle By Name(w2431) -> ("Main Home Screen.GUI"=w2439:refnum<vi>)
        n1406 = local write "Analysis Home new"(FALSE ("Analysis Home new")) -> ()
        n1407 = property class="TabCtl (strict)"(reference=w2434, "Value"=T8."  Acquire  ") -> (reference out=w2432:refnum<vi>, error out=w2433:errorcluster)  [unwired: 1 in]
        n1408 = property class="TabCtl (strict)"(reference=w2441, "Value"=T5."HOME") -> (reference out=w2443:refnum<vi>, error out=w2442:errorcluster)  [unwired: 1 in]
        n1409 = property class="TabCtl (strict)"(reference=w2439, "Value"=T4."Setup") -> (reference out=w2437:refnum<vi>, error out=w2438:errorcluster)  [unwired: 1 in]
        n1410 = Close Reference(reference=w2432, error in (no error)=w2433) -> ()  [unwired: 1 out]
        n1411 = Close Reference(reference=w2443, error in (no error)=w2442) -> ()  [unwired: 1 out]
        n1412 = Close Reference(reference=w2437, error in (no error)=w2438) -> ()  [unwired: 1 out]
        n1413 = call "DATA ENCRYPT STRING FILE WRITE.vi"("error in (no error)"=w2446, "User Action"="User Pressed Home from AnalysisScreen", "main ref"=w2431) -> ("error out"=w2445:errorcluster)  [unwired: 6 in, 1 out]
      }
      frame "Post Analysis" {
        n1414 = Unbundle By Name(w2449) -> ("Main Screen.Main Screen Tab"=w2452:refnum<vi>)
        n1415 = Unbundle By Name(w2449) -> ("Main Home Screen.MainPage"=w2458:refnum<vi>)
        n1416 = Unbundle By Name(w2449) -> ("Main Home Screen.GUI"=w2456:refnum<vi>)
        n1417 = property class="TabCtl (strict)"(reference=w2452, "Value"=T8."Compare Files Rot") -> (reference out=w2450:refnum<vi>, error out=w2451:errorcluster)  [unwired: 1 in]
        n1418 = property class="TabCtl (strict)"(reference=w2458, "Value"=T5."HOME") -> (reference out=w2460:refnum<vi>, error out=w2459:errorcluster)  [unwired: 1 in]
        n1419 = property class="TabCtl (strict)"(reference=w2456, "Value"=T4."Begin") -> (reference out=w2454:refnum<vi>, error out=w2455:errorcluster)  [unwired: 1 in]
        n1420 = local write "Post Analysis"(FALSE ("Post Analysis")) -> ()
        n1421 = Close Reference(reference=w2450, error in (no error)=w2451) -> ()  [unwired: 1 out]
        n1422 = Close Reference(reference=w2460, error in (no error)=w2459) -> ()  [unwired: 1 out]
        n1423 = Close Reference(reference=w2454, error in (no error)=w2455) -> ()  [unwired: 1 out]
        n1424 = call "DATA ENCRYPT STRING FILE WRITE.vi"("error in (no error)"=w2463, "User Action"="User Pressed Post Analysis ", "main ref"=w2449) -> ("error out"=w2462:errorcluster)  [unwired: 6 in, 1 out]
      }
      frame "Edit Gain Constants" {
        n1425 = Unbundle By Name(w2465) -> ("About Screen.Heave and Surge COM Port:"=w2495:refnum<vi>)
        n1426 = Unbundle By Name(w2465) -> ("About Screen.Edit Gain Constants"=w2475:refnum<vi>)
        n1427 = Unbundle By Name(w2465) -> ("About Screen.Sway COM Port:"=w2492:refnum<vi>)
        n1428 = Unbundle By Name(w2465) -> ("About Screen.Ramp Port:"=w2469:refnum<vi>)
        n1429 = Unbundle By Name(w2465) -> ("About Screen.Temp Modbus:"=w2489:refnum<vi>)
        n1430 = Unbundle By Name(w2465) -> ("About Screen.Humidity Port:"=w2488:refnum<vi>)
        n1431 = Unbundle By Name(w2465) -> ("About Screen.Password"=w2483:refnum<vi>)
        n1432 = Unbundle By Name(w2465) -> ("About Screen.ECR Port:"=w2468:refnum<vi>)
        n1433 = property class="VISAName"(reference=w2469, "DisabledEnum"=T16."Enabled" ("Disabled")) -> (reference out=w2471:refnum<vi>, error out=w2470:errorcluster)  [unwired: 1 in]
        n1434 = property class="Bool (strict)"(reference=w2475, "Value"=FALSE) -> (reference out=w2476:refnum<vi>, error out=w2474:errorcluster)  [unwired: 1 in]
        n1435 = property class="VISAName"(reference=w2468, "DisabledEnum"=T16."Enabled" ("Disabled")) -> (reference out=w2464:refnum<vi>, error out=w2467:errorcluster)  [unwired: 1 in]
        n1436 = property class="VISAName"(reference=w2495, "DisabledEnum"=T16."Enabled" ("Disabled")) -> (reference out=w2496:refnum<vi>, error out=w2494:errorcluster)  [unwired: 1 in]
        n1437 = property class="VISAName"(reference=w2492, "DisabledEnum"=T16."Enabled" ("Disabled")) -> (reference out=w2493:refnum<vi>, error out=w2491:errorcluster)  [unwired: 1 in]
        n1438 = property class="VISAName"(reference=w2489, "DisabledEnum"=T16."Enabled" ("Disabled")) -> (reference out=w2477:refnum<vi>, error out=w2490:errorcluster)  [unwired: 1 in]
        n1439 = property class="VISAName"(reference=w2488, "DisabledEnum"=T16."Enabled" ("Disabled")) -> (reference out=w2486:refnum<vi>, error out=w2487:errorcluster)  [unwired: 1 in]
        n1440 = property class="Str"(reference=w2483, "Visible"=FALSE) -> (reference out=w2485:refnum<vi>, error out=w2484:errorcluster)  [unwired: 1 in]
        n1441 = Close Reference(reference=w2471, error in (no error)=w2470) -> ()  [unwired: 1 out]
        n1442 = Close Reference(reference=w2485, error in (no error)=w2484) -> ()  [unwired: 1 out]
        n1443 = Close Reference(reference=w2464, error in (no error)=w2467) -> ()  [unwired: 1 out]
        n1444 = Close Reference(reference=w2476, error in (no error)=w2474) -> ()  [unwired: 1 out]
        n1445 = Close Reference(reference=w2496, error in (no error)=w2494) -> ()  [unwired: 1 out]
        n1446 = Close Reference(reference=w2493, error in (no error)=w2491) -> ()  [unwired: 1 out]
        n1447 = Close Reference(reference=w2477, error in (no error)=w2490) -> ()  [unwired: 1 out]
        n1448 = Close Reference(reference=w2486, error in (no error)=w2487) -> ()  [unwired: 1 out]
        n1449 = call "DATA ENCRYPT STRING FILE WRITE.vi"("error in (no error)"=w2499, "User Action"="User Pressed Home Service from Service Screen", "main ref"=w2465) -> ("error out"=w2498:errorcluster)  [unwired: 6 in, 1 out]
      }
      frame "Advanced Setting" {
        n1450 = Unbundle By Name(w2501) -> ("About Screen.Advanced Setting"=w2503:refnum<vi>)
        n1451 = property class="Bool (strict)"(reference=w2503) -> (reference out=w2504:refnum<vi>, error out=w2502:errorcluster, "Value"=w2500:bool)  [unwired: 1 in]
        n1452 = Close Reference(reference=w2504, error in (no error)=w2502) -> ()  [unwired: 1 out]
        n1453 = case shown="True" w2500 {
          tunnel: w2501 -> [w2509 w2534]
          frame True {
            n1454 = Unbundle By Name(w2509) -> ("About Screen.Heave and Surge COM Port:"=w2531:refnum<vi>)
            n1455 = Unbundle By Name(w2509) -> ("About Screen.Edit Gain Constants"=w2511:refnum<vi>)
            n1456 = Unbundle By Name(w2509) -> ("About Screen.Sway COM Port:"=w2528:refnum<vi>)
            n1457 = Unbundle By Name(w2509) -> ("About Screen.Temp Modbus:"=w2525:refnum<vi>)
            n1458 = Unbundle By Name(w2509) -> ("About Screen.Humidity Port:"=w2524:refnum<vi>)
            n1459 = Unbundle By Name(w2509) -> ("About Screen.Password"=w2519:refnum<vi>)
            n1460 = property class="Bool (strict)"(reference=w2511, "Value"=FALSE) -> (reference out=w2512:refnum<vi>, error out=w2510:errorcluster)  [unwired: 1 in]
            n1461 = property class="VISAName"(reference=w2531, "DisabledEnum"=T16."Disabled and Grayed Out" ("Disabled")) -> (reference out=w2532:refnum<vi>, error out=w2530:errorcluster)  [unwired: 1 in]
            n1462 = property class="VISAName"(reference=w2528, "DisabledEnum"=T16."Disabled and Grayed Out" ("Disabled")) -> (reference out=w2529:refnum<vi>, error out=w2527:errorcluster)  [unwired: 1 in]
            n1463 = property class="VISAName"(reference=w2525, "DisabledEnum"=T16."Disabled and Grayed Out" ("Disabled")) -> (reference out=w2513:refnum<vi>, error out=w2526:errorcluster)  [unwired: 1 in]
            n1464 = property class="VISAName"(reference=w2524, "DisabledEnum"=T16."Disabled and Grayed Out" ("Disabled")) -> (reference out=w2522:refnum<vi>, error out=w2523:errorcluster)  [unwired: 1 in]
            n1465 = property class="Str"(reference=w2519, "Visible"=TRUE) -> (reference out=w2521:refnum<vi>, error out=w2520:errorcluster)  [unwired: 1 in]
            n1466 = Close Reference(reference=w2512, error in (no error)=w2510) -> ()  [unwired: 1 out]
            n1467 = Close Reference(reference=w2532, error in (no error)=w2530) -> ()  [unwired: 1 out]
            n1468 = Close Reference(reference=w2529, error in (no error)=w2527) -> ()  [unwired: 1 out]
            n1469 = Close Reference(reference=w2513, error in (no error)=w2526) -> ()  [unwired: 1 out]
            n1470 = Close Reference(reference=w2522, error in (no error)=w2523) -> ()  [unwired: 1 out]
            n1471 = Close Reference(reference=w2521, error in (no error)=w2520) -> ()  [unwired: 1 out]
          }
          frame False {
            n1472 = Unbundle By Name(w2534) -> ("About Screen.Heave and Surge COM Port:"=w2556:refnum<vi>)
            n1473 = Unbundle By Name(w2534) -> ("About Screen.Edit Gain Constants"=w2536:refnum<vi>)
            n1474 = Unbundle By Name(w2534) -> ("About Screen.Sway COM Port:"=w2553:refnum<vi>)
            n1475 = Unbundle By Name(w2534) -> ("About Screen.Temp Modbus:"=w2550:refnum<vi>)
            n1476 = Unbundle By Name(w2534) -> ("About Screen.Humidity Port:"=w2549:refnum<vi>)
            n1477 = Unbundle By Name(w2534) -> ("About Screen.Password"=w2544:refnum<vi>)
            n1478 = property class="Bool (strict)"(reference=w2536, "Value"=FALSE) -> (reference out=w2537:refnum<vi>, error out=w2535:errorcluster)  [unwired: 1 in]
            n1479 = property class="VISAName"(reference=w2556, "DisabledEnum"=T16."Disabled and Grayed Out" ("Disabled")) -> (reference out=w2557:refnum<vi>, error out=w2555:errorcluster)  [unwired: 1 in]
            n1480 = property class="VISAName"(reference=w2553, "DisabledEnum"=T16."Disabled and Grayed Out" ("Disabled")) -> (reference out=w2554:refnum<vi>, error out=w2552:errorcluster)  [unwired: 1 in]
            n1481 = property class="VISAName"(reference=w2550, "DisabledEnum"=T16."Disabled and Grayed Out" ("Disabled")) -> (reference out=w2538:refnum<vi>, error out=w2551:errorcluster)  [unwired: 1 in]
            n1482 = property class="VISAName"(reference=w2549, "DisabledEnum"=T16."Disabled and Grayed Out" ("Disabled")) -> (reference out=w2547:refnum<vi>, error out=w2548:errorcluster)  [unwired: 1 in]
            n1483 = property class="Str"(reference=w2544, "Visible"=FALSE) -> (reference out=w2546:refnum<vi>, error out=w2545:errorcluster)  [unwired: 1 in]
            n1484 = Close Reference(reference=w2537, error in (no error)=w2535) -> ()  [unwired: 1 out]
            n1485 = Close Reference(reference=w2557, error in (no error)=w2555) -> ()  [unwired: 1 out]
            n1486 = Close Reference(reference=w2554, error in (no error)=w2552) -> ()  [unwired: 1 out]
            n1487 = Close Reference(reference=w2538, error in (no error)=w2551) -> ()  [unwired: 1 out]
            n1488 = Close Reference(reference=w2547, error in (no error)=w2548) -> ()  [unwired: 1 out]
            n1489 = Close Reference(reference=w2546, error in (no error)=w2545) -> ()  [unwired: 1 out]
          }
        }
        n1490 = call "DATA ENCRYPT STRING FILE WRITE.vi"("error in (no error)"=w2507, "User Action"="User Pressed Advance Setting in Service Screen", "main ref"=w2501) -> ("error out"=w2506:errorcluster)  [unwired: 6 in, 1 out]
      }
      frame "Password" {
        n1491 = Unbundle By Name(w2558) -> ("About Screen.Password"=w2564:refnum<vi>)
        n1492 = property class="Str"(reference=w2564) -> (reference out=w2565:refnum<vi>, error out=w2563:errorcluster, "Value"=w2562:string)  [unwired: 1 in]
        n1493 = call <vilib>:"Trim Whitespace.vi"("string"=w2562) -> ("trimmed string"=w2561:string)  [unwired: 1 in]
        n1494 = Close Reference(reference=w2565, error in (no error)=w2563) -> ()  [unwired: 1 out]
        n1495 = Equal?(x=w2561, y="UT150$") -> (x = y?=w2559:bool)
        n1496 = case shown="True" w2559 {
          tunnel: w2558 -> [_ w2568]
          frame False {
          }
          frame True {
            n1497 = Unbundle By Name(w2568) -> ("Main Screen.Main Screen Tab"=w2570:refnum<vi>)
            n1498 = Unbundle By Name(w2568) -> ("Main Home Screen.GUI"=w2574:refnum<vi>)
            n1499 = Unbundle By Name(w2568) -> ("About Screen.Password"=w2578:refnum<vi>)
            n1500 = property class="TabCtl (strict)"(reference=w2574, "Value"=T4."Begin") -> (reference out=w2575:refnum<vi>, error out=w2573:errorcluster)  [unwired: 1 in]
            n1501 = property class="TabCtl (strict)"(reference=w2570, "Value"=T8."Service") -> (reference out=w2569:refnum<vi>, error out=w2571:errorcluster)  [unwired: 1 in]
            n1502 = property class="Str"(reference=w2578, "Value"="") -> (reference out=w2579:refnum<vi>, error out=w2577:errorcluster)  [unwired: 1 in]
            n1503 = Close Reference(reference=w2579, error in (no error)=w2577) -> ()  [unwired: 1 out]
            n1504 = Close Reference(reference=w2575, error in (no error)=w2573) -> ()  [unwired: 1 out]
            n1505 = Close Reference(reference=w2569, error in (no error)=w2571) -> ()  [unwired: 1 out]
          }
        }
      }
      frame "Service About" {
        n1506 = Unbundle By Name(w2581) -> ("Main Screen.Main Screen Tab"=w2584:refnum<vi>)
        n1507 = Unbundle By Name(w2581) -> ("Main Home Screen.GUI"=w2588:refnum<vi>)
        n1508 = local write "Service About"(FALSE ("Service About")) -> ()
        n1509 = property class="TabCtl (strict)"(reference=w2588, "Value"=T4."Begin") -> (reference out=w2589:refnum<vi>, error out=w2587:errorcluster)  [unwired: 1 in]
        n1510 = property class="TabCtl (strict)"(reference=w2584, "Value"=T8."About") -> (reference out=w2583:refnum<vi>, error out=w2585:errorcluster)  [unwired: 1 in]
        n1511 = Close Reference(reference=w2589, error in (no error)=w2587) -> ()  [unwired: 1 out]
        n1512 = Close Reference(reference=w2583, error in (no error)=w2585) -> ()  [unwired: 1 out]
      }
      frame "OPEN 1" {
        n1513 = Unbundle By Name(w2593) -> ("Analysis Screen.File 1 Discription"=w2602:refnum<vi>)
        n1514 = property class="Str"(reference=w2602, error in=w2600, "Value"="") -> (reference out=w2603:refnum<vi>, error out=w2601:errorcluster)
        n1515 = Close Reference(reference=w2603, error in (no error)=w2601) -> (error out=w2599:errorcluster)
        n1516 = call <vilib>:"Application Directory.vi"() -> ("Application Directory"=w2607:path)
        n1517 = Unbundle By Name(w2593) -> ("Analysis Screen.OPEN 1"=w2595:refnum<vi>)
        n1518 = Build Path(base path=w2607, name or relative path="data") -> (appended path=w2605:path)
        n1519 = property class="Bool (strict)"(reference=w2595, "Value"=FALSE) -> (reference out=w2596:refnum<vi>, error out=w2594:errorcluster)  [unwired: 1 in]
        n1520 = call "File Dialog3"("start path"=w2605, "error in"=w2599) -> ("selected path"=w2604:path, "cancelled"=w2591:bool, "error out"=w2608:errorcluster)  [unwired: 10 in, 1 out]
        n1521 = case shown="True" w2591 {
          tunnel: w2608 -> [w2622 _]
          tunnel: w2604 -> [w2618 _]
          tunnel: [w2610 _] -> w2597
          tunnel: w2593 -> [w2609 w2624]
          frame False {
            n1522 = Path To String(path=w2618) -> (string=w2617:string)
            n1523 = Unbundle By Name(w2609) -> ("Analysis Screen.File Name 1"=w2620:refnum<vi>)
            n1524 = call <vilib>:"Clear Errors.vi"("error in (no error)"=w2622) -> ("error out"=w2616:errorcluster)  [unwired: 5 in, 1 out]
            n1525 = property class="Str"(reference=w2620, "Value"=w2617) -> (reference out=w2621:refnum<vi>, error out=w2619:errorcluster)  [unwired: 1 in]
            n1526 = call "INI FILE READ.vi"("error in (no error)"=w2616, "File Path"=w2617) -> ("error out"=w2612:errorcluster, "concatenated string"=w2611:string)  [unwired: 8 in]
            n1527 = Unbundle By Name(w2609) -> ("Analysis Screen.File 1 Discription"=w2614:refnum<vi>)
            n1528 = Close Reference(reference=w2621, error in (no error)=w2619) -> ()  [unwired: 1 out]
            n1529 = property class="Str"(reference=w2614, error in=w2612, "Value"=w2611) -> (reference out=w2615:refnum<vi>, error out=w2613:errorcluster)
            n1530 = Close Reference(reference=w2615, error in (no error)=w2613) -> (error out=w2610:errorcluster)
          }
          frame True {
            n1531 = Unbundle By Name(w2624) -> ("Analysis Screen.File 1 Discription"=w2626:refnum<vi>)
            n1532 = Unbundle By Name(w2624) -> ("Analysis Screen.File Name 1"=w2630:refnum<vi>)
            n1533 = property class="Str"(reference=w2626, "Value"="") -> (reference out=w2627:refnum<vi>, error out=w2625:errorcluster)  [unwired: 1 in]
            n1534 = property class="Str"(reference=w2630, "Value"="") -> (reference out=w2631:refnum<vi>, error out=w2629:errorcluster)  [unwired: 1 in]
            n1535 = Close Reference(reference=w2627, error in (no error)=w2625) -> ()  [unwired: 1 out]
            n1536 = Close Reference(reference=w2631, error in (no error)=w2629) -> ()  [unwired: 1 out]
          }
        }
        n1537 = Close Reference(reference=w2596, error in (no error)=w2594) -> ()  [unwired: 1 out]
      }
      frame "OPEN 2" {
        n1538 = Unbundle By Name(w2634) -> ("Analysis Screen.File 2 Discription"=w2643:refnum<vi>)
        n1539 = property class="Str"(reference=w2643, error in=w2641, "Value"="") -> (reference out=w2644:refnum<vi>, error out=w2642:errorcluster)
        n1540 = Close Reference(reference=w2644, error in (no error)=w2642) -> (error out=w2640:errorcluster)
        n1541 = call <vilib>:"Application Directory.vi"() -> ("Application Directory"=w2648:path)
        n1542 = Unbundle By Name(w2634) -> ("Analysis Screen.OPEN 2"=w2636:refnum<vi>)
        n1543 = Build Path(base path=w2648, name or relative path="data") -> (appended path=w2646:path)
        n1544 = property class="Bool (strict)"(reference=w2636, "Value"=FALSE) -> (reference out=w2637:refnum<vi>, error out=w2635:errorcluster)  [unwired: 1 in]
        n1545 = call "File Dialog4"("start path"=w2646, "error in"=w2640) -> ("selected path"=w2645:path, "cancelled"=w2632:bool, "error out"=w2649:errorcluster)  [unwired: 10 in, 1 out]
        n1546 = case shown="True" w2632 {
          tunnel: w2649 -> [w2663 w2665]
          tunnel: w2645 -> [w2659 _]
          tunnel: [w2651 w2664] -> w2638
          tunnel: w2634 -> [w2650 w2667]
          frame False {
            n1547 = Path To String(path=w2659) -> (string=w2658:string)
            n1548 = Unbundle By Name(w2650) -> ("Analysis Screen.File Name 2"=w2661:refnum<vi>)
            n1549 = call <vilib>:"Clear Errors.vi"("error in (no error)"=w2663) -> ("error out"=w2657:errorcluster)  [unwired: 5 in, 1 out]
            n1550 = property class="Str"(reference=w2661, "Value"=w2658) -> (reference out=w2662:refnum<vi>, error out=w2660:errorcluster)  [unwired: 1 in]
            n1551 = call "INI FILE READ.vi"("error in (no error)"=w2657, "File Path"=w2658) -> ("error out"=w2653:errorcluster, "concatenated string"=w2652:string)  [unwired: 8 in]
            n1552 = Unbundle By Name(w2650) -> ("Analysis Screen.File 2 Discription"=w2655:refnum<vi>)
            n1553 = Close Reference(reference=w2662, error in (no error)=w2660) -> ()  [unwired: 1 out]
            n1554 = property class="Str"(reference=w2655, error in=w2653, "Value"=w2652) -> (reference out=w2656:refnum<vi>, error out=w2654:errorcluster)
            n1555 = Close Reference(reference=w2656, error in (no error)=w2654) -> (error out=w2651:errorcluster)
          }
          frame True {
            n1556 = Unbundle By Name(w2667) -> ("Analysis Screen.File Name 2"=w2673:refnum<vi>)
            n1557 = Unbundle By Name(w2667) -> ("Analysis Screen.File 2 Discription"=w2669:refnum<vi>)
            n1558 = property class="Str"(reference=w2673, "Value"="") -> (reference out=w2674:refnum<vi>, error out=w2672:errorcluster)  [unwired: 1 in]
            n1559 = property class="Str"(reference=w2669, "Value"="") -> (reference out=w2668:refnum<vi>, error out=w2670:errorcluster)  [unwired: 1 in]
            n1560 = call <vilib>:"Clear Errors.vi"("error in (no error)"=w2665) -> ("error out"=w2664:errorcluster)  [unwired: 5 in, 1 out]
            n1561 = Close Reference(reference=w2668, error in (no error)=w2670) -> ()  [unwired: 1 out]
            n1562 = Close Reference(reference=w2674, error in (no error)=w2672) -> ()  [unwired: 1 out]
          }
        }
        n1563 = Close Reference(reference=w2637, error in (no error)=w2635) -> ()  [unwired: 1 out]
      }
      frame "OPEN 3" {
        # "3416\n4017\n4554"
        n1564 = Unbundle By Name(w2677) -> ("Analysis Screen.File 3 Discription"=w2686:refnum<vi>)
        n1565 = property class="Str"(reference=w2686, error in=w2684, "Value"="") -> (reference out=w2687:refnum<vi>, error out=w2685:errorcluster)
        n1566 = Close Reference(reference=w2687, error in (no error)=w2685) -> (error out=w2683:errorcluster)
        n1567 = call <vilib>:"Application Directory.vi"() -> ("Application Directory"=w2691:path)
        n1568 = Unbundle By Name(w2677) -> ("Analysis Screen.OPEN 3"=w2679:refnum<vi>)
        n1569 = Build Path(base path=w2691, name or relative path="data") -> (appended path=w2689:path)
        n1570 = property class="Bool (strict)"(reference=w2679, "Value"=FALSE) -> (reference out=w2680:refnum<vi>, error out=w2678:errorcluster)  [unwired: 1 in]
        n1571 = call "File Dialog5"("start path"=w2689, "error in"=w2683) -> ("selected path"=w2688:path, "cancelled"=w2675:bool, "error out"=w2692:errorcluster)  [unwired: 10 in, 1 out]
        n1572 = case shown="True" w2675 {
          tunnel: w2692 -> [w2706 w2708]
          tunnel: w2688 -> [w2702 _]
          tunnel: [w2694 w2707] -> w2681
          tunnel: w2677 -> [w2693 w2710]
          frame False {
            n1573 = Path To String(path=w2702) -> (string=w2701:string)
            n1574 = Unbundle By Name(w2693) -> ("Analysis Screen.File Name 3"=w2704:refnum<vi>)
            n1575 = call <vilib>:"Clear Errors.vi"("error in (no error)"=w2706) -> ("error out"=w2700:errorcluster)  [unwired: 5 in, 1 out]
            n1576 = property class="Str"(reference=w2704, "Value"=w2701) -> (reference out=w2705:refnum<vi>, error out=w2703:errorcluster)  [unwired: 1 in]
            n1577 = call "INI FILE READ.vi"("error in (no error)"=w2700, "File Path"=w2701) -> ("error out"=w2696:errorcluster, "concatenated string"=w2695:string)  [unwired: 8 in]
            n1578 = Unbundle By Name(w2693) -> ("Analysis Screen.File 3 Discription"=w2698:refnum<vi>)
            n1579 = Close Reference(reference=w2705, error in (no error)=w2703) -> ()  [unwired: 1 out]
            n1580 = property class="Str"(reference=w2698, error in=w2696, "Value"=w2695) -> (reference out=w2699:refnum<vi>, error out=w2697:errorcluster)
            n1581 = Close Reference(reference=w2699, error in (no error)=w2697) -> (error out=w2694:errorcluster)
          }
          frame True {
            n1582 = Unbundle By Name(w2710) -> ("Analysis Screen.File Name 3"=w2716:refnum<vi>)
            n1583 = Unbundle By Name(w2710) -> ("Analysis Screen.File 3 Discription"=w2712:refnum<vi>)
            n1584 = property class="Str"(reference=w2716, "Value"="") -> (reference out=w2717:refnum<vi>, error out=w2715:errorcluster)  [unwired: 1 in]
            n1585 = property class="Str"(reference=w2712, "Value"="") -> (reference out=w2711:refnum<vi>, error out=w2713:errorcluster)  [unwired: 1 in]
            n1586 = Close Reference(reference=w2711, error in (no error)=w2713) -> ()  [unwired: 1 out]
            n1587 = Close Reference(reference=w2717, error in (no error)=w2715) -> ()  [unwired: 1 out]
            n1588 = call <vilib>:"Clear Errors.vi"("error in (no error)"=w2708) -> ("error out"=w2707:errorcluster)  [unwired: 5 in, 1 out]
          }
        }
        n1589 = Close Reference(reference=w2680, error in (no error)=w2678) -> ()  [unwired: 1 out]
      }
      frame "OPEN 4" {
        n1590 = Unbundle By Name(w2720) -> ("Analysis Screen.File 4 Discription"=w2729:refnum<vi>)
        n1591 = property class="Str"(reference=w2729, error in=w2727, "Value"="") -> (reference out=w2730:refnum<vi>, error out=w2728:errorcluster)
        n1592 = Close Reference(reference=w2730, error in (no error)=w2728) -> (error out=w2726:errorcluster)
        n1593 = call <vilib>:"Application Directory.vi"() -> ("Application Directory"=w2734:path)
        n1594 = Unbundle By Name(w2720) -> ("Analysis Screen.OPEN 4"=w2722:refnum<vi>)
        n1595 = Build Path(base path=w2734, name or relative path="data") -> (appended path=w2732:path)
        n1596 = property class="Bool (strict)"(reference=w2722, "Value"=FALSE) -> (reference out=w2723:refnum<vi>, error out=w2721:errorcluster)  [unwired: 1 in]
        n1597 = call "File Dialog6"("start path"=w2732, "error in"=w2726) -> ("selected path"=w2731:path, "cancelled"=w2718:bool, "error out"=w2735:errorcluster)  [unwired: 10 in, 1 out]
        n1598 = case shown="True" w2718 {
          tunnel: w2735 -> [w2749 w2751]
          tunnel: w2731 -> [w2745 _]
          tunnel: [w2737 w2750] -> w2724
          tunnel: w2720 -> [w2736 w2753]
          frame False {
            n1599 = Path To String(path=w2745) -> (string=w2744:string)
            n1600 = Unbundle By Name(w2736) -> ("Analysis Screen.File Name 4"=w2747:refnum<vi>)
            n1601 = call <vilib>:"Clear Errors.vi"("error in (no error)"=w2749) -> ("error out"=w2743:errorcluster)  [unwired: 5 in, 1 out]
            n1602 = property class="Str"(reference=w2747, "Value"=w2744) -> (reference out=w2748:refnum<vi>, error out=w2746:errorcluster)  [unwired: 1 in]
            n1603 = call "INI FILE READ.vi"("error in (no error)"=w2743, "File Path"=w2744) -> ("error out"=w2739:errorcluster, "concatenated string"=w2738:string)  [unwired: 8 in]
            n1604 = Unbundle By Name(w2736) -> ("Analysis Screen.File 4 Discription"=w2741:refnum<vi>)
            n1605 = Close Reference(reference=w2748, error in (no error)=w2746) -> ()  [unwired: 1 out]
            n1606 = property class="Str"(reference=w2741, error in=w2739, "Value"=w2738) -> (reference out=w2742:refnum<vi>, error out=w2740:errorcluster)
            n1607 = Close Reference(reference=w2742, error in (no error)=w2740) -> (error out=w2737:errorcluster)
          }
          frame True {
            n1608 = Unbundle By Name(w2753) -> ("Analysis Screen.File Name 4"=w2759:refnum<vi>)
            n1609 = Unbundle By Name(w2753) -> ("Analysis Screen.File 4 Discription"=w2755:refnum<vi>)
            n1610 = property class="Str"(reference=w2759, "Value"="") -> (reference out=w2760:refnum<vi>, error out=w2758:errorcluster)  [unwired: 1 in]
            n1611 = property class="Str"(reference=w2755, "Value"="") -> (reference out=w2754:refnum<vi>, error out=w2756:errorcluster)  [unwired: 1 in]
            n1612 = Close Reference(reference=w2754, error in (no error)=w2756) -> ()  [unwired: 1 out]
            n1613 = Close Reference(reference=w2760, error in (no error)=w2758) -> ()  [unwired: 1 out]
            n1614 = call <vilib>:"Clear Errors.vi"("error in (no error)"=w2751) -> ("error out"=w2750:errorcluster)  [unwired: 5 in, 1 out]
          }
        }
        n1615 = Close Reference(reference=w2723, error in (no error)=w2721) -> ()  [unwired: 1 out]
      }
      frame "Refresh 2" {
        n1616 = call "Data Log Refresh.vi"("error in (no error)"=w2763, "Data Cluster"=w2762) -> ("error out"=w2764:errorcluster)  [unwired: 9 in]
        n1617 = local write "Refresh 2"(FALSE ("Refresh 2")) -> ()
      }
      frame "Scratch Mode" {
        n1618 = Unbundle By Name(w2765) -> ("Motion Module.Scratch Mode"=w2768:refnum<vi>)
        n1619 = property class="Ring (strict)"(reference=w2768) -> (reference out=w2769:refnum<vi>, error out=w2767:errorcluster, "Value"=w2766:u16)  [unwired: 1 in]
        n1620 = Close Reference(reference=w2769, error in (no error)=w2767) -> ()  [unwired: 1 out]
        n1621 = case shown="2" w2766 {
          tunnel: w2765 -> [w2772 w2776]
          frame 0, Default {
            n1622 = Unbundle By Name(w2772) -> ("Motion Module.No of Scratch"=w2774:refnum<vi>)
            n1623 = property class="DigNum (strict)"(reference=w2774, "Visible"=FALSE) -> (reference out=w2775:refnum<vi>, error out=w2773:errorcluster)  [unwired: 1 in]
            n1624 = Close Reference(reference=w2775, error in (no error)=w2773) -> ()  [unwired: 1 out]
          }
          frame 2 {
            n1625 = Unbundle By Name(w2776) -> ("Motion Module.No of Scratch"=w2779:refnum<vi>)
            n1626 = property class="DigNum (strict)"(reference=w2779, "Visible"=TRUE) -> (reference out=w2780:refnum<vi>, error out=w2778:errorcluster)  [unwired: 1 in]
            n1627 = Close Reference(reference=w2780, error in (no error)=w2778) -> ()  [unwired: 1 out]
          }
        }
      }
      frame "Export" {
        n1628 = call "Export file.vi"("error in (no error)"=w2789, "Data Cluster"=w2782) -> ("error out"=w2784:errorcluster)  [unwired: 9 in]
        n1629 = call "DATA ENCRYPT STRING FILE WRITE.vi"("error in (no error)"=w2784, "User Action"="User Pressed  Export ", "main ref"=w2782) -> ("error out"=w2783:errorcluster)  [unwired: 6 in, 1 out]
        n1630 = Unbundle By Name(w2782) -> ("Analysis Screen.Export"=w2787:refnum<vi>)
        n1631 = property class="Bool (strict)"(reference=w2787, "Value"=FALSE) -> (reference out=w2788:refnum<vi>, error out=w2786:errorcluster)  [unwired: 1 in]
        n1632 = Close Reference(reference=w2788, error in (no error)=w2786) -> ()  [unwired: 1 out]
      }
      frame "Error" {
        # "#CodeRecommended - If you ever change the name of this \"Error\" message, you'll need to update the name in the Check Loop Error.vi as well."
        # "#CodeRecommended - Consider creating a system for logging errors in some way. These errors are for notification purposes only. Handling of specific errors should be performed in the message frames that generated the error."
        # "Error - Display an error dialog. This message is sent by the \"Error Handler\" VIs at the end of other loops in this application."
        n1633 = Variant To Data(error in=w2796, type=errorcluster {"status"=FALSE, "code"=0, "source"=""} ("error constant"), Variant=w2794) -> (data=w2792:errorcluster, error out=w2791:errorcluster)
        n1634 = call <vilib>:"Simple Error Handler.vi"("error in (no error)"=w2792) -> ()  [unwired: 4 in, 5 out]
        n1635 = Merge Errors(w2791) -> (w2790:errorcluster)
      }
      frame "Confirm Quit" {
        # "#CodeNeeded - If you want to provide an \"Are you sure\" dialog (or some other notification) before the application exits, place that code here. This message is typically sent from a Panel Close? event."
        # "Confirm Quit - Message that can confirm whether or not the user wants to exit the application."
        n1636 = call-poly "Enqueue Message.vi"("Priority Message? (F)"=TRUE, "error in (no error)"=w2803, "Message"="Exit", "Message Queue"=w2800) -> ("error out"=w2801:errorcluster)  [unwired: 6 in, 1 out]
        n1637 = Merge Errors(w2801) -> (w2802:errorcluster)
      }
      frame "Exit" {
        # "Stop the VI"
        # "Release the message queue reference"
        # "#CodeNeeded - Add any required cleanup code here. Note that if 'Exit' was called as a result of an error, an error dialog will be displayed. Add any custom error handling for an 'Exit' condition here as well."
        # "Exit - Exit the application."
        n1638 = call "Fire User Event - Stop.vi"("User Event - Stop"=w2806) -> ("error out"=w2805:errorcluster)  [unwired: 10 in]
        n1639 = Release Queue(queue=w2811, error in (no error)=w2804) -> (error out=w2808:errorcluster)  [unwired: 1 in, 2 out]
        n1640 = Merge Errors(w2805, w2808) -> (w2807:errorcluster)
      }
      frame Default {
        # "'Default' case only runs if there is a message that isn't defined in any of the other cases.  Output a programming error."
        n1641 = xnode "Error Ring"("parameter 0"=w2812) -> ("error out"=w2813:errorcluster)
      }
    }
    n1642 = call "LAB-IQ Error Handler - Message Handling Loop.vi"("error in (no error)"=w1505, "Message Queue"=w1507) -> ("dup error in"=w1506:errorcluster)  [unwired: 8 in, 1 out]
  }
  n1643 = timed-loop {
    shift-right: [w2832] -> _
    shift-left: w26 -> [w2833]
    tunnel: [w2826] -> w31
    tunnel: w17 -> [w2824]
    tunnel: w16 -> [w2823]
    tunnel: w25 -> [w2822]
    timing: w9 -> [_]
    timing-out: [_] -> w8
    stop <- w2831 stop-if-true
    # "Heave Motor  Handling Loop"
    n1644 = node-c288() -> ()  [unwired: 1 in, 1 out]
    n1645 = call "Dequeue Message.vi"("error in (no error)"=w2823, "Message Queue"=w2824) -> ("error out"=w2830:errorcluster, "Message Data"=w2828:variant, "Message"=w2829:string, "dup Message Queue"=w2827:refnum<queue>)  [unwired: 6 in]
    n1646 = case "Message Cases" shown="\"Heave Main\"" w2829 {
      selector: w2829 -> [_ _ _ _ _ w2926]
      tunnel: w2827 -> [w2846 w2862 _ w2914 w2925 _]
      tunnel: w2830 -> [w2843 w2860 w2906 w2917 w2919 _]
      tunnel: [w2844 w2863 w2900 w2907 w2921 w2927] -> w2825
      tunnel: w2833 -> [w2836 w2848 w2905 w2910 w2924 w2928]
      tunnel: [w2836 w2848 w2905 w2910 w2924 w2928] -> w2832
      tunnel: [_ _ _ _ TRUE _] -> w2831
      tunnel: w2828 -> [_ _ w2904 _ _ _]
      tunnel: w2822 -> [_ _ _ _ w2918 _]
      frame "init" {
        # "Initialize - All initialization work should take place in this message, since other loops can potentially enqueue messages that execute immediately after this one."
        n1647 = call "HEAVE WRITE FGV.vi"("Enum - Menu"=Heave_Write_enum."INIT", "error in (no error)"=w2843, "main ref"=w2836) -> ("error out"=w2842:errorcluster)  [unwired: 7 in, 1 out]
        n1648 = call <vilib>:"Clear Errors.vi"("error in (no error)"=w2842) -> ("error out"=w2837:errorcluster)  [unwired: 5 in, 1 out]
        n1649 = call "Stall Data Flow.vim"("value in"=w2837, "milliseconds to wait"=u32 1000) -> ("value out"=w2840:errorcluster)  [unwired: 1 out]
        n1650 = call "Heave Init.vi"("error in (no error)"=w2840, "main ref"=w2836) -> ("error out"=w2838:errorcluster)  [unwired: 9 in]
        n1651 = call <vilib>:"Clear Errors.vi"("error in (no error)"=w2838) -> ("error out"=w2845:errorcluster)  [unwired: 5 in, 1 out]
        n1652 = call-poly "Enqueue Message.vi"("error in (no error)"=w2845, "Message"="Heave Main", "Message Queue"=w2846) -> ("error out"=w2844:errorcluster)  [unwired: 7 in, 1 out]
      }
      frame "Heave Main" {
        n1653 = Unbundle By Name(w2848) -> ("Heave AND Surge.Read Heave Temp"=w2856:refnum<vi>)
        n1654 = property class="Bool (strict)"(reference=w2856) -> (reference out=w2854:refnum<vi>, error out=w2855:errorcluster, "Value"=w2853:bool)  [unwired: 1 in]
        n1655 = Close Reference(reference=w2854, error in (no error)=w2855) -> ()  [unwired: 1 out]
        n1656 = case shown="True" w2853 {
          tunnel: w2860 -> [w2886 w2891]
          tunnel: [w2886 w2890] -> w2851
          tunnel: w2848 -> [_ w2889]
          tunnel: [FALSE ("x < y?") w2887] -> w2849
          frame False {
          }
          frame True {
            n1657 = call "HEAVE WRITE FGV.vi"("Enum - Menu"=Heave_Write_enum."READ", "error in (no error)"=w2891, "main ref"=w2889) -> ("error out"=w2890:errorcluster, "x < y?"=w2887:bool)  [unwired: 7 in]
          }
        }
        n1658 = case shown="True" w2849 {
          tunnel: w2848 -> [w2866 w2873]
          frame False {
            w2864 = TRUE ("PAUSE")
            w2865 = FALSE ("Value")
            n1659 = Unbundle By Name(w2866) -> ("Platform Settings.Heave COM Status"=w2872:refnum<vi>)
            n1660 = Unbundle By Name(w2866) -> ("Main Screen.Heave COM Status"=w2867:refnum<vi>)
            n1661 = property class="Bool (strict)"(reference=w2872, "Value"=w2865) -> (reference out=w2870:refnum<vi>, error out=w2871:errorcluster)  [unwired: 1 in]
            n1662 = property class="Bool (strict)"(reference=w2867, "Value"=w2865) -> (reference out=w2869:refnum<vi>, error out=w2868:errorcluster)  [unwired: 1 in]
            n1663 = Close Reference(reference=w2870, error in (no error)=w2871) -> ()  [unwired: 1 out]
            n1664 = Close Reference(reference=w2869, error in (no error)=w2868) -> ()  [unwired: 1 out]
            n1665 = call "ELAPSED TIMER VI FOR Sway Loop Connection.vi"("RESET"=w2864, "PAUSE"=w2864) -> ()  [unwired: 7 in, 3 out]
          }
          frame True {
            w2876 = FALSE ("PAUSE")
            n1666 = call "ELAPSED TIMER VI FOR Sway Loop Connection.vi"("TARGET"=2.0, "RESET"=w2876, "PAUSE"=w2876) -> ("ELAPSED INDICATION"=w2874:bool)  [unwired: 6 in, 2 out]
            n1667 = case shown="True" w2874 {
              tunnel: w2873 -> [_ w2877]
              frame False {
              }
              frame True {
                w2878 = TRUE ("Value")
                n1668 = Unbundle By Name(w2877) -> ("Main Screen.Heave COM Status"=w2879:refnum<vi>)
                n1669 = Unbundle By Name(w2877) -> ("Platform Settings.Heave COM Status"=w2884:refnum<vi>)
                n1670 = property class="Bool (strict)"(reference=w2879, "Value"=w2878) -> (reference out=w2881:refnum<vi>, error out=w2880:errorcluster)  [unwired: 1 in]
                n1671 = property class="Bool (strict)"(reference=w2884, "Value"=w2878) -> (reference out=w2882:refnum<vi>, error out=w2883:errorcluster)  [unwired: 1 in]
                n1672 = Close Reference(reference=w2881, error in (no error)=w2880) -> ()  [unwired: 1 out]
                n1673 = Close Reference(reference=w2882, error in (no error)=w2883) -> ()  [unwired: 1 out]
              }
            }
          }
        }
        n1674 = call "Heave Reinitial.vi"("error in (no error)"=w2851, "Data Cluster"=w2848) -> ("error out"=w2850:errorcluster)  [unwired: 9 in]
        n1675 = Unbundle By Name(w2848) -> ("Main Home Screen.EXIT"=w2861:refnum<vi>)
        n1676 = property class="Bool (strict)"(reference=w2861) -> (reference out=w2858:refnum<vi>, error out=w2859:errorcluster, "Value"=w2857:bool)  [unwired: 1 in]
        n1677 = call <vilib>:"Clear Errors.vi"("error in (no error)"=w2850) -> ("error out"=w2852:errorcluster)  [unwired: 5 in, 1 out]
        n1678 = Close Reference(reference=w2858, error in (no error)=w2859) -> ()  [unwired: 1 out]
        n1679 = case shown="False" w2857 {
          tunnel: [w2894 w2898] -> w2863
          tunnel: w2862 -> [w2893 w2897]
          tunnel: w2852 -> [w2892 w2896]
          frame True {
            n1680 = call-poly "Enqueue Message.vi"("error in (no error)"=w2892, "Message"="Confirm Quit", "Message Queue"=w2893) -> ("error out"=w2894:errorcluster)  [unwired: 7 in, 1 out]
          }
          frame False {
            n1681 = call-poly "Enqueue Message.vi"("error in (no error)"=w2896, "Message"="Heave Main", "Message Queue"=w2897) -> ("error out"=w2898:errorcluster)  [unwired: 7 in, 1 out]
          }
        }
      }
      frame "Error" {
        # "#CodeRecommended - If you ever change the name of this \"Error\" message, you'll need to update the name in the Check Loop Error.vi as well."
        # "#CodeRecommended - Consider creating a system for logging errors in some way. These errors are for notification purposes only. Handling of specific errors should be performed in the message frames that generated the error."
        # "Error - Display an error dialog. This message is sent by the \"Error Handler\" VIs at the end of other loops in this application."
        n1682 = Variant To Data(error in=w2906, type=errorcluster {"status"=FALSE, "code"=0, "source"=""} ("error constant"), Variant=w2904) -> (data=w2902:errorcluster, error out=w2901:errorcluster)
        n1683 = call <vilib>:"Simple Error Handler.vi"("error in (no error)"=w2902) -> ()  [unwired: 4 in, 5 out]
        n1684 = Merge Errors(w2901) -> (w2900:errorcluster)
      }
      frame "Confirm Quit" {
        # "#CodeNeeded - If you want to provide an \"Are you sure\" dialog (or some other notification) before the application exits, place that code here. This message is typically sent from a Panel Close? event."
        # "Confirm Quit - Message that can confirm whether or not the user wants to exit the application."
        n1685 = call-poly "Enqueue Message.vi"("Priority Message? (F)"=TRUE, "error in (no error)"=w2917, "Message"="Exit", "Message Queue"=w2914) -> ("error out"=w2915:errorcluster)  [unwired: 6 in, 1 out]
        n1686 = Merge Errors(w2915) -> (w2916:errorcluster)
        n1687 = call <vilib>:"Clear Errors.vi"("error in (no error)"=w2916) -> ("error out"=w2908:errorcluster)  [unwired: 5 in, 1 out]
        n1688 = call "HEAVE WRITE FGV.vi"("Enum - Menu"=Heave_Write_enum."CLOSE", "error in (no error)"=w2908, "main ref"=w2910) -> ("error out"=w2911:errorcluster)  [unwired: 7 in, 1 out]
        n1689 = call <vilib>:"Clear Errors.vi"("error in (no error)"=w2911) -> ("error out"=w2907:errorcluster)  [unwired: 5 in, 1 out]
      }
      frame "Exit" {
        # "Stop the VI"
        # "Release the message queue reference"
        # "#CodeNeeded - Add any required cleanup code here. Note that if 'Exit' was called as a result of an error, an error dialog will be displayed. Add any custom error handling for an 'Exit' condition here as well."
        # "Exit - Exit the application."
        n1690 = call "Fire User Event - Stop.vi"("User Event - Stop"=w2918) -> ("error out"=w2920:errorcluster)  [unwired: 10 in]
        n1691 = Release Queue(queue=w2925, error in (no error)=w2919) -> (error out=w2922:errorcluster)  [unwired: 1 in, 2 out]
        n1692 = Merge Errors(w2920, w2922) -> (w2921:errorcluster)
      }
      frame Default {
        # "'Default' case only runs if there is a message that isn't defined in any of the other cases.  Output a programming error."
        n1693 = xnode "Error Ring"("parameter 0"=w2926) -> ("error out"=w2927:errorcluster)
      }
    }
    n1694 = node-c288() -> ()  [unwired: 1 in, 1 out]
    n1695 = call "LAB-IQ Error Handler - Message Handling Loop.vi"("error in (no error)"=w2825, "Message Queue"=w2827) -> ("dup error in"=w2826:errorcluster)  [unwired: 8 in, 1 out]
  }
  n1696 = timed-loop {
    shift-right: [w2946] -> _
    shift-left: w26 -> [w2947]
    tunnel: [w2940] -> w36
    tunnel: w35 -> [w2938]
    tunnel: w16 -> [w2937]
    tunnel: w25 -> [w2936]
    timing: w5 -> [_]
    timing-out: [_] -> w4
    stop <- w2945 stop-if-true
    # "Load  Handling Loop"
    n1697 = node-c288() -> ()  [unwired: 1 in, 1 out]
    n1698 = call "Dequeue Message.vi"("error in (no error)"=w2937, "Message Queue"=w2938) -> ("error out"=w2944:errorcluster, "Message Data"=w2942:variant, "Message"=w2943:string, "dup Message Queue"=w2941:refnum<queue>)  [unwired: 6 in]
    n1699 = case "Message Cases" shown="\"Load Main\"" w2943 {
      selector: w2943 -> [_ _ _ _ _ w3003]
      tunnel: w2941 -> [w2950 w2963 _ w2992 w3002 _]
      tunnel: w2944 -> [w2953 w2961 w2979 w2994 w2996 _]
      tunnel: [w2954 w2964 w2973 w2980 w2998 w3004] -> w2939
      tunnel: w2947 -> [w2952 w2956 w2978 w2989 w3001 w3005]
      tunnel: [w2952 w2956 w2978 w2989 w3001 w3005] -> w2946
      tunnel: [_ _ _ _ TRUE _] -> w2945
      tunnel: w2942 -> [_ _ w2977 _ _ _]
      tunnel: w2936 -> [_ _ _ _ w2995 _]
      frame "init" {
        # "Bundle control references and a sample string value."
        # "Initialize - All initialization work should take place in this message, since other loops can potentially enqueue messages that execute immediately after this one."
        n1700 = call-poly "Enqueue Message.vi"("error in (no error)"=w2953, "Message"="Load Main", "Message Queue"=w2950) -> ("error out"=w2954:errorcluster)  [unwired: 7 in, 1 out]
      }
      frame "Load Main" {
        n1701 = call "LOAD CELL READ.vi"("error in (no error)"=w2961, "main ref"=w2956) -> ("error out"=w2957:errorcluster)  [unwired: 9 in]
        n1702 = call <vilib>:"Clear Errors.vi"("error in (no error)"=w2957) -> ("error out"=w2955:errorcluster)  [unwired: 5 in, 1 out]
        n1703 = Unbundle By Name(w2956) -> ("Main Home Screen.EXIT"=w2962:refnum<vi>)
        n1704 = property class="Bool (strict)"(reference=w2962) -> (reference out=w2959:refnum<vi>, error out=w2960:errorcluster, "Value"=w2958:bool)  [unwired: 1 in]
        n1705 = Close Reference(reference=w2959, error in (no error)=w2960) -> ()  [unwired: 1 out]
        n1706 = case shown="False" w2958 {
          tunnel: [w2967 w2971] -> w2964
          tunnel: w2963 -> [w2966 w2970]
          tunnel: w2955 -> [w2965 w2969]
          frame True {
            n1707 = call-poly "Enqueue Message.vi"("error in (no error)"=w2965, "Message"="Confirm Quit", "Message Queue"=w2966) -> ("error out"=w2967:errorcluster)  [unwired: 7 in, 1 out]
          }
          frame False {
            n1708 = call-poly "Enqueue Message.vi"("error in (no error)"=w2969, "Message"="Load Main", "Message Queue"=w2970) -> ("error out"=w2971:errorcluster)  [unwired: 7 in, 1 out]
          }
        }
      }
      frame "Error" {
        # "#CodeRecommended - If you ever change the name of this \"Error\" message, you'll need to update the name in the Check Loop Error.vi as well."
        # "#CodeRecommended - Consider creating a system for logging errors in some way. These errors are for notification purposes only. Handling of specific errors should be performed in the message frames that generated the error."
        # "Error - Display an error dialog. This message is sent by the \"Error Handler\" VIs at the end of other loops in this application."
        n1709 = Variant To Data(error in=w2979, type=errorcluster {"status"=FALSE, "code"=0, "source"=""} ("error constant"), Variant=w2977) -> (data=w2975:errorcluster, error out=w2974:errorcluster)
        n1710 = call <vilib>:"Simple Error Handler.vi"("error in (no error)"=w2975) -> ()  [unwired: 4 in, 5 out]
        n1711 = Merge Errors(w2974) -> (w2973:errorcluster)
      }
      frame "Confirm Quit" {
        # "#CodeNeeded - If you want to provide an \"Are you sure\" dialog (or some other notification) before the application exits, place that code here. This message is typically sent from a Panel Close? event."
        # "Confirm Quit - Message that can confirm whether or not the user wants to exit the application."
        n1712 = call-poly "Enqueue Message.vi"("Priority Message? (F)"=TRUE, "error in (no error)"=w2994, "Message"="Exit", "Message Queue"=w2992) -> ("error out"=w2993:errorcluster)  [unwired: 6 in, 1 out]
        n1713 = Merge Errors(w2993) -> (w2985:errorcluster)
        n1714 = call <vilib>:"Clear Errors.vi"("error in (no error)"=w2985) -> ("error out"=w2981:errorcluster)  [unwired: 5 in, 1 out]
        n1715 = call "LOAD CELL FGV MAIN.vi"("Enum"=T17."UNINITIAL", "error in (no error)"=w2981, "main ref"=w2989) -> ("error IO"=w2988:errorcluster)  [unwired: 8 in]
        n1716 = call "Stall Data Flow.vim"("value in"=w2988, "milliseconds to wait"=u32 1000) -> ("value out"=w2983:errorcluster)  [unwired: 1 out]
        n1717 = call "LOAD CELL FGV MAIN.vi"("Enum"=T17."DELETEHANDLE", "error in (no error)"=w2983, "main ref"=w2989) -> ("error IO"=w2984:errorcluster)  [unwired: 8 in]
        n1718 = call <vilib>:"Clear Errors.vi"("error in (no error)"=w2984) -> ("error out"=w2980:errorcluster)  [unwired: 5 in, 1 out]
      }
      frame "Exit" {
        # "Stop the VI"
        # "Release the message queue reference"
        # "#CodeNeeded - Add any required cleanup code here. Note that if 'Exit' was called as a result of an error, an error dialog will be displayed. Add any custom error handling for an 'Exit' condition here as well."
        # "Exit - Exit the application."
        n1719 = call "Fire User Event - Stop.vi"("User Event - Stop"=w2995) -> ("error out"=w2997:errorcluster)  [unwired: 10 in]
        n1720 = Release Queue(queue=w3002, error in (no error)=w2996) -> (error out=w2999:errorcluster)  [unwired: 1 in, 2 out]
        n1721 = Merge Errors(w2997, w2999) -> (w2998:errorcluster)
      }
      frame Default {
        # "'Default' case only runs if there is a message that isn't defined in any of the other cases.  Output a programming error."
        n1722 = xnode "Error Ring"("parameter 0"=w3003) -> ("error out"=w3004:errorcluster)
      }
    }
    n1723 = node-c288() -> ()  [unwired: 1 in, 1 out]
    n1724 = call "LAB-IQ Error Handler - Message Handling Loop.vi"("error in (no error)"=w2939, "Message Queue"=w2941) -> ("dup error in"=w2940:errorcluster)  [unwired: 8 in, 1 out]
  }
  n1725 = timed-loop {
    shift-right: [w3023] -> _
    shift-left: w26 -> [w3024]
    tunnel: [w3017] -> w33
    tunnel: w34 -> [w3015]
    tunnel: w16 -> [w3014]
    tunnel: w25 -> [w3013]
    timing: w7 -> [_]
    timing-out: [_] -> w6
    stop <- w3022 stop-if-true
    # "Sway Motor  Handling Loop"
    n1726 = node-c288() -> ()  [unwired: 1 in, 1 out]
    n1727 = call "Dequeue Message.vi"("error in (no error)"=w3014, "Message Queue"=w3015) -> ("error out"=w3021:errorcluster, "Message Data"=w3019:variant, "Message"=w3020:string, "dup Message Queue"=w3018:refnum<queue>)  [unwired: 6 in]
    n1728 = case "Message Cases" shown="\"Sway Main\"" w3020 {
      selector: w3020 -> [_ _ _ _ _ w3108]
      tunnel: w3018 -> [w3036 w3065 _ w3095 w3107 _]
      tunnel: w3021 -> [w3038 w3046 w3092 w3099 w3101 _]
      tunnel: [w3039 w3066 w3086 w3097 w3103 w3109] -> w3016
      tunnel: w3024 -> [w3029 w3040 w3091 w3098 w3106 w3110]
      tunnel: [w3029 w3040 w3091 w3098 w3106 w3110] -> w3023
      tunnel: [_ _ _ _ TRUE _] -> w3022
      tunnel: w3019 -> [_ _ w3090 _ _ _]
      tunnel: w3013 -> [_ _ _ _ w3100 _]
      frame "init" {
        # "Initialize - All initialization work should take place in this message, since other loops can potentially enqueue messages that execute immediately after this one."
        n1729 = call "SWAY WRITE FGV.vi"("Enum - Menu"=Sway_Write_enum."INIT", "error in (no error)"=w3038, "main ref"=w3029) -> ("error out"=w3035:errorcluster)  [unwired: 8 in]
        n1730 = call <vilib>:"Clear Errors.vi"("error in (no error)"=w3035) -> ("error out"=w3028:errorcluster)  [unwired: 5 in, 1 out]
        n1731 = call "Stall Data Flow.vim"("value in"=w3028, "milliseconds to wait"=u32 1000) -> ("value out"=w3033:errorcluster)  [unwired: 1 out]
        n1732 = call "Sway Init.vi"("error in (no error)"=w3033, "main ref"=w3029) -> ("error out"=w3030:errorcluster)  [unwired: 9 in]
        n1733 = call <vilib>:"Clear Errors.vi"("error in (no error)"=w3030) -> ("error out"=w3027:errorcluster)  [unwired: 5 in, 1 out]
        n1734 = call <vilib>:"Clear Errors.vi"("error in (no error)"=w3027) -> ("error out"=w3031:errorcluster)  [unwired: 5 in, 1 out]
        n1735 = call-poly "Enqueue Message.vi"("error in (no error)"=w3031, "Message"="Sway Main", "Message Queue"=w3036) -> ("error out"=w3039:errorcluster)  [unwired: 7 in, 1 out]
      }
      frame "Sway Main" {
        n1736 = Unbundle By Name(w3040) -> ("Heave AND Surge.SURGE POSE"=w3051:refnum<vi>)
        n1737 = Unbundle By Name(w3040) -> ("SWAY.Read SWAY Temp"=w3060:refnum<vi>)
        n1738 = local read "HEAVE ENABLE"() -> (w3055:bool)
        n1739 = property class="DigNum (strict)"(reference=w3051) -> (reference out=w3053:refnum<vi>, error out=w3052:errorcluster, "Value"=w3050:sgl)  [unwired: 1 in]
        n1740 = property class="Bool (strict)"(reference=w3060) -> (reference out=w3058:refnum<vi>, error out=w3059:errorcluster, "Value"=w3057:bool)  [unwired: 1 in]
        n1741 = Equal?(x=w3055, y=TRUE) -> (x = y?=w3049:bool)
        n1742 = Close Reference(reference=w3053, error in (no error)=w3052) -> ()  [unwired: 1 out]
        n1743 = Equal?(x=w3050, y=sgl 25000.0) -> (x = y?=w3048:bool)
        n1744 = Close Reference(reference=w3058, error in (no error)=w3059) -> ()  [unwired: 1 out]
        n1745 = And(x=w3049, y=w3048) -> (x .and. y?=w3047:bool)
        n1746 = case shown="True" w3057 {
          tunnel: w3046 -> [w3073 w3077]
          tunnel: [w3073 w3076] -> w3042
          tunnel: w3040 -> [_ w3075]
          frame False {
          }
          frame True {
            n1747 = call "SWAY WRITE FGV.vi"("Enum - Menu"=Sway_Write_enum."READ", "error in (no error)"=w3077, "main ref"=w3075) -> ("error out"=w3076:errorcluster)  [unwired: 8 in]
          }
        }
        n1748 = case shown="True" w3047 {
          tunnel: w3040 -> [_ w3072]
          tunnel: w3046 -> [w3067 w3071]
          tunnel: [w3067 w3068] -> w3044
          frame False {
          }
          frame True {
            n1749 = call "SWAY HOME.vi"("error in (no error)"=w3071, "Data Cluster"=w3072) -> ("error out"=w3069:errorcluster)  [unwired: 9 in]
            n1750 = local write "HEAVE ENABLE"(FALSE ("HEAVE ENABLE")) -> ()
            n1751 = call <vilib>:"Clear Errors.vi"("error in (no error)"=w3069) -> ("error out"=w3068:errorcluster)  [unwired: 5 in, 1 out]
          }
        }
        n1752 = call "Sway Reinitize.vi"("error in (no error)"=w3042, "Data Cluster"=w3040) -> ("error out"=w3041:errorcluster)  [unwired: 9 in]
        n1753 = Unbundle By Name(w3040) -> ("Main Home Screen.EXIT"=w3064:refnum<vi>)
        n1754 = property class="Bool (strict)"(reference=w3064) -> (reference out=w3062:refnum<vi>, error out=w3063:errorcluster, "Value"=w3061:bool)  [unwired: 1 in]
        n1755 = call <vilib>:"Clear Errors.vi"("error in (no error)"=w3041) -> ("error out"=w3056:errorcluster)  [unwired: 5 in, 1 out]
        n1756 = Merge Errors(w3056, w3044) -> (w3045:errorcluster)
        n1757 = Close Reference(reference=w3062, error in (no error)=w3063) -> ()  [unwired: 1 out]
        n1758 = case shown="False" w3061 {
          tunnel: [w3080 w3084] -> w3066
          tunnel: w3065 -> [w3079 w3083]
          tunnel: w3045 -> [w3078 w3082]
          frame True {
            n1759 = call-poly "Enqueue Message.vi"("error in (no error)"=w3078, "Message"="Confirm Quit", "Message Queue"=w3079) -> ("error out"=w3080:errorcluster)  [unwired: 7 in, 1 out]
          }
          frame False {
            n1760 = call-poly "Enqueue Message.vi"("error in (no error)"=w3082, "Message"="Sway Main", "Message Queue"=w3083) -> ("error out"=w3084:errorcluster)  [unwired: 7 in, 1 out]
          }
        }
      }
      frame "Error" {
        # "#CodeRecommended - If you ever change the name of this \"Error\" message, you'll need to update the name in the Check Loop Error.vi as well."
        # "#CodeRecommended - Consider creating a system for logging errors in some way. These errors are for notification purposes only. Handling of specific errors should be performed in the message frames that generated the error."
        # "Error - Display an error dialog. This message is sent by the \"Error Handler\" VIs at the end of other loops in this application."
        n1761 = Variant To Data(error in=w3092, type=errorcluster {"status"=FALSE, "code"=0, "source"=""} ("error constant"), Variant=w3090) -> (data=w3088:errorcluster, error out=w3087:errorcluster)
        n1762 = call <vilib>:"Simple Error Handler.vi"("error in (no error)"=w3088) -> ()  [unwired: 4 in, 5 out]
        n1763 = Merge Errors(w3087) -> (w3086:errorcluster)
      }
      frame "Confirm Quit" {
        # "#CodeNeeded - If you want to provide an \"Are you sure\" dialog (or some other notification) before the application exits, place that code here. This message is typically sent from a Panel Close? event."
        # "Confirm Quit - Message that can confirm whether or not the user wants to exit the application."
        n1764 = call-poly "Enqueue Message.vi"("Priority Message? (F)"=TRUE, "error in (no error)"=w3099, "Message"="Exit", "Message Queue"=w3095) -> ("error out"=w3096:errorcluster)  [unwired: 6 in, 1 out]
        n1765 = Merge Errors(w3096) -> (w3097:errorcluster)
      }
      frame "Exit" {
        # "Stop the VI"
        # "Release the message queue reference"
        # "#CodeNeeded - Add any required cleanup code here. Note that if 'Exit' was called as a result of an error, an error dialog will be displayed. Add any custom error handling for an 'Exit' condition here as well."
        # "Exit - Exit the application."
        n1766 = call "Fire User Event - Stop.vi"("User Event - Stop"=w3100) -> ("error out"=w3102:errorcluster)  [unwired: 10 in]
        n1767 = Release Queue(queue=w3107, error in (no error)=w3101) -> (error out=w3104:errorcluster)  [unwired: 1 in, 2 out]
        n1768 = Merge Errors(w3102, w3104) -> (w3103:errorcluster)
      }
      frame Default {
        # "'Default' case only runs if there is a message that isn't defined in any of the other cases.  Output a programming error."
        n1769 = xnode "Error Ring"("parameter 0"=w3108) -> ("error out"=w3109:errorcluster)
      }
    }
    n1770 = node-c288() -> ()  [unwired: 1 in, 1 out]
    n1771 = call "LAB-IQ Error Handler - Message Handling Loop.vi"("error in (no error)"=w3016, "Message Queue"=w3018) -> ("dup error in"=w3017:errorcluster)  [unwired: 8 in, 1 out]
  }
  n1772 = while {
    shift-right: [w3128] -> _
    shift-left: w26 -> [w3129]
    tunnel: [w3122] -> _
    tunnel: w27 -> [w3120]
    tunnel: w16 -> [w3119]
    tunnel: w25 -> [w3118]
    stop <- w3127 stop-if-true
    # "Program  Handling Loop"
    n1773 = call "Dequeue Message.vi"("error in (no error)"=w3119, "Message Queue"=w3120) -> ("error out"=w3126:errorcluster, "Message Data"=w3124:variant, "Message"=w3125:string, "dup Message Queue"=w3123:refnum<queue>)  [unwired: 6 in]
    n1774 = case "Message Cases" shown="\"Program Main\"" w3125 {
      selector: w3125 -> [_ _ _ _ _ w3174]
      tunnel: w3123 -> [w3130 w3142 _ w3161 w3173 _]
      tunnel: w3126 -> [w3133 w3136 w3158 w3165 w3167 _]
      tunnel: [w3134 w3143 w3152 w3163 w3169 w3175] -> w3121
      tunnel: w3129 -> [w3132 w3135 w3157 w3164 w3172 w3176]
      tunnel: [w3132 w3135 w3157 w3164 w3172 w3176] -> w3128
      tunnel: [_ _ _ _ TRUE _] -> w3127
      tunnel: w3124 -> [_ _ w3156 _ _ _]
      tunnel: w3118 -> [_ _ _ _ w3166 _]
      frame "init" {
        # "Initialize - All initialization work should take place in this message, since other loops can potentially enqueue messages that execute immediately after this one."
        n1775 = call-poly "Enqueue Message.vi"("error in (no error)"=w3133, "Message"="Program Main", "Message Queue"=w3130) -> ("error out"=w3134:errorcluster)  [unwired: 7 in, 1 out]
      }
      frame "Program Main" {
        n1776 = call "Main Program Loop Vi.vi"("error in (no error)"=w3136, "Data Cluster"=w3135) -> ("error out"=w3137:errorcluster)  [unwired: 9 in]
        n1777 = Unbundle By Name(w3135) -> ("Main Home Screen.EXIT"=w3141:refnum<vi>)
        n1778 = property class="Bool (strict)"(reference=w3141) -> (reference out=w3139:refnum<vi>, error out=w3140:errorcluster, "Value"=w3138:bool)  [unwired: 1 in]
        n1779 = case shown="False" w3138 {
          tunnel: [w3146 w3150] -> w3143
          tunnel: w3142 -> [w3145 w3149]
          tunnel: w3137 -> [w3144 w3148]
          frame True {
            n1780 = call-poly "Enqueue Message.vi"("error in (no error)"=w3144, "Message"="Confirm Quit", "Message Queue"=w3145) -> ("error out"=w3146:errorcluster)  [unwired: 7 in, 1 out]
          }
          frame False {
            n1781 = call-poly "Enqueue Message.vi"("error in (no error)"=w3148, "Message"="Program Main", "Message Queue"=w3149) -> ("error out"=w3150:errorcluster)  [unwired: 7 in, 1 out]
          }
        }
        n1782 = Close Reference(reference=w3139, error in (no error)=w3140) -> ()  [unwired: 1 out]
      }
      frame "Error" {
        # "#CodeRecommended - If you ever change the name of this \"Error\" message, you'll need to update the name in the Check Loop Error.vi as well."
        # "#CodeRecommended - Consider creating a system for logging errors in some way. These errors are for notification purposes only. Handling of specific errors should be performed in the message frames that generated the error."
        # "Error - Display an error dialog. This message is sent by the \"Error Handler\" VIs at the end of other loops in this application."
        n1783 = Variant To Data(error in=w3158, type=errorcluster {"status"=FALSE, "code"=0, "source"=""} ("error constant"), Variant=w3156) -> (data=w3154:errorcluster, error out=w3153:errorcluster)
        n1784 = call <vilib>:"Simple Error Handler.vi"("error in (no error)"=w3154) -> ()  [unwired: 4 in, 5 out]
        n1785 = Merge Errors(w3153) -> (w3152:errorcluster)
      }
      frame "Confirm Quit" {
        # "#CodeNeeded - If you want to provide an \"Are you sure\" dialog (or some other notification) before the application exits, place that code here. This message is typically sent from a Panel Close? event."
        # "Confirm Quit - Message that can confirm whether or not the user wants to exit the application."
        n1786 = call-poly "Enqueue Message.vi"("Priority Message? (F)"=TRUE, "error in (no error)"=w3165, "Message"="Exit", "Message Queue"=w3161) -> ("error out"=w3162:errorcluster)  [unwired: 6 in, 1 out]
        n1787 = Merge Errors(w3162) -> (w3163:errorcluster)
      }
      frame "Exit" {
        # "Stop the VI"
        # "Release the message queue reference"
        # "#CodeNeeded - Add any required cleanup code here. Note that if 'Exit' was called as a result of an error, an error dialog will be displayed. Add any custom error handling for an 'Exit' condition here as well."
        # "Exit - Exit the application."
        n1788 = call "Fire User Event - Stop.vi"("User Event - Stop"=w3166) -> ("error out"=w3168:errorcluster)  [unwired: 10 in]
        n1789 = Release Queue(queue=w3173, error in (no error)=w3167) -> (error out=w3170:errorcluster)  [unwired: 1 in, 2 out]
        n1790 = Merge Errors(w3168, w3170) -> (w3169:errorcluster)
      }
      frame Default {
        # "'Default' case only runs if there is a message that isn't defined in any of the other cases.  Output a programming error."
        n1791 = xnode "Error Ring"("parameter 0"=w3174) -> ("error out"=w3175:errorcluster)
      }
    }
    n1792 = call "LAB-IQ Error Handler - Message Handling Loop.vi"("error in (no error)"=w3121, "Message Queue"=w3123) -> ("dup error in"=w3122:errorcluster)  [unwired: 8 in, 1 out]
  }
  n1793 = timed-loop {
    shift-right: [w3194] -> _
    shift-left: w26 -> [w3195]
    tunnel: [w3188] -> _
    tunnel: w24 -> [w3186]
    tunnel: w16 -> [w3185]
    tunnel: w25 -> [w3184]
    timing: w11 -> [_]
    timing-out: [_] -> w10
    stop <- w3193 stop-if-true
    # "Monitor  Handling Loop"
    n1794 = node-c288() -> ()  [unwired: 1 in, 1 out]
    n1795 = call "Dequeue Message.vi"("error in (no error)"=w3185, "Message Queue"=w3186) -> ("error out"=w3192:errorcluster, "Message Data"=w3190:variant, "Message"=w3191:string, "dup Message Queue"=w3189:refnum<queue>)  [unwired: 6 in]
    n1796 = case "Message Cases" shown="\"Monitor Main\"" w3191 {
      selector: w3191 -> [_ _ _ _ _ w3245]
      tunnel: w3189 -> [w3198 w3213 _ w3232 w3244 _]
      tunnel: w3192 -> [w3201 w3203 w3229 w3236 w3238 _]
      tunnel: [w3202 w3214 w3223 w3234 w3240 w3246] -> w3187
      tunnel: w3195 -> [w3200 w3204 w3228 w3235 w3243 w3247]
      tunnel: [w3200 w3204 w3228 w3235 w3243 w3247] -> w3194
      tunnel: [_ _ _ _ TRUE _] -> w3193
      tunnel: w3190 -> [_ _ w3227 _ _ _]
      tunnel: w3184 -> [_ _ _ _ w3237 _]
      frame "init" {
        # "Initialize - All initialization work should take place in this message, since other loops can potentially enqueue messages that execute immediately after this one."
        n1797 = call-poly "Enqueue Message.vi"("error in (no error)"=w3201, "Message"="Monitor Main", "Message Queue"=w3198) -> ("error out"=w3202:errorcluster)  [unwired: 7 in, 1 out]
      }
      frame "Monitor Main" {
        n1798 = call "Main Monitor Loop.vi"("error in (no error)"=w3203, "main ref"=w3204) -> ("error out"=w3208:errorcluster)  [unwired: 9 in]
        n1799 = call "LOAD SELECTION MAIN CODE.vi"("error in (no error)"=w3203, "main ref"=w3204) -> ("error out"=w3206:errorcluster)  [unwired: 9 in]
        n1800 = call "Trip Log and Trip Monitor.vi"("error in (no error)"=w3203, "main ref"=w3204) -> ("error out"=w3205:errorcluster)  [unwired: 9 in]
        n1801 = Merge Errors(w3208, w3206, w3205) -> (w3207:errorcluster)
        n1802 = Unbundle By Name(w3204) -> ("Main Home Screen.EXIT"=w3212:refnum<vi>)
        n1803 = property class="Bool (strict)"(reference=w3212) -> (reference out=w3210:refnum<vi>, error out=w3211:errorcluster, "Value"=w3209:bool)  [unwired: 1 in]
        n1804 = case shown="False" w3209 {
          tunnel: [w3217 w3221] -> w3214
          tunnel: w3213 -> [w3216 w3220]
          tunnel: w3207 -> [w3215 w3219]
          frame True {
            n1805 = call-poly "Enqueue Message.vi"("error in (no error)"=w3215, "Message"="Confirm Quit", "Message Queue"=w3216) -> ("error out"=w3217:errorcluster)  [unwired: 7 in, 1 out]
          }
          frame False {
            n1806 = call-poly "Enqueue Message.vi"("error in (no error)"=w3219, "Message"="Monitor Main", "Message Queue"=w3220) -> ("error out"=w3221:errorcluster)  [unwired: 7 in, 1 out]
          }
        }
        n1807 = Close Reference(reference=w3210, error in (no error)=w3211) -> ()  [unwired: 1 out]
      }
      frame "Error" {
        # "#CodeRecommended - If you ever change the name of this \"Error\" message, you'll need to update the name in the Check Loop Error.vi as well."
        # "#CodeRecommended - Consider creating a system for logging errors in some way. These errors are for notification purposes only. Handling of specific errors should be performed in the message frames that generated the error."
        # "Error - Display an error dialog. This message is sent by the \"Error Handler\" VIs at the end of other loops in this application."
        n1808 = Variant To Data(error in=w3229, type=errorcluster {"status"=FALSE, "code"=0, "source"=""} ("error constant"), Variant=w3227) -> (data=w3225:errorcluster, error out=w3224:errorcluster)
        n1809 = call <vilib>:"Simple Error Handler.vi"("error in (no error)"=w3225) -> ()  [unwired: 4 in, 5 out]
        n1810 = Merge Errors(w3224) -> (w3223:errorcluster)
      }
      frame "Confirm Quit" {
        # "#CodeNeeded - If you want to provide an \"Are you sure\" dialog (or some other notification) before the application exits, place that code here. This message is typically sent from a Panel Close? event."
        # "Confirm Quit - Message that can confirm whether or not the user wants to exit the application."
        n1811 = call-poly "Enqueue Message.vi"("Priority Message? (F)"=TRUE, "error in (no error)"=w3236, "Message"="Exit", "Message Queue"=w3232) -> ("error out"=w3233:errorcluster)  [unwired: 6 in, 1 out]
        n1812 = Merge Errors(w3233) -> (w3234:errorcluster)
      }
      frame "Exit" {
        # "Stop the VI"
        # "Release the message queue reference"
        # "#CodeNeeded - Add any required cleanup code here. Note that if 'Exit' was called as a result of an error, an error dialog will be displayed. Add any custom error handling for an 'Exit' condition here as well."
        # "Exit - Exit the application."
        n1813 = call "Fire User Event - Stop.vi"("User Event - Stop"=w3237) -> ("error out"=w3239:errorcluster)  [unwired: 10 in]
        n1814 = Release Queue(queue=w3244, error in (no error)=w3238) -> (error out=w3241:errorcluster)  [unwired: 1 in, 2 out]
        n1815 = Merge Errors(w3239, w3241) -> (w3240:errorcluster)
      }
      frame Default {
        # "'Default' case only runs if there is a message that isn't defined in any of the other cases.  Output a programming error."
        n1816 = xnode "Error Ring"("parameter 0"=w3245) -> ("error out"=w3246:errorcluster)
      }
    }
    n1817 = node-c288() -> ()  [unwired: 1 in, 1 out]
    n1818 = call "LAB-IQ Error Handler - Message Handling Loop.vi"("error in (no error)"=w3187, "Message Queue"=w3189) -> ("dup error in"=w3188:errorcluster)  [unwired: 8 in, 1 out]
  }
  n1819 = Unregister For Events(event registration refnum=w60, error in=w58) -> (error out=w61:errorcluster)
  n1820 = node-c288(w8) -> ()  [unwired: 1 out]
  n1821 = node-c288(w4) -> ()  [unwired: 1 out]
  n1822 = node-c288(w6) -> ()  [unwired: 1 out]
  n1823 = node-c288(w10) -> ()  [unwired: 1 out]
  n1824 = node-c288(w2) -> ()  [unwired: 1 out]
  n1825 = Merge Errors(w61, w64, w36, w33, w31, w13) -> (w62:errorcluster)
  n1826 = call "Destroy User Event - Stop.vi"("error in (no error)"=w62, "User Event - Stop"=w25) -> ("error out"=w59:errorcluster)  [unwired: 9 in]
  n1827 = disable-structure shown="RUN_TIME_ENGINE==True" {
    disable-tunnel: w59 -> [_ _]
    frame condition #0 (active) {
    }
    frame condition #1 {
      # "Call Quit LabVIEW if running as a built application."
      n1828 = Quit LabVIEW() -> ()  [unwired: 1 in]
    }
  }
